vi "sub_pwrpak7-log_conversion.vi"() -> ()   [LabVIEW 2019]
panel:
  out "data T":dbl[](graph)=[382024.75, 382024.8, 382024.85, 382024.9, 382024.95, 382025.0, 382025.05, 382025.1, 382025.15, 382025.2, 382025.25, 382025.3, 382025.35, 382025.4, 382025.45, 382025.5, 382025.55, 382025.65, 382025.75, 382025.85, 382025.95, 382026.05, 382026.15, 382026.25, 382026.35, 382026.45, 382026.55, 382026.65, 382026.75, 382026.85, 382026.95, 382027.05, 382027.15, 382027.25, 382027.35, 382027.45, 382027.55, 382027.65, 382027.75, 382027.85, 382027.95, 382028.05, 382028.15, 382028.25, 382028.35, 382028.45, 382028.55, 382028.65, 382028.75, 382028.75, 382028.85, 382028.95, 382029.0, 382029.05, 382029.2, 382029.25, 382029.4, 382029.45, 382029.45, 382029.6, 382029.65, 382029.65, 382029.8, 382029.85, 382029.85, 382029.95, 382030.0, 382030.05, 382030.1, 382030.15, 382030.2, 382030.25, 382030.3, 382030.35, 382030.4, 382030.45, 382030.5, 382030.55, 382030.6, 382030.65, 382030.7, 382030.75, 382030.8, 382030.85, 382030.9, 382030.95, 382031.0, 382031.05, 382031.1, 382031.15, 382031.2, 382031.25, 382031.3, 382031.35, 382031.45, 382031.5, 382031.55, 382031.65, 382031.7, 382031.75, 382031.85, 382031.95, 382032.05, 382032.15, 382032.25, 382032.35, 382032.45, 382032.55, 382032.65, 382032.75, 382032.85, 382032.95, 382033.05, 382033.15, 382033.25, 382033.35, 382033.45, 382033.55, 382033.65, 382033.75, 382033.85, 382033.95, 382034.05, 382034.15, 382034.25, 382034.35, 382034.45, 382034.55, 382034.65, 382034.65, 382034.75, 382034.85, 382034.95, 382035.05, 382035.15, 382035.25, 382035.25, 382035.35, 382035.45, 382035.5, 382035.55, 382035.7, 382035.75, 382035.85, 382035.9, 382035.95, 382036.05, 382036.1, 382036.15, 382036.3, 382036.35, 382036.35, 382036.5, 382036.55, 382036.55, 382036.7, 382036.75, 382036.75, 382036.85, 382036.9, 382036.95, 382037.0, 382037.05, 382037.1, 382037.15, 382037.2, 382037.25, 382037.3, 382037.35, 382037.4, 382037.45, 382037.5, 382037.55, 382037.6, 382037.65, 382037.7, 382037.75, 382037.8, 382037.85, 382037.95, 382038.0, 382038.05, 382038.15, 382038.2, 382038.25, 382038.35, 382038.4, 382038.45, 382038.55, 382038.6, 382038.65, 382038.75, 382038.8, 382038.85, 382038.95, 382039.05, 382039.15, 382039.25, 382039.3, 382039.35, 382039.45, 382039.5, 382039.55, 382039.65, 382039.7, 382039.75, 382039.85, 382039.95, 382040.05, 382040.15, 382040.25, 382040.35, 382040.45, 382040.55, 382040.65, 382040.75, 382040.85, 382040.95, 382041.05, 382041.15, 382041.25, 382041.35, 382041.45, 382041.55, 382041.65, 382041.75, 382041.85, 382041.95, 382042.05, 382042.15, 382042.25, 382042.35, 382042.35, 382042.5, 382042.55, 382042.55, 382042.7, 382042.75, 382042.75, 382042.9, 382042.95, 382043.0, 382043.05, 382043.15, 382043.2, 382043.3, 382043.35, 382043.4, 382043.45, 382043.55, 382043.6, 382043.65, 382043.65, 382043.75, 382043.8, 382043.85, 382043.85, 382043.95, 382044.0, 382044.05, 382044.1, 382044.15, 382044.2, 382044.25, 382044.3, 382044.35, 382044.4, 382044.45, 382044.5, 382044.55, 382044.6, 382044.65, 382044.7, 382044.75, 382044.8, 382044.85, 382044.9, 382044.95, 382045.05, 382045.1, 382045.15, 382045.25, 382045.3, 382045.35, 382045.45, 382045.5, 382045.55, 382045.65, 382045.7, 382045.75, 382045.85, 382045.9, 382045.95, 382046.0, 382046.05, 382046.15, 382046.25, 382046.35, 382046.45, 382046.55, 382046.65, 382046.75, 382046.85, 382046.95, 382047.05, 382047.15, 382047.25, 382047.35, 382047.45, 382047.55, 382047.65, 382047.75, 382047.85, 382047.95, 382048.05, 382048.15, 382048.25, 382048.35, 382048.45, 382048.55, 382048.65, 382048.75, 382048.85, 382048.95, 382049.05, 382049.15, 382049.25, 382049.35, 382049.45, 382049.55, 382049.55, 382049.65, 382049.75, 382049.8, 382049.85, 382049.95, 382050.0, 382050.05, 382050.05, 382050.15, 382050.2, 382050.25, 382050.25, 382050.35, 382050.4, 382050.45, 382050.45, 382050.55, 382050.6, 382050.65, 382050.7, 382050.75, 382050.8, 382050.85, 382050.9, 382050.95, 382051.0, 382051.05, 382051.1, 382051.15, 382051.2, 382051.25, 382051.3, 382051.35, 382051.4, 382051.45, 382051.5, 382051.55, 382051.65, 382051.7, 382051.75, 382051.85, 382051.9, 382051.95, 382052.05, 382052.1, 382052.15, 382052.25, 382052.3, 382052.35, 382052.45, 382052.5, 382052.55, 382052.65, 382052.75, 382052.85, 382052.95, 382053.05, 382053.15, 382053.25, 382053.35, 382053.45, 382053.55, 382053.65, 382053.75, 382053.85, 382053.95, 382054.05, 382054.15, 382054.25, 382054.35, 382054.45, 382054.55, 382054.65, 382054.75, 382054.85, 382054.95, 382055.05, 382055.15, 382055.25, 382055.35, 382055.45, 382055.6, 382055.65, 382055.75, 382055.85, 382055.95, 382056.05, 382056.05, 382056.15, 382056.25, 382056.25, 382056.35, 382056.45, 382056.5, 382056.55, 382056.65, 382056.7, 382056.75, 382056.85, 382056.9, 382056.95, 382057.05, 382057.1, 382057.15, 382057.15, 382057.25, 382057.3, 382057.35, 382057.35, 382057.45, 382057.5, 382057.55, 382057.6, 382057.65, 382057.7, 382057.75, 382057.8, 382057.85, 382057.9, 382057.95, 382058.0, 382058.05, 382058.1, 382058.15, 382058.2, 382058.25, 382058.3, 382058.35, 382058.4, 382058.45, 382058.55, 382058.6, 382058.65, 382058.75, 382058.8, 382058.85, 382058.95, 382059.0, 382059.05, 382059.15, 382059.2, 382059.25, 382059.35, 382059.4, 382059.45, 382059.55, 382059.6, 382059.65, 382059.75, 382059.8, 382059.85, 382059.95, 382060.0, 382060.05, 382060.15, 382060.25, 382060.35, 382060.4, 382060.45, 382060.55, 382060.6, 382060.65, 382060.75, 382060.85, 382060.95, 382061.05, 382061.15, 382061.25, 382061.35, 382061.45, 382061.55, 382061.65, 382061.75, 382061.85, 382061.95, 382062.05, 382062.15, 382062.25, 382062.35, 382062.45, 382062.55, 382062.65, 382062.75, 382062.85, 382062.95, 382063.05, 382063.05, 382063.15, 382063.25, 382063.25, 382063.35, 382063.45, 382063.5, 382063.55, 382063.65, 382063.7, 382063.75, 382063.85, 382063.9, 382063.95, 382063.95, 382064.1, 382064.15, 382064.15, 382064.25, 382064.3, 382064.35, 382064.35, 382064.5, 382064.55, 382064.6, 382064.7, 382064.75, 382064.8, 382064.9, 382064.95, 382065.0, 382065.05, 382065.1, 382065.15, 382065.2, 382065.25, 382065.3, 382065.35, 382065.4, 382065.45, 382065.5, 382065.55, 382065.6, 382065.65, 382065.75, 382065.8, 382065.85, 382065.9, 382065.95, 382066.0, 382066.05, 382066.1, 382066.15, 382066.2, 382066.25, 382066.3, 382066.35, 382066.4, 382066.45, 382066.5, 382066.55, 382066.65, 382066.7, 382066.75, 382066.85, 382066.9, 382066.95, 382067.05, 382067.1, 382067.15, 382067.25, 382067.3, 382067.35, 382067.45, 382067.5, 382067.55, 382067.65, 382067.75, 382067.85, 382067.9, 382067.95, 382068.05, 382068.15, 382068.25, 382068.35, 382068.45, 382068.55, 382068.65, 382068.75, 382068.85, 382068.95, 382069.05, 382069.15, 382069.25, 382069.35, 382069.45, 382069.55, 382069.65, 382069.75, 382069.85, 382069.95, 382070.05, 382070.15, 382070.25, 382070.35, 382070.45, 382070.55, 382070.55, 382070.65, 382070.75, 382070.75, 382070.9, 382070.95, 382071.1, 382071.15, 382071.15, 382071.3, 382071.35, 382071.35, 382071.45, 382071.55, 382071.6, 382071.7, 382071.75, 382071.8, 382071.85, 382071.95, 382072.0, 382072.05, 382072.1, 382072.15, 382072.2, 382072.25, 382072.25, 382072.35, 382072.4, 382072.45, 382072.45, 382072.55, 382072.6, 382072.65, 382072.75, 382072.8, 382072.85, 382072.9, 382072.95, 382073.0, 382073.05, 382073.1, 382073.15, 382073.2, 382073.25, 382073.3, 382073.35, 382073.4, 382073.45, 382073.5, 382073.55, 382073.6, 382073.65, 382073.7, 382073.75, 382073.8, 382073.85, 382073.95, 382074.05, 382074.1, 382074.15, 382074.25, 382074.35, 382074.45, 382074.5, 382074.55, 382074.65, 382074.75, 382074.85, 382074.95, 382075.05, 382075.15, 382075.25, 382075.35, 382075.45, 382075.55, 382075.65, 382075.75, 382075.85, 382075.95, 382076.05, 382076.15, 382076.25, 382076.35, 382076.45, 382076.55, 382076.7, 382076.75, 382076.9, 382076.95, 382077.05, 382077.15, 382077.15, 382077.3, 382077.35, 382077.35, 382077.45, 382077.55, 382077.55, 382077.7, 382077.75, 382077.8, 382077.9, 382077.95, 382078.0, 382078.05, 382078.15, 382078.2, 382078.25, 382078.3, 382078.35, 382078.4, 382078.45, 382078.5, 382078.55, 382078.6, 382078.65, 382078.7, 382078.75, 382078.8, 382078.85, 382078.95, 382079.0, 382079.05, 382079.15, 382079.2, 382079.25, 382079.35, 382079.4, 382079.45, 382079.55, 382079.6, 382079.65, 382079.7, 382079.75, 382079.85, 382079.95, 382080.05, 382080.15, 382080.25, 382080.35, 382080.45, 382080.5, 382080.55, 382080.65, 382080.75, 382080.85, 382080.95, 382081.05, 382081.15, 382081.25, 382081.35, 382081.45, 382081.55, 382081.65, 382081.75, 382081.85, 382081.95, 382082.05, 382082.15, 382082.25, 382082.35, 382082.45, 382082.55, 382082.65, 382082.75, 382082.85, 382082.95, 382083.05, 382083.15, 382083.3, 382083.35, 382083.45, 382083.55, 382083.7, 382083.75, 382083.75, 382083.9, 382083.95, 382084.1, 382084.15, 382084.15, 382084.3, 382084.35, 382084.35, 382084.5, 382084.55, 382084.55, 382084.65, 382084.7, 382084.75, 382084.75, 382084.9, 382084.95, 382084.95, 382085.05, 382085.1, 382085.15, 382085.15, 382085.25, 382085.3, 382085.35, 382085.35, 382085.45, 382085.5, 382085.55, 382085.6, 382085.65, 382085.7, 382085.75, 382085.8, 382085.85, 382085.9, 382085.95, 382086.0, 382086.05, 382086.1, 382086.15, 382086.2, 382086.25, 382086.3, 382086.35, 382086.4, 382086.45, 382086.55, 382086.6, 382086.65, 382086.75, 382086.8, 382086.85, 382086.95, 382087.0, 382087.05, 382087.15, 382087.2, 382087.25, 382087.35, 382087.45]
  out "heading T":dbl[](graph)=[382025.6, 382025.7, 382025.8, 382025.9, 382026.0, 382026.1, 382026.2, 382026.3, 382026.4, 382026.5, 382026.6, 382026.7, 382026.8, 382026.9, 382027.0, 382027.1, 382027.2, 382027.3, 382027.4, 382027.5, 382027.6, 382027.7, 382027.8, 382027.9, 382028.0, 382028.1, 382028.2, 382028.3, 382028.4, 382028.5, 382028.6, 382028.8, 382029.0, 382029.1, 382029.2, 382029.3, 382029.5, 382029.7, 382031.4, 382031.6, 382031.8, 382031.9, 382032.0, 382032.1, 382032.2, 382032.3, 382032.4, 382032.5, 382032.6, 382032.7, 382032.8, 382032.9, 382033.0, 382033.1, 382033.2, 382033.3, 382033.4, 382033.5, 382033.6, 382033.7, 382033.8, 382033.9, 382034.0, 382034.1, 382034.2, 382034.3, 382034.4, 382034.5, 382034.7, 382034.8, 382034.9, 382035.0, 382035.1, 382035.3, 382035.5, 382035.6, 382035.7, 382035.9, 382036.1, 382036.2, 382036.4, 382036.6, 382037.9, 382038.1, 382038.3, 382038.5, 382038.7, 382038.9, 382039.0, 382039.1, 382039.2, 382039.4, 382039.6, 382039.8, 382039.9, 382040.0, 382040.1, 382040.2, 382040.3, 382040.4, 382040.5, 382040.6, 382040.7, 382040.8, 382040.9, 382041.0, 382041.1, 382041.2, 382041.3, 382041.4, 382041.5, 382041.6, 382041.7, 382041.8, 382041.9, 382042.0, 382042.1, 382042.2, 382042.4, 382042.6, 382042.8, 382043.0, 382043.2, 382043.4, 382045.0, 382045.2, 382045.4, 382045.6, 382045.8, 382046.1, 382046.2, 382046.3, 382046.4, 382046.5, 382046.6, 382046.7, 382046.8, 382046.9, 382047.0, 382047.1, 382047.2, 382047.3, 382047.4, 382047.5, 382047.6, 382047.7, 382047.8, 382047.9, 382048.0, 382048.1, 382048.2, 382048.3, 382048.4, 382048.5, 382048.6, 382048.7, 382048.8, 382048.9, 382049.0, 382049.1, 382049.2, 382049.3, 382049.4, 382049.6, 382049.8, 382051.6, 382051.8, 382052.0, 382052.2, 382052.4, 382052.6, 382052.7, 382052.8, 382052.9, 382053.0, 382053.1, 382053.2, 382053.3, 382053.4, 382053.5, 382053.6, 382053.7, 382053.8, 382053.9, 382054.0, 382054.1, 382054.2, 382054.3, 382054.4, 382054.5, 382054.6, 382054.7, 382054.8, 382054.9, 382055.0, 382055.1, 382055.2, 382055.3, 382055.4, 382055.5, 382055.6, 382055.7, 382055.8, 382055.9, 382056.1, 382056.3, 382056.5, 382056.7, 382056.9, 382058.5, 382058.7, 382058.9, 382059.1, 382059.3, 382059.5, 382059.7, 382059.9, 382060.1, 382060.2, 382060.3, 382060.5, 382060.7, 382060.8, 382060.9, 382061.0, 382061.1, 382061.2, 382061.3, 382061.4, 382061.5, 382061.6, 382061.7, 382061.8, 382061.9, 382062.0, 382062.1, 382062.2, 382062.3, 382062.4, 382062.5, 382062.6, 382062.7, 382062.8, 382062.9, 382063.1, 382063.3, 382063.5, 382063.7, 382064.0, 382064.4, 382064.6, 382064.8, 382065.7, 382066.6, 382066.8, 382067.0, 382067.2, 382067.4, 382067.6, 382067.7, 382067.8, 382068.0, 382068.1, 382068.2, 382068.3, 382068.4, 382068.5, 382068.6, 382068.7, 382068.8, 382068.9, 382069.0, 382069.1, 382069.2, 382069.3, 382069.4, 382069.5, 382069.6, 382069.7, 382069.8, 382069.9, 382070.0, 382070.1, 382070.2, 382070.3, 382070.4, 382070.6, 382070.8, 382070.9, 382071.0, 382071.2, 382071.4, 382071.6, 382071.8, 382072.7, 382073.9, 382074.0, 382074.2, 382074.3, 382074.4, 382074.6, 382074.7, 382074.8, 382074.9, 382075.0, 382075.1, 382075.2, 382075.3, 382075.4, 382075.5, 382075.6, 382075.7, 382075.8, 382075.9, 382076.0, 382076.1, 382076.2, 382076.3, 382076.4, 382076.5, 382076.6, 382076.7, 382076.8, 382076.9, 382077.0, 382077.2, 382077.4, 382077.6, 382077.8, 382078.0, 382078.9, 382079.1, 382079.3, 382079.5, 382079.8, 382079.9, 382080.0, 382080.1, 382080.2, 382080.3, 382080.4, 382080.6, 382080.7, 382080.8, 382080.9, 382081.0, 382081.1, 382081.2, 382081.3, 382081.4, 382081.5, 382081.6, 382081.7, 382081.8, 382081.9, 382082.0, 382082.1, 382082.2, 382082.3, 382082.4, 382082.5, 382082.6, 382082.7, 382082.8, 382082.9, 382083.0, 382083.1, 382083.2, 382083.3, 382083.4, 382083.5, 382083.6, 382083.8, 382083.9, 382084.0, 382084.2, 382084.4, 382084.8, 382086.5, 382086.7, 382086.9, 382087.1, 382087.3, 382087.4]
  out "I":i32=3229
  out "heading arr":string[][](array[string])
  out "data arr":string[][](array[string])
  out "부분배열":string[](array[string])=["", "", "", "", "", "", "", "", "", "", "", "", "", "", "", "", "", "", "", "", "", "", "", "", "", "", "", "", "", "", "", "", "", "", "", "", "", "", "", "", "", "", "", "", "", "", "", "", "", "", "", "", "", "", "", "", "", "", "", "", "", "", "", "", "", "", "", "", "", "", "", "", "", "", "", "", "", "", "", "", "", "", "", "", "", "", "", "", "", "", "", "", "", "", "", "", "", "", "", "", "", "", "", "", "", "", "", "", "", "", "", "", "", "", "", "", "", "", "", "", "", "", "", "", "", "", "", "", "", "", "", "", "", "", "", "", "", "", "", "", "", "", "", "", "", "", "", "", "", "", "", "", "", "", "", "", "", "", "", "", "", "", "", "", "", "", "", "", "", "", "", "", "", "", "", "", "", "", "", "", "", "", "", "", "", "", "", "", "", "", "", "", "", "", "", "", "", "", "", "", "", "", "", "", "", "", "", "", "", "", "", "", "", "", "", "", "", "", "", "", "", "", "", "", "", "", "", "", "", "", "", "", "", "", "", "", "<OK", "robot status", "<OK", "robot status", "<OK", "robot status", "<OK", "robot status", "<OK", "robot status", "<OK", "robot status", "<OK", "robot status", "<OK", "robot status", "<OK", "robot status", "<OK", "robot status", "<OK", "robot status", "<OK", "robot status", "<OK", "robot status", "<OK", "robot status", "<OK", "robot status", "<OK", "robot status", "<OK", "robot status", "<OK", "robot status", "<OK", "robot status", "<OK", "robot status", "<OK", "robot status", "<OK", "robot status", "<OK", "robot status", "<OK", "robot status", "<OK", "robot status", "<OK", "robot status", "<OK", "robot status", "<OK", "robot status", "<OK", "robot status", "<OK", "robot status", "<OK", "robot status", "<OK", "robot status", "<OK", "robot status", "<OK", "robot status", "<OK", "robot status", "<OK", "robot status", "<OK", "robot status", "<OK", "robot status", "<OK", "robot status", "<OK", "robot status", "<OK", "robot status", "<OK", "robot status", "<OK", "robot status", "<OK", "robot status", "<OK", "robot status", "<OK", "robot status", "<OK", "robot status", "<OK", "robot status", "<OK", "robot status", "<OK", "robot status", "<OK", "robot status", "<OK", "robot status", "<OK", "robot status", "<OK", "robot status", "<OK", "robot status", "<OK", "robot status", "<OK", "robot status", "<OK", "robot status", "<OK", "robot status", "<OK", "robot status", "<OK", "robot status", "<OK", "robot status", "<OK", "robot status", "<OK", "robot status", "<OK", "robot status", "<OK", "robot status", "<OK", "robot status", "<OK", "robot status", "<OK", "robot status", "<OK", "robot status", "<OK", "robot status", "<OK", "robot status", "<OK", "robot status", "<OK", "robot status", "<OK", "robot status", "<OK", "robot status", "<OK", "robot status", "<OK", "robot status", "<OK", "robot status", "<OK", "robot status", "<OK", "robot status", "<OK", "robot status", "<OK", "robot status", "<OK", "robot status", "<OK", "robot status", "<OK", "robot status", "<OK", "robot status", "<OK", "robot status", "<OK", "robot status", "<OK", "robot status", "<OK", "robot status", "<OK", "robot status", "<OK", "robot status", "<OK", "robot status", "<OK", "robot status", "<OK", "robot status", "<OK", "robot status", "<OK", "robot status", "<OK", "robot status", "<OK", "robot status", "<OK", "robot status", "<OK", "robot status", "<OK", "robot status", "<OK", "robot status", "<OK", "robot status", "<OK", "robot status", "<OK", "robot status", "<OK", "robot status", "<OK", "robot status", "<OK", "robot status", "<OK", "robot status", "<OK", "robot status", "<OK", "robot status", "<OK", "robot status", "<OK", "robot status", "<OK", "robot status", "<OK", "robot status", "<OK", "robot status", "<OK", "robot status", "<OK", "robot status", "<OK", "robot status", "<OK", "robot status", "<OK", "robot status", "<OK", "robot status", "<OK", "robot status", "<OK", "robot status", "<OK", "robot status", "<OK", "robot status", "<OK", "robot status", "<OK", "robot status", "<OK", "robot status", "<OK", "robot status", "<OK", "robot status", "<OK", "robot status", "<OK", "robot status", "<OK", "robot status", "<OK", "robot status", "<OK", "robot status", "<OK", "robot status", "<OK", "robot status", "<OK", "robot status", "<OK", "robot status", "<OK", "robot status", "<OK", "robot status", "<OK", "robot status", "<OK", "robot status", "<OK", "robot status", "<OK", "robot status", "<OK", "robot status", "<OK", "robot status", "<OK", "robot status", "<OK", "robot status", "<OK", "robot status", "<OK", "robot status", "<OK", "robot status", "<OK", "robot status", "<OK", "robot status", "<OK", "robot status", "<OK", "robot status", "<OK", "robot status", "<OK", "robot status", "<OK", "robot status", "<OK", "robot status", "<OK", "robot status", "<OK", "robot status", "<OK", "robot status", "<OK", "robot status", "<OK", "robot status", "<OK", "robot status", "<OK", "robot status", "<OK", "robot status", "<OK", "robot status", "<OK", "robot status", "<OK", "robot status", "<OK", "robot status", "<OK", "robot status", "<OK", "robot status", "<OK", "robot status", "<OK", "robot status", "<OK", "robot status", "<OK", "robot status", "<OK", "robot status", "<OK", "robot status", "<OK", "robot status", "<OK", "robot status", "<OK", "robot status", "<OK", "robot status", "<OK", "robot status", "<OK", "robot status", "<OK", "robot status", "<OK", "robot status", "<OK", "robot status", "<OK", "robot status", "<OK", "robot status", "<OK", "robot status", "<OK", "robot status", "<OK", "robot status", "<OK", "robot status", "<OK", "robot status", "<OK", "robot status", "<OK", "robot status", "<OK", "robot status", "<OK", "robot status", "<OK", "robot status", "<OK", "robot status", "<OK", "robot status", "<OK", "robot status", "<OK", "robot status", "<OK", "robot status", "<OK", "robot status", "<OK", "robot status", "<OK", "robot status", "<OK", "robot status", "<OK", "robot status", "<OK", "robot status", "<OK", "robot status", "<OK", "robot status", "<OK", "robot status", "<OK", "robot status", "<OK", "robot status", "<OK", "robot status", "<OK", "robot status", "<OK", "robot status", "<OK", "robot status", "<OK", "robot status", "<OK", "robot status", "<OK", "robot status", "<OK", "robot status", "<OK", "robot status", "<OK", "robot status", "<OK", "robot status", "<OK", "robot status", "<OK", "robot status", "<OK", "robot status", "<OK", "robot status", "<OK", "robot status", "<OK", "robot status", "<OK", "robot status", "<OK", "robot status", "<OK", "robot status", "<OK", "robot status", "<OK", "robot status", "<OK", "robot status", "<OK", "robot status", "<OK", "robot status", "<OK", "robot status", "<OK", "robot status", "<OK", "robot status", "<OK", "robot status", "<OK", "robot status", "<OK", "robot status", "#INSPVAXA,USB3,0,41.0,FINESTEERING,2113,382024.750,02000000,471d,15824;INS_SOLUTION_GOOD,INS_RTKFIXED,37.37018369976,126.72086597157,9.9381,22.3000,0.0198,0.0069,0.0055,-0.729721292,-0.467737212,152.592783383,0.0830,0.0922,0.0819,0.0253,0.0263,0.0205,0.0289,0.0288,0.0775,0f000041,0*b216c52d", "robot status", "#INSPVAXA,USB3,0,41.0,FINESTEERING,2113,382024.800,02000000,471d,15824;INS_SOLUTION_GOOD,INS_RTKFIXED,37.37018370626,126.72086597191,9.9383,22.3000,0.0206,0.0063,0.0054,-0.730371572,-0.467330960,152.593899261,0.0830,0.0922,0.0819,0.0253,0.0263,0.0205,0.0289,0.0288,0.0775,0f000041,0*340d1d1e", "robot status", "#INSPVAXA,USB3,0,41.0,FINESTEERING,2113,382024.850,02000000,471d,15824;INS_SOLUTION_GOOD,INS_RTKFIXED,37.37018371265,126.72086597165,9.9385,22.3000,0.0208,0.0067,0.0057,-0.730042287,-0.466924674,152.593459848,0.0830,0.0922,0.0819,0.0253,0.0263,0.0205,0.0289,0.0288,0.0775,0f000041,0*a3e0566d", "robot status", "#INSPVAXA,USB3,0,41.0,FINESTEERING,2113,382024.900,02000000,471d,15824;INS_SOLUTION_GOOD,INS_RTKFIXED,37.37018371942,126.72086597216,9.9387,22.3000,0.0203,0.0070,0.0059,-0.730302817,-0.466656468,152.594518112,0.0830,0.0922,0.0819,0.0253,0.0263,0.0205,0.0289,0.0288,0.0775,0f000041,0*b966c6e0", "robot status", "#INSPVAXA,USB3,0,41.0,FINESTEERING,2113,382024.950,02000000,471d,15824;INS_SOLUTION_GOOD,INS_RTKFIXED,37.37018372616,126.72086597280,9.9389,22.3000,0.0205,0.0071,0.0058,-0.729837391,-0.467014747,152.594484484,0.0830,0.0922,0.0819,0.0253,0.0263,0.0205,0.0289,0.0288,0.0775,0f000041,0*c9b08c61", "robot status", "#INSPVAXA,USB3,0,41.0,FINESTEERING,2113,382025.000,02000000,471d,15824;INS_SOLUTION_GOOD,INS_RTKFIXED,37.37018373314,126.72086597346,9.9392,22.3000,0.0211,0.0068,0.0059,-0.729725959,-0.466969403,152.594152669,0.0830,0.0922,0.0819,0.0253,0.0263,0.0205,0.0289,0.0288,0.0775,0f000041,0*c8abde32", "robot status", "#INSPVAXA,USB3,0,41.0,FINESTEERING,2113,382025.050,02000000,471d,15824;INS_SOLUTION_GOOD,INS_RTKFIXED,37.37018373760,126.72086597197,9.9393,22.3000,0.0218,0.0067,0.0058,-0.729631791,-0.467061420,152.593830540,0.0961,0.1071,0.0938,0.0275,0.0290,0.0215,0.0301,0.0299,0.0782,0f000041,0*f74ecec6", "robot status", "#INSPVAXA,USB3,0,45.5,FINESTEERING,2113,382025.100,02000000,471d,15824;INS_SOLUTION_GOOD,INS_RTKFIXED,37.37018374163,126.72086597046,9.9393,22.3000,0.0217,0.0067,0.0060,-0.730180033,-0.466610622,152.593108629,0.0961,0.1071,0.0938,0.0275,0.0290,0.0215,0.0301,0.0299,0.0782,0f000041,0*ede3f3a7", "robot status", "#INSPVAXA,USB3,0,45.5,FINESTEERING,2113,382025.150,02000000,471d,15824;INS_SOLUTION_GOOD,INS_RTKFIXED,37.37018374560,126.72086596911,9.9394,22.3000,0.0214,0.0071,0.0058,-0.729850693,-0.466261357,152.594252106,0.0961,0.1071,0.0938,0.0275,0.0290,0.0215,0.0301,0.0299,0.0782,0f000041,0*dbccd46e", "robot status", "#INSPVAXA,USB3,0,45.5,FINESTEERING,2113,382025.200,02000000,471d,15824;INS_SOLUTION_GOOD,INS_RTKFIXED,37.37018374958,126.72086596786,9.9395,22.3000,0.0215,0.0068,0.0059,-0.730016188,-0.466427204,152.593304599,0.0961,0.1071,0.0938,0.0275,0.0290,0.0215,0.0301,0.0299,0.0782,0f000041,0*6894b41e", "robot status", "#INSPVAXA,USB3,0,45.5,FINESTEERING,2113,382025.250,02000000,471d,15824;INS_SOLUTION_GOOD,INS_RTKFIXED,37.37018375384,126.72086596657,9.9396,22.3000,0.0223,0.0069,0.0058,-0.730137890,-0.466685773,152.593266150,0.0961,0.1071,0.0938,0.0275,0.0290,0.0215,0.0301,0.0299,0.0782,0f000041,0*47582ee5", "robot status", "#INSPVAXA,USB3,0,45.5,FINESTEERING,2113,382025.300,02000000,471d,15824;INS_SOLUTION_GOOD,INS_RTKFIXED,37.37018375759,126.72086596450,9.9396,22.3000,0.0226,0.0066,0.0057,-0.729934603,-0.466322917,152.593247189,0.0961,0.1071,0.0938,0.0275,0.0290,0.0215,0.0301,0.0299,0.0782,0f000041,0*28a54055", "robot status", "#INSPVAXA,USB3,0,45.5,FINESTEERING,2113,382025.350,02000000,471d,15824;INS_SOLUTION_GOOD,INS_RTKFIXED,37.37018376219,126.72086596322,9.9397,22.3000,0.0224,0.0067,0.0057,-0.729983991,-0.466103112,152.593315489,0.0961,0.1071,0.0938,0.0275,0.0290,0.0215,0.0301,0.0299,0.0782,0f000041,0*5693f211", "robot status", "#INSPVAXA,USB3,0,45.5,FINESTEERING,2113,382025.400,02000000,471d,15824;INS_SOLUTION_GOOD,INS_RTKFIXED,37.37018376676,126.72086596200,9.9398,22.3000,0.0225,0.0065,0.0057,-0.729588122,-0.466736324,152.593809863,0.0961,0.1071,0.0938,0.0275,0.0290,0.0215,0.0301,0.0299,0.0782,0f000041,0*8175a42e", "robot status", "#INSPVAXA,USB3,0,45.5,FINESTEERING,2113,382025.450,02000000,471d,15824;INS_SOLUTION_GOOD,INS_RTKFIXED,37.37018377077,126.72086595999,9.9398,22.3000,0.0231,0.0063,0.0056,-0.729925270,-0.467152594,152.593776517,0.0961,0.1071,0.0938,0.0275,0.0290,0.0215,0.0301,0.0299,0.0782,0f000041,0*10a645a0", "robot status", "#INSPVAXA,USB3,0,45.5,FINESTEERING,2113,382025.500,02000000,471d,15824;INS_SOLUTION_GOOD,INS_RTKFIXED,37.37018377589,126.72086595868,9.9399,22.3000,0.0237,0.0061,0.0057,-0.729817898,-0.467054387,152.593893018,0.0961,0.1071,0.0938,0.0275,0.0290,0.0215,0.0301,0.0299,0.0782,0f000041,0*9fba37f2", "robot status", "#INSPVAXA,USB3,0,45.5,FINESTEERING,2113,382025.550,02000000,471d,15824;INS_SOLUTION_GOOD,INS_RTKFIXED,37.37018378124,126.72086595741,9.9400,22.3000,0.0238,0.0062,0.0056,-0.729449696,-0.467439102,152.593895045,0.0961,0.1071,0.0938,0.0275,0.0290,0.0215,0.0301,0.0299,0.0782,0f000041,0*02ddb99e", "robot status", "#DUALANTENNAHEADINGA,USB3,0,45.5,FINESTEERING,2113,382025.600,02000000,d426,15824;SOL_COMPUTED,NARROW_INT,-1.000000000,157.761886597,-14.048614502,0.0,0.340079188,0.906907201,\"681H\",37,27,27,20,04,00,30,33*30139603", "robot status", "#INSPVAXA,USB3,0,45.5,FINESTEERING,2113,382025.650,02000000,471d,15824;INS_SOLUTION_GOOD,INS_RTKFIXED,37.37018379199,126.72086595512,9.9402,22.3000,0.0238,0.0064,0.0057,-0.729977006,-0.466502482,152.593562345,0.0961,0.1071,0.0938,0.0275,0.0290,0.0215,0.0301,0.0299,0.0782,0f000041,0*e9293c2f", "robot status", "#DUALANTENNAHEADINGA,USB3,0,45.5,FINESTEERING,2113,382025.700,02000000,d426,15824;SOL_COMPUTED,NARROW_INT,-1.000000000,157.699172974,-14.030242920,0.0,0.340588301,0.908101737,\"681H\",37,27,27,20,04,00,30,33*1b355fa5", "robot status", "#INSPVAXA,USB3,0,45.5,FINESTEERING,2113,382025.750,02000000,471d,15824;INS_SOLUTION_GOOD,INS_RTKFIXED,37.37018380260,126.72086595218,9.9404,22.3000,0.0244,0.0062,0.0058,-0.728657563,-0.465931440,152.593624205,0.0961,0.1071,0.0938,0.0275,0.0290,0.0215,0.0301,0.0299,0.0782,0f000041,0*74c13f5b", "robot status", "#DUALANTENNAHEADINGA,USB3,0,45.5,FINESTEERING,2113,382025.800,02000000,d426,15824;SOL_COMPUTED,NARROW_INT,-1.000000000,157.821578979,-14.375122070,0.0,0.342067271,0.910245121,\"681H\",37,27,27,20,04,00,30,33*2529407e", "robot status", "#INSPVAXA,USB3,0,45.5,FINESTEERING,2113,382025.850,02000000,471d,15824;INS_SOLUTION_GOOD,INS_RTKFIXED,37.37018381375,126.72086594948,9.9405,22.3000,0.0243,0.0064,0.0059,-0.728879825,-0.466013684,152.593850424,0.0961,0.1071,0.0938,0.0275,0.0290,0.0215,0.0301,0.0299,0.0782,0f000041,0*d9358f05", "robot status", "#DUALANTENNAHEADINGA,USB3,0,45.5,FINESTEERING,2113,382025.900,02000000,d426,15824;SOL_COMPUTED,NARROW_INT,-1.000000000,157.786605835,-14.218627930,0.0,0.341675878,0.910721183,\"681H\",37,27,27,20,04,00,30,33*64d0d047", "robot status", "#INSPVAXA,USB3,0,45.5,FINESTEERING,2113,382025.950,02000000,471d,15824;INS_SOLUTION_GOOD,INS_RTKFIXED,37.37018382627,126.72086594769,9.9407,22.3000,0.0251,0.0064,0.0057,-0.728736707,-0.465697206,152.593264431,0.0961,0.1071,0.0938,0.0275,0.0290,0.0215,0.0301,0.0299,0.0782,0f000041,0*70b4c2e8", "robot status", "#DUALANTENNAHEADINGA,USB3,0,45.5,FINESTEERING,2113,382026.000,02000000,d426,15824;SOL_COMPUTED,NARROW_INT,-1.000000000,157.656082153,-13.939971924,0.0,0.342579305,0.914604962,\"681H\",37,27,27,20,04,00,30,33*0038ead5", "robot status", "#INSPVAXA,USB3,0,45.5,FINESTEERING,2113,382026.050,02000000,471d,15824;INS_SOLUTION_GOOD,INS_RTKFIXED,37.37018383590,126.72086594359,9.9408,22.3000,0.0254,0.0063,0.0058,-0.728220972,-0.466045039,152.593491664,0.1074,0.1213,0.1046,0.0293,0.0313,0.0223,0.0311,0.0309,0.0789,0f000041,0*ddca915d", "robot status", "#DUALANTENNAHEADINGA,USB3,0,45.5,FINESTEERING,2113,382026.100,02000000,d426,15824;SOL_COMPUTED,NARROW_INT,-1.000000000,157.813766479,-14.580902100,0.0,0.344610006,0.918504715,\"681H\",37,27,27,20,04,00,30,33*b665cead", "robot status", "#INSPVAXA,USB3,0,45.5,FINESTEERING,2113,382026.150,02000000,471d,15824;INS_SOLUTION_GOOD,INS_RTKFIXED,37.37018384191,126.72086593759,9.9409,22.3000,0.0256,0.0061,0.0059,-0.728788620,-0.466458201,152.592754737,0.1074,0.1213,0.1046,0.0293,0.0313,0.0223,0.0311,0.0309,0.0789,0f000041,0*1db6a280", "robot status", "#DUALANTENNAHEADINGA,USB3,0,45.5,FINESTEERING,2113,382026.200,02000000,d426,15824;SOL_COMPUTED,NARROW_INT,-1.000000000,157.657928467,-13.661041260,0.0,0.250532568,0.451991320,\"681H\",37,28,28,21,04,00,30,33*b4e2ce87", "robot status", "#INSPVAXA,USB3,0,45.5,FINESTEERING,2113,382026.250,02000000,471d,15824;INS_SOLUTION_GOOD,INS_RTKFIXED,37.37018384854,126.72086593159,9.9409,22.3000,0.0258,0.0059,0.0061,-0.729011578,-0.466641645,152.592433509,0.1074,0.1213,0.1046,0.0293,0.0313,0.0223,0.0311,0.0309,0.0789,0f000041,0*f2421b2e", "robot status", "#DUALANTENNAHEADINGA,USB3,0,45.5,FINESTEERING,2113,382026.300,02000000,d426,15824;SOL_COMPUTED,NARROW_INT,-1.000000000,157.811996460,-13.674285889,0.0,0.250180334,0.450847596,\"681H\",37,28,28,21,04,00,30,33*6e576a72", "robot status", "#INSPVAXA,USB3,0,45.5,FINESTEERING,2113,382026.350,02000000,471d,15824;INS_SOLUTION_GOOD,INS_RTKFIXED,37.37018385449,126.72086592473,9.9409,22.3000,0.0260,0.0057,0.0060,-0.729419124,-0.468118596,152.593211469,0.1074,0.1213,0.1046,0.0293,0.0313,0.0223,0.0311,0.0309,0.0789,0f000041,0*939db643", "robot status", "#DUALANTENNAHEADINGA,USB3,0,45.5,FINESTEERING,2113,382026.400,02000000,d426,15824;SOL_COMPUTED,NARROW_INT,-1.000000000,157.790802002,-13.518280029,0.0,0.249182746,0.449917048,\"681H\",37,28,28,21,04,00,30,33*9ca43c5c", "robot status", "#INSPVAXA,USB3,0,45.5,FINESTEERING,2113,382026.450,02000000,471d,15824;INS_SOLUTION_GOOD,INS_RTKFIXED,37.37018386083,126.72086591801,9.9409,22.3000,0.0262,0.0056,0.0058,-0.728866584,-0.468667556,152.592837179,0.1074,0.1213,0.1046,0.0293,0.0313,0.0223,0.0311,0.0309,0.0789,0f000041,0*4f8b9385", "robot status", "#DUALANTENNAHEADINGA,USB3,0,45.5,FINESTEERING,2113,382026.500,02000000,d426,15824;SOL_COMPUTED,NARROW_INT,-1.000000000,157.809783936,-13.655975342,0.0,0.249282792,0.449163228,\"681H\",37,28,28,21,04,00,30,33*0a3d9fb3", "robot status", "#INSPVAXA,USB3,0,45.5,FINESTEERING,2113,382026.550,02000000,471d,15824;INS_SOLUTION_GOOD,INS_RTKFIXED,37.37018386863,126.72086591228,9.9410,22.3000,0.0262,0.0056,0.0059,-0.728296903,-0.468521646,152.592669171,0.1074,0.1213,0.1046,0.0293,0.0313,0.0223,0.0311,0.0309,0.0789,0f000041,0*1809c9bb", "robot status", "#DUALANTENNAHEADINGA,USB3,0,45.5,FINESTEERING,2113,382026.600,02000000,d426,15824;SOL_COMPUTED,NARROW_INT,-1.000000000,157.826156616,-13.286224365,0.0,0.249381214,0.450397789,\"681H\",37,28,28,21,04,00,30,33*a1eef553", "robot status", "#INSPVAXA,USB3,0,45.5,FINESTEERING,2113,382026.650,02000000,471d,15824;INS_SOLUTION_GOOD,INS_RTKFIXED,37.37018387390,126.72086590707,9.9411,22.3000,0.0206,0.0090,0.0055,-0.728052930,-0.459535077,152.515196847,0.1074,0.1213,0.1046,0.0293,0.0313,0.0223,0.0311,0.0309,0.0789,0f000041,0*a50522dd", "robot status", "#DUALANTENNAHEADINGA,USB3,0,45.5,FINESTEERING,2113,382026.700,02000000,d426,15824;SOL_COMPUTED,NARROW_INT,-1.000000000,157.605941772,-13.480682373,0.0,0.249976858,0.451360375,\"681H\",37,28,28,21,04,00,30,33*e0b55b15", "robot status", "#INSPVAXA,USB3,0,45.5,FINESTEERING,2113,382026.750,02000000,471d,15824;INS_SOLUTION_GOOD,INS_RTKFIXED,37.37018386692,126.72086591194,9.9411,22.3000,-0.0038,0.0214,0.0051,-0.741471713,-0.426381972,152.256583462,0.1074,0.1213,0.1046,0.0293,0.0313,0.0223,0.0311,0.0309,0.0789,0f000041,0*d49ecacb", "robot status", "#DUALANTENNAHEADINGA,USB3,0,45.5,FINESTEERING,2113,382026.800,02000000,d426,15824;SOL_COMPUTED,NARROW_INT,-1.000000000,157.260543823,-13.341644287,0.0,0.248979479,0.450180978,\"681H\",37,28,28,21,04,00,30,33*89246cae", "robot status", "#INSPVAXA,USB3,0,45.5,FINESTEERING,2113,382026.850,02000000,471d,15824;INS_SOLUTION_GOOD,INS_RTKFIXED,37.37018383812,126.72086592861,9.9412,22.3000,-0.0252,0.0289,0.0067,-0.764949009,-0.395213206,151.943519287,0.1074,0.1213,0.1046,0.0293,0.0313,0.0223,0.0311,0.0309,0.0789,0f000041,0*9ae6352c", "robot status", "#DUALANTENNAHEADINGA,USB3,0,45.5,FINESTEERING,2113,382026.900,02000000,d426,15824;SOL_COMPUTED,NARROW_INT,-1.000000000,156.915863037,-13.211517334,0.0,0.249344677,0.451337904,\"681H\",37,28,28,21,04,00,30,33*a0b0eddf", "robot status", "#INSPVAXA,USB3,0,45.5,FINESTEERING,2113,382026.950,02000000,471d,15824;INS_SOLUTION_GOOD,INS_RTKFIXED,37.37018377309,126.72086595230,9.9415,22.3000,-0.0879,0.0314,0.0029,-0.828695783,-0.285356825,151.441232536,0.1074,0.1213,0.1046,0.0293,0.0313,0.0223,0.0311,0.0309,0.0789,0f000041,0*bf083295", "robot status", "#DUALANTENNAHEADINGA,USB3,0,45.5,FINESTEERING,2113,382027.000,02000000,d426,15824;SOL_COMPUTED,NARROW_INT,-1.000000000,156.241455078,-13.160186768,0.0,0.247624099,0.449924767,\"681H\",37,28,28,21,04,00,30,33*46f838e6", "robot status", "#INSPVAXA,USB3,0,45.5,FINESTEERING,2113,382027.050,02000000,471d,15824;INS_SOLUTION_GOOD,INS_RTKFIXED,37.37018366001,126.72086597018,9.9419,22.3000,-0.1214,0.0319,0.0109,-0.833606937,-0.286887161,150.527554805,0.1173,0.1332,0.1140,0.0308,0.0331,0.0228,0.0320,0.0318,0.0796,0f000041,0*55b03074", "robot status", "#DUALANTENNAHEADINGA,USB3,0,45.0,FINESTEERING,2113,382027.100,02000000,d426,15824;SOL_COMPUTED,NARROW_INT,-1.000000000,155.351913452,-12.896453857,0.0,0.247077301,0.450401723,\"681H\",37,28,28,21,04,00,30,33*84044d4e", "robot status", "#INSPVAXA,USB3,0,45.0,FINESTEERING,2113,382027.150,02000000,471d,15824;INS_SOLUTION_GOOD,INS_RTKFIXED,37.37018352263,126.72086601161,9.9421,22.3000,-0.1357,0.0653,0.0076,-0.832653540,-0.312850321,149.713105011,0.1173,0.1332,0.1140,0.0308,0.0331,0.0228,0.0320,0.0318,0.0796,0f000041,0*6f3a4945", "robot status", "#DUALANTENNAHEADINGA,USB3,0,45.0,FINESTEERING,2113,382027.200,02000000,d426,15824;SOL_COMPUTED,NARROW_INT,-1.000000000,154.459472656,-12.925933838,0.0,0.338010401,0.912385702,\"681H\",37,28,28,23,04,00,30,33*d80ba54f", "robot status", "#INSPVAXA,USB3,0,45.0,FINESTEERING,2113,382027.250,02000000,471d,15824;INS_SOLUTION_GOOD,INS_RTKFIXED,37.37018338020,126.72086607307,9.9424,22.3000,-0.1383,0.0719,0.0046,-0.751633358,-0.331230126,149.109098673,0.1173,0.1332,0.1140,0.0308,0.0331,0.0228,0.0320,0.0318,0.0796,0f000041,0*4ad22fb3", "robot status", "#DUALANTENNAHEADINGA,USB3,0,45.0,FINESTEERING,2113,382027.300,02000000,d426,15824;SOL_COMPUTED,NARROW_INT,-1.000000000,154.180465698,-13.140441895,0.0,0.336679190,0.909444690,\"681H\",37,28,28,23,04,00,30,33*26e9658a", "robot status", "#INSPVAXA,USB3,0,45.0,FINESTEERING,2113,382027.350,02000000,471d,15824;INS_SOLUTION_GOOD,INS_RTKFIXED,37.37018324256,126.72086615320,9.9429,22.3000,-0.1275,0.1002,0.0074,-0.820753827,-0.331514928,148.703206870,0.1173,0.1332,0.1140,0.0308,0.0331,0.0228,0.0320,0.0318,0.0796,0f000041,0*79badbc9", "robot status", "#DUALANTENNAHEADINGA,USB3,0,45.0,FINESTEERING,2113,382027.400,02000000,d426,15824;SOL_COMPUTED,NARROW_INT,-1.000000000,153.986251831,-12.734893799,0.0,0.339710087,0.919114232,\"681H\",37,28,28,23,04,00,30,33*69bcc4de", "robot status", "#INSPVAXA,USB3,0,45.0,FINESTEERING,2113,382027.450,02000000,471d,15824;INS_SOLUTION_GOOD,INS_RTKFIXED,37.37018310294,126.72086624949,9.9427,22.3000,-0.1380,0.0972,0.0053,-0.872166164,-0.381909150,148.411356187,0.1173,0.1332,0.1140,0.0308,0.0331,0.0228,0.0320,0.0318,0.0796,0f000041,0*66da6b52", "robot status", "#DUALANTENNAHEADINGA,USB3,0,45.0,FINESTEERING,2113,382027.500,02000000,d426,15824;SOL_COMPUTED,NARROW_INT,-1.000000000,153.684631348,-12.823913574,0.0,0.338548183,0.917375743,\"681H\",37,28,28,23,04,00,30,33*d83ca21d", "robot status", "#INSPVAXA,USB3,0,45.0,FINESTEERING,2113,382027.550,02000000,471d,15824;INS_SOLUTION_GOOD,INS_RTKFIXED,37.37018296034,126.72086634103,9.9424,22.3000,-0.1391,0.0956,0.0048,-0.818820811,-0.403526520,148.063328951,0.1173,0.1332,0.1140,0.0308,0.0331,0.0228,0.0320,0.0318,0.0796,0f000041,0*baf86aa9", "robot status", "#DUALANTENNAHEADINGA,USB3,0,45.0,FINESTEERING,2113,382027.600,02000000,d426,15824;SOL_COMPUTED,NARROW_INT,-1.000000000,153.287597656,-12.288726807,0.0,0.342138797,0.927053928,\"681H\",37,28,28,23,04,00,30,33*b4d4855d", "robot status", "#INSPVAXA,USB3,0,45.0,FINESTEERING,2113,382027.650,02000000,471d,15824;INS_SOLUTION_GOOD,INS_RTKFIXED,37.37018282250,126.72086643807,9.9425,22.3000,-0.1190,0.0903,0.0088,-0.840171068,-0.453068369,147.683405031,0.1173,0.1332,0.1140,0.0308,0.0331,0.0228,0.0320,0.0318,0.0796,0f000041,0*e3dd1b0e", "robot status", "#DUALANTENNAHEADINGA,USB3,0,45.0,FINESTEERING,2113,382027.700,02000000,d426,15824;SOL_COMPUTED,NARROW_INT,-1.000000000,153.066085815,-12.042663574,0.0,0.343047619,0.930896401,\"681H\",37,28,28,23,04,00,30,33*f2abea1a", "robot status", "#INSPVAXA,USB3,0,45.0,FINESTEERING,2113,382027.750,02000000,471d,15824;INS_SOLUTION_GOOD,INS_RTKFIXED,37.37018269002,126.72086652106,9.9428,22.3000,-0.1372,0.0959,0.0079,-0.778295062,-0.444595992,147.394086139,0.1173,0.1332,0.1140,0.0308,0.0331,0.0228,0.0320,0.0318,0.0796,0f000041,0*3b14e06f", "robot status", "#DUALANTENNAHEADINGA,USB3,0,45.0,FINESTEERING,2113,382027.800,02000000,d426,15824;SOL_COMPUTED,NARROW_INT,-1.000000000,152.814361572,-12.192199707,0.0,0.343393594,0.931128740,\"681H\",37,28,28,23,04,00,30,33*2938f518", "robot status", "#INSPVAXA,USB3,0,45.0,FINESTEERING,2113,382027.850,02000000,471d,15824;INS_SOLUTION_GOOD,INS_RTKFIXED,37.37018254991,126.72086663700,9.9428,22.3000,-0.1414,0.1084,0.0045,-0.824604775,-0.541130568,147.189765666,0.1173,0.1332,0.1140,0.0308,0.0331,0.0228,0.0320,0.0318,0.0796,0f000041,0*b170f649", "robot status", "#DUALANTENNAHEADINGA,USB3,0,45.0,FINESTEERING,2113,382027.900,02000000,d426,15824;SOL_COMPUTED,NARROW_INT,-1.000000000,152.573516846,-13.259033203,0.0,0.344713658,0.933732092,\"681H\",37,28,28,23,04,00,30,33*0652e530", "robot status", "#INSPVAXA,USB3,0,45.0,FINESTEERING,2113,382027.950,02000000,471d,15824;INS_SOLUTION_GOOD,INS_RTKFIXED,37.37018240464,126.72086673027,9.9429,22.3000,-0.1372,0.0996,0.0038,-0.787171702,-0.468906181,146.762263490,0.1173,0.1332,0.1140,0.0308,0.0331,0.0228,0.0320,0.0318,0.0796,0f000041,0*b0a91176", "robot status", "#DUALANTENNAHEADINGA,USB3,0,45.0,FINESTEERING,2113,382028.000,02000000,d426,15824;SOL_COMPUTED,NARROW_INT,-1.000000000,151.886795044,-12.737731934,0.0,0.340786248,0.925476909,\"681H\",37,28,28,23,04,00,30,33*40e8b561", "robot status", "#INSPVAXA,USB3,0,45.0,FINESTEERING,2113,382028.050,02000000,471d,15824;INS_SOLUTION_GOOD,INS_RTKFIXED,37.37018226892,126.72086683422,9.9429,22.3000,-0.1346,0.1080,0.0034,-0.816615190,-0.549208473,146.451006332,0.1266,0.1409,0.1219,0.0324,0.0342,0.0233,0.0326,0.0325,0.0803,0f000041,0*6c3557a7", "robot status", "#DUALANTENNAHEADINGA,USB3,0,45.0,FINESTEERING,2113,382028.100,02000000,d426,15824;SOL_COMPUTED,NARROW_INT,-1.000000000,151.732757568,-13.181213379,0.0,0.342809558,0.927002490,\"681H\",37,28,28,23,04,00,30,33*3a292bc0", "robot status", "#INSPVAXA,USB3,0,45.0,FINESTEERING,2113,382028.150,02000000,471d,15824;INS_SOLUTION_GOOD,INS_RTKFIXED,37.37018211897,126.72086693094,9.9426,22.3000,-0.1461,0.1130,0.0091,-0.730104671,-0.576236530,146.306482822,0.1266,0.1409,0.1219,0.0324,0.0342,0.0233,0.0326,0.0325,0.0803,0f000041,0*e87428ea", "robot status", "#DUALANTENNAHEADINGA,USB3,0,45.0,FINESTEERING,2113,382028.200,02000000,d426,15824;SOL_COMPUTED,NARROW_INT,-1.000000000,151.663055420,-12.860565186,0.0,0.343021452,0.929463506,\"681H\",37,28,28,23,04,00,30,33*bcc4118d", "robot status", "#INSPVAXA,USB3,0,45.0,FINESTEERING,2113,382028.250,02000000,471d,15824;INS_SOLUTION_GOOD,INS_RTKFIXED,37.37018196774,126.72086704330,9.9427,22.3000,-0.1376,0.1224,-0.0049,-0.801020112,-0.544590154,146.071828508,0.1266,0.1409,0.1219,0.0324,0.0342,0.0233,0.0326,0.0325,0.0803,0f000041,0*749635fc", "robot status", "#DUALANTENNAHEADINGA,USB3,0,45.0,FINESTEERING,2113,382028.300,02000000,d426,15824;SOL_COMPUTED,NARROW_INT,-1.000000000,151.432601929,-13.367828369,0.0,0.346029371,0.937085807,\"681H\",37,28,28,23,04,00,30,33*de301cba", "robot status", "#INSPVAXA,USB3,0,45.0,FINESTEERING,2113,382028.350,02000000,471d,15824;INS_SOLUTION_GOOD,INS_RTKFIXED,37.37018182665,126.72086712758,9.9423,22.3000,-0.1264,0.0795,0.0069,-0.743304792,-0.626001329,145.696957983,0.1266,0.1409,0.1219,0.0324,0.0342,0.0233,0.0326,0.0325,0.0803,0f000041,0*437207fc", "robot status", "#DUALANTENNAHEADINGA,USB3,0,45.0,FINESTEERING,2113,382028.400,02000000,d426,15824;SOL_COMPUTED,NARROW_INT,-1.000000000,150.962142944,-13.235198975,0.0,0.348135680,0.943217695,\"681H\",37,28,28,23,04,00,30,33*7acd45ef", "robot status", "#INSPVAXA,USB3,0,45.0,FINESTEERING,2113,382028.450,02000000,471d,15824;INS_SOLUTION_GOOD,INS_RTKFIXED,37.37018169674,126.72086721145,9.9422,22.3000,-0.1150,0.1072,0.0011,-0.695050374,-0.718921850,145.472127602,0.1266,0.1409,0.1219,0.0324,0.0342,0.0233,0.0326,0.0325,0.0803,0f000041,0*eb1df100", "robot status", "#DUALANTENNAHEADINGA,USB3,0,45.0,FINESTEERING,2113,382028.500,02000000,d426,15824;SOL_COMPUTED,NARROW_INT,-1.000000000,150.584945679,-13.356414795,0.0,0.346031010,0.937932432,\"681H\",37,28,28,22,04,00,30,33*9f6e71fb", "robot status", "#INSPVAXA,USB3,0,45.0,FINESTEERING,2113,382028.550,02000000,471d,15824;INS_SOLUTION_GOOD,INS_RTKFIXED,37.37018157142,126.72086729553,9.9422,22.3000,-0.1203,0.0816,0.0095,-0.715162026,-0.699309353,145.126556394,0.1266,0.1409,0.1219,0.0324,0.0342,0.0233,0.0326,0.0325,0.0803,0f000041,0*368ecc1a", "robot status", "#DUALANTENNAHEADINGA,USB3,0,45.0,FINESTEERING,2113,382028.600,02000000,d426,15824;SOL_COMPUTED,NARROW_INT,-1.000000000,150.185440063,-13.701995850,0.0,0.345769703,0.937384784,\"681H\",37,28,28,22,04,00,30,33*f06ae36e", "robot status", "#INSPVAXA,USB3,0,45.0,FINESTEERING,2113,382028.650,02000000,471d,15824;INS_SOLUTION_GOOD,INS_RTKFIXED,37.37018144382,126.72086737306,9.9419,22.3000,-0.1168,0.0950,0.0018,-0.728745914,-0.637370114,144.743835103,0.1266,0.1409,0.1219,0.0324,0.0342,0.0233,0.0326,0.0325,0.0803,0f000041,0*78fc01ae", "robot status", "#INSPVAXA,USB3,0,45.0,FINESTEERING,2113,382028.750,02000000,471d,15824;INS_SOLUTION_GOOD,INS_RTKFIXED,37.37018131816,126.72086746313,9.9417,22.3000,-0.1192,0.1016,-0.0000,-0.723266696,-0.684400467,144.489232544,0.1266,0.1409,0.1219,0.0324,0.0342,0.0233,0.0326,0.0325,0.0803,0f000041,0*9493f89d", "robot status", "#INSPVAXA,USB3,0,45.0,FINESTEERING,2113,382028.750,02000000,471d,15824;INS_SOLUTION_GOOD,INS_RTKFIXED,37.37018131816,126.72086746313,9.9417,22.3000,-0.1192,0.1016,-0.0000,-0.723266696,-0.684400467,144.489232544,0.1266,0.1409,0.1219,0.0324,0.0342,0.0233,0.0326,0.0325,0.0803,0f000041,0*9493f89d", "robot status", "#DUALANTENNAHEADINGA,USB3,0,45.0,FINESTEERING,2113,382028.800,02000000,d426,15824;SOL_COMPUTED,NARROW_INT,-1.000000000,149.314788818,-14.509643555,0.0,0.344122738,0.932756066,\"681H\",37,28,28,23,04,00,30,33*3e386749", "robot status", "#INSPVAXA,USB3,0,45.0,FINESTEERING,2113,382028.850,02000000,471d,15824;INS_SOLUTION_GOOD,INS_RTKFIXED,37.37018119274,126.72086755820,9.9414,22.3000,-0.1203,0.1005,0.0025,-0.731696993,-0.634675365,144.226558190,0.1266,0.1409,0.1219,0.0324,0.0342,0.0233,0.0326,0.0325,0.0803,0f000041,0*01ba01ab", "robot status", "#INSPVAXA,USB3,0,45.0,FINESTEERING,2113,382028.950,02000000,471d,15824;INS_SOLUTION_GOOD,INS_RTKFIXED,37.37018106915,126.72086763924,9.9415,22.3000,-0.1178,0.0835,-0.0063,-0.766877785,-0.487025716,143.856266135,0.1266,0.1409,0.1219,0.0324,0.0342,0.0233,0.0326,0.0325,0.0803,0f000041,0*cc141e23", "robot status", "#INSPVAXA,USB3,0,45.0,FINESTEERING,2113,382029.000,02000000,471d,15824;INS_SOLUTION_GOOD,INS_RTKFIXED,37.37018100836,126.72086767737,9.9413,22.3000,-0.1169,0.0863,-0.0001,-0.740797224,-0.493394451,143.678090005,0.1266,0.1409,0.1219,0.0324,0.0342,0.0233,0.0326,0.0325,0.0803,0f000041,0*2796755e", "robot status", "#DUALANTENNAHEADINGA,USB3,0,45.0,FINESTEERING,2113,382029.000,02000000,d426,15824;SOL_COMPUTED,NARROW_INT,-1.000000000,148.747497559,-14.477294922,0.0,0.343506366,0.931676030,\"681H\",38,28,28,23,04,00,30,33*66bd932d", "robot status", "#INSPVAXA,USB3,0,45.0,FINESTEERING,2113,382029.050,02000000,471d,15824;INS_SOLUTION_GOOD,INS_RTKFIXED,37.37018094029,126.72086771672,9.9409,22.3000,-0.1186,0.0969,-0.0012,-0.731617504,-0.440006284,143.558313047,0.1347,0.1449,0.1282,0.0339,0.0349,0.0235,0.0331,0.0330,0.0810,0f000041,0*02c55e6f", "robot status", "#DUALANTENNAHEADINGA,USB3,0,45.0,FINESTEERING,2113,382029.100,02000000,d426,15824;SOL_COMPUTED,NARROW_INT,-1.000000000,148.538803101,-13.550445557,0.0,0.343090981,0.938554645,\"681H\",38,28,28,23,04,00,30,33*e490c6c8", "robot status", "#INSPVAXA,USB3,0,45.0,FINESTEERING,2113,382029.200,02000000,471d,15824;INS_SOLUTION_GOOD,INS_RTKFIXED,37.37018073980,126.72086787179,9.9404,22.3000,-0.1228,0.1025,-0.0008,-0.773586830,-0.471863439,143.303506074,0.1347,0.1449,0.1282,0.0339,0.0349,0.0235,0.0331,0.0330,0.0810,0f000041,0*31d3088a", "robot status", "#DUALANTENNAHEADINGA,USB3,0,45.0,FINESTEERING,2113,382029.200,02000000,d426,15824;SOL_COMPUTED,NARROW_INT,-1.000000000,148.654098511,-13.142150879,0.0,0.344523758,0.940166295,\"681H\",38,28,28,23,04,00,30,33*2a6385a7", "robot status", "#INSPVAXA,USB3,0,45.0,FINESTEERING,2113,382029.250,02000000,471d,15824;INS_SOLUTION_GOOD,INS_RTKFIXED,37.37018066989,126.72086791715,9.9401,22.3000,-0.1193,0.1000,0.0007,-0.798793107,-0.412955262,143.126156023,0.1347,0.1449,0.1282,0.0339,0.0349,0.0235,0.0331,0.0330,0.0810,0f000041,0*9a915e04", "robot status", "#DUALANTENNAHEADINGA,USB3,0,45.0,FINESTEERING,2113,382029.300,02000000,d426,15824;SOL_COMPUTED,NARROW_INT,-1.000000000,148.217773438,-13.508789063,0.0,0.343095958,0.934650242,\"681H\",38,28,28,23,04,00,30,33*1245e49c", "robot status", "#INSPVAXA,USB3,0,45.0,FINESTEERING,2113,382029.400,02000000,471d,15824;INS_SOLUTION_GOOD,INS_RTKFIXED,37.37018046759,126.72086805050,9.9397,22.3000,-0.1249,0.1031,0.0034,-0.720505559,-0.381138323,142.750222934,0.1347,0.1449,0.1282,0.0339,0.0349,0.0235,0.0331,0.0330,0.0810,0f000041,0*a99795a9", "robot status", "#INSPVAXA,USB3,0,45.0,FINESTEERING,2113,382029.450,02000000,471d,15824;INS_SOLUTION_GOOD,INS_RTKFIXED,37.37018039578,126.72086810323,9.9395,22.3000,-0.1292,0.1217,-0.0014,-0.686897121,-0.384447132,142.697922850,0.1347,0.1449,0.1282,0.0339,0.0349,0.0235,0.0331,0.0330,0.0810,0f000041,0*5af9d940", "robot status", "#INSPVAXA,USB3,0,45.0,FINESTEERING,2113,382029.450,02000000,471d,15824;INS_SOLUTION_GOOD,INS_RTKFIXED,37.37018039578,126.72086810323,9.9395,22.3000,-0.1292,0.1217,-0.0014,-0.686897121,-0.384447132,142.697922850,0.1347,0.1449,0.1282,0.0339,0.0349,0.0235,0.0331,0.0330,0.0810,0f000041,0*5af9d940", "robot status", "#DUALANTENNAHEADINGA,USB3,0,45.0,FINESTEERING,2113,382029.500,02000000,d426,15824;SOL_COMPUTED,NARROW_INT,-1.000000000,147.984436035,-14.029235840,0.0,0.342575997,0.935300469,\"681H\",38,28,28,23,04,00,30,33*f0bdccbb", "robot status", "#INSPVAXA,USB3,0,45.0,FINESTEERING,2113,382029.600,02000000,471d,15824;INS_SOLUTION_GOOD,INS_RTKFIXED,37.37018018620,126.72086826747,9.9390,22.3000,-0.1145,0.0898,0.0016,-0.690148999,-0.336993817,142.313742872,0.1347,0.1449,0.1282,0.0339,0.0349,0.0235,0.0331,0.0330,0.0810,0f000041,0*cd02684e", "robot status", "#INSPVAXA,USB3,0,45.0,FINESTEERING,2113,382029.650,02000000,471d,15824;INS_SOLUTION_GOOD,INS_RTKFIXED,37.37018012125,126.72086830483,9.9388,22.3000,-0.1100,0.0824,-0.0009,-0.656032651,-0.303559739,142.149329661,0.1347,0.1449,0.1282,0.0339,0.0349,0.0235,0.0331,0.0330,0.0810,0f000041,0*ce4c8193", "robot status", "#INSPVAXA,USB3,0,45.0,FINESTEERING,2113,382029.650,02000000,471d,15824;INS_SOLUTION_GOOD,INS_RTKFIXED,37.37018012125,126.72086830483,9.9388,22.3000,-0.1100,0.0824,-0.0009,-0.656032651,-0.303559739,142.149329661,0.1347,0.1449,0.1282,0.0339,0.0349,0.0235,0.0331,0.0330,0.0810,0f000041,0*ce4c8193", "robot status", "#DUALANTENNAHEADINGA,USB3,0,45.0,FINESTEERING,2113,382029.700,02000000,d426,15824;SOL_COMPUTED,NARROW_INT,-1.000000000,147.084045410,-14.474975586,0.0,0.342461318,0.936222255,\"681H\",36,28,28,23,04,00,30,33*aa5376e9", "robot status", "#INSPVAXA,USB3,0,45.0,FINESTEERING,2113,382029.800,02000000,471d,15824;INS_SOLUTION_GOOD,INS_RTKFIXED,37.37017995800,126.72086841502,9.9384,22.3000,-0.0778,0.0753,0.0008,-0.510693599,-0.359491334,141.973133237,0.1347,0.1449,0.1282,0.0339,0.0349,0.0235,0.0331,0.0330,0.0810,0f000041,0*6b4e41f9", "robot status", "#INSPVAXA,USB3,0,45.0,FINESTEERING,2113,382029.850,02000000,471d,15824;INS_SOLUTION_GOOD,INS_RTKFIXED,37.37017991408,126.72086844304,9.9382,22.3000,-0.0531,0.0578,-0.0008,-0.473777902,-0.383229256,142.080235315,0.1347,0.1449,0.1282,0.0339,0.0349,0.0235,0.0331,0.0330,0.0810,0f000041,0*9081a0aa", "robot status", "#INSPVAXA,USB3,0,45.0,FINESTEERING,2113,382029.850,02000000,471d,15824;INS_SOLUTION_GOOD,INS_RTKFIXED,37.37017991408,126.72086844304,9.9382,22.3000,-0.0531,0.0578,-0.0008,-0.473777902,-0.383229256,142.080235315,0.1347,0.1449,0.1282,0.0339,0.0349,0.0235,0.0331,0.0330,0.0810,0f000041,0*9081a0aa", "robot status", "#INSPVAXA,USB3,0,45.0,FINESTEERING,2113,382029.950,02000000,471d,15824;INS_SOLUTION_GOOD,INS_RTKFIXED,37.37017987220,126.72086846481,9.9373,22.3000,0.0136,0.0075,-0.0056,-0.549419245,-0.438856369,142.595872632,0.1347,0.1449,0.1282,0.0339,0.0349,0.0235,0.0331,0.0330,0.0810,0f000041,0*1dff9198", "robot status", "#INSPVAXA,USB3,0,45.0,FINESTEERING,2113,382030.000,02000000,471d,15824;INS_SOLUTION_GOOD,INS_RTKFIXED,37.37017987507,126.72086845270,9.9372,22.3000,0.0501,-0.0145,0.0014,-0.500101526,-0.422133138,142.387042693,0.1347,0.1449,0.1282,0.0339,0.0349,0.0235,0.0331,0.0330,0.0810,0f000041,0*da7a6e44", "robot status", "#INSPVAXA,USB3,0,45.0,FINESTEERING,2113,382030.050,02000000,471d,15824;INS_SOLUTION_GOOD,INS_RTKFIXED,37.37017988457,126.72086843209,9.9369,22.3000,0.0683,-0.0239,-0.0025,-0.537551561,-0.414672106,142.352258707,0.1413,0.1474,0.1331,0.0351,0.0356,0.0237,0.0336,0.0337,0.0817,0f000041,0*332fa38f", "robot status", "#INSPVAXA,USB3,0,42.5,FINESTEERING,2113,382030.100,02000000,471d,15824;INS_SOLUTION_GOOD,INS_RTKFIXED,37.37017989677,126.72086840600,9.9369,22.3000,0.0610,-0.0356,-0.0015,-0.551601155,-0.382946615,142.472938123,0.1413,0.1474,0.1331,0.0351,0.0356,0.0237,0.0336,0.0337,0.0817,0f000041,0*72715536", "robot status", "#INSPVAXA,USB3,0,42.5,FINESTEERING,2113,382030.150,02000000,471d,15824;INS_SOLUTION_GOOD,INS_RTKFIXED,37.37017990426,126.72086837979,9.9367,22.3000,0.0494,-0.0246,-0.0029,-0.532668927,-0.380992522,142.394428538,0.1413,0.1474,0.1331,0.0351,0.0356,0.0237,0.0336,0.0337,0.0817,0f000041,0*0e336d96", "robot status", "#INSPVAXA,USB3,0,42.5,FINESTEERING,2113,382030.200,02000000,471d,15824;INS_SOLUTION_GOOD,INS_RTKFIXED,37.37017990667,126.72086836348,9.9366,22.3000,0.0363,-0.0035,-0.0020,-0.546082139,-0.370728369,142.360741443,0.1413,0.1474,0.1331,0.0351,0.0356,0.0237,0.0336,0.0337,0.0817,0f000041,0*827712c1", "robot status", "#INSPVAXA,USB3,0,42.5,FINESTEERING,2113,382030.250,02000000,471d,15824;INS_SOLUTION_GOOD,INS_RTKFIXED,37.37017989927,126.72086835389,9.9365,22.3000,0.0165,0.0026,-0.0010,-0.563934485,-0.374700017,142.425555375,0.1413,0.1474,0.1331,0.0351,0.0356,0.0237,0.0336,0.0337,0.0817,0f000041,0*f494a8c8", "robot status", "#INSPVAXA,USB3,0,42.5,FINESTEERING,2113,382030.300,02000000,471d,15824;INS_SOLUTION_GOOD,INS_RTKFIXED,37.37017988868,126.72086834599,9.9365,22.3000,0.0123,-0.0006,-0.0027,-0.548180889,-0.387208420,142.402336099,0.1413,0.1474,0.1331,0.0351,0.0356,0.0237,0.0336,0.0337,0.0817,0f000041,0*0d7cbe96", "robot status", "#INSPVAXA,USB3,0,42.5,FINESTEERING,2113,382030.350,02000000,471d,15824;INS_SOLUTION_GOOD,INS_RTKFIXED,37.37017988049,126.72086833702,9.9364,22.3000,0.0243,-0.0015,-0.0010,-0.538574228,-0.392377468,142.413056231,0.1413,0.1474,0.1331,0.0351,0.0356,0.0237,0.0336,0.0337,0.0817,0f000041,0*a750c7ba", "robot status", "#INSPVAXA,USB3,0,42.5,FINESTEERING,2113,382030.400,02000000,471d,15824;INS_SOLUTION_GOOD,INS_RTKFIXED,37.37017987738,126.72086832643,9.9363,22.3000,0.0334,-0.0073,-0.0023,-0.547534085,-0.390686577,142.431405168,0.1413,0.1474,0.1331,0.0351,0.0356,0.0237,0.0336,0.0337,0.0817,0f000041,0*99389371", "robot status", "#INSPVAXA,USB3,0,42.5,FINESTEERING,2113,382030.450,02000000,471d,15824;INS_SOLUTION_GOOD,INS_RTKFIXED,37.37017987639,126.72086831177,9.9362,22.3000,0.0337,-0.0146,-0.0015,-0.545800579,-0.385454638,142.405840222,0.1413,0.1474,0.1331,0.0351,0.0356,0.0237,0.0336,0.0337,0.0817,0f000041,0*309c8354", "robot status", "#INSPVAXA,USB3,0,42.5,FINESTEERING,2113,382030.500,02000000,471d,15824;INS_SOLUTION_GOOD,INS_RTKFIXED,37.37017987255,126.72086829529,9.9361,22.3000,0.0310,-0.0103,-0.0013,-0.541731022,-0.379840887,142.416856827,0.1413,0.1474,0.1331,0.0351,0.0356,0.0237,0.0336,0.0337,0.0817,0f000041,0*28cfb681", "robot status", "#INSPVAXA,USB3,0,42.5,FINESTEERING,2113,382030.550,02000000,471d,15824;INS_SOLUTION_GOOD,INS_RTKFIXED,37.37017986983,126.72086828341,9.9360,22.3000,0.0271,-0.0039,-0.0021,-0.546418678,-0.380531626,142.414757469,0.1413,0.1474,0.1331,0.0351,0.0356,0.0237,0.0336,0.0337,0.0817,0f000041,0*9dd20320", "robot status", "#INSPVAXA,USB3,0,42.5,FINESTEERING,2113,382030.600,02000000,471d,15824;INS_SOLUTION_GOOD,INS_RTKFIXED,37.37017986548,126.72086827271,9.9359,22.3000,0.0239,-0.0058,-0.0017,-0.547988045,-0.386001302,142.410059408,0.1413,0.1474,0.1331,0.0351,0.0356,0.0237,0.0336,0.0337,0.0817,0f000041,0*b31e4140", "robot status", "#INSPVAXA,USB3,0,42.5,FINESTEERING,2113,382030.650,02000000,471d,15824;INS_SOLUTION_GOOD,INS_RTKFIXED,37.37017985896,126.72086825909,9.9359,22.3000,0.0272,-0.0092,-0.0018,-0.543750597,-0.386107961,142.422594945,0.1413,0.1474,0.1331,0.0351,0.0356,0.0237,0.0336,0.0337,0.0817,0f000041,0*9c47158f", "robot status", "#INSPVAXA,USB3,0,42.5,FINESTEERING,2113,382030.700,02000000,471d,15824;INS_SOLUTION_GOOD,INS_RTKFIXED,37.37017985692,126.72086824601,9.9358,22.3000,0.0315,-0.0094,-0.0020,-0.542536221,-0.385294075,142.414689640,0.1413,0.1474,0.1331,0.0351,0.0356,0.0237,0.0336,0.0337,0.0817,0f000041,0*86e73438", "robot status", "#INSPVAXA,USB3,0,42.5,FINESTEERING,2113,382030.750,02000000,471d,15824;INS_SOLUTION_GOOD,INS_RTKFIXED,37.37017985566,126.72086823282,9.9357,22.3000,0.0301,-0.0098,-0.0019,-0.547292860,-0.381578568,142.415561153,0.1413,0.1474,0.1331,0.0351,0.0356,0.0237,0.0336,0.0337,0.0817,0f000041,0*1cdf1f9d", "robot status", "#INSPVAXA,USB3,0,42.5,FINESTEERING,2113,382030.800,02000000,471d,15824;INS_SOLUTION_GOOD,INS_RTKFIXED,37.37017985294,126.72086821975,9.9356,22.3000,0.0256,-0.0089,-0.0021,-0.546222115,-0.380559388,142.417813308,0.1413,0.1474,0.1331,0.0351,0.0356,0.0237,0.0336,0.0337,0.0817,0f000041,0*16aa2e26", "robot status", "#INSPVAXA,USB3,0,42.5,FINESTEERING,2113,382030.850,02000000,471d,15824;INS_SOLUTION_GOOD,INS_RTKFIXED,37.37017984948,126.72086820783,9.9355,22.3000,0.0258,-0.0066,-0.0021,-0.544040370,-0.383622061,142.414564641,0.1413,0.1474,0.1331,0.0351,0.0356,0.0237,0.0336,0.0337,0.0817,0f000041,0*28959844", "robot status", "#INSPVAXA,USB3,0,42.5,FINESTEERING,2113,382030.900,02000000,471d,15824;INS_SOLUTION_GOOD,INS_RTKFIXED,37.37017984439,126.72086819477,9.9354,22.3000,0.0279,-0.0088,-0.0019,-0.546777227,-0.385245828,142.420637928,0.1413,0.1474,0.1331,0.0351,0.0356,0.0237,0.0336,0.0337,0.0817,0f000041,0*6f79455c", "robot status", "#INSPVAXA,USB3,0,42.5,FINESTEERING,2113,382030.950,02000000,471d,15824;INS_SOLUTION_GOOD,INS_RTKFIXED,37.37017984259,126.72086818141,9.9353,22.3000,0.0291,-0.0119,-0.0019,-0.546344698,-0.384266415,142.416913485,0.1413,0.1474,0.1331,0.0351,0.0356,0.0237,0.0336,0.0337,0.0817,0f000041,0*b907505a", "robot status", "#INSPVAXA,USB3,0,42.5,FINESTEERING,2113,382031.000,02000000,471d,15824;INS_SOLUTION_GOOD,INS_RTKFIXED,37.37017984109,126.72086816755,9.9353,22.3000,0.0287,-0.0109,-0.0017,-0.545584609,-0.382148088,142.415514521,0.1413,0.1474,0.1331,0.0351,0.0356,0.0237,0.0336,0.0337,0.0817,0f000041,0*7a1b9ac2", "robot status", "#INSPVAXA,USB3,0,42.5,FINESTEERING,2113,382031.050,02000000,471d,15824;INS_SOLUTION_GOOD,INS_RTKFIXED,37.37017983424,126.72086815425,9.9351,22.3000,0.0267,-0.0089,-0.0018,-0.547505658,-0.381237454,142.417505280,0.1462,0.1496,0.1369,0.0360,0.0363,0.0239,0.0342,0.0343,0.0825,0f000041,0*6dd38661", "robot status", "#INSPVAXA,USB3,0,44.0,FINESTEERING,2113,382031.100,02000000,471d,15824;INS_SOLUTION_GOOD,INS_RTKFIXED,37.37017982843,126.72086814301,9.9350,22.3000,0.0256,-0.0097,-0.0017,-0.546965838,-0.381770900,142.416361696,0.1462,0.1496,0.1369,0.0360,0.0363,0.0239,0.0342,0.0343,0.0825,0f000041,0*c332444d", "robot status", "#INSPVAXA,USB3,0,44.0,FINESTEERING,2113,382031.150,02000000,471d,15824;INS_SOLUTION_GOOD,INS_RTKFIXED,37.37017982297,126.72086813118,9.9349,22.3000,0.0273,-0.0108,-0.0015,-0.545126210,-0.382317151,142.419621658,0.1462,0.1496,0.1369,0.0360,0.0363,0.0239,0.0342,0.0343,0.0825,0f000041,0*c375f341", "robot status", "#INSPVAXA,USB3,0,44.0,FINESTEERING,2113,382031.200,02000000,471d,15824;INS_SOLUTION_GOOD,INS_RTKFIXED,37.37017981847,126.72086811894,9.9347,22.3000,0.0289,-0.0113,-0.0017,-0.546685897,-0.380513956,142.416970449,0.1462,0.1496,0.1369,0.0360,0.0363,0.0239,0.0342,0.0343,0.0825,0f000041,0*eeb4dfa7", "robot status", "#INSPVAXA,USB3,0,44.0,FINESTEERING,2113,382031.250,02000000,471d,15824;INS_SOLUTION_GOOD,INS_RTKFIXED,37.37017981172,126.72086810567,9.9346,22.3000,0.0276,-0.0115,-0.0018,-0.547971580,-0.379632756,142.416363509,0.1462,0.1496,0.1369,0.0360,0.0363,0.0239,0.0342,0.0343,0.0825,0f000041,0*ff4e777b", "robot status", "#INSPVAXA,USB3,0,44.0,FINESTEERING,2113,382031.300,02000000,471d,15824;INS_SOLUTION_GOOD,INS_RTKFIXED,37.37017980678,126.72086809354,9.9344,22.3000,0.0256,-0.0106,-0.0018,-0.546737394,-0.379360102,142.417700456,0.1462,0.1496,0.1369,0.0360,0.0363,0.0239,0.0342,0.0343,0.0825,0f000041,0*ed2b430a", "robot status", "#INSPVAXA,USB3,0,44.0,FINESTEERING,2113,382031.350,02000000,471d,15824;INS_SOLUTION_GOOD,INS_RTKFIXED,37.37017980173,126.72086808187,9.9343,22.3000,0.0261,-0.0103,-0.0019,-0.547079467,-0.381109001,142.416768344,0.1462,0.1496,0.1369,0.0360,0.0363,0.0239,0.0342,0.0343,0.0825,0f000041,0*a1ec21f2", "robot status", "#DUALANTENNAHEADINGA,USB3,0,44.0,FINESTEERING,2113,382031.400,02000000,d426,15824;SOL_COMPUTED,NARROW_INT,-1.000000000,147.424392700,-13.453247070,0.0,0.338110238,0.920547247,\"681H\",37,28,28,24,04,00,30,33*ddc00683", "robot status", "#INSPVAXA,USB3,0,44.0,FINESTEERING,2113,382031.450,02000000,471d,15824;INS_SOLUTION_GOOD,INS_RTKFIXED,37.37017979066,126.72086805628,9.9340,22.3000,0.0275,-0.0125,-0.0020,-0.547539180,-0.380361963,142.417580645,0.1462,0.1496,0.1369,0.0360,0.0363,0.0239,0.0342,0.0343,0.0825,0f000041,0*94092a02", "robot status", "#INSPVAXA,USB3,0,44.0,FINESTEERING,2113,382031.500,02000000,471d,15824;INS_SOLUTION_GOOD,INS_RTKFIXED,37.37017978659,126.72086804382,9.9339,22.3000,0.0268,-0.0116,-0.0021,-0.546948573,-0.378855506,142.417510041,0.1462,0.1496,0.1369,0.0360,0.0363,0.0239,0.0342,0.0343,0.0825,0f000041,0*0e229a32", "robot status", "#INSPVAXA,USB3,0,44.0,FINESTEERING,2113,382031.550,02000000,471d,15824;INS_SOLUTION_GOOD,INS_RTKFIXED,37.37017978224,126.72086803181,9.9337,22.3000,0.0256,-0.0111,-0.0023,-0.547686208,-0.380389728,142.418399270,0.1462,0.1496,0.1369,0.0360,0.0363,0.0239,0.0342,0.0343,0.0825,0f000041,0*4345ee88", "robot status", "#DUALANTENNAHEADINGA,USB3,0,44.0,FINESTEERING,2113,382031.600,02000000,d426,15824;SOL_COMPUTED,NARROW_INT,-1.000000000,147.570556641,-14.387939453,0.0,0.338513523,0.918324351,\"681H\",37,28,28,24,04,00,30,33*53154418", "robot status", "#INSPVAXA,USB3,0,44.0,FINESTEERING,2113,382031.650,02000000,471d,15824;INS_SOLUTION_GOOD,INS_RTKFIXED,37.37017977119,126.72086800644,9.9334,22.3000,0.0265,-0.0124,-0.0022,-0.546796964,-0.380689614,142.418751964,0.1462,0.1496,0.1369,0.0360,0.0363,0.0239,0.0342,0.0343,0.0825,0f000041,0*1ed2b6c6", "robot status", "#INSPVAXA,USB3,0,44.0,FINESTEERING,2113,382031.700,02000000,471d,15824;INS_SOLUTION_GOOD,INS_RTKFIXED,37.37017976745,126.72086799376,9.9332,22.3000,0.0264,-0.0129,-0.0021,-0.547228105,-0.379461001,142.417510213,0.1462,0.1496,0.1369,0.0360,0.0363,0.0239,0.0342,0.0343,0.0825,0f000041,0*389e13a0", "robot status", "#INSPVAXA,USB3,0,44.0,FINESTEERING,2113,382031.750,02000000,471d,15824;INS_SOLUTION_GOOD,INS_RTKFIXED,37.37017976363,126.72086798106,9.9331,22.3000,0.0255,-0.0126,-0.0023,-0.546414505,-0.379195147,142.417465304,0.1462,0.1496,0.1369,0.0360,0.0363,0.0239,0.0342,0.0343,0.0825,0f000041,0*77c33b70", "robot status", "#DUALANTENNAHEADINGA,USB3,0,44.0,FINESTEERING,2113,382031.800,02000000,d426,15824;SOL_COMPUTED,NARROW_INT,-1.000000000,147.497467041,-13.451293945,0.0,0.335862130,0.915910482,\"681H\",37,28,28,24,04,00,30,33*822b83fb", "robot status", "#INSPVAXA,USB3,0,44.0,FINESTEERING,2113,382031.850,02000000,471d,15824;INS_SOLUTION_GOOD,INS_RTKFIXED,37.37017975564,126.72086795593,9.9327,22.3000,0.0255,-0.0131,-0.0025,-0.546170185,-0.379325924,142.417840920,0.1462,0.1496,0.1369,0.0360,0.0363,0.0239,0.0342,0.0343,0.0825,0f000041,0*a8273bf7", "robot status", "#DUALANTENNAHEADINGA,USB3,0,44.0,FINESTEERING,2113,382031.900,02000000,d426,15824;SOL_COMPUTED,NARROW_INT,-1.000000000,147.633483887,-13.628692627,0.0,0.336416453,0.918723643,\"681H\",37,28,28,24,04,00,30,33*aee097b1", "robot status", "#INSPVAXA,USB3,0,44.0,FINESTEERING,2113,382031.950,02000000,471d,15824;INS_SOLUTION_GOOD,INS_RTKFIXED,37.37017974622,126.72086792884,9.9324,22.3000,0.0255,-0.0140,-0.0023,-0.546314526,-0.377783765,142.419101431,0.1462,0.1496,0.1369,0.0360,0.0363,0.0239,0.0342,0.0343,0.0825,0f000041,0*6b4fe082", "robot status", "#DUALANTENNAHEADINGA,USB3,0,44.0,FINESTEERING,2113,382032.000,02000000,d426,15824;SOL_COMPUTED,NARROW_INT,-1.000000000,147.470779419,-13.850677490,0.0,0.335202277,0.914509058,\"681H\",37,27,27,22,04,00,30,33*bc4e5f73", "robot status", "#INSPVAXA,USB3,0,44.0,FINESTEERING,2113,382032.050,02000000,471d,15824;INS_SOLUTION_GOOD,INS_RTKFIXED,37.37017973358,126.72086790495,9.9321,22.3000,0.0242,-0.0138,-0.0026,-0.546322742,-0.378433365,142.418321183,0.1497,0.1514,0.1395,0.0368,0.0370,0.0241,0.0347,0.0348,0.0832,0f000041,0*1b0862e2", "robot status", "#DUALANTENNAHEADINGA,USB3,0,44.0,FINESTEERING,2113,382032.100,02000000,d426,15824;SOL_COMPUTED,NARROW_INT,-1.000000000,147.471832275,-13.630493164,0.0,0.334774137,0.911805034,\"681H\",37,28,28,23,04,00,30,33*a85516f5", "robot status", "#INSPVAXA,USB3,0,46.0,FINESTEERING,2113,382032.150,02000000,471d,15824;INS_SOLUTION_GOOD,INS_RTKFIXED,37.37017971904,126.72086788710,9.9319,22.3000,0.0247,-0.0146,-0.0027,-0.547023789,-0.378098606,142.417033366,0.1497,0.1514,0.1395,0.0368,0.0370,0.0241,0.0347,0.0348,0.0832,0f000041,0*d24c5010", "robot status", "#DUALANTENNAHEADINGA,USB3,0,46.0,FINESTEERING,2113,382032.200,02000000,d426,15824;SOL_COMPUTED,NARROW_INT,-1.000000000,147.567276001,-13.428741455,0.0,0.334659070,0.913134634,\"681H\",37,28,28,23,04,00,30,33*61ef7426", "robot status", "#INSPVAXA,USB3,0,46.0,FINESTEERING,2113,382032.250,02000000,471d,15824;INS_SOLUTION_GOOD,INS_RTKFIXED,37.37017970240,126.72086786881,9.9317,22.3000,0.0240,-0.0145,-0.0031,-0.547665259,-0.378798614,142.416391203,0.1497,0.1514,0.1395,0.0368,0.0370,0.0241,0.0347,0.0348,0.0832,0f000041,0*452dd163", "robot status", "#DUALANTENNAHEADINGA,USB3,0,46.0,FINESTEERING,2113,382032.300,02000000,d426,15824;SOL_COMPUTED,NARROW_INT,-1.000000000,147.542755127,-13.863616943,0.0,0.335281938,0.914014935,\"681H\",37,28,28,23,04,00,30,33*d153f4e1", "robot status", "#INSPVAXA,USB3,0,46.0,FINESTEERING,2113,382032.350,02000000,471d,15824;INS_SOLUTION_GOOD,INS_RTKFIXED,37.37017968868,126.72086785066,9.9314,22.3000,0.0242,-0.0149,-0.0035,-0.547446160,-0.378237080,142.416983778,0.1497,0.1514,0.1395,0.0368,0.0370,0.0241,0.0347,0.0348,0.0832,0f000041,0*ccacac98", "robot status", "#DUALANTENNAHEADINGA,USB3,0,46.0,FINESTEERING,2113,382032.400,02000000,d426,15824;SOL_COMPUTED,NARROW_INT,-1.000000000,147.633514404,-14.064239502,0.0,0.333826274,0.907531559,\"681H\",37,28,28,23,04,00,30,33*b10c0148", "robot status", "#INSPVAXA,USB3,0,46.0,FINESTEERING,2113,382032.450,02000000,471d,15824;INS_SOLUTION_GOOD,INS_RTKFIXED,37.37017967567,126.72086783218,9.9311,22.3000,0.0239,-0.0147,-0.0034,-0.547421366,-0.376637268,142.416122870,0.1497,0.1514,0.1395,0.0368,0.0370,0.0241,0.0347,0.0348,0.0832,0f000041,0*c68f6a9e", "robot status", "#DUALANTENNAHEADINGA,USB3,0,46.0,FINESTEERING,2113,382032.500,02000000,d426,15824;SOL_COMPUTED,NARROW_INT,-1.000000000,147.605773926,-13.720153809,0.0,0.334427088,0.910322726,\"681H\",37,28,28,23,04,00,30,33*8e08e436", "robot status", "#INSPVAXA,USB3,0,46.0,FINESTEERING,2113,382032.550,02000000,471d,15824;INS_SOLUTION_GOOD,INS_RTKFIXED,37.37017966024,126.72086781356,9.9308,22.3000,0.0234,-0.0151,-0.0034,-0.548213170,-0.375706833,142.416349114,0.1497,0.1514,0.1395,0.0368,0.0370,0.0241,0.0347,0.0348,0.0832,0f000041,0*8d184a72", "robot status", "#DUALANTENNAHEADINGA,USB3,0,46.0,FINESTEERING,2113,382032.600,02000000,d426,15824;SOL_COMPUTED,NARROW_INT,-1.000000000,147.680450439,-14.212280273,0.0,0.337830007,0.918079555,\"681H\",37,28,28,24,04,00,30,33*ec6cbef1", "robot status", "#INSPVAXA,USB3,0,46.0,FINESTEERING,2113,382032.650,02000000,471d,15824;INS_SOLUTION_GOOD,INS_RTKFIXED,37.37017964547,126.72086779453,9.9306,22.3000,0.0236,-0.0153,-0.0036,-0.547465626,-0.374246908,142.416504998,0.1497,0.1514,0.1395,0.0368,0.0370,0.0241,0.0347,0.0348,0.0832,0f000041,0*18f20d28", "robot status", "#DUALANTENNAHEADINGA,USB3,0,46.0,FINESTEERING,2113,382032.700,02000000,d426,15824;SOL_COMPUTED,NARROW_INT,-1.000000000,147.557327271,-13.653442383,0.0,0.336965472,0.918174922,\"681H\",37,28,28,24,04,00,30,33*76931c3f", "robot status", "#INSPVAXA,USB3,0,46.0,FINESTEERING,2113,382032.750,02000000,471d,15824;INS_SOLUTION_GOOD,INS_RTKFIXED,37.37017963382,126.72086777558,9.9302,22.3000,0.0235,-0.0156,-0.0038,-0.547787938,-0.375922635,142.416770454,0.1497,0.1514,0.1395,0.0368,0.0370,0.0241,0.0347,0.0348,0.0832,0f000041,0*89b2a1f1", "robot status", "#DUALANTENNAHEADINGA,USB3,0,46.0,FINESTEERING,2113,382032.800,02000000,d426,15824;SOL_COMPUTED,NARROW_INT,-1.000000000,147.587890625,-13.205261230,0.0,0.335237086,0.914233923,\"681H\",37,28,28,24,04,00,30,33*a40483ec", "robot status", "#INSPVAXA,USB3,0,46.0,FINESTEERING,2113,382032.850,02000000,471d,15824;INS_SOLUTION_GOOD,INS_RTKFIXED,37.37017962290,126.72086775622,9.9299,22.3000,0.0237,-0.0159,-0.0041,-0.546930434,-0.376234284,142.415444705,0.1497,0.1514,0.1395,0.0368,0.0370,0.0241,0.0347,0.0348,0.0832,0f000041,0*240c5b47", "robot status", "#DUALANTENNAHEADINGA,USB3,0,46.0,FINESTEERING,2113,382032.900,02000000,d426,15824;SOL_COMPUTED,NARROW_INT,-1.000000000,147.621200562,-13.761627197,0.0,0.337081671,0.918612719,\"681H\",37,28,28,23,04,00,30,33*24926c59", "robot status", "#INSPVAXA,USB3,0,46.0,FINESTEERING,2113,382032.950,02000000,471d,15824;INS_SOLUTION_GOOD,INS_RTKFIXED,37.37017961001,126.72086773644,9.9296,22.3000,0.0235,-0.0158,-0.0041,-0.547138206,-0.375895619,142.415215242,0.1497,0.1514,0.1395,0.0368,0.0370,0.0241,0.0347,0.0348,0.0832,0f000041,0*5c19a7e7", "robot status", "#DUALANTENNAHEADINGA,USB3,0,46.0,FINESTEERING,2113,382033.000,02000000,d426,15824;SOL_COMPUTED,NARROW_INT,-1.000000000,147.660507202,-13.878356934,0.0,0.338865966,0.922558546,\"681H\",37,28,28,23,04,00,30,33*c713fa30", "robot status", "#INSPVAXA,USB3,0,46.0,FINESTEERING,2113,382033.050,02000000,471d,15824;INS_SOLUTION_GOOD,INS_RTKFIXED,37.37017959900,126.72086771810,9.9293,22.3000,0.0236,-0.0163,-0.0041,-0.547176543,-0.375392866,142.415846508,0.1520,0.1529,0.1414,0.0375,0.0376,0.0242,0.0351,0.0352,0.0840,0f000041,0*479fcffc", "robot status", "#DUALANTENNAHEADINGA,USB3,0,46.0,FINESTEERING,2113,382033.100,02000000,d426,15824;SOL_COMPUTED,NARROW_INT,-1.000000000,147.663513184,-14.312103271,0.0,0.341427773,0.929877698,\"681H\",37,28,28,23,04,00,30,33*7c949c2f", "robot status", "#INSPVAXA,USB3,0,46.0,FINESTEERING,2113,382033.150,02000000,471d,15824;INS_SOLUTION_GOOD,INS_RTKFIXED,37.37017958595,126.72086770344,9.9293,22.3000,0.0233,-0.0165,-0.0041,-0.547100497,-0.375669663,142.415603725,0.1520,0.1529,0.1414,0.0375,0.0376,0.0242,0.0351,0.0352,0.0840,0f000041,0*64787cd5", "robot status", "#DUALANTENNAHEADINGA,USB3,0,46.0,FINESTEERING,2113,382033.200,02000000,d426,15824;SOL_COMPUTED,NARROW_INT,-1.000000000,147.501770020,-12.949005127,0.0,0.338094473,0.924235582,\"681H\",37,29,29,24,04,00,30,33*1e691d39", "robot status", "#INSPVAXA,USB3,0,46.0,FINESTEERING,2113,382033.250,02000000,471d,15824;INS_SOLUTION_GOOD,INS_RTKFIXED,37.37017957334,126.72086768869,9.9293,22.3000,0.0234,-0.0165,-0.0043,-0.547810074,-0.375834004,142.415588762,0.1520,0.1529,0.1414,0.0375,0.0376,0.0242,0.0351,0.0352,0.0840,0f000041,0*5721023b", "robot status", "#DUALANTENNAHEADINGA,USB3,0,46.0,FINESTEERING,2113,382033.300,02000000,d426,15824;SOL_COMPUTED,NARROW_INT,-1.000000000,147.555221558,-13.413085938,0.0,0.338916332,0.923790455,\"681H\",37,29,29,24,04,00,30,33*f67f1fa1", "robot status", "#INSPVAXA,USB3,0,46.0,FINESTEERING,2113,382033.350,02000000,471d,15824;INS_SOLUTION_GOOD,INS_RTKFIXED,37.37017956342,126.72086767341,9.9292,22.3000,0.0229,-0.0166,-0.0043,-0.547694562,-0.375635405,142.415026909,0.1520,0.1529,0.1414,0.0375,0.0376,0.0242,0.0351,0.0352,0.0840,0f000041,0*8dcfcd57", "robot status", "#DUALANTENNAHEADINGA,USB3,0,46.0,FINESTEERING,2113,382033.400,02000000,d426,15824;SOL_COMPUTED,NARROW_INT,-1.000000000,147.773559570,-13.823394775,0.0,0.340764105,0.928639412,\"681H\",37,29,29,24,04,00,30,33*1ef169a5", "robot status", "#INSPVAXA,USB3,0,46.0,FINESTEERING,2113,382033.450,02000000,471d,15824;INS_SOLUTION_GOOD,INS_RTKFIXED,37.37017955259,126.72086765939,9.9291,22.3000,0.0186,-0.0125,-0.0047,-0.547916877,-0.371886801,142.368633785,0.1520,0.1529,0.1414,0.0375,0.0376,0.0242,0.0351,0.0352,0.0840,0f000041,0*ba253e89", "robot status", "#DUALANTENNAHEADINGA,USB3,0,46.0,FINESTEERING,2113,382033.500,02000000,d426,15824;SOL_COMPUTED,NARROW_INT,-1.000000000,147.532882690,-13.543701172,0.0,0.340999722,0.929950953,\"681H\",37,28,28,23,04,00,30,33*7a9ae75d", "robot status", "#INSPVAXA,USB3,0,46.0,FINESTEERING,2113,382033.550,02000000,471d,15824;INS_SOLUTION_GOOD,INS_RTKFIXED,37.37017952891,126.72086765613,9.9290,22.3000,-0.0002,0.0010,-0.0068,-0.554931524,-0.348428210,142.133743385,0.1520,0.1529,0.1414,0.0375,0.0376,0.0242,0.0351,0.0352,0.0840,0f000041,0*a4fb30e7", "robot status", "#DUALANTENNAHEADINGA,USB3,0,46.0,FINESTEERING,2113,382033.600,02000000,d426,15824;SOL_COMPUTED,NARROW_INT,-1.000000000,147.207748413,-13.984344482,0.0,0.341872275,0.930336773,\"681H\",37,29,29,24,04,00,30,33*8fbd8216", "robot status", "#INSPVAXA,USB3,0,46.0,FINESTEERING,2113,382033.650,02000000,471d,15824;INS_SOLUTION_GOOD,INS_RTKFIXED,37.37017948382,126.72086767106,9.9289,22.3000,-0.0394,0.0232,-0.0040,-0.563302760,-0.298058493,141.870858485,0.1520,0.1529,0.1414,0.0375,0.0376,0.0242,0.0351,0.0352,0.0840,0f000041,0*a37e698c", "robot status", "#DUALANTENNAHEADINGA,USB3,0,46.0,FINESTEERING,2113,382033.700,02000000,d426,15824;SOL_COMPUTED,NARROW_INT,-1.000000000,146.917007446,-13.644836426,0.0,0.342521280,0.932795286,\"681H\",37,29,29,24,04,00,30,33*6f572c3f", "robot status", "#INSPVAXA,USB3,0,46.0,FINESTEERING,2113,382033.750,02000000,471d,15824;INS_SOLUTION_GOOD,INS_RTKFIXED,37.37017938693,126.72086772727,9.9287,22.3000,-0.1084,0.0724,-0.0044,-0.538845302,-0.233690415,141.518364970,0.1520,0.1529,0.1414,0.0375,0.0376,0.0242,0.0351,0.0352,0.0840,0f000041,0*530c9730", "robot status", "#DUALANTENNAHEADINGA,USB3,0,46.0,FINESTEERING,2113,382033.800,02000000,d426,15824;SOL_COMPUTED,NARROW_INT,-1.000000000,146.546005249,-13.247344971,0.0,0.340983421,0.928570807,\"681H\",37,29,29,24,04,00,30,33*a9f60b5f", "robot status", "#INSPVAXA,USB3,0,46.0,FINESTEERING,2113,382033.850,02000000,471d,15824;INS_SOLUTION_GOOD,INS_RTKFIXED,37.37017924042,126.72086784072,9.9286,22.3000,-0.1500,0.1224,-0.0030,-0.561937166,-0.215991900,141.155580204,0.1520,0.1529,0.1414,0.0375,0.0376,0.0242,0.0351,0.0352,0.0840,0f000041,0*607dc084", "robot status", "#DUALANTENNAHEADINGA,USB3,0,46.0,FINESTEERING,2113,382033.900,02000000,d426,15824;SOL_COMPUTED,NARROW_INT,-1.000000000,146.414611816,-13.241760254,0.0,0.341605425,0.931110740,\"681H\",37,29,29,24,04,00,30,33*055d4c93", "robot status", "#INSPVAXA,USB3,0,46.0,FINESTEERING,2113,382033.950,02000000,471d,15824;INS_SOLUTION_GOOD,INS_RTKFIXED,37.37017906432,126.72086799717,9.9286,22.3000,-0.1693,0.1452,-0.0044,-0.543602734,-0.306257258,141.045154353,0.1520,0.1529,0.1414,0.0375,0.0376,0.0242,0.0351,0.0352,0.0840,0f000041,0*d3c5d385", "robot status", "#DUALANTENNAHEADINGA,USB3,0,46.0,FINESTEERING,2113,382034.000,02000000,d426,15824;SOL_COMPUTED,NARROW_INT,-1.000000000,146.478866577,-12.810150146,0.0,0.342516333,0.935827315,\"681H\",37,29,29,24,04,00,30,33*2ccadfdc", "robot status", "#INSPVAXA,USB3,0,45.5,FINESTEERING,2113,382034.050,02000000,471d,15824;INS_SOLUTION_GOOD,INS_RTKFIXED,37.37017888510,126.72086815559,9.9288,22.3000,-0.1648,0.1232,-0.0010,-0.585630516,-0.263647642,140.847537490,0.1543,0.1531,0.1427,0.0381,0.0381,0.0243,0.0352,0.0354,0.0847,0f000041,0*fe604449", "robot status", "#DUALANTENNAHEADINGA,USB3,0,45.5,FINESTEERING,2113,382034.100,02000000,d426,15824;SOL_COMPUTED,NARROW_INT,-1.000000000,146.156738281,-13.703491211,0.0,0.343589127,0.936918616,\"681H\",37,29,29,24,04,00,30,33*da03cdc1", "robot status", "#INSPVAXA,USB3,0,45.5,FINESTEERING,2113,382034.150,02000000,471d,15824;INS_SOLUTION_GOOD,INS_RTKFIXED,37.37017871550,126.72086829489,9.9279,22.3000,-0.1402,0.1187,-0.0056,-0.579919682,-0.246344639,140.606635849,0.1543,0.1531,0.1427,0.0381,0.0381,0.0243,0.0352,0.0354,0.0847,0f000041,0*67df8422", "robot status", "#DUALANTENNAHEADINGA,USB3,0,45.5,FINESTEERING,2113,382034.200,02000000,d426,15824;SOL_COMPUTED,NARROW_INT,-1.000000000,145.943847656,-13.405151367,0.0,0.342577010,0.935270369,\"681H\",37,29,29,24,04,00,30,33*b1543e0c", "robot status", "#INSPVAXA,USB3,0,45.5,FINESTEERING,2113,382034.250,02000000,471d,15824;INS_SOLUTION_GOOD,INS_RTKFIXED,37.37017856450,126.72086842716,9.9277,22.3000,-0.1308,0.1005,-0.0046,-0.533419520,-0.317264427,140.477287337,0.1543,0.1531,0.1427,0.0381,0.0381,0.0243,0.0352,0.0354,0.0847,0f000041,0*d17420c4", "robot status", "#DUALANTENNAHEADINGA,USB3,0,45.5,FINESTEERING,2113,382034.300,02000000,d426,15824;SOL_COMPUTED,NARROW_INT,-1.000000000,145.654525757,-13.427581787,0.0,0.342915505,0.938795328,\"681H\",37,29,29,24,04,00,30,33*9aa2385d", "robot status", "#INSPVAXA,USB3,0,45.5,FINESTEERING,2113,382034.350,02000000,471d,15824;INS_SOLUTION_GOOD,INS_RTKFIXED,37.37017843036,126.72086854331,9.9273,22.3000,-0.1042,0.0829,-0.0009,-0.521519207,-0.282443525,140.275408670,0.1543,0.1531,0.1427,0.0381,0.0381,0.0243,0.0352,0.0354,0.0847,0f000041,0*cec2228c", "robot status", "#DUALANTENNAHEADINGA,USB3,0,45.5,FINESTEERING,2113,382034.400,02000000,d426,15824;SOL_COMPUTED,NARROW_INT,-1.000000000,145.423385620,-13.754333496,0.0,0.345984697,0.948092937,\"681H\",37,29,29,24,04,00,30,33*c0282408", "robot status", "#INSPVAXA,USB3,0,45.5,FINESTEERING,2113,382034.450,02000000,471d,15824;INS_SOLUTION_GOOD,INS_RTKFIXED,37.37017830267,126.72086862272,9.9268,22.3000,-0.1128,0.0650,-0.0084,-0.398656374,-0.259682939,139.931798645,0.1543,0.1531,0.1427,0.0381,0.0381,0.0243,0.0352,0.0354,0.0847,0f000041,0*55e94dbb", "robot status", "#DUALANTENNAHEADINGA,USB3,0,45.5,FINESTEERING,2113,382034.500,02000000,d426,15824;SOL_COMPUTED,NARROW_INT,-1.000000000,144.879302979,-12.860168457,0.0,0.345901459,0.952228725,\"681H\",37,29,29,24,04,00,30,33*df6340d3", "robot status", "#INSPVAXA,USB3,0,45.5,FINESTEERING,2113,382034.550,02000000,471d,15824;INS_SOLUTION_GOOD,INS_RTKFIXED,37.37017817450,126.72086873161,9.9263,22.3000,-0.1117,0.1083,-0.0032,-0.398883944,-0.306674809,139.664814502,0.1543,0.1531,0.1427,0.0381,0.0381,0.0243,0.0352,0.0354,0.0847,0f000041,0*8e2a6893", "robot status", "#INSPVAXA,USB3,0,45.5,FINESTEERING,2113,382034.650,02000000,471d,15824;INS_SOLUTION_GOOD,INS_RTKFIXED,37.37017803343,126.72086885744,9.9258,22.3000,-0.1324,0.1088,-0.0052,-0.343949486,-0.326992443,139.549936239,0.1543,0.1531,0.1427,0.0381,0.0381,0.0243,0.0352,0.0354,0.0847,0f000041,0*eff8c5d9", "robot status", "#INSPVAXA,USB3,0,45.5,FINESTEERING,2113,382034.650,02000000,471d,15824;INS_SOLUTION_GOOD,INS_RTKFIXED,37.37017803343,126.72086885744,9.9258,22.3000,-0.1324,0.1088,-0.0052,-0.343949486,-0.326992443,139.549936239,0.1543,0.1531,0.1427,0.0381,0.0381,0.0243,0.0352,0.0354,0.0847,0f000041,0*eff8c5d9", "robot status", "#DUALANTENNAHEADINGA,USB3,0,45.5,FINESTEERING,2113,382034.700,02000000,d426,15824;SOL_COMPUTED,NARROW_INT,-1.000000000,144.732101440,-12.617797852,0.0,0.349006176,0.958688200,\"681H\",36,29,29,24,04,00,30,33*2f2aaad2", "robot status", "#INSPVAXA,USB3,0,45.5,FINESTEERING,2113,382034.750,02000000,471d,15824;INS_SOLUTION_GOOD,INS_RTKFIXED,37.37017788822,126.72086897686,9.9250,22.3000,-0.1324,0.0880,-0.0131,-0.314087302,-0.310188373,139.159395779,0.1543,0.1531,0.1427,0.0381,0.0381,0.0243,0.0352,0.0354,0.0847,0f000041,0*b3950d91", "robot status", "#DUALANTENNAHEADINGA,USB3,0,45.5,FINESTEERING,2113,382034.800,02000000,d426,15824;SOL_COMPUTED,NARROW_INT,-1.000000000,144.261596680,-12.579010010,0.0,0.352737516,0.968103468,\"681H\",37,29,29,24,04,00,30,33*b72dc266", "robot status", "#INSPVAXA,USB3,0,45.5,FINESTEERING,2113,382034.850,02000000,471d,15824;INS_SOLUTION_GOOD,INS_RTKFIXED,37.37017774971,126.72086908581,9.9244,22.3000,-0.1101,0.1034,-0.0045,-0.260270682,-0.286911105,138.938494595,0.1543,0.1531,0.1427,0.0381,0.0381,0.0243,0.0352,0.0354,0.0847,0f000041,0*abe6ae4d", "robot status", "#DUALANTENNAHEADINGA,USB3,0,45.5,FINESTEERING,2113,382034.900,02000000,d426,15824;SOL_COMPUTED,NARROW_INT,-1.000000000,144.158706665,-12.778289795,0.0,0.352949679,0.966478884,\"681H\",37,29,29,24,04,00,30,33*9f1f1cec", "robot status", "#INSPVAXA,USB3,0,45.5,FINESTEERING,2113,382034.950,02000000,471d,15824;INS_SOLUTION_GOOD,INS_RTKFIXED,37.37017761764,126.72086921709,9.9238,22.3000,-0.1225,0.1099,-0.0126,-0.363570148,-0.293083747,138.780967944,0.1543,0.1531,0.1427,0.0381,0.0381,0.0243,0.0352,0.0354,0.0847,0f000041,0*00dbf10c", "robot status", "#DUALANTENNAHEADINGA,USB3,0,45.5,FINESTEERING,2113,382035.000,02000000,d426,15824;SOL_COMPUTED,NARROW_INT,-1.000000000,143.904144287,-12.943817139,0.0,0.351785988,0.961377859,\"681H\",36,28,28,23,04,00,30,33*10795ecd", "robot status", "#INSPVAXA,USB3,0,45.5,FINESTEERING,2113,382035.050,02000000,471d,15824;INS_SOLUTION_GOOD,INS_RTKFIXED,37.37017748072,126.72086934651,9.9231,22.3000,-0.1199,0.0996,-0.0082,-0.451427101,-0.215956162,138.526690049,0.1567,0.1517,0.1436,0.0388,0.0381,0.0245,0.0352,0.0356,0.0853,0f000041,0*6e62362d", "robot status", "#DUALANTENNAHEADINGA,USB3,0,45.5,FINESTEERING,2113,382035.100,02000000,d426,15824;SOL_COMPUTED,NARROW_INT,-1.000000000,143.487380981,-13.028076172,0.0,0.351447284,0.960495532,\"681H\",36,27,27,22,04,00,30,33*07437053", "robot status", "#INSPVAXA,USB3,0,46.0,FINESTEERING,2113,382035.150,02000000,471d,15824;INS_SOLUTION_GOOD,INS_RTKFIXED,37.37017733641,126.72086945761,9.9227,22.3000,-0.1262,0.0863,-0.0142,-0.427571759,-0.205490811,138.176706965,0.1567,0.1517,0.1436,0.0388,0.0381,0.0245,0.0352,0.0356,0.0853,0f000041,0*4bbe4f53", "robot status", "#INSPVAXA,USB3,0,46.0,FINESTEERING,2113,382035.250,02000000,471d,15824;INS_SOLUTION_GOOD,INS_RTKFIXED,37.37017720050,126.72086957388,9.9227,22.3000,-0.1109,0.0983,-0.0087,-0.444634053,-0.283405777,137.883234714,0.1567,0.1517,0.1436,0.0388,0.0381,0.0245,0.0352,0.0356,0.0853,0f000041,0*c04cf8ae", "robot status", "#INSPVAXA,USB3,0,46.0,FINESTEERING,2113,382035.250,02000000,471d,15824;INS_SOLUTION_GOOD,INS_RTKFIXED,37.37017720050,126.72086957388,9.9227,22.3000,-0.1109,0.0983,-0.0087,-0.444634053,-0.283405777,137.883234714,0.1567,0.1517,0.1436,0.0388,0.0381,0.0245,0.0352,0.0356,0.0853,0f000041,0*c04cf8ae", "robot status", "#DUALANTENNAHEADINGA,USB3,0,46.0,FINESTEERING,2113,382035.300,02000000,d426,15824;SOL_COMPUTED,NARROW_INT,-1.000000000,142.740325928,-13.488647461,0.0,0.350875437,0.954844952,\"681H\",36,28,28,22,04,00,30,33*53f7949d", "robot status", "#INSPVAXA,USB3,0,46.0,FINESTEERING,2113,382035.350,02000000,471d,15824;INS_SOLUTION_GOOD,INS_RTKFIXED,37.37017707535,126.72086969032,9.9228,22.3000,-0.1051,0.0893,-0.0100,-0.516217387,-0.226496732,137.702360311,0.1567,0.1517,0.1436,0.0388,0.0381,0.0245,0.0352,0.0356,0.0853,0f000041,0*fcb41b07", "robot status", "#INSPVAXA,USB3,0,46.0,FINESTEERING,2113,382035.450,02000000,471d,15824;INS_SOLUTION_GOOD,INS_RTKFIXED,37.37017695300,126.72086978371,9.9228,22.3000,-0.1054,0.0661,-0.0077,-0.512684815,-0.185503590,137.217109794,0.1567,0.1517,0.1436,0.0388,0.0381,0.0245,0.0352,0.0356,0.0853,0f000041,0*cfec679e", "robot status", "#INSPVAXA,USB3,0,46.0,FINESTEERING,2113,382035.500,02000000,471d,15824;INS_SOLUTION_GOOD,INS_RTKFIXED,37.37017688977,126.72086982893,9.9228,22.3000,-0.1058,0.0803,-0.0108,-0.507749021,-0.185252142,136.999229251,0.1567,0.1517,0.1436,0.0388,0.0381,0.0245,0.0352,0.0356,0.0853,0f000041,0*515e313e", "robot status", "#DUALANTENNAHEADINGA,USB3,0,46.0,FINESTEERING,2113,382035.500,02000000,d426,15824;SOL_COMPUTED,NARROW_INT,-1.000000000,142.351409912,-13.256134033,0.0,0.347597092,0.947488010,\"681H\",36,28,28,22,04,00,30,33*353c45ef", "robot status", "#INSPVAXA,USB3,0,46.0,FINESTEERING,2113,382035.550,02000000,471d,15824;INS_SOLUTION_GOOD,INS_RTKFIXED,37.37017682778,126.72086988324,9.9228,22.3000,-0.1093,0.0985,-0.0082,-0.503569323,-0.226773130,136.854020668,0.1567,0.1517,0.1436,0.0388,0.0381,0.0245,0.0352,0.0356,0.0853,0f000041,0*8bf81598", "robot status", "#DUALANTENNAHEADINGA,USB3,0,46.0,FINESTEERING,2113,382035.600,02000000,d426,15824;SOL_COMPUTED,NARROW_INT,-1.000000000,142.134765625,-13.774871826,0.0,0.348382890,0.947803617,\"681H\",35,28,28,22,04,00,30,33*899876aa", "robot status", "#INSPVAXA,USB3,0,46.0,FINESTEERING,2113,382035.700,02000000,471d,15824;INS_SOLUTION_GOOD,INS_RTKFIXED,37.37017662012,126.72087008196,9.9227,22.3000,-0.1326,0.1111,-0.0054,-0.505647508,-0.267464720,136.492237328,0.1567,0.1517,0.1436,0.0388,0.0381,0.0245,0.0352,0.0356,0.0853,0f000041,0*1d09d545", "robot status", "#DUALANTENNAHEADINGA,USB3,0,46.0,FINESTEERING,2113,382035.700,02000000,d426,15824;SOL_COMPUTED,NARROW_INT,-1.000000000,142.166244507,-12.547790527,0.0,0.347424209,0.947535038,\"681H\",35,28,28,22,04,00,30,33*424e8164", "robot status", "#INSPVAXA,USB3,0,46.0,FINESTEERING,2113,382035.750,02000000,471d,15824;INS_SOLUTION_GOOD,INS_RTKFIXED,37.37017654621,126.72087014548,9.9229,22.3000,-0.1356,0.1021,-0.0051,-0.507130959,-0.242924673,136.308397009,0.1567,0.1517,0.1436,0.0388,0.0381,0.0245,0.0352,0.0356,0.0853,0f000041,0*6eefa77b", "robot status", "#INSPVAXA,USB3,0,46.0,FINESTEERING,2113,382035.850,02000000,471d,15824;INS_SOLUTION_GOOD,INS_RTKFIXED,37.37017640209,126.72087027126,9.9227,22.3000,-0.1216,0.1139,-0.0060,-0.513341100,-0.258435964,135.923267121,0.1567,0.1517,0.1436,0.0388,0.0381,0.0245,0.0352,0.0356,0.0853,0f000041,0*251a5cf7", "robot status", "#INSPVAXA,USB3,0,46.0,FINESTEERING,2113,382035.900,02000000,471d,15824;INS_SOLUTION_GOOD,INS_RTKFIXED,37.37017633461,126.72087034120,9.9228,22.3000,-0.1245,0.1214,-0.0054,-0.496872782,-0.348410223,135.820160504,0.1567,0.1517,0.1436,0.0388,0.0381,0.0245,0.0352,0.0356,0.0853,0f000041,0*5331177e", "robot status", "#DUALANTENNAHEADINGA,USB3,0,46.0,FINESTEERING,2113,382035.900,02000000,d426,15824;SOL_COMPUTED,NARROW_INT,-1.000000000,141.341598511,-12.057983398,0.0,0.348134905,0.950228930,\"681H\",35,28,28,22,04,00,30,33*385dd9f5", "robot status", "#INSPVAXA,USB3,0,46.0,FINESTEERING,2113,382035.950,02000000,471d,15824;INS_SOLUTION_GOOD,INS_RTKFIXED,37.37017626407,126.72087041360,9.9225,22.3000,-0.1322,0.1244,-0.0152,-0.481843137,-0.349918836,135.771901116,0.1567,0.1517,0.1436,0.0388,0.0381,0.0245,0.0352,0.0356,0.0853,0f000041,0*9b4964c3", "robot status", "#INSPVAXA,USB3,0,46.0,FINESTEERING,2113,382036.050,02000000,471d,15824;INS_SOLUTION_GOOD,INS_RTKFIXED,37.37017611225,126.72087056975,9.9221,22.3000,-0.1504,0.1320,-0.0160,-0.431775707,-0.399331657,135.605996277,0.1594,0.1485,0.1442,0.0395,0.0379,0.0246,0.0351,0.0357,0.0860,0f000041,0*ba791927", "robot status", "#INSPVAXA,USB3,0,43.0,FINESTEERING,2113,382036.100,02000000,471d,15824;INS_SOLUTION_GOOD,INS_RTKFIXED,37.37017602832,126.72087064507,9.9221,22.3000,-0.1541,0.1252,-0.0010,-0.418006820,-0.383555922,135.414734649,0.1594,0.1485,0.1442,0.0395,0.0379,0.0246,0.0351,0.0357,0.0860,0f000041,0*fc53c8f2", "robot status", "#DUALANTENNAHEADINGA,USB3,0,43.0,FINESTEERING,2113,382036.100,02000000,d426,15824;SOL_COMPUTED,NARROW_INT,-1.000000000,140.735229492,-12.557037354,0.0,0.351257235,0.952364743,\"681H\",36,28,28,22,04,00,30,33*85bb44bd", "robot status", "#INSPVAXA,USB3,0,43.0,FINESTEERING,2113,382036.150,02000000,471d,15824;INS_SOLUTION_GOOD,INS_RTKFIXED,37.37017594700,126.72087072053,9.9219,22.3000,-0.1477,0.1332,-0.0185,-0.396978318,-0.336780700,135.308765379,0.1594,0.1485,0.1442,0.0395,0.0379,0.0246,0.0351,0.0357,0.0860,0f000041,0*adc00bc6", "robot status", "#DUALANTENNAHEADINGA,USB3,0,43.0,FINESTEERING,2113,382036.200,02000000,d426,15824;SOL_COMPUTED,NARROW_INT,-1.000000000,140.484741211,-12.597045898,0.0,0.355971217,0.962328553,\"681H\",36,27,27,22,04,00,30,33*22095ba9", "robot status", "#INSPVAXA,USB3,0,43.0,FINESTEERING,2113,382036.300,02000000,471d,15824;INS_SOLUTION_GOOD,INS_RTKFIXED,37.37017573070,126.72087095509,9.9220,22.3000,-0.1237,0.1136,-0.0071,-0.384020682,-0.385100724,135.100336300,0.1594,0.1485,0.1442,0.0395,0.0379,0.0246,0.0351,0.0357,0.0860,0f000041,0*219b2090", "robot status", "#INSPVAXA,USB3,0,43.0,FINESTEERING,2113,382036.350,02000000,471d,15824;INS_SOLUTION_GOOD,INS_RTKFIXED,37.37017566444,126.72087101910,9.9217,22.3000,-0.1154,0.1037,-0.0130,-0.374805893,-0.378924336,135.009446233,0.1594,0.1485,0.1442,0.0395,0.0379,0.0246,0.0351,0.0357,0.0860,0f000041,0*3b0f3cc7", "robot status", "#INSPVAXA,USB3,0,43.0,FINESTEERING,2113,382036.350,02000000,471d,15824;INS_SOLUTION_GOOD,INS_RTKFIXED,37.37017566444,126.72087101910,9.9217,22.3000,-0.1154,0.1037,-0.0130,-0.374805893,-0.378924336,135.009446233,0.1594,0.1485,0.1442,0.0395,0.0379,0.0246,0.0351,0.0357,0.0860,0f000041,0*3b0f3cc7", "robot status", "#DUALANTENNAHEADINGA,USB3,0,43.0,FINESTEERING,2113,382036.400,02000000,d426,15824;SOL_COMPUTED,NARROW_INT,-1.000000000,140.298324585,-12.188201904,0.0,0.357363671,0.965269744,\"681H\",36,27,27,22,04,00,30,33*55f53c89", "robot status", "#INSPVAXA,USB3,0,43.0,FINESTEERING,2113,382036.500,02000000,471d,15824;INS_SOLUTION_GOOD,INS_RTKFIXED,37.37017546895,126.72087119787,9.9215,22.3000,-0.1198,0.1117,-0.0059,-0.305855333,-0.341639681,134.583793155,0.1594,0.1485,0.1442,0.0395,0.0379,0.0246,0.0351,0.0357,0.0860,0f000041,0*300d0d12", "robot status", "#INSPVAXA,USB3,0,43.0,FINESTEERING,2113,382036.550,02000000,471d,15824;INS_SOLUTION_GOOD,INS_RTKFIXED,37.37017540244,126.72087126841,9.9214,22.3000,-0.1228,0.1276,-0.0098,-0.291202196,-0.382468099,134.516010395,0.1594,0.1485,0.1442,0.0395,0.0379,0.0246,0.0351,0.0357,0.0860,0f000041,0*414c82b6", "robot status", "#INSPVAXA,USB3,0,43.0,FINESTEERING,2113,382036.550,02000000,471d,15824;INS_SOLUTION_GOOD,INS_RTKFIXED,37.37017540244,126.72087126841,9.9214,22.3000,-0.1228,0.1276,-0.0098,-0.291202196,-0.382468099,134.516010395,0.1594,0.1485,0.1442,0.0395,0.0379,0.0246,0.0351,0.0357,0.0860,0f000041,0*414c82b6", "robot status", "#DUALANTENNAHEADINGA,USB3,0,43.0,FINESTEERING,2113,382036.600,02000000,d426,15824;SOL_COMPUTED,NARROW_INT,-1.000000000,140.120742798,-12.776428223,0.0,0.364644855,0.976225138,\"681H\",36,27,27,21,04,00,30,33*18b75c25", "robot status", "#INSPVAXA,USB3,0,43.0,FINESTEERING,2113,382036.700,02000000,471d,15824;INS_SOLUTION_GOOD,INS_RTKFIXED,37.37017519599,126.72087149967,9.9210,22.3000,-0.1211,0.1218,-0.0071,-0.341525472,-0.423184652,134.209569095,0.1594,0.1485,0.1442,0.0395,0.0379,0.0246,0.0351,0.0357,0.0860,0f000041,0*95a53141", "robot status", "#INSPVAXA,USB3,0,43.0,FINESTEERING,2113,382036.750,02000000,471d,15824;INS_SOLUTION_GOOD,INS_RTKFIXED,37.37017512870,126.72087156444,9.9209,22.3000,-0.1256,0.0996,-0.0139,-0.307522001,-0.418777977,134.029836966,0.1594,0.1485,0.1442,0.0395,0.0379,0.0246,0.0351,0.0357,0.0860,0f000041,0*2ea19536", "robot status", "#INSPVAXA,USB3,0,43.0,FINESTEERING,2113,382036.750,02000000,471d,15824;INS_SOLUTION_GOOD,INS_RTKFIXED,37.37017512870,126.72087156444,9.9209,22.3000,-0.1256,0.0996,-0.0139,-0.307522001,-0.418777977,134.029836966,0.1594,0.1485,0.1442,0.0395,0.0379,0.0246,0.0351,0.0357,0.0860,0f000041,0*2ea19536", "robot status", "#INSPVAXA,USB3,0,43.0,FINESTEERING,2113,382036.850,02000000,471d,15824;INS_SOLUTION_GOOD,INS_RTKFIXED,37.37017499448,126.72087168018,9.9206,22.3000,-0.1143,0.1060,0.0015,-0.175648547,-0.457552379,133.717191746,0.1594,0.1485,0.1442,0.0395,0.0379,0.0246,0.0351,0.0357,0.0860,0f000041,0*76572a5a", "robot status", "#INSPVAXA,USB3,0,43.0,FINESTEERING,2113,382036.900,02000000,471d,15824;INS_SOLUTION_GOOD,INS_RTKFIXED,37.37017493280,126.72087174571,9.9207,22.3000,-0.1112,0.1180,-0.0086,-0.119865949,-0.529113606,133.656233636,0.1594,0.1485,0.1442,0.0395,0.0379,0.0246,0.0351,0.0357,0.0860,0f000041,0*59f1f104", "robot status", "#INSPVAXA,USB3,0,43.0,FINESTEERING,2113,382036.950,02000000,471d,15824;INS_SOLUTION_GOOD,INS_RTKFIXED,37.37017487150,126.72087181550,9.9207,22.3000,-0.1099,0.1208,-0.0046,-0.122254097,-0.540921596,133.619626258,0.1594,0.1485,0.1442,0.0395,0.0379,0.0246,0.0351,0.0357,0.0860,0f000041,0*ba11facd", "robot status", "#INSPVAXA,USB3,0,43.0,FINESTEERING,2113,382037.000,02000000,471d,15824;INS_SOLUTION_GOOD,INS_RTKFIXED,37.37017481173,126.72087188339,9.9208,22.3000,-0.1061,0.1122,-0.0074,-0.149066915,-0.553505756,133.474230666,0.1594,0.1485,0.1442,0.0395,0.0379,0.0246,0.0351,0.0357,0.0860,0f000041,0*569baee2", "robot status", "#INSPVAXA,USB3,0,43.0,FINESTEERING,2113,382037.050,02000000,471d,15824;INS_SOLUTION_GOOD,INS_RTKFIXED,37.37017475032,126.72087194377,9.9207,22.3000,-0.1063,0.0931,-0.0081,-0.183412825,-0.545303380,133.241776623,0.1622,0.1450,0.1448,0.0402,0.0376,0.0248,0.0349,0.0357,0.0867,0f000041,0*08d98314", "robot status", "#INSPVAXA,USB3,0,45.5,FINESTEERING,2113,382037.100,02000000,471d,15824;INS_SOLUTION_GOOD,INS_RTKFIXED,37.37017468694,126.72087199527,9.9205,22.3000,-0.1059,0.0819,-0.0115,-0.186336891,-0.527372034,132.951029256,0.1622,0.1450,0.1448,0.0402,0.0376,0.0248,0.0349,0.0357,0.0867,0f000041,0*37a253e8", "robot status", "#INSPVAXA,USB3,0,45.5,FINESTEERING,2113,382037.150,02000000,471d,15824;INS_SOLUTION_GOOD,INS_RTKFIXED,37.37017462526,126.72087204414,9.9201,22.3000,-0.1006,0.0812,-0.0073,-0.176565743,-0.482234995,132.695681690,0.1622,0.1450,0.1448,0.0402,0.0376,0.0248,0.0349,0.0357,0.0867,0f000041,0*86f79269", "robot status", "#INSPVAXA,USB3,0,45.5,FINESTEERING,2113,382037.200,02000000,471d,15824;INS_SOLUTION_GOOD,INS_RTKFIXED,37.37017456813,126.72087209313,9.9202,22.3000,-0.0937,0.0818,-0.0007,-0.155528665,-0.553727183,132.470354491,0.1622,0.1450,0.1448,0.0402,0.0376,0.0248,0.0349,0.0357,0.0867,0f000041,0*73c46839", "robot status", "#INSPVAXA,USB3,0,45.5,FINESTEERING,2113,382037.250,02000000,471d,15824;INS_SOLUTION_GOOD,INS_RTKFIXED,37.37017451159,126.72087213871,9.9202,22.3000,-0.0915,0.0743,-0.0055,-0.136766507,-0.566468560,132.242584427,0.1622,0.1450,0.1448,0.0402,0.0376,0.0248,0.0349,0.0357,0.0867,0f000041,0*a43f99e4", "robot status", "#INSPVAXA,USB3,0,45.5,FINESTEERING,2113,382037.300,02000000,471d,15824;INS_SOLUTION_GOOD,INS_RTKFIXED,37.37017445556,126.72087218406,9.9203,22.3000,-0.0960,0.0811,0.0002,-0.090493119,-0.568676122,132.014930352,0.1622,0.1450,0.1448,0.0402,0.0376,0.0248,0.0349,0.0357,0.0867,0f000041,0*5f745cee", "robot status", "#INSPVAXA,USB3,0,45.5,FINESTEERING,2113,382037.350,02000000,471d,15824;INS_SOLUTION_GOOD,INS_RTKFIXED,37.37017440004,126.72087223491,9.9204,22.3000,-0.0910,0.0900,-0.0054,-0.089033758,-0.533890492,131.824235174,0.1622,0.1450,0.1448,0.0402,0.0376,0.0248,0.0349,0.0357,0.0867,0f000041,0*ade87302", "robot status", "#INSPVAXA,USB3,0,45.5,FINESTEERING,2113,382037.400,02000000,471d,15824;INS_SOLUTION_GOOD,INS_RTKFIXED,37.37017434592,126.72087228439,9.9203,22.3000,-0.0932,0.0746,-0.0142,-0.141491167,-0.485624758,131.565470396,0.1622,0.1450,0.1448,0.0402,0.0376,0.0248,0.0349,0.0357,0.0867,0f000041,0*e5a8b6e9", "robot status", "#INSPVAXA,USB3,0,45.5,FINESTEERING,2113,382037.450,02000000,471d,15824;INS_SOLUTION_GOOD,INS_RTKFIXED,37.37017428589,126.72087232621,9.9201,22.3000,-0.1121,0.0652,-0.0147,-0.185891346,-0.366709082,131.220853502,0.1622,0.1450,0.1448,0.0402,0.0376,0.0248,0.0349,0.0357,0.0867,0f000041,0*ebee27fa", "robot status", "#INSPVAXA,USB3,0,45.5,FINESTEERING,2113,382037.500,02000000,471d,15824;INS_SOLUTION_GOOD,INS_RTKFIXED,37.37017422140,126.72087236909,9.9203,22.3000,-0.1141,0.0798,-0.0010,-0.101055560,-0.366673628,130.865435791,0.1622,0.1450,0.1448,0.0402,0.0376,0.0248,0.0349,0.0357,0.0867,0f000041,0*945da2a9", "robot status", "#INSPVAXA,USB3,0,45.5,FINESTEERING,2113,382037.550,02000000,471d,15824;INS_SOLUTION_GOOD,INS_RTKFIXED,37.37017415612,126.72087242490,9.9202,22.3000,-0.1186,0.1091,-0.0136,-0.138663111,-0.385854826,130.613680441,0.1622,0.1450,0.1448,0.0402,0.0376,0.0248,0.0349,0.0357,0.0867,0f000041,0*3790431d", "robot status", "#INSPVAXA,USB3,0,45.5,FINESTEERING,2113,382037.600,02000000,471d,15824;INS_SOLUTION_GOOD,INS_RTKFIXED,37.37017409086,126.72087249341,9.9201,22.3000,-0.1188,0.1262,-0.0040,-0.093162398,-0.435999911,130.327771161,0.1622,0.1450,0.1448,0.0402,0.0376,0.0248,0.0349,0.0357,0.0867,0f000041,0*9293c3cc", "robot status", "#INSPVAXA,USB3,0,45.5,FINESTEERING,2113,382037.650,02000000,471d,15824;INS_SOLUTION_GOOD,INS_RTKFIXED,37.37017402070,126.72087256588,9.9200,22.3000,-0.1285,0.1205,-0.0140,-0.122134356,-0.469834445,130.159602799,0.1622,0.1450,0.1448,0.0402,0.0376,0.0248,0.0349,0.0357,0.0867,0f000041,0*0880db8d", "robot status", "#INSPVAXA,USB3,0,45.5,FINESTEERING,2113,382037.700,02000000,471d,15824;INS_SOLUTION_GOOD,INS_RTKFIXED,37.37017395121,126.72087263441,9.9196,22.3000,-0.1227,0.1189,-0.0082,-0.054100785,-0.450527608,129.981031322,0.1622,0.1450,0.1448,0.0402,0.0376,0.0248,0.0349,0.0357,0.0867,0f000041,0*d599605b", "robot status", "#INSPVAXA,USB3,0,45.5,FINESTEERING,2113,382037.750,02000000,471d,15824;INS_SOLUTION_GOOD,INS_RTKFIXED,37.37017388961,126.72087270548,9.9197,22.3000,-0.0982,0.1240,-0.0037,-0.105032056,-0.407338792,129.808393019,0.1622,0.1450,0.1448,0.0402,0.0376,0.0248,0.0349,0.0357,0.0867,0f000041,0*35334fae", "robot status", "#INSPVAXA,USB3,0,45.5,FINESTEERING,2113,382037.800,02000000,471d,15824;INS_SOLUTION_GOOD,INS_RTKFIXED,37.37017383404,126.72087277135,9.9193,22.3000,-0.0945,0.0997,-0.0132,-0.158440926,-0.418813709,129.537462978,0.1622,0.1450,0.1448,0.0402,0.0376,0.0248,0.0349,0.0357,0.0867,0f000041,0*a594d64d", "robot status", "#INSPVAXA,USB3,0,45.5,FINESTEERING,2113,382037.850,02000000,471d,15824;INS_SOLUTION_GOOD,INS_RTKFIXED,37.37017377604,126.72087282497,9.9194,22.3000,-0.1017,0.0836,-0.0066,-0.145595047,-0.397399259,129.308058409,0.1622,0.1450,0.1448,0.0402,0.0376,0.0248,0.0349,0.0357,0.0867,0f000041,0*9ba3960d", "robot status", "#DUALANTENNAHEADINGA,USB3,0,45.5,FINESTEERING,2113,382037.900,02000000,d426,15824;SOL_COMPUTED,NARROW_INT,-1.000000000,133.748184204,-14.352416992,0.0,0.369591892,0.942851245,\"681H\",37,29,29,21,04,00,30,33*2be12134", "robot status", "#INSPVAXA,USB3,0,45.5,FINESTEERING,2113,382037.950,02000000,471d,15824;INS_SOLUTION_GOOD,INS_RTKFIXED,37.37017366182,126.72087293423,9.9190,22.3000,-0.1015,0.1069,-0.0118,-0.085374161,-0.412975524,128.964153610,0.1622,0.1450,0.1448,0.0402,0.0376,0.0248,0.0349,0.0357,0.0867,0f000041,0*d7d9e099", "robot status", "#INSPVAXA,USB3,0,45.5,FINESTEERING,2113,382038.000,02000000,471d,15824;INS_SOLUTION_GOOD,INS_RTKFIXED,37.37017360350,126.72087299570,9.9187,22.3000,-0.1084,0.1056,-0.0094,-0.044012011,-0.422366305,128.743881766,0.1622,0.1450,0.1448,0.0402,0.0376,0.0248,0.0349,0.0357,0.0867,0f000041,0*a17e0a0e", "robot status", "#INSPVAXA,USB3,0,44.5,FINESTEERING,2113,382038.050,02000000,471d,15824;INS_SOLUTION_GOOD,INS_RTKFIXED,37.37017354069,126.72087305769,9.9183,22.3000,-0.1073,0.1045,-0.0079,0.018350397,-0.406160875,128.548769137,0.1652,0.1385,0.1451,0.0408,0.0366,0.0249,0.0347,0.0360,0.0874,0f000041,0*48a78d6b", "robot status", "#DUALANTENNAHEADINGA,USB3,0,44.5,FINESTEERING,2113,382038.100,02000000,d426,15824;SOL_COMPUTED,NARROW_INT,-1.000000000,132.982055664,-14.845703125,0.0,0.374608010,0.943178952,\"681H\",37,29,29,21,04,00,30,33*db169fd3", "robot status", "#INSPVAXA,USB3,0,44.5,FINESTEERING,2113,382038.150,02000000,471d,15824;INS_SOLUTION_GOOD,INS_RTKFIXED,37.37017342162,126.72087318312,9.9186,22.3000,-0.0954,0.0950,-0.0146,-0.000818494,-0.369424525,128.075434167,0.1652,0.1385,0.1451,0.0408,0.0366,0.0249,0.0347,0.0360,0.0874,0f000041,0*658a76dc", "robot status", "#INSPVAXA,USB3,0,44.5,FINESTEERING,2113,382038.200,02000000,471d,15824;INS_SOLUTION_GOOD,INS_RTKFIXED,37.37017336427,126.72087323705,9.9186,22.3000,-0.0975,0.0851,0.0015,0.021030805,-0.372529253,127.796387907,0.1652,0.1385,0.1451,0.0408,0.0366,0.0249,0.0347,0.0360,0.0874,0f000041,0*9c11a226", "robot status", "#INSPVAXA,USB3,0,44.5,FINESTEERING,2113,382038.250,02000000,471d,15824;INS_SOLUTION_GOOD,INS_RTKFIXED,37.37017330203,126.72087328993,9.9186,22.3000,-0.1062,0.0880,-0.0106,0.070740995,-0.401140926,127.546780444,0.1652,0.1385,0.1451,0.0408,0.0366,0.0249,0.0347,0.0360,0.0874,0f000041,0*288102bb", "robot status", "#DUALANTENNAHEADINGA,USB3,0,44.5,FINESTEERING,2113,382038.300,02000000,d426,15824;SOL_COMPUTED,NARROW_INT,-1.000000000,131.856643677,-14.958892822,0.0,0.375133634,0.935270488,\"681H\",37,28,28,22,04,00,30,33*372a2756", "robot status", "#INSPVAXA,USB3,0,44.5,FINESTEERING,2113,382038.350,02000000,471d,15824;INS_SOLUTION_GOOD,INS_RTKFIXED,37.37017317724,126.72087340884,9.9187,22.3000,-0.1045,0.1126,-0.0126,0.205985057,-0.433585857,127.099263383,0.1652,0.1385,0.1451,0.0408,0.0366,0.0249,0.0347,0.0360,0.0874,0f000041,0*989d35df", "robot status", "#INSPVAXA,USB3,0,44.5,FINESTEERING,2113,382038.400,02000000,471d,15824;INS_SOLUTION_GOOD,INS_RTKFIXED,37.37017311852,126.72087347763,9.9186,22.3000,-0.0931,0.1173,-0.0039,0.235960639,-0.440283042,126.992343180,0.1652,0.1385,0.1451,0.0408,0.0366,0.0249,0.0347,0.0360,0.0874,0f000041,0*a8303163", "robot status", "#INSPVAXA,USB3,0,44.5,FINESTEERING,2113,382038.450,02000000,471d,15824;INS_SOLUTION_GOOD,INS_RTKFIXED,37.37017306723,126.72087354439,9.9188,22.3000,-0.0754,0.1075,-0.0046,0.220974745,-0.440106435,126.958200547,0.1652,0.1385,0.1451,0.0408,0.0366,0.0249,0.0347,0.0360,0.0874,0f000041,0*f332e25c", "robot status", "#DUALANTENNAHEADINGA,USB3,0,44.5,FINESTEERING,2113,382038.500,02000000,d426,15824;SOL_COMPUTED,NARROW_INT,-1.000000000,131.791564941,-13.635559082,0.0,0.375162244,0.940676570,\"681H\",37,28,28,22,04,00,30,33*f3e89b6f", "robot status", "#INSPVAXA,USB3,0,44.5,FINESTEERING,2113,382038.550,02000000,471d,15824;INS_SOLUTION_GOOD,INS_RTKFIXED,37.37017299767,126.72087362423,9.9187,22.3000,-0.0114,0.0229,-0.0046,0.226922561,-0.493761898,127.488517855,0.1652,0.1385,0.1451,0.0408,0.0366,0.0249,0.0347,0.0360,0.0874,0f000041,0*5d5dac61", "robot status", "#INSPVAXA,USB3,0,44.5,FINESTEERING,2113,382038.600,02000000,471d,15824;INS_SOLUTION_GOOD,INS_RTKFIXED,37.37017298716,126.72087362893,9.9185,22.3000,0.0229,-0.0187,-0.0137,0.210471735,-0.489646969,127.479239030,0.1652,0.1385,0.1451,0.0408,0.0366,0.0249,0.0347,0.0360,0.0874,0f000041,0*a79fb506", "robot status", "#INSPVAXA,USB3,0,44.5,FINESTEERING,2113,382038.650,02000000,471d,15824;INS_SOLUTION_GOOD,INS_RTKFIXED,37.37017298602,126.72087361235,9.9184,22.3000,0.0400,-0.0521,-0.0085,0.218299649,-0.459276579,127.263496377,0.1652,0.1385,0.1451,0.0408,0.0366,0.0249,0.0347,0.0360,0.0874,0f000041,0*578d5b72", "robot status", "#DUALANTENNAHEADINGA,USB3,0,44.5,FINESTEERING,2113,382038.700,02000000,d426,15824;SOL_COMPUTED,NARROW_INT,-1.000000000,132.110488892,-13.338256836,0.0,0.380160600,0.952131987,\"681H\",37,28,28,21,04,00,30,33*dec645dd", "robot status", "#INSPVAXA,USB3,0,44.5,FINESTEERING,2113,382038.750,02000000,471d,15824;INS_SOLUTION_GOOD,INS_RTKFIXED,37.37017301524,126.72087352273,9.9181,22.3000,0.0869,-0.1187,-0.0100,0.250060195,-0.512328301,127.462726059,0.1652,0.1385,0.1451,0.0408,0.0366,0.0249,0.0347,0.0360,0.0874,0f000041,0*4523ef4d", "robot status", "#INSPVAXA,USB3,0,44.5,FINESTEERING,2113,382038.800,02000000,471d,15824;INS_SOLUTION_GOOD,INS_RTKFIXED,37.37017304934,126.72087345003,9.9179,22.3000,0.1217,-0.1492,-0.0062,0.287670797,-0.539861381,127.317267323,0.1652,0.1385,0.1451,0.0408,0.0366,0.0249,0.0347,0.0360,0.0874,0f000041,0*0fcdda23", "robot status", "#INSPVAXA,USB3,0,44.5,FINESTEERING,2113,382038.850,02000000,471d,15824;INS_SOLUTION_GOOD,INS_RTKFIXED,37.37017309614,126.72087335661,9.9179,22.3000,0.1532,-0.1940,-0.0096,0.252126489,-0.559872136,127.280462060,0.1652,0.1385,0.1451,0.0408,0.0366,0.0249,0.0347,0.0360,0.0874,0f000041,0*f373c1d6", "robot status", "#DUALANTENNAHEADINGA,USB3,0,44.5,FINESTEERING,2113,382038.900,02000000,d426,15824;SOL_COMPUTED,NARROW_INT,-1.000000000,131.914276123,-15.260711670,0.0,0.379344344,0.944019556,\"681H\",37,28,28,21,04,00,30,33*abf7e7ac", "robot status", "#INSPVAXA,USB3,0,44.5,FINESTEERING,2113,382038.950,02000000,471d,15824;INS_SOLUTION_GOOD,INS_RTKFIXED,37.37017324351,126.72087309140,9.9172,22.3000,0.2291,-0.2865,-0.0108,0.132420933,-0.616735917,127.142439043,0.1652,0.1385,0.1451,0.0408,0.0366,0.0249,0.0347,0.0360,0.0874,0f000041,0*c7b4d67c", "robot status", "#DUALANTENNAHEADINGA,USB3,0,44.5,FINESTEERING,2113,382039.000,02000000,d426,15824;SOL_COMPUTED,NARROW_INT,-1.000000000,131.589553833,-15.212341309,0.0,0.379837811,0.945539713,\"681H\",37,28,28,21,04,00,30,33*5be776f0", "robot status", "#INSPVAXA,USB3,0,44.5,FINESTEERING,2113,382039.050,02000000,471d,15824;INS_SOLUTION_GOOD,INS_RTKFIXED,37.37017346694,126.72087268611,9.9166,22.3000,0.3222,-0.4372,-0.0049,0.092112708,-0.709135065,127.018965567,0.1682,0.1342,0.1455,0.0413,0.0361,0.0251,0.0347,0.0361,0.0882,0f000041,0*10805667", "robot status", "#DUALANTENNAHEADINGA,USB3,0,44.5,FINESTEERING,2113,382039.100,02000000,d426,15824;SOL_COMPUTED,NARROW_INT,-1.000000000,131.513717651,-14.392364502,0.0,0.380167335,0.950130761,\"681H\",37,28,28,21,04,00,30,33*f87b02b6", "robot status", "#INSPVAXA,USB3,0,45.0,FINESTEERING,2113,382039.150,02000000,471d,15824;INS_SOLUTION_GOOD,INS_RTKFIXED,37.37017378630,126.72087213679,9.9169,22.3000,0.4190,-0.5672,-0.0394,-0.007640761,-0.718204375,126.777494187,0.1682,0.1342,0.1455,0.0413,0.0361,0.0251,0.0347,0.0361,0.0882,0f000041,0*65be2f9d", "robot status", "#DUALANTENNAHEADINGA,USB3,0,45.0,FINESTEERING,2113,382039.200,02000000,d426,15824;SOL_COMPUTED,NARROW_INT,-1.000000000,131.121780396,-14.650421143,0.0,0.380796850,0.906092942,\"681H\",37,28,28,21,04,00,30,33*9bda838a", "robot status", "#INSPVAXA,USB3,0,45.0,FINESTEERING,2113,382039.250,02000000,471d,15824;INS_SOLUTION_GOOD,INS_RTKFIXED,37.37017418920,126.72087143733,9.9174,22.3000,0.5193,-0.6816,-0.0264,-0.134549913,-0.573595170,126.604647909,0.1682,0.1342,0.1455,0.0413,0.0361,0.0251,0.0347,0.0361,0.0882,0f000041,0*9380e58d", "robot status", "#INSPVAXA,USB3,0,45.0,FINESTEERING,2113,382039.300,02000000,471d,15824;INS_SOLUTION_GOOD,INS_RTKFIXED,37.37017442059,126.72087104053,9.9164,22.3000,0.5575,-0.7376,-0.0163,-0.358166188,-0.676721230,126.502598718,0.1682,0.1342,0.1455,0.0413,0.0361,0.0251,0.0347,0.0361,0.0882,0f000041,0*c5a04323", "robot status", "#INSPVAXA,USB3,0,45.0,FINESTEERING,2113,382039.350,02000000,471d,15824;INS_SOLUTION_GOOD,INS_RTKFIXED,37.37017466807,126.72087060869,9.9155,22.3000,0.5894,-0.8045,-0.0454,-0.228393430,-0.529299494,126.474074744,0.1682,0.1342,0.1455,0.0413,0.0361,0.0251,0.0347,0.0361,0.0882,0f000041,0*e24fc955", "robot status", "#DUALANTENNAHEADINGA,USB3,0,45.0,FINESTEERING,2113,382039.400,02000000,d426,15824;SOL_COMPUTED,NARROW_INT,-1.000000000,131.504135132,-13.201354980,0.0,0.381710082,0.915473580,\"681H\",37,28,28,21,04,00,30,33*a55ebdaf", "robot status", "#INSPVAXA,USB3,0,45.0,FINESTEERING,2113,382039.450,02000000,471d,15824;INS_SOLUTION_GOOD,INS_RTKFIXED,37.37017520934,126.72086966540,9.9161,22.3000,0.6550,-0.8885,0.0097,-0.396464277,-0.648383569,126.274232981,0.1682,0.1342,0.1455,0.0413,0.0361,0.0251,0.0347,0.0361,0.0882,0f000041,0*3ea90089", "robot status", "#INSPVAXA,USB3,0,45.0,FINESTEERING,2113,382039.500,02000000,471d,15824;INS_SOLUTION_GOOD,INS_RTKFIXED,37.37017550105,126.72086915131,9.9163,22.3000,0.6854,-0.9349,-0.0007,-0.354689430,-0.475031426,126.266254413,0.1682,0.1342,0.1455,0.0413,0.0361,0.0251,0.0347,0.0361,0.0882,0f000041,0*10d2ab12", "robot status", "#INSPVAXA,USB3,0,45.0,FINESTEERING,2113,382039.550,02000000,471d,15824;INS_SOLUTION_GOOD,INS_RTKFIXED,37.37017580890,126.72086861779,9.9167,22.3000,0.7224,-0.9663,-0.0003,-0.488193360,-0.406006969,126.160945445,0.1682,0.1342,0.1455,0.0413,0.0361,0.0251,0.0347,0.0361,0.0882,0f000041,0*ce2f4901", "robot status", "#DUALANTENNAHEADINGA,USB3,0,45.0,FINESTEERING,2113,382039.600,02000000,d426,15824;SOL_COMPUTED,NARROW_INT,-1.000000000,130.749755859,-15.418060303,0.0,0.392649740,0.926576793,\"681H\",37,28,28,21,04,00,30,33*5324307f", "robot status", "#INSPVAXA,USB3,0,45.0,FINESTEERING,2113,382039.650,02000000,471d,15824;INS_SOLUTION_GOOD,INS_RTKFIXED,37.37017645344,126.72086746708,9.9170,22.3000,0.7697,-1.0767,-0.0294,-0.485532075,-0.386630388,125.975723550,0.1682,0.1342,0.1455,0.0413,0.0361,0.0251,0.0347,0.0361,0.0882,0f000041,0*30030612", "robot status", "#INSPVAXA,USB3,0,45.0,FINESTEERING,2113,382039.700,02000000,471d,15824;INS_SOLUTION_GOOD,INS_RTKFIXED,37.37017680164,126.72086685532,9.9174,22.3000,0.8098,-1.1056,0.0218,-0.513147126,-0.403534188,125.866876908,0.1682,0.1342,0.1455,0.0413,0.0361,0.0251,0.0347,0.0361,0.0882,0f000041,0*33193311", "robot status", "#INSPVAXA,USB3,0,45.0,FINESTEERING,2113,382039.750,02000000,471d,15824;INS_SOLUTION_GOOD,INS_RTKFIXED,37.37017716338,126.72086622398,9.9180,22.3000,0.8364,-1.1406,-0.0018,-0.610723888,-0.458838053,125.752655178,0.1682,0.1342,0.1455,0.0413,0.0361,0.0251,0.0347,0.0361,0.0882,0f000041,0*fc77852f", "robot status", "#DUALANTENNAHEADINGA,USB3,0,45.0,FINESTEERING,2113,382039.800,02000000,d426,15824;SOL_COMPUTED,NARROW_INT,-1.000000000,130.576797485,-13.400848389,0.0,0.405704230,0.959964871,\"681H\",37,28,28,21,04,00,30,33*daa10485", "robot status", "#INSPVAXA,USB3,0,45.0,FINESTEERING,2113,382039.850,02000000,471d,15824;INS_SOLUTION_GOOD,INS_RTKFIXED,37.37017791407,126.72086490546,9.9174,22.3000,0.8613,-1.1911,0.0088,-0.805642160,-0.662709261,125.481368019,0.1682,0.1342,0.1455,0.0413,0.0361,0.0251,0.0347,0.0361,0.0882,0f000041,0*d6e9af4e", "robot status", "#DUALANTENNAHEADINGA,USB3,0,45.0,FINESTEERING,2113,382039.900,02000000,d426,15824;SOL_COMPUTED,NARROW_INT,-1.000000000,130.281204224,-14.222045898,0.0,0.407653749,0.959813118,\"681H\",37,28,28,21,04,00,30,33*653ec9f5", "robot status", "#INSPVAXA,USB3,0,45.0,FINESTEERING,2113,382039.950,02000000,471d,15824;INS_SOLUTION_GOOD,INS_RTKFIXED,37.37017865878,126.72086355931,9.9173,22.3000,0.8365,-1.1903,-0.0026,-0.690319926,-0.717177185,125.275608922,0.1682,0.1342,0.1455,0.0413,0.0361,0.0251,0.0347,0.0361,0.0882,0f000041,0*f182f7a8", "robot status", "#DUALANTENNAHEADINGA,USB3,0,45.0,FINESTEERING,2113,382040.000,02000000,d426,15824;SOL_COMPUTED,NARROW_INT,-1.000000000,130.328094482,-14.070892334,0.0,0.406570047,0.957207561,\"681H\",36,27,27,20,04,00,30,33*0b6d1c2d", "robot status", "#INSPVAXA,USB3,0,45.0,FINESTEERING,2113,382040.050,02000000,471d,15824;INS_SOLUTION_GOOD,INS_RTKFIXED,37.37017938611,126.72086224371,9.9170,22.3000,0.8057,-1.1751,-0.0233,-0.579108683,-0.523577997,125.006024550,0.1706,0.1306,0.1461,0.0417,0.0356,0.0252,0.0346,0.0363,0.0889,0f000041,0*cdd5fc88", "robot status", "#DUALANTENNAHEADINGA,USB3,0,44.0,FINESTEERING,2113,382040.100,02000000,d426,15824;SOL_COMPUTED,NARROW_INT,-1.000000000,130.335845947,-13.151580811,0.0,0.417014152,0.981959403,\"681H\",36,27,27,20,04,00,30,33*f26c0f61", "robot status", "#INSPVAXA,USB3,0,44.0,FINESTEERING,2113,382040.150,02000000,471d,15824;INS_SOLUTION_GOOD,INS_RTKFIXED,37.37018010503,126.72086101023,9.9163,22.3000,0.7736,-1.1087,-0.0053,-0.631835187,-0.452826202,124.757480547,0.1706,0.1306,0.1461,0.0417,0.0356,0.0252,0.0346,0.0363,0.0889,0f000041,0*44d4169e", "robot status", "#DUALANTENNAHEADINGA,USB3,0,44.0,FINESTEERING,2113,382040.200,02000000,d426,15824;SOL_COMPUTED,NARROW_INT,-1.000000000,129.794647217,-12.979339600,0.0,0.416089982,0.978759348,\"681H\",35,28,28,20,04,00,30,33*5271a122", "robot status", "#INSPVAXA,USB3,0,44.0,FINESTEERING,2113,382040.250,02000000,471d,15824;INS_SOLUTION_GOOD,INS_RTKFIXED,37.37018077591,126.72085983080,9.9171,22.3000,0.7258,-1.0347,0.0144,-0.638063256,-0.109269939,124.622891978,0.1706,0.1306,0.1461,0.0417,0.0356,0.0252,0.0346,0.0363,0.0889,0f000041,0*7d553eb5", "robot status", "#DUALANTENNAHEADINGA,USB3,0,44.0,FINESTEERING,2113,382040.300,02000000,d426,15824;SOL_COMPUTED,NARROW_INT,-1.000000000,129.701660156,-13.405090332,0.0,0.424458444,1.000435591,\"681H\",36,28,28,19,04,00,30,33*ffd7ae58", "robot status", "#INSPVAXA,USB3,0,44.0,FINESTEERING,2113,382040.350,02000000,471d,15824;INS_SOLUTION_GOOD,INS_RTKFIXED,37.37018140352,126.72085878190,9.9189,22.3000,0.6461,-0.9073,-0.0022,-0.872774653,-0.052154221,124.401871260,0.1706,0.1306,0.1461,0.0417,0.0356,0.0252,0.0346,0.0363,0.0889,0f000041,0*c4ef61b3", "robot status", "#DUALANTENNAHEADINGA,USB3,0,44.0,FINESTEERING,2113,382040.400,02000000,d426,15824;SOL_COMPUTED,NARROW_INT,-1.000000000,129.465454102,-13.373413086,0.0,0.421807587,0.998780966,\"681H\",36,28,28,19,04,00,30,33*d009ed86", "robot status", "#INSPVAXA,USB3,0,44.0,FINESTEERING,2113,382040.450,02000000,471d,15824;INS_SOLUTION_GOOD,INS_RTKFIXED,37.37018193164,126.72085786176,9.9205,22.3000,0.5280,-0.7924,0.0341,-0.916260371,-0.180167364,124.252750461,0.1706,0.1306,0.1461,0.0417,0.0356,0.0252,0.0346,0.0363,0.0889,0f000041,0*c9086a24", "robot status", "#DUALANTENNAHEADINGA,USB3,0,44.0,FINESTEERING,2113,382040.500,02000000,d426,15824;SOL_COMPUTED,NARROW_INT,-1.000000000,129.559051514,-11.819091797,0.0,0.417860329,0.993308306,\"681H\",36,28,28,20,04,00,30,33*a6287bb7", "robot status", "#INSPVAXA,USB3,0,44.0,FINESTEERING,2113,382040.550,02000000,471d,15824;INS_SOLUTION_GOOD,INS_RTKFIXED,37.37018236752,126.72085709311,9.9206,22.3000,0.4354,-0.6143,-0.0034,-0.820690096,-0.070667195,123.676235211,0.1706,0.1306,0.1461,0.0417,0.0356,0.0252,0.0346,0.0363,0.0889,0f000041,0*850bb0b4", "robot status", "#DUALANTENNAHEADINGA,USB3,0,44.0,FINESTEERING,2113,382040.600,02000000,d426,15824;SOL_COMPUTED,NARROW_INT,-1.000000000,128.443878174,-11.809295654,0.0,0.428597450,1.006724000,\"681H\",36,28,28,20,04,00,30,33*4b71f5f9", "robot status", "#INSPVAXA,USB3,0,44.0,FINESTEERING,2113,382040.650,02000000,471d,15824;INS_SOLUTION_GOOD,INS_RTKFIXED,37.37018269617,126.72085657263,9.9199,22.3000,0.2906,-0.4045,-0.0359,-0.774173731,-0.339101181,123.154795404,0.1706,0.1306,0.1461,0.0417,0.0356,0.0252,0.0346,0.0363,0.0889,0f000041,0*1bb2cdc0", "robot status", "#DUALANTENNAHEADINGA,USB3,0,44.0,FINESTEERING,2113,382040.700,02000000,d426,15824;SOL_COMPUTED,NARROW_INT,-1.000000000,128.251495361,-13.475311279,0.0,0.436341643,1.020166755,\"681H\",36,28,28,20,04,00,30,33*c729bd15", "robot status", "#INSPVAXA,USB3,0,44.0,FINESTEERING,2113,382040.750,02000000,471d,15824;INS_SOLUTION_GOOD,INS_RTKFIXED,37.37018287091,126.72085628357,9.9203,22.3000,0.1212,-0.1698,-0.0047,-0.634967207,-0.257097098,122.881002520,0.1706,0.1306,0.1461,0.0417,0.0356,0.0252,0.0346,0.0363,0.0889,0f000041,0*203b5b4a", "robot status", "#DUALANTENNAHEADINGA,USB3,0,44.0,FINESTEERING,2113,382040.800,02000000,d426,15824;SOL_COMPUTED,NARROW_INT,-1.000000000,127.882827759,-14.149047852,0.0,0.435033113,1.012094378,\"681H\",36,28,28,20,04,00,30,33*1c659d40", "robot status", "#INSPVAXA,USB3,0,44.0,FINESTEERING,2113,382040.850,02000000,471d,15824;INS_SOLUTION_GOOD,INS_RTKFIXED,37.37018294926,126.72085620787,9.9199,22.3000,0.0672,-0.0742,-0.0121,-0.706315718,-0.421420554,122.854161170,0.1706,0.1306,0.1461,0.0417,0.0356,0.0252,0.0346,0.0363,0.0889,0f000041,0*59eb6afa", "robot status", "#DUALANTENNAHEADINGA,USB3,0,44.0,FINESTEERING,2113,382040.900,02000000,d426,15824;SOL_COMPUTED,NARROW_INT,-1.000000000,127.949264526,-13.875885010,0.0,0.433813214,1.009172082,\"681H\",36,28,28,20,04,00,30,33*84155cd9", "robot status", "#INSPVAXA,USB3,0,44.0,FINESTEERING,2113,382040.950,02000000,471d,15824;INS_SOLUTION_GOOD,INS_RTKFIXED,37.37018301783,126.72085611332,9.9196,22.3000,0.0816,-0.1513,0.0005,-0.687891989,-0.659339914,122.492535409,0.1706,0.1306,0.1461,0.0417,0.0356,0.0252,0.0346,0.0363,0.0889,0f000041,0*662e47b0", "robot status", "#DUALANTENNAHEADINGA,USB3,0,44.0,FINESTEERING,2113,382041.000,02000000,d426,15824;SOL_COMPUTED,NARROW_INT,-1.000000000,127.347503662,-14.073913574,0.0,0.432040602,1.001151681,\"681H\",36,28,28,20,04,00,30,33*8fa1cd44", "robot status", "#INSPVAXA,USB3,0,44.0,FINESTEERING,2113,382041.050,02000000,471d,15824;INS_SOLUTION_GOOD,INS_RTKFIXED,37.37018310405,126.72085599307,9.9191,22.3000,0.0977,-0.1199,-0.0093,-0.612937733,-0.622906252,122.061292730,0.1729,0.1267,0.1466,0.0419,0.0346,0.0254,0.0344,0.0364,0.0897,0f000041,0*2e336a51", "robot status", "#DUALANTENNAHEADINGA,USB3,0,44.0,FINESTEERING,2113,382041.100,02000000,d426,15824;SOL_COMPUTED,NARROW_INT,-1.000000000,126.880668640,-13.804931641,0.0,0.430480123,0.998872519,\"681H\",36,28,28,20,04,00,30,33*c150a0a5", "robot status", "#INSPVAXA,USB3,0,45.5,FINESTEERING,2113,382041.150,02000000,471d,15824;INS_SOLUTION_GOOD,INS_RTKFIXED,37.37018317199,126.72085595570,9.9189,22.3000,0.0230,-0.0336,-0.0090,-0.597265728,-0.554547247,121.741932736,0.1729,0.1267,0.1466,0.0419,0.0346,0.0254,0.0344,0.0364,0.0897,0f000041,0*fffed022", "robot status", "#DUALANTENNAHEADINGA,USB3,0,45.5,FINESTEERING,2113,382041.200,02000000,d426,15824;SOL_COMPUTED,NARROW_INT,-1.000000000,126.550605774,-12.867858887,0.0,0.421657920,1.033517003,\"681H\",36,28,28,21,04,00,30,33*8b6a9263", "robot status", "#INSPVAXA,USB3,0,45.5,FINESTEERING,2113,382041.250,02000000,471d,15824;INS_SOLUTION_GOOD,INS_RTKFIXED,37.37018317716,126.72085604942,9.9188,22.3000,-0.0271,0.1079,-0.0028,-0.644900705,-0.521703597,121.633917003,0.1729,0.1267,0.1466,0.0419,0.0346,0.0254,0.0344,0.0364,0.0897,0f000041,0*c8fcfe2f", "robot status", "#DUALANTENNAHEADINGA,USB3,0,45.5,FINESTEERING,2113,382041.300,02000000,d426,15824;SOL_COMPUTED,NARROW_INT,-1.000000000,126.780883789,-13.160034180,0.0,0.417828888,1.025860429,\"681H\",36,28,28,21,04,00,30,33*a7c41a4c", "robot status", "#INSPVAXA,USB3,0,45.5,FINESTEERING,2113,382041.350,02000000,471d,15824;INS_SOLUTION_GOOD,INS_RTKFIXED,37.37018313295,126.72085626891,9.9192,22.3000,-0.0932,0.1803,-0.0021,-0.791987506,-0.589586799,121.458841080,0.1729,0.1267,0.1466,0.0419,0.0346,0.0254,0.0344,0.0364,0.0897,0f000041,0*bf6e772d", "robot status", "#DUALANTENNAHEADINGA,USB3,0,45.5,FINESTEERING,2113,382041.400,02000000,d426,15824;SOL_COMPUTED,NARROW_INT,-1.000000000,126.330741882,-14.128784180,0.0,0.417461425,1.015315294,\"681H\",36,28,28,21,04,00,30,33*cabdff96", "robot status", "#INSPVAXA,USB3,0,45.5,FINESTEERING,2113,382041.450,02000000,471d,15824;INS_SOLUTION_GOOD,INS_RTKFIXED,37.37018304119,126.72085653991,9.9195,22.3000,-0.1190,0.2038,-0.0004,-0.675601789,-0.668217598,121.170638709,0.1729,0.1267,0.1466,0.0419,0.0346,0.0254,0.0344,0.0364,0.0897,0f000041,0*6eac59ce", "robot status", "#DUALANTENNAHEADINGA,USB3,0,45.5,FINESTEERING,2113,382041.500,02000000,d426,15824;SOL_COMPUTED,NARROW_INT,-1.000000000,126.128067017,-13.198364258,0.0,0.413153559,1.010225892,\"681H\",37,28,28,21,04,00,30,33*588c2281", "robot status", "#INSPVAXA,USB3,0,45.5,FINESTEERING,2113,382041.550,02000000,471d,15824;INS_SOLUTION_GOOD,INS_RTKFIXED,37.37018295507,126.72085680167,9.9196,22.3000,-0.0851,0.1800,0.0029,-0.608502215,-0.690852555,120.854392991,0.1729,0.1267,0.1466,0.0419,0.0346,0.0254,0.0344,0.0364,0.0897,0f000041,0*88d97a82", "robot status", "#DUALANTENNAHEADINGA,USB3,0,45.5,FINESTEERING,2113,382041.600,02000000,d426,15824;SOL_COMPUTED,NARROW_INT,-1.000000000,125.864669800,-13.245239258,0.0,0.408464223,1.000799894,\"681H\",37,28,28,21,04,00,30,33*653ccc29", "robot status", "#INSPVAXA,USB3,0,45.5,FINESTEERING,2113,382041.650,02000000,471d,15824;INS_SOLUTION_GOOD,INS_RTKFIXED,37.37018290771,126.72085703245,9.9200,22.3000,-0.0513,0.1415,-0.0096,-0.738251358,-0.700928213,120.688048973,0.1729,0.1267,0.1466,0.0419,0.0346,0.0254,0.0344,0.0364,0.0897,0f000041,0*280cbd85", "robot status", "#DUALANTENNAHEADINGA,USB3,0,45.5,FINESTEERING,2113,382041.700,02000000,d426,15824;SOL_COMPUTED,NARROW_INT,-1.000000000,125.815193176,-13.145996094,0.0,0.408402503,1.001439214,\"681H\",37,28,28,21,04,00,30,33*c6f32cf9", "robot status", "#INSPVAXA,USB3,0,45.5,FINESTEERING,2113,382041.750,02000000,471d,15824;INS_SOLUTION_GOOD,INS_RTKFIXED,37.37018286409,126.72085720949,9.9199,22.3000,-0.0677,0.1045,-0.0084,-0.685619982,-0.669310142,120.313555328,0.1729,0.1267,0.1466,0.0419,0.0346,0.0254,0.0344,0.0364,0.0897,0f000041,0*5133ee27", "robot status", "#DUALANTENNAHEADINGA,USB3,0,45.5,FINESTEERING,2113,382041.800,02000000,d426,15824;SOL_COMPUTED,NARROW_INT,-1.000000000,125.454772949,-12.735107422,0.0,0.407116205,0.996651351,\"681H\",37,28,28,21,04,00,30,33*6c18e486", "robot status", "#INSPVAXA,USB3,0,45.5,FINESTEERING,2113,382041.850,02000000,471d,15824;INS_SOLUTION_GOOD,INS_RTKFIXED,37.37018282098,126.72085738973,9.9195,22.3000,-0.0545,0.1317,-0.0124,-0.664856353,-0.645418340,119.928134420,0.1729,0.1267,0.1466,0.0419,0.0346,0.0254,0.0344,0.0364,0.0897,0f000041,0*e362a80e", "robot status", "#DUALANTENNAHEADINGA,USB3,0,45.5,FINESTEERING,2113,382041.900,02000000,d426,15824;SOL_COMPUTED,NARROW_INT,-1.000000000,124.977478027,-12.484527588,0.0,0.404974282,0.986610413,\"681H\",37,28,28,21,04,00,30,33*61023521", "robot status", "#INSPVAXA,USB3,0,45.5,FINESTEERING,2113,382041.950,02000000,471d,15824;INS_SOLUTION_GOOD,INS_RTKFIXED,37.37018278268,126.72085759212,9.9195,22.3000,-0.0580,0.1536,-0.0009,-0.715837836,-0.589213950,119.680768588,0.1729,0.1267,0.1466,0.0419,0.0346,0.0254,0.0344,0.0364,0.0897,0f000041,0*ce251c89", "robot status", "#DUALANTENNAHEADINGA,USB3,0,45.5,FINESTEERING,2113,382042.000,02000000,d426,15824;SOL_COMPUTED,NARROW_INT,-1.000000000,124.872573853,-12.600860596,0.0,0.404576421,0.984803259,\"681H\",37,28,28,21,04,00,30,33*e6df10c4", "robot status", "#INSPVAXA,USB3,0,45.5,FINESTEERING,2113,382042.050,02000000,471d,15824;INS_SOLUTION_GOOD,INS_RTKFIXED,37.37018273023,126.72085780898,9.9196,22.3000,-0.0753,0.1593,-0.0048,-0.778324792,-0.511227199,119.408087923,0.1750,0.1231,0.1470,0.0421,0.0337,0.0255,0.0341,0.0365,0.0905,0f000041,0*e5deea1d", "robot status", "#DUALANTENNAHEADINGA,USB3,0,42.0,FINESTEERING,2113,382042.100,02000000,d426,15824;SOL_COMPUTED,NARROW_INT,-1.000000000,124.569641113,-12.740020752,0.0,0.399478376,0.970420361,\"681H\",37,28,28,21,04,00,30,33*991b1b3e", "robot status", "#INSPVAXA,USB3,0,42.0,FINESTEERING,2113,382042.150,02000000,471d,15824;INS_SOLUTION_GOOD,INS_RTKFIXED,37.37018265862,126.72085801536,9.9195,22.3000,-0.0726,0.1586,-0.0090,-0.764160347,-0.454116886,118.973352725,0.1750,0.1231,0.1470,0.0421,0.0337,0.0255,0.0341,0.0365,0.0905,0f000041,0*cc4da7ee", "robot status", "#DUALANTENNAHEADINGA,USB3,0,42.0,FINESTEERING,2113,382042.200,02000000,d426,15824;SOL_COMPUTED,NARROW_INT,-1.000000000,123.845954895,-13.371032715,0.0,0.400096387,0.962732196,\"681H\",37,28,28,22,04,00,30,33*e4228c9e", "robot status", "#INSPVAXA,USB3,0,42.0,FINESTEERING,2113,382042.250,02000000,471d,15824;INS_SOLUTION_GOOD,INS_RTKFIXED,37.37018260131,126.72085821856,9.9200,22.3000,-0.0566,0.1560,-0.0017,-0.759139266,-0.468139219,118.683807868,0.1750,0.1231,0.1470,0.0421,0.0337,0.0255,0.0341,0.0365,0.0905,0f000041,0*fdc94f88", "robot status", "#INSPVAXA,USB3,0,42.0,FINESTEERING,2113,382042.350,02000000,471d,15824;INS_SOLUTION_GOOD,INS_RTKFIXED,37.37018255721,126.72085842274,9.9203,22.3000,-0.0469,0.1519,-0.0036,-0.848481326,-0.411291027,118.455593913,0.1750,0.1231,0.1470,0.0421,0.0337,0.0255,0.0341,0.0365,0.0905,0f000041,0*e7ce3ab6", "robot status", "#INSPVAXA,USB3,0,42.0,FINESTEERING,2113,382042.350,02000000,471d,15824;INS_SOLUTION_GOOD,INS_RTKFIXED,37.37018255721,126.72085842274,9.9203,22.3000,-0.0469,0.1519,-0.0036,-0.848481326,-0.411291027,118.455593913,0.1750,0.1231,0.1470,0.0421,0.0337,0.0255,0.0341,0.0365,0.0905,0f000041,0*e7ce3ab6", "robot status", "#DUALANTENNAHEADINGA,USB3,0,42.0,FINESTEERING,2113,382042.400,02000000,d426,15824;SOL_COMPUTED,NARROW_INT,-1.000000000,123.320114136,-13.632385254,0.0,0.397878706,0.950293362,\"681H\",37,28,28,22,04,00,30,33*b252c18e", "robot status", "#INSPVAXA,USB3,0,42.0,FINESTEERING,2113,382042.500,02000000,471d,15824;INS_SOLUTION_GOOD,INS_RTKFIXED,37.37018246278,126.72085868015,9.9207,22.3000,-0.0731,0.1346,-0.0103,-0.728761343,-0.282319381,117.654727820,0.1750,0.1231,0.1470,0.0421,0.0337,0.0255,0.0341,0.0365,0.0905,0f000041,0*f5aa0955", "robot status", "#INSPVAXA,USB3,0,42.0,FINESTEERING,2113,382042.550,02000000,471d,15824;INS_SOLUTION_GOOD,INS_RTKFIXED,37.37018243530,126.72085877125,9.9207,22.3000,-0.0513,0.1449,-0.0051,-0.700499096,-0.301125060,117.381291460,0.1750,0.1231,0.1470,0.0421,0.0337,0.0255,0.0341,0.0365,0.0905,0f000041,0*679bd386", "robot status", "#INSPVAXA,USB3,0,42.0,FINESTEERING,2113,382042.550,02000000,471d,15824;INS_SOLUTION_GOOD,INS_RTKFIXED,37.37018243530,126.72085877125,9.9207,22.3000,-0.0513,0.1449,-0.0051,-0.700499096,-0.301125060,117.381291460,0.1750,0.1231,0.1470,0.0421,0.0337,0.0255,0.0341,0.0365,0.0905,0f000041,0*679bd386", "robot status", "#DUALANTENNAHEADINGA,USB3,0,42.0,FINESTEERING,2113,382042.600,02000000,d426,15824;SOL_COMPUTED,NARROW_INT,-1.000000000,122.133644104,-13.482116699,0.0,0.400358945,0.948118985,\"681H\",36,28,28,22,04,00,30,33*8f2b2377", "robot status", "#INSPVAXA,USB3,0,42.0,FINESTEERING,2113,382042.700,02000000,471d,15824;INS_SOLUTION_GOOD,INS_RTKFIXED,37.37018235948,126.72085904228,9.9210,22.3000,-0.0525,0.1383,-0.0029,-0.688303195,-0.303404905,116.724046512,0.1750,0.1231,0.1470,0.0421,0.0337,0.0255,0.0341,0.0365,0.0905,0f000041,0*e760ad34", "robot status", "#INSPVAXA,USB3,0,42.0,FINESTEERING,2113,382042.750,02000000,471d,15824;INS_SOLUTION_GOOD,INS_RTKFIXED,37.37018233796,126.72085913340,9.9212,22.3000,-0.0483,0.1434,-0.0052,-0.684254535,-0.304866849,116.506184902,0.1750,0.1231,0.1470,0.0421,0.0337,0.0255,0.0341,0.0365,0.0905,0f000041,0*1fcf7a94", "robot status", "#INSPVAXA,USB3,0,42.0,FINESTEERING,2113,382042.750,02000000,471d,15824;INS_SOLUTION_GOOD,INS_RTKFIXED,37.37018233796,126.72085913340,9.9212,22.3000,-0.0483,0.1434,-0.0052,-0.684254535,-0.304866849,116.506184902,0.1750,0.1231,0.1470,0.0421,0.0337,0.0255,0.0341,0.0365,0.0905,0f000041,0*1fcf7a94", "robot status", "#DUALANTENNAHEADINGA,USB3,0,42.0,FINESTEERING,2113,382042.800,02000000,d426,15824;SOL_COMPUTED,NARROW_INT,-1.000000000,121.384597778,-12.706634521,0.0,0.402153343,0.948337138,\"681H\",36,28,28,22,04,00,30,33*16b0933c", "robot status", "#INSPVAXA,USB3,0,42.0,FINESTEERING,2113,382042.900,02000000,471d,15824;INS_SOLUTION_GOOD,INS_RTKFIXED,37.37018225748,126.72085940042,9.9213,22.3000,-0.0593,0.1464,-0.0057,-0.614364063,-0.293247191,115.649490894,0.1750,0.1231,0.1470,0.0421,0.0337,0.0255,0.0341,0.0365,0.0905,0f000041,0*dc53ceba", "robot status", "#INSPVAXA,USB3,0,42.0,FINESTEERING,2113,382042.950,02000000,471d,15824;INS_SOLUTION_GOOD,INS_RTKFIXED,37.37018222994,126.72085949579,9.9213,22.3000,-0.0643,0.1521,-0.0116,-0.639279962,-0.319745948,115.400719299,0.1750,0.1231,0.1470,0.0421,0.0337,0.0255,0.0341,0.0365,0.0905,0f000041,0*ca73d494", "robot status", "#INSPVAXA,USB3,0,42.0,FINESTEERING,2113,382043.000,02000000,471d,15824;INS_SOLUTION_GOOD,INS_RTKFIXED,37.37018219939,126.72085959420,9.9210,22.3000,-0.0707,0.1615,-0.0128,-0.580172028,-0.293733213,115.123214081,0.1750,0.1231,0.1470,0.0421,0.0337,0.0255,0.0341,0.0365,0.0905,0f000041,0*c9ae7347", "robot status", "#DUALANTENNAHEADINGA,USB3,0,42.0,FINESTEERING,2113,382043.000,02000000,d426,15824;SOL_COMPUTED,NARROW_INT,-1.000000000,120.096504211,-13.048706055,0.0,0.404469609,0.941555977,\"681H\",36,28,28,22,04,00,30,33*8ce35e69", "robot status", "#INSPVAXA,USB3,0,42.0,FINESTEERING,2113,382043.050,02000000,471d,15824;INS_SOLUTION_GOOD,INS_RTKFIXED,37.37018217133,126.72085969568,9.9208,22.3000,-0.0514,0.1748,-0.0029,-0.539329529,-0.322608006,114.934303882,0.1771,0.1195,0.1474,0.0423,0.0328,0.0256,0.0339,0.0366,0.0912,0f000041,0*d87b3c4d", "robot status", "#INSPVAXA,USB3,0,44.5,FINESTEERING,2113,382043.150,02000000,471d,15824;INS_SOLUTION_GOOD,INS_RTKFIXED,37.37018212345,126.72085988069,9.9206,22.3000,-0.0509,0.1461,-0.0106,-0.651882987,-0.322495907,114.428430048,0.1771,0.1195,0.1474,0.0423,0.0328,0.0256,0.0339,0.0366,0.0912,0f000041,0*0e90e5a9", "robot status", "#INSPVAXA,USB3,0,44.5,FINESTEERING,2113,382043.200,02000000,471d,15824;INS_SOLUTION_GOOD,INS_RTKFIXED,37.37018209537,126.72085995747,9.9204,22.3000,-0.0568,0.1320,-0.0078,-0.671759286,-0.298418516,114.130824552,0.1771,0.1195,0.1474,0.0423,0.0328,0.0256,0.0339,0.0366,0.0912,0f000041,0*eb9b973d", "robot status", "#DUALANTENNAHEADINGA,USB3,0,44.5,FINESTEERING,2113,382043.200,02000000,d426,15824;SOL_COMPUTED,NARROW_INT,-1.000000000,119.233612061,-13.515014648,0.0,0.404297411,0.930233717,\"681H\",36,28,28,23,04,00,30,33*50fa3145", "robot status", "#INSPVAXA,USB3,0,44.5,FINESTEERING,2113,382043.300,02000000,471d,15824;INS_SOLUTION_GOOD,INS_RTKFIXED,37.37018204186,126.72086011273,9.9202,22.3000,-0.0535,0.1450,-0.0116,-0.623638454,-0.380842955,113.596312059,0.1771,0.1195,0.1474,0.0423,0.0328,0.0256,0.0339,0.0366,0.0912,0f000041,0*829218ac", "robot status", "#INSPVAXA,USB3,0,44.5,FINESTEERING,2113,382043.350,02000000,471d,15824;INS_SOLUTION_GOOD,INS_RTKFIXED,37.37018201377,126.72086019385,9.9199,22.3000,-0.0569,0.1474,-0.0087,-0.569123391,-0.410611637,113.288066281,0.1771,0.1195,0.1474,0.0423,0.0328,0.0256,0.0339,0.0366,0.0912,0f000041,0*fb415d35", "robot status", "#INSPVAXA,USB3,0,44.5,FINESTEERING,2113,382043.400,02000000,471d,15824;INS_SOLUTION_GOOD,INS_RTKFIXED,37.37018198664,126.72086027857,9.9196,22.3000,-0.0502,0.1580,-0.0112,-0.527926735,-0.427861530,113.045564094,0.1771,0.1195,0.1474,0.0423,0.0328,0.0256,0.0339,0.0366,0.0912,0f000041,0*a8d11b66", "robot status", "#DUALANTENNAHEADINGA,USB3,0,44.5,FINESTEERING,2113,382043.400,02000000,d426,15824;SOL_COMPUTED,NARROW_INT,-1.000000000,118.083244324,-13.913055420,0.0,0.405499697,0.923583090,\"681H\",36,28,28,23,04,00,30,33*b587c552", "robot status", "#INSPVAXA,USB3,0,44.5,FINESTEERING,2113,382043.450,02000000,471d,15824;INS_SOLUTION_GOOD,INS_RTKFIXED,37.37018196462,126.72086036513,9.9194,22.3000,-0.0324,0.1535,-0.0054,-0.544396528,-0.392479170,112.858057396,0.1771,0.1195,0.1474,0.0423,0.0328,0.0256,0.0339,0.0366,0.0912,0f000041,0*5ace5e87", "robot status", "#INSPVAXA,USB3,0,44.5,FINESTEERING,2113,382043.550,02000000,471d,15824;INS_SOLUTION_GOOD,INS_RTKFIXED,37.37018194447,126.72086050535,9.9192,22.3000,0.0046,0.0927,-0.0079,-0.592611486,-0.442736317,112.878015631,0.1771,0.1195,0.1474,0.0423,0.0328,0.0256,0.0339,0.0366,0.0912,0f000041,0*30410c8e", "robot status", "#INSPVAXA,USB3,0,44.5,FINESTEERING,2113,382043.600,02000000,471d,15824;INS_SOLUTION_GOOD,INS_RTKFIXED,37.37018194988,126.72086054205,9.9192,22.3000,0.0331,0.0407,-0.0011,-0.600024074,-0.500060840,113.186159853,0.1771,0.1195,0.1474,0.0423,0.0328,0.0256,0.0339,0.0366,0.0912,0f000041,0*08d40667", "robot status", "#INSPVAXA,USB3,0,44.5,FINESTEERING,2113,382043.650,02000000,471d,15824;INS_SOLUTION_GOOD,INS_RTKFIXED,37.37018196403,126.72086054798,9.9191,22.3000,0.0457,-0.0133,-0.0120,-0.616446841,-0.489842416,113.076235379,0.1771,0.1195,0.1474,0.0423,0.0328,0.0256,0.0339,0.0366,0.0912,0f000041,0*fc165023", "robot status", "#INSPVAXA,USB3,0,44.5,FINESTEERING,2113,382043.650,02000000,471d,15824;INS_SOLUTION_GOOD,INS_RTKFIXED,37.37018196403,126.72086054798,9.9191,22.3000,0.0457,-0.0133,-0.0120,-0.616446841,-0.489842416,113.076235379,0.1771,0.1195,0.1474,0.0423,0.0328,0.0256,0.0339,0.0366,0.0912,0f000041,0*fc165023", "robot status", "#INSPVAXA,USB3,0,44.5,FINESTEERING,2113,382043.750,02000000,471d,15824;INS_SOLUTION_GOOD,INS_RTKFIXED,37.37018200479,126.72086050099,9.9189,22.3000,0.0634,-0.0484,-0.0097,-0.572527014,-0.443924648,113.404612747,0.1771,0.1195,0.1474,0.0423,0.0328,0.0256,0.0339,0.0366,0.0912,0f000041,0*0b8ce0fb", "robot status", "#INSPVAXA,USB3,0,44.5,FINESTEERING,2113,382043.800,02000000,471d,15824;INS_SOLUTION_GOOD,INS_RTKFIXED,37.37018202867,126.72086047502,9.9186,22.3000,0.0559,-0.0399,-0.0150,-0.656309069,-0.384020317,113.624775736,0.1771,0.1195,0.1474,0.0423,0.0328,0.0256,0.0339,0.0366,0.0912,0f000041,0*1ed5e243", "robot status", "#INSPVAXA,USB3,0,44.5,FINESTEERING,2113,382043.850,02000000,471d,15824;INS_SOLUTION_GOOD,INS_RTKFIXED,37.37018204771,126.72086045367,9.9186,22.3000,0.0465,-0.0296,-0.0029,-0.640293829,-0.381349282,113.650349507,0.1771,0.1195,0.1474,0.0423,0.0328,0.0256,0.0339,0.0366,0.0912,0f000041,0*bf548666", "robot status", "#INSPVAXA,USB3,0,44.5,FINESTEERING,2113,382043.850,02000000,471d,15824;INS_SOLUTION_GOOD,INS_RTKFIXED,37.37018204771,126.72086045367,9.9186,22.3000,0.0465,-0.0296,-0.0029,-0.640293829,-0.381349282,113.650349507,0.1771,0.1195,0.1474,0.0423,0.0328,0.0256,0.0339,0.0366,0.0912,0f000041,0*bf548666", "robot status", "#INSPVAXA,USB3,0,44.5,FINESTEERING,2113,382043.950,02000000,471d,15824;INS_SOLUTION_GOOD,INS_RTKFIXED,37.37018208741,126.72086042533,9.9184,22.3000,0.0482,-0.0091,-0.0053,-0.632769829,-0.363094801,113.765640648,0.1771,0.1195,0.1474,0.0423,0.0328,0.0256,0.0339,0.0366,0.0912,0f000041,0*54fc1bdd", "robot status", "#INSPVAXA,USB3,0,44.5,FINESTEERING,2113,382044.000,02000000,471d,15824;INS_SOLUTION_GOOD,INS_RTKFIXED,37.37018210526,126.72086042034,9.9182,22.3000,0.0440,-0.0043,-0.0101,-0.643990490,-0.380204849,114.052677998,0.1771,0.1195,0.1474,0.0423,0.0328,0.0256,0.0339,0.0366,0.0912,0f000041,0*8e2fb256", "robot status", "#INSPVAXA,USB3,0,44.0,FINESTEERING,2113,382044.050,02000000,471d,15824;INS_SOLUTION_GOOD,INS_RTKFIXED,37.37018212062,126.72086041430,9.9182,22.3000,0.0512,-0.0116,-0.0036,-0.633398688,-0.375165666,114.208056039,0.1789,0.1177,0.1478,0.0426,0.0324,0.0257,0.0339,0.0369,0.0920,0f000041,0*cf9d4b24", "robot status", "#INSPVAXA,USB3,0,44.0,FINESTEERING,2113,382044.100,02000000,471d,15824;INS_SOLUTION_GOOD,INS_RTKFIXED,37.37018213908,126.72086039923,9.9184,22.3000,0.0840,-0.0380,-0.0078,-0.597883749,-0.413980337,114.449110353,0.1789,0.1177,0.1478,0.0426,0.0324,0.0257,0.0339,0.0369,0.0920,0f000041,0*32e76cd8", "robot status", "#INSPVAXA,USB3,0,44.0,FINESTEERING,2113,382044.150,02000000,471d,15824;INS_SOLUTION_GOOD,INS_RTKFIXED,37.37018218466,126.72086036553,9.9186,22.3000,0.1593,-0.0749,-0.0041,-0.538473127,-0.456700757,115.001034625,0.1789,0.1177,0.1478,0.0426,0.0324,0.0257,0.0339,0.0369,0.0920,0f000041,0*3c61a5e5", "robot status", "#INSPVAXA,USB3,0,44.0,FINESTEERING,2113,382044.200,02000000,471d,15824;INS_SOLUTION_GOOD,INS_RTKFIXED,37.37018225639,126.72086031208,9.9190,22.3000,0.1909,-0.1069,0.0029,-0.714606306,-0.380473357,115.707639774,0.1789,0.1177,0.1478,0.0426,0.0324,0.0257,0.0339,0.0369,0.0920,0f000041,0*968eb905", "robot status", "#INSPVAXA,USB3,0,44.0,FINESTEERING,2113,382044.250,02000000,471d,15824;INS_SOLUTION_GOOD,INS_RTKFIXED,37.37018233048,126.72086024084,9.9194,22.3000,0.1921,-0.1423,-0.0100,-0.683722161,-0.381580693,116.417824477,0.1789,0.1177,0.1478,0.0426,0.0324,0.0257,0.0339,0.0369,0.0920,0f000041,0*311486b1", "robot status", "#INSPVAXA,USB3,0,44.0,FINESTEERING,2113,382044.300,02000000,471d,15824;INS_SOLUTION_GOOD,INS_RTKFIXED,37.37018240996,126.72086014853,9.9196,22.3000,0.2044,-0.1778,-0.0021,-0.737866067,-0.406460181,117.135528003,0.1789,0.1177,0.1478,0.0426,0.0324,0.0257,0.0339,0.0369,0.0920,0f000041,0*35824f16", "robot status", "#INSPVAXA,USB3,0,44.0,FINESTEERING,2113,382044.350,02000000,471d,15824;INS_SOLUTION_GOOD,INS_RTKFIXED,37.37018249635,126.72086003550,9.9195,22.3000,0.2124,-0.2163,-0.0116,-0.688973545,-0.399385228,117.716803341,0.1789,0.1177,0.1478,0.0426,0.0324,0.0257,0.0339,0.0369,0.0920,0f000041,0*874a051d", "robot status", "#INSPVAXA,USB3,0,44.0,FINESTEERING,2113,382044.400,02000000,471d,15824;INS_SOLUTION_GOOD,INS_RTKFIXED,37.37018258226,126.72085990615,9.9199,22.3000,0.2097,-0.2383,0.0029,-0.801988126,-0.384587612,118.190737712,0.1789,0.1177,0.1478,0.0426,0.0324,0.0257,0.0339,0.0369,0.0920,0f000041,0*758e727b", "robot status", "#INSPVAXA,USB3,0,44.0,FINESTEERING,2113,382044.450,02000000,471d,15824;INS_SOLUTION_GOOD,INS_RTKFIXED,37.37018267261,126.72085976407,9.9203,22.3000,0.2185,-0.2573,0.0045,-0.867415686,-0.329624648,118.460395859,0.1789,0.1177,0.1478,0.0426,0.0324,0.0257,0.0339,0.0369,0.0920,0f000041,0*78eed538", "robot status", "#INSPVAXA,USB3,0,44.0,FINESTEERING,2113,382044.500,02000000,471d,15824;INS_SOLUTION_GOOD,INS_RTKFIXED,37.37018275271,126.72085961829,9.9210,22.3000,0.1822,-0.2552,-0.0007,-0.867166551,-0.265336659,118.723840884,0.1789,0.1177,0.1478,0.0426,0.0324,0.0257,0.0339,0.0369,0.0920,0f000041,0*8e081eb9", "robot status", "#INSPVAXA,USB3,0,44.0,FINESTEERING,2113,382044.550,02000000,471d,15824;INS_SOLUTION_GOOD,INS_RTKFIXED,37.37018282547,126.72085946886,9.9209,22.3000,0.1823,-0.2693,-0.0124,-0.706254619,-0.392370502,118.947238928,0.1789,0.1177,0.1478,0.0426,0.0324,0.0257,0.0339,0.0369,0.0920,0f000041,0*8ff19df0", "robot status", "#INSPVAXA,USB3,0,44.0,FINESTEERING,2113,382044.600,02000000,471d,15824;INS_SOLUTION_GOOD,INS_RTKFIXED,37.37018290598,126.72085931252,9.9214,22.3000,0.2084,-0.2796,0.0144,-0.720943222,-0.454320641,118.965140950,0.1789,0.1177,0.1478,0.0426,0.0324,0.0257,0.0339,0.0369,0.0920,0f000041,0*c86eec22", "robot status", "#INSPVAXA,USB3,0,44.0,FINESTEERING,2113,382044.650,02000000,471d,15824;INS_SOLUTION_GOOD,INS_RTKFIXED,37.37018299681,126.72085914882,9.9219,22.3000,0.2252,-0.2917,-0.0068,-0.804348021,-0.400015813,118.985170722,0.1789,0.1177,0.1478,0.0426,0.0324,0.0257,0.0339,0.0369,0.0920,0f000041,0*7255a9e5", "robot status", "#INSPVAXA,USB3,0,44.0,FINESTEERING,2113,382044.700,02000000,471d,15824;INS_SOLUTION_GOOD,INS_RTKFIXED,37.37018308536,126.72085898732,9.9223,22.3000,0.2083,-0.2765,0.0050,-0.806747859,-0.428071591,119.204492465,0.1789,0.1177,0.1478,0.0426,0.0324,0.0257,0.0339,0.0369,0.0920,0f000041,0*96e7d984", "robot status", "#INSPVAXA,USB3,0,44.0,FINESTEERING,2113,382044.750,02000000,471d,15824;INS_SOLUTION_GOOD,INS_RTKFIXED,37.37018316536,126.72085883491,9.9223,22.3000,0.1825,-0.2560,-0.0156,-0.753881296,-0.474609175,119.423997421,0.1789,0.1177,0.1478,0.0426,0.0324,0.0257,0.0339,0.0369,0.0920,0f000041,0*79fd0a37", "robot status", "#INSPVAXA,USB3,0,44.0,FINESTEERING,2113,382044.800,02000000,471d,15824;INS_SOLUTION_GOOD,INS_RTKFIXED,37.37018323548,126.72085870279,9.9226,22.3000,0.1614,-0.2053,0.0063,-0.739986548,-0.407825269,119.431156514,0.1789,0.1177,0.1478,0.0426,0.0324,0.0257,0.0339,0.0369,0.0920,0f000041,0*f0a1c265", "robot status", "#INSPVAXA,USB3,0,44.0,FINESTEERING,2113,382044.850,02000000,471d,15824;INS_SOLUTION_GOOD,INS_RTKFIXED,37.37018329279,126.72085860340,9.9230,22.3000,0.1304,-0.1399,-0.0083,-0.802491521,-0.354025239,119.389802932,0.1789,0.1177,0.1478,0.0426,0.0324,0.0257,0.0339,0.0369,0.0920,0f000041,0*c2af1227", "robot status", "#INSPVAXA,USB3,0,44.0,FINESTEERING,2113,382044.900,02000000,471d,15824;INS_SOLUTION_GOOD,INS_RTKFIXED,37.37018333425,126.72085854385,9.9231,22.3000,0.0862,-0.0638,-0.0029,-0.826266057,-0.349275152,119.405657063,0.1789,0.1177,0.1478,0.0426,0.0324,0.0257,0.0339,0.0369,0.0920,0f000041,0*2cb8dc6c", "robot status", "#INSPVAXA,USB3,0,44.0,FINESTEERING,2113,382044.950,02000000,471d,15824;INS_SOLUTION_GOOD,INS_RTKFIXED,37.37018335529,126.72085852863,9.9233,22.3000,0.0404,0.0149,-0.0050,-0.829689843,-0.335273876,119.413268918,0.1789,0.1177,0.1478,0.0426,0.0324,0.0257,0.0339,0.0369,0.0920,0f000041,0*d9216fec", "robot status", "#DUALANTENNAHEADINGA,USB3,0,44.0,FINESTEERING,2113,382045.000,02000000,d426,15824;SOL_COMPUTED,NARROW_INT,-1.000000000,124.594978333,-12.904571533,0.0,0.383978039,0.931631625,\"681H\",36,27,27,21,04,00,30,33*1014dfef", "robot status", "#INSPVAXA,USB3,0,44.0,FINESTEERING,2113,382045.050,02000000,471d,15824;INS_SOLUTION_GOOD,INS_RTKFIXED,37.37018334562,126.72085860644,9.9233,22.3000,-0.0173,0.1156,-0.0088,-0.808506545,-0.356613639,119.335655135,0.1794,0.1189,0.1483,0.0426,0.0326,0.0258,0.0341,0.0370,0.0928,0f000041,0*9ceee5e3", "robot status", "#INSPVAXA,USB3,0,44.0,FINESTEERING,2113,382045.100,02000000,471d,15824;INS_SOLUTION_GOOD,INS_RTKFIXED,37.37018332729,126.72085867565,9.9232,22.3000,-0.0256,0.1358,-0.0089,-0.802300406,-0.390704596,119.268252073,0.1794,0.1189,0.1483,0.0426,0.0326,0.0258,0.0341,0.0370,0.0928,0f000041,0*b548db3d", "robot status", "#INSPVAXA,USB3,0,45.0,FINESTEERING,2113,382045.150,02000000,471d,15824;INS_SOLUTION_GOOD,INS_RTKFIXED,37.37018330754,126.72085875037,9.9231,22.3000,-0.0243,0.1345,-0.0093,-0.796317012,-0.402649837,119.117498902,0.1794,0.1189,0.1483,0.0426,0.0326,0.0258,0.0341,0.0370,0.0928,0f000041,0*35a6db17", "robot status", "#DUALANTENNAHEADINGA,USB3,0,45.0,FINESTEERING,2113,382045.200,02000000,d426,15824;SOL_COMPUTED,NARROW_INT,-1.000000000,123.928237915,-13.600097656,0.0,0.387685776,0.933416307,\"681H\",36,28,28,21,04,00,30,33*7771ad58", "robot status", "#INSPVAXA,USB3,0,45.0,FINESTEERING,2113,382045.250,02000000,471d,15824;INS_SOLUTION_GOOD,INS_RTKFIXED,37.37018326842,126.72085889097,9.9232,22.3000,-0.0273,0.1208,-0.0078,-0.754616174,-0.414293255,118.931089377,0.1794,0.1189,0.1483,0.0426,0.0326,0.0258,0.0341,0.0370,0.0928,0f000041,0*4a91f728", "robot status", "#INSPVAXA,USB3,0,45.0,FINESTEERING,2113,382045.300,02000000,471d,15824;INS_SOLUTION_GOOD,INS_RTKFIXED,37.37018325024,126.72085895434,9.9233,22.3000,-0.0152,0.1110,-0.0019,-0.758979193,-0.433624310,118.973847932,0.1794,0.1189,0.1483,0.0426,0.0326,0.0258,0.0341,0.0370,0.0928,0f000041,0*804c01e5", "robot status", "#INSPVAXA,USB3,0,45.0,FINESTEERING,2113,382045.350,02000000,471d,15824;INS_SOLUTION_GOOD,INS_RTKFIXED,37.37018324363,126.72085900249,9.9235,22.3000,0.0200,0.0672,-0.0068,-0.750044443,-0.481733340,118.746744087,0.1794,0.1189,0.1483,0.0426,0.0326,0.0258,0.0341,0.0370,0.0928,0f000041,0*74fceb12", "robot status", "#DUALANTENNAHEADINGA,USB3,0,45.0,FINESTEERING,2113,382045.400,02000000,d426,15824;SOL_COMPUTED,NARROW_INT,-1.000000000,123.179939270,-14.330291748,0.0,0.389762998,0.932966173,\"681H\",36,28,28,21,04,00,30,33*a31ecb32", "robot status", "#INSPVAXA,USB3,0,45.0,FINESTEERING,2113,382045.450,02000000,471d,15824;INS_SOLUTION_GOOD,INS_RTKFIXED,37.37018326605,126.72085901762,9.9237,22.3000,0.0545,-0.0208,-0.0038,-0.776504404,-0.416347157,118.286471645,0.1794,0.1189,0.1483,0.0426,0.0326,0.0258,0.0341,0.0370,0.0928,0f000041,0*9234cbb8", "robot status", "#INSPVAXA,USB3,0,45.0,FINESTEERING,2113,382045.500,02000000,471d,15824;INS_SOLUTION_GOOD,INS_RTKFIXED,37.37018328098,126.72085900164,9.9237,22.3000,0.0438,-0.0229,-0.0067,-0.767156036,-0.367634401,118.004377112,0.1794,0.1189,0.1483,0.0426,0.0326,0.0258,0.0341,0.0370,0.0928,0f000041,0*6ed207d8", "robot status", "#INSPVAXA,USB3,0,45.0,FINESTEERING,2113,382045.550,02000000,471d,15824;INS_SOLUTION_GOOD,INS_RTKFIXED,37.37018328789,126.72085899695,9.9239,22.3000,0.0197,0.0175,0.0026,-0.755262930,-0.250312537,117.641322086,0.1794,0.1189,0.1483,0.0426,0.0326,0.0258,0.0341,0.0370,0.0928,0f000041,0*c524a68f", "robot status", "#DUALANTENNAHEADINGA,USB3,0,45.0,FINESTEERING,2113,382045.600,02000000,d426,15824;SOL_COMPUTED,NARROW_INT,-1.000000000,122.177436829,-13.534210205,0.0,0.392673314,0.933407128,\"681H\",36,28,28,21,04,00,30,33*55bee265", "robot status", "#INSPVAXA,USB3,0,45.0,FINESTEERING,2113,382045.650,02000000,471d,15824;INS_SOLUTION_GOOD,INS_RTKFIXED,37.37018326398,126.72085908994,9.9251,22.3000,-0.0489,0.1465,-0.0180,-0.743039230,-0.038515063,116.751384495,0.1794,0.1189,0.1483,0.0426,0.0326,0.0258,0.0341,0.0370,0.0928,0f000041,0*25660571", "robot status", "#INSPVAXA,USB3,0,45.0,FINESTEERING,2113,382045.700,02000000,471d,15824;INS_SOLUTION_GOOD,INS_RTKFIXED,37.37018322037,126.72085917955,9.9248,22.3000,-0.1033,0.1813,-0.0009,-0.722450884,-0.098766890,116.132751118,0.1794,0.1189,0.1483,0.0426,0.0326,0.0258,0.0341,0.0370,0.0928,0f000041,0*56afa59a", "robot status", "#INSPVAXA,USB3,0,45.0,FINESTEERING,2113,382045.750,02000000,471d,15824;INS_SOLUTION_GOOD,INS_RTKFIXED,37.37018315612,126.72085928801,9.9250,22.3000,-0.1463,0.2107,-0.0113,-0.696558758,-0.123722440,115.686260551,0.1794,0.1189,0.1483,0.0426,0.0326,0.0258,0.0341,0.0370,0.0928,0f000041,0*58646f9c", "robot status", "#DUALANTENNAHEADINGA,USB3,0,45.0,FINESTEERING,2113,382045.800,02000000,d426,15824;SOL_COMPUTED,NARROW_INT,-1.000000000,120.007202148,-13.639373779,0.0,0.399467647,0.935086608,\"681H\",36,28,28,21,04,00,30,33*4bafb432", "robot status", "#INSPVAXA,USB3,0,45.0,FINESTEERING,2113,382045.850,02000000,471d,15824;INS_SOLUTION_GOOD,INS_RTKFIXED,37.37018303491,126.72085956877,9.9250,22.3000,-0.0948,0.2766,-0.0024,-0.671142601,-0.127895351,114.582432246,0.1794,0.1189,0.1483,0.0426,0.0326,0.0258,0.0341,0.0370,0.0928,0f000041,0*c547236c", "robot status", "#INSPVAXA,USB3,0,45.0,FINESTEERING,2113,382045.900,02000000,471d,15824;INS_SOLUTION_GOOD,INS_RTKFIXED,37.37018298036,126.72085971954,9.9246,22.3000,-0.1168,0.2643,-0.0215,-0.707291504,-0.238411576,114.060517724,0.1794,0.1189,0.1483,0.0426,0.0326,0.0258,0.0341,0.0370,0.0928,0f000041,0*7bf7fc26", "robot status", "#INSPVAXA,USB3,0,45.0,FINESTEERING,2113,382045.950,02000000,471d,15824;INS_SOLUTION_GOOD,INS_RTKFIXED,37.37018291624,126.72085986085,9.9241,22.3000,-0.1288,0.2480,-0.0089,-0.580459835,-0.269960432,113.644325856,0.1794,0.1189,0.1483,0.0426,0.0326,0.0258,0.0341,0.0370,0.0928,0f000041,0*a3ca4e44", "robot status", "#INSPVAXA,USB3,0,45.0,FINESTEERING,2113,382046.000,02000000,471d,15824;INS_SOLUTION_GOOD,INS_RTKFIXED,37.37018285947,126.72086000357,9.9241,22.3000,-0.0921,0.2655,-0.0050,-0.474581926,-0.209286328,113.324658424,0.1794,0.1189,0.1483,0.0426,0.0326,0.0258,0.0341,0.0370,0.0928,0f000041,0*e113bff5", "robot status", "#INSPVAXA,USB3,0,45.0,FINESTEERING,2113,382046.050,02000000,471d,15824;INS_SOLUTION_GOOD,INS_RTKFIXED,37.37018281412,126.72086014802,9.9239,22.3000,-0.0529,0.2622,-0.0090,-0.558415808,-0.188217768,112.935146496,0.1805,0.1174,0.1486,0.0428,0.0319,0.0259,0.0340,0.0372,0.0936,0f000041,0*215c3e39", "robot status", "#DUALANTENNAHEADINGA,USB3,0,44.0,FINESTEERING,2113,382046.100,02000000,d426,15824;SOL_COMPUTED,NARROW_INT,-1.000000000,117.478904724,-13.876281738,0.0,0.404973328,0.925294816,\"681H\",36,28,28,21,04,00,30,33*b21d5689", "robot status", "#INSPVAXA,USB3,0,44.0,FINESTEERING,2113,382046.150,02000000,471d,15824;INS_SOLUTION_GOOD,INS_RTKFIXED,37.37018271366,126.72086040443,9.9227,22.3000,-0.0951,0.2130,-0.0133,-0.556427454,-0.280435139,112.091749820,0.1805,0.1174,0.1486,0.0428,0.0319,0.0259,0.0340,0.0372,0.0936,0f000041,0*6ceedc27", "robot status", "#DUALANTENNAHEADINGA,USB3,0,44.0,FINESTEERING,2113,382046.200,02000000,d426,15824;SOL_COMPUTED,NARROW_INT,-1.000000000,116.657501221,-13.462432861,0.0,0.406259596,0.922787368,\"681H\",36,28,28,21,04,00,30,33*04ce2f58", "robot status", "#INSPVAXA,USB3,0,44.0,FINESTEERING,2113,382046.250,02000000,471d,15824;INS_SOLUTION_GOOD,INS_RTKFIXED,37.37018261515,126.72086064789,9.9219,22.3000,-0.0490,0.2382,-0.0063,-0.513116671,-0.266158735,111.311036839,0.1805,0.1174,0.1486,0.0428,0.0319,0.0259,0.0340,0.0372,0.0936,0f000041,0*ae3884b5", "robot status", "#DUALANTENNAHEADINGA,USB3,0,44.0,FINESTEERING,2113,382046.300,02000000,d426,15824;SOL_COMPUTED,NARROW_INT,-1.000000000,116.124450684,-13.352752686,0.0,0.410278559,0.927334487,\"681H\",36,28,28,21,04,00,30,33*f53ce2cd", "robot status", "#INSPVAXA,USB3,0,44.0,FINESTEERING,2113,382046.350,02000000,471d,15824;INS_SOLUTION_GOOD,INS_RTKFIXED,37.37018252576,126.72086090290,9.9215,22.3000,-0.0993,0.2214,-0.0117,-0.608050703,-0.351712909,110.360802695,0.1805,0.1174,0.1486,0.0428,0.0319,0.0259,0.0340,0.0372,0.0936,0f000041,0*8566a023", "robot status", "#DUALANTENNAHEADINGA,USB3,0,44.0,FINESTEERING,2113,382046.400,02000000,d426,15824;SOL_COMPUTED,NARROW_INT,-1.000000000,115.258308411,-12.881195068,0.0,0.415206283,0.933827043,\"681H\",36,28,28,21,04,00,30,33*6300acc5", "robot status", "#INSPVAXA,USB3,0,44.0,FINESTEERING,2113,382046.450,02000000,471d,15824;INS_SOLUTION_GOOD,INS_RTKFIXED,37.37018240836,126.72086115150,9.9205,22.3000,-0.0683,0.2492,-0.0016,-0.369754373,-0.426283382,109.431251569,0.1805,0.1174,0.1486,0.0428,0.0319,0.0259,0.0340,0.0372,0.0936,0f000041,0*8af59999", "robot status", "#DUALANTENNAHEADINGA,USB3,0,44.0,FINESTEERING,2113,382046.500,02000000,d426,15824;SOL_COMPUTED,NARROW_INT,-1.000000000,113.988082886,-13.483612061,0.0,0.419930547,0.932076275,\"681H\",36,27,27,21,04,00,30,33*e11a59c9", "robot status", "#INSPVAXA,USB3,0,44.0,FINESTEERING,2113,382046.550,02000000,471d,15824;INS_SOLUTION_GOOD,INS_RTKFIXED,37.37018232964,126.72086142961,9.9202,22.3000,-0.0825,0.2387,-0.0117,-0.513809080,-0.527696716,108.344891464,0.1805,0.1174,0.1486,0.0428,0.0319,0.0259,0.0340,0.0372,0.0936,0f000041,0*69fdf985", "robot status", "#DUALANTENNAHEADINGA,USB3,0,44.0,FINESTEERING,2113,382046.600,02000000,d426,15824;SOL_COMPUTED,NARROW_INT,-1.000000000,112.414703369,-13.860504150,0.0,0.426283747,0.931046665,\"681H\",36,27,27,21,04,00,30,33*42464bf0", "robot status", "#INSPVAXA,USB3,0,44.0,FINESTEERING,2113,382046.650,02000000,471d,15824;INS_SOLUTION_GOOD,INS_RTKFIXED,37.37018221960,126.72086167550,9.9203,22.3000,-0.0677,0.2344,0.0017,-0.297748569,-0.671206781,107.376844926,0.1805,0.1174,0.1486,0.0428,0.0319,0.0259,0.0340,0.0372,0.0936,0f000041,0*3b7dc13b", "robot status", "#DUALANTENNAHEADINGA,USB3,0,44.0,FINESTEERING,2113,382046.700,02000000,d426,15824;SOL_COMPUTED,NARROW_INT,-1.000000000,111.457298279,-13.806365967,0.0,0.430951893,0.932600021,\"681H\",36,27,27,21,04,00,30,33*cc9c9ea7", "robot status", "#INSPVAXA,USB3,0,44.0,FINESTEERING,2113,382046.750,02000000,471d,15824;INS_SOLUTION_GOOD,INS_RTKFIXED,37.37018214736,126.72086194511,9.9201,22.3000,-0.0634,0.2491,-0.0163,-0.425432975,-0.728050663,106.341980121,0.1805,0.1174,0.1486,0.0428,0.0319,0.0259,0.0340,0.0372,0.0936,0f000041,0*24dbf45c", "robot status", "#DUALANTENNAHEADINGA,USB3,0,44.0,FINESTEERING,2113,382046.800,02000000,d426,15824;SOL_COMPUTED,NARROW_INT,-1.000000000,110.397987366,-14.550201416,0.0,0.432301432,0.923781157,\"681H\",36,27,27,21,04,00,30,33*b80a9211", "robot status", "#INSPVAXA,USB3,0,44.0,FINESTEERING,2113,382046.850,02000000,471d,15824;INS_SOLUTION_GOOD,INS_RTKFIXED,37.37018205145,126.72086219756,9.9195,22.3000,-0.0568,0.2321,0.0017,-0.279923454,-0.803252761,105.338081208,0.1805,0.1174,0.1486,0.0428,0.0319,0.0259,0.0340,0.0372,0.0936,0f000041,0*d4a563e9", "robot status", "#DUALANTENNAHEADINGA,USB3,0,44.0,FINESTEERING,2113,382046.900,02000000,d426,15824;SOL_COMPUTED,NARROW_INT,-1.000000000,109.613197327,-14.308807373,0.0,0.434831947,0.925777912,\"681H\",36,27,27,21,04,00,30,33*f51c7b46", "robot status", "#INSPVAXA,USB3,0,44.0,FINESTEERING,2113,382046.950,02000000,471d,15824;INS_SOLUTION_GOOD,INS_RTKFIXED,37.37018198656,126.72086244734,9.9192,22.3000,-0.0393,0.2213,-0.0128,-0.467090658,-0.714998177,104.190201915,0.1805,0.1174,0.1486,0.0428,0.0319,0.0259,0.0340,0.0372,0.0936,0f000041,0*2573d2ea", "robot status", "#DUALANTENNAHEADINGA,USB3,0,44.0,FINESTEERING,2113,382047.000,02000000,d426,15824;SOL_COMPUTED,NARROW_INT,-1.000000000,108.607452393,-13.600738525,0.0,0.439293146,0.932854354,\"681H\",36,27,27,21,04,00,30,33*96979504", "robot status", "#INSPVAXA,USB3,0,44.0,FINESTEERING,2113,382047.050,02000000,471d,15824;INS_SOLUTION_GOOD,INS_RTKFIXED,37.37018190192,126.72086266714,9.9189,22.3000,-0.0663,0.1997,-0.0068,-0.422150093,-0.769144869,103.086248386,0.1819,0.1170,0.1480,0.0432,0.0328,0.0259,0.0345,0.0374,0.0945,0f000041,0*74968d1e", "robot status", "#DUALANTENNAHEADINGA,USB3,0,44.0,FINESTEERING,2113,382047.100,02000000,d426,15824;SOL_COMPUTED,NARROW_INT,-1.000000000,107.593391418,-13.394836426,0.0,0.443387747,0.934106708,\"681H\",36,27,27,21,04,00,30,33*8ce1c884", "robot status", "#INSPVAXA,USB3,0,45.0,FINESTEERING,2113,382047.150,02000000,471d,15824;INS_SOLUTION_GOOD,INS_RTKFIXED,37.37018182751,126.72086287013,9.9200,22.3000,-0.0206,0.2030,-0.0063,-0.549115962,-0.700042196,101.995500830,0.1819,0.1170,0.1480,0.0432,0.0328,0.0259,0.0345,0.0374,0.0945,0f000041,0*81053848", "robot status", "#DUALANTENNAHEADINGA,USB3,0,45.0,FINESTEERING,2113,382047.200,02000000,d426,15824;SOL_COMPUTED,NARROW_INT,-1.000000000,106.413528442,-12.896942139,0.0,0.444939315,0.931608737,\"681H\",36,28,28,22,04,00,30,33*322da1ec", "robot status", "#INSPVAXA,USB3,0,45.0,FINESTEERING,2113,382047.250,02000000,471d,15824;INS_SOLUTION_GOOD,INS_RTKFIXED,37.37018175451,126.72086304980,9.9201,22.3000,-0.0513,0.1626,-0.0153,-0.554432882,-0.725918527,100.957692880,0.1819,0.1170,0.1480,0.0432,0.0328,0.0259,0.0345,0.0374,0.0945,0f000041,0*e2fc0ef0", "robot status", "#DUALANTENNAHEADINGA,USB3,0,45.0,FINESTEERING,2113,382047.300,02000000,d426,15824;SOL_COMPUTED,NARROW_INT,-1.000000000,105.589530945,-12.932952881,0.0,0.447847217,0.929723382,\"681H\",36,28,28,22,04,00,30,33*e2824a2c", "robot status", "#INSPVAXA,USB3,0,45.0,FINESTEERING,2113,382047.350,02000000,471d,15824;INS_SOLUTION_GOOD,INS_RTKFIXED,37.37018170455,126.72086318106,9.9205,22.3000,0.0195,0.1157,-0.0076,-0.517345426,-0.816566560,100.354245672,0.1819,0.1170,0.1480,0.0432,0.0328,0.0259,0.0345,0.0374,0.0945,0f000041,0*2509961e", "robot status", "#DUALANTENNAHEADINGA,USB3,0,45.0,FINESTEERING,2113,382047.400,02000000,d426,15824;SOL_COMPUTED,NARROW_INT,-1.000000000,105.122306824,-13.538848877,0.0,0.448971778,0.926412821,\"681H\",36,28,28,22,04,00,30,33*33a4cb3b", "robot status", "#INSPVAXA,USB3,0,45.0,FINESTEERING,2113,382047.450,02000000,471d,15824;INS_SOLUTION_GOOD,INS_RTKFIXED,37.37018169919,126.72086324959,9.9210,22.3000,0.0490,0.0601,-0.0059,-0.555029124,-0.854723439,100.883796938,0.1819,0.1170,0.1480,0.0432,0.0328,0.0259,0.0345,0.0374,0.0945,0f000041,0*2ee7376e", "robot status", "#DUALANTENNAHEADINGA,USB3,0,45.0,FINESTEERING,2113,382047.500,02000000,d426,15824;SOL_COMPUTED,NARROW_INT,-1.000000000,106.227523804,-13.724945068,0.0,0.443731487,0.922842503,\"681H\",36,28,28,22,04,00,30,33*d398b7e8", "robot status", "#INSPVAXA,USB3,0,45.0,FINESTEERING,2113,382047.550,02000000,471d,15824;INS_SOLUTION_GOOD,INS_RTKFIXED,37.37018170445,126.72086325644,9.9212,22.3000,0.0406,0.0032,-0.0077,-0.562375264,-0.872773332,100.726887379,0.1819,0.1170,0.1480,0.0432,0.0328,0.0259,0.0345,0.0374,0.0945,0f000041,0*333adc69", "robot status", "#DUALANTENNAHEADINGA,USB3,0,45.0,FINESTEERING,2113,382047.600,02000000,d426,15824;SOL_COMPUTED,NARROW_INT,-1.000000000,105.693519592,-13.339385986,0.0,0.448140502,0.929471552,\"681H\",36,28,28,22,04,00,30,33*b78f902b", "robot status", "#INSPVAXA,USB3,0,45.0,FINESTEERING,2113,382047.650,02000000,471d,15824;INS_SOLUTION_GOOD,INS_RTKFIXED,37.37018171220,126.72086322021,9.9217,22.3000,0.0562,-0.0087,-0.0083,-0.569870798,-0.840734273,100.914601520,0.1819,0.1170,0.1480,0.0432,0.0328,0.0259,0.0345,0.0374,0.0945,0f000041,0*6503f1c3", "robot status", "#DUALANTENNAHEADINGA,USB3,0,45.0,FINESTEERING,2113,382047.700,02000000,d426,15824;SOL_COMPUTED,NARROW_INT,-1.000000000,105.813179016,-13.557037354,0.0,0.450193226,0.934405982,\"681H\",36,28,28,22,04,00,30,33*840ba539", "robot status", "#INSPVAXA,USB3,0,45.0,FINESTEERING,2113,382047.750,02000000,471d,15824;INS_SOLUTION_GOOD,INS_RTKFIXED,37.37018172180,126.72086319293,9.9220,22.3000,0.0431,0.0085,-0.0048,-0.565718123,-0.830916693,100.831199650,0.1819,0.1170,0.1480,0.0432,0.0328,0.0259,0.0345,0.0374,0.0945,0f000041,0*baa94eea", "robot status", "#DUALANTENNAHEADINGA,USB3,0,45.0,FINESTEERING,2113,382047.800,02000000,d426,15824;SOL_COMPUTED,NARROW_INT,-1.000000000,105.765167236,-13.312500000,0.0,0.450101197,0.935074985,\"681H\",36,28,28,22,04,00,30,33*184a026b", "robot status", "#INSPVAXA,USB3,0,45.0,FINESTEERING,2113,382047.850,02000000,471d,15824;INS_SOLUTION_GOOD,INS_RTKFIXED,37.37018172820,126.72086318164,9.9225,22.3000,0.0484,0.0145,-0.0050,-0.569930538,-0.846887671,100.819425519,0.1819,0.1170,0.1480,0.0432,0.0328,0.0259,0.0345,0.0374,0.0945,0f000041,0*714d04d7", "robot status", "#DUALANTENNAHEADINGA,USB3,0,45.0,FINESTEERING,2113,382047.900,02000000,d426,15824;SOL_COMPUTED,NARROW_INT,-1.000000000,105.740768433,-13.858642578,0.0,0.447376400,0.927213788,\"681H\",36,28,28,22,04,00,30,33*563420bb", "robot status", "#INSPVAXA,USB3,0,45.0,FINESTEERING,2113,382047.950,02000000,471d,15824;INS_SOLUTION_GOOD,INS_RTKFIXED,37.37018173686,126.72086316498,9.9229,22.3000,0.0466,0.0038,-0.0051,-0.565966285,-0.841132141,100.853522197,0.1819,0.1170,0.1480,0.0432,0.0328,0.0259,0.0345,0.0374,0.0945,0f000041,0*4668e94a", "robot status", "#DUALANTENNAHEADINGA,USB3,0,45.0,FINESTEERING,2113,382048.000,02000000,d426,15824;SOL_COMPUTED,NARROW_INT,-1.000000000,105.898361206,-13.665161133,0.0,0.448473990,0.931421578,\"681H\",36,28,28,22,04,00,30,33*18af81fc", "robot status", "#INSPVAXA,USB3,0,45.0,FINESTEERING,2113,382048.050,02000000,471d,15824;INS_SOLUTION_GOOD,INS_RTKFIXED,37.37018174522,126.72086314749,9.9233,22.3000,0.0461,0.0103,-0.0049,-0.571911188,-0.837334848,100.856344663,0.1832,0.1175,0.1476,0.0436,0.0336,0.0260,0.0348,0.0376,0.0952,0f000041,0*3d853827", "robot status", "#DUALANTENNAHEADINGA,USB3,0,43.5,FINESTEERING,2113,382048.100,02000000,d426,15824;SOL_COMPUTED,NARROW_INT,-1.000000000,105.881820679,-13.540191650,0.0,0.451658428,0.937966526,\"681H\",36,28,28,22,04,00,30,33*def820eb", "robot status", "#INSPVAXA,USB3,0,43.5,FINESTEERING,2113,382048.150,02000000,471d,15824;INS_SOLUTION_GOOD,INS_RTKFIXED,37.37018174524,126.72086313260,9.9236,22.3000,0.0482,0.0068,-0.0050,-0.565487628,-0.842979376,100.841811075,0.1832,0.1175,0.1476,0.0436,0.0336,0.0260,0.0348,0.0376,0.0952,0f000041,0*8b811e99", "robot status", "#DUALANTENNAHEADINGA,USB3,0,43.5,FINESTEERING,2113,382048.200,02000000,d426,15824;SOL_COMPUTED,NARROW_INT,-1.000000000,105.761756897,-12.936126709,0.0,0.450926661,0.938185155,\"681H\",36,28,28,22,04,00,30,33*64ca5e34", "robot status", "#INSPVAXA,USB3,0,43.5,FINESTEERING,2113,382048.250,02000000,471d,15824;INS_SOLUTION_GOOD,INS_RTKFIXED,37.37018174751,126.72086311446,9.9239,22.3000,0.0454,0.0064,-0.0055,-0.568128737,-0.838472145,100.837507360,0.1832,0.1175,0.1476,0.0436,0.0336,0.0260,0.0348,0.0376,0.0952,0f000041,0*3b237696", "robot status", "#DUALANTENNAHEADINGA,USB3,0,43.5,FINESTEERING,2113,382048.300,02000000,d426,15824;SOL_COMPUTED,NARROW_INT,-1.000000000,105.861244202,-13.786956787,0.0,0.450709343,0.933096230,\"681H\",36,28,28,22,04,00,30,33*5d673c61", "robot status", "#INSPVAXA,USB3,0,43.5,FINESTEERING,2113,382048.350,02000000,471d,15824;INS_SOLUTION_GOOD,INS_RTKFIXED,37.37018174675,126.72086309750,9.9242,22.3000,0.0479,0.0078,-0.0053,-0.567481244,-0.841384254,100.847934116,0.1832,0.1175,0.1476,0.0436,0.0336,0.0260,0.0348,0.0376,0.0952,0f000041,0*716dd434", "robot status", "#DUALANTENNAHEADINGA,USB3,0,43.5,FINESTEERING,2113,382048.400,02000000,d426,15824;SOL_COMPUTED,NARROW_INT,-1.000000000,105.830253601,-13.503204346,0.0,0.448643357,0.930388987,\"681H\",36,28,28,22,04,00,30,33*bd417d6c", "robot status", "#INSPVAXA,USB3,0,43.5,FINESTEERING,2113,382048.450,02000000,471d,15824;INS_SOLUTION_GOOD,INS_RTKFIXED,37.37018174665,126.72086307832,9.9246,22.3000,0.0464,0.0051,-0.0047,-0.565957923,-0.838244625,100.851921729,0.1832,0.1175,0.1476,0.0436,0.0336,0.0260,0.0348,0.0376,0.0952,0f000041,0*694aa4e3", "robot status", "#DUALANTENNAHEADINGA,USB3,0,43.5,FINESTEERING,2113,382048.500,02000000,d426,15824;SOL_COMPUTED,NARROW_INT,-1.000000000,105.917610168,-12.879028320,0.0,0.448994756,0.934205532,\"681H\",36,28,28,22,04,00,30,33*9839706a", "robot status", "#INSPVAXA,USB3,0,43.5,FINESTEERING,2113,382048.550,02000000,471d,15824;INS_SOLUTION_GOOD,INS_RTKFIXED,37.37018175041,126.72086306223,9.9249,22.3000,0.0467,0.0073,-0.0049,-0.567643390,-0.839683144,100.849091788,0.1832,0.1175,0.1476,0.0436,0.0336,0.0260,0.0348,0.0376,0.0952,0f000041,0*956c7baf", "robot status", "#DUALANTENNAHEADINGA,USB3,0,43.5,FINESTEERING,2113,382048.600,02000000,d426,15824;SOL_COMPUTED,NARROW_INT,-1.000000000,105.843879700,-13.245758057,0.0,0.447214097,0.928849638,\"681H\",36,28,28,22,04,00,30,33*7a7753ef", "robot status", "#INSPVAXA,USB3,0,43.5,FINESTEERING,2113,382048.650,02000000,471d,15824;INS_SOLUTION_GOOD,INS_RTKFIXED,37.37018175132,126.72086304402,9.9252,22.3000,0.0470,0.0047,-0.0048,-0.565695111,-0.840387671,100.845531863,0.1832,0.1175,0.1476,0.0436,0.0336,0.0260,0.0348,0.0376,0.0952,0f000041,0*57feaf2a", "robot status", "#DUALANTENNAHEADINGA,USB3,0,43.5,FINESTEERING,2113,382048.700,02000000,d426,15824;SOL_COMPUTED,NARROW_INT,-1.000000000,105.774047852,-13.596527100,0.0,0.447161019,0.923722863,\"681H\",36,28,28,22,04,00,30,33*19cb2569", "robot status", "#INSPVAXA,USB3,0,43.5,FINESTEERING,2113,382048.750,02000000,471d,15824;INS_SOLUTION_GOOD,INS_RTKFIXED,37.37018175606,126.72086302875,9.9255,22.3000,0.0455,0.0106,-0.0051,-0.567537582,-0.836856638,100.807562146,0.1832,0.1175,0.1476,0.0436,0.0336,0.0260,0.0348,0.0376,0.0952,0f000041,0*4ea62479", "robot status", "#DUALANTENNAHEADINGA,USB3,0,43.5,FINESTEERING,2113,382048.800,02000000,d426,15824;SOL_COMPUTED,NARROW_INT,-1.000000000,105.758270264,-12.780456543,0.0,0.445461690,0.923769176,\"681H\",36,28,28,21,04,00,30,33*83da7012", "robot status", "#INSPVAXA,USB3,0,43.5,FINESTEERING,2113,382048.850,02000000,471d,15824;INS_SOLUTION_GOOD,INS_RTKFIXED,37.37018175721,126.72086302655,9.9258,22.3000,0.0427,0.0335,-0.0059,-0.581006833,-0.821254954,100.577930500,0.1832,0.1175,0.1476,0.0436,0.0336,0.0260,0.0348,0.0376,0.0952,0f000041,0*12bbf60b", "robot status", "#DUALANTENNAHEADINGA,USB3,0,43.5,FINESTEERING,2113,382048.900,02000000,d426,15824;SOL_COMPUTED,NARROW_INT,-1.000000000,105.415016174,-13.279327393,0.0,0.448866785,0.923833966,\"681H\",36,28,28,21,04,00,30,33*3e830be4", "robot status", "#INSPVAXA,USB3,0,43.5,FINESTEERING,2113,382048.950,02000000,471d,15824;INS_SOLUTION_GOOD,INS_RTKFIXED,37.37018175557,126.72086305260,9.9261,22.3000,0.0343,0.0521,-0.0031,-0.588757317,-0.822527035,100.291212555,0.1832,0.1175,0.1476,0.0436,0.0336,0.0260,0.0348,0.0376,0.0952,0f000041,0*02ef5191", "robot status", "#DUALANTENNAHEADINGA,USB3,0,43.5,FINESTEERING,2113,382049.000,02000000,d426,15824;SOL_COMPUTED,NARROW_INT,-1.000000000,105.012748718,-13.373535156,0.0,0.449422091,0.921198428,\"681H\",36,28,28,21,04,00,30,33*808960d5", "robot status", "#INSPVAXA,USB3,0,43.5,FINESTEERING,2113,382049.050,02000000,471d,15824;INS_SOLUTION_GOOD,INS_RTKFIXED,37.37018173546,126.72086310546,9.9266,22.3000,0.0048,0.0828,-0.0028,-0.652405165,-0.806839997,99.865893021,0.1844,0.1184,0.1476,0.0439,0.0341,0.0260,0.0351,0.0379,0.0961,0f000041,0*d4f0806e", "robot status", "#DUALANTENNAHEADINGA,USB3,0,43.5,FINESTEERING,2113,382049.100,02000000,d426,15824;SOL_COMPUTED,NARROW_INT,-1.000000000,104.565528870,-13.454772949,0.0,0.452582359,0.921454370,\"681H\",36,28,28,21,04,00,30,33*3e9979d8", "robot status", "#INSPVAXA,USB3,0,45.5,FINESTEERING,2113,382049.150,02000000,471d,15824;INS_SOLUTION_GOOD,INS_RTKFIXED,37.37018167841,126.72086320881,9.9271,22.3000,-0.0307,0.1298,-0.0041,-0.633499394,-0.850525346,98.967439962,0.1844,0.1184,0.1476,0.0439,0.0341,0.0260,0.0351,0.0379,0.0961,0f000041,0*5110c669", "robot status", "#DUALANTENNAHEADINGA,USB3,0,45.5,FINESTEERING,2113,382049.200,02000000,d426,15824;SOL_COMPUTED,NARROW_INT,-1.000000000,103.331459045,-13.499847412,0.0,0.457163900,0.920419574,\"681H\",36,28,28,21,04,00,30,33*ebf8cba2", "robot status", "#INSPVAXA,USB3,0,45.5,FINESTEERING,2113,382049.250,02000000,471d,15824;INS_SOLUTION_GOOD,INS_RTKFIXED,37.37018161188,126.72086336681,9.9278,22.3000,-0.0189,0.1729,-0.0038,-0.599893984,-0.965135396,98.094171059,0.1844,0.1184,0.1476,0.0439,0.0341,0.0260,0.0351,0.0379,0.0961,0f000041,0*98d032e1", "robot status", "#DUALANTENNAHEADINGA,USB3,0,45.5,FINESTEERING,2113,382049.300,02000000,d426,15824;SOL_COMPUTED,NARROW_INT,-1.000000000,102.421768188,-14.127593994,0.0,0.459712535,0.917162299,\"681H\",36,28,28,21,04,00,30,33*9eb7a063", "robot status", "#INSPVAXA,USB3,0,45.5,FINESTEERING,2113,382049.350,02000000,471d,15824;INS_SOLUTION_GOOD,INS_RTKFIXED,37.37018155298,126.72086355540,9.9282,22.3000,-0.0032,0.1878,0.0005,-0.569745476,-1.011439121,97.322605170,0.1844,0.1184,0.1476,0.0439,0.0341,0.0260,0.0351,0.0379,0.0961,0f000041,0*d1391cab", "robot status", "#DUALANTENNAHEADINGA,USB3,0,45.5,FINESTEERING,2113,382049.400,02000000,d426,15824;SOL_COMPUTED,NARROW_INT,-1.000000000,102.023880005,-14.092468262,0.0,0.460822582,0.917445600,\"681H\",36,28,28,20,04,00,30,33*df94957b", "robot status", "#INSPVAXA,USB3,0,45.5,FINESTEERING,2113,382049.450,02000000,471d,15824;INS_SOLUTION_GOOD,INS_RTKFIXED,37.37018150678,126.72086374259,9.9285,22.3000,-0.0074,0.1714,-0.0025,-0.630167281,-1.042497658,96.576189483,0.1844,0.1184,0.1476,0.0439,0.0341,0.0260,0.0351,0.0379,0.0961,0f000041,0*c2c5cc33", "robot status", "#INSPVAXA,USB3,0,45.5,FINESTEERING,2113,382049.550,02000000,471d,15824;INS_SOLUTION_GOOD,INS_RTKFIXED,37.37018145518,126.72086391622,9.9286,22.3000,0.0003,0.1706,-0.0104,-0.566342979,-1.097877509,95.906901055,0.1844,0.1184,0.1476,0.0439,0.0341,0.0260,0.0351,0.0379,0.0961,0f000041,0*8d12361b", "robot status", "#INSPVAXA,USB3,0,45.5,FINESTEERING,2113,382049.550,02000000,471d,15824;INS_SOLUTION_GOOD,INS_RTKFIXED,37.37018145518,126.72086391622,9.9286,22.3000,0.0003,0.1706,-0.0104,-0.566342979,-1.097877509,95.906901055,0.1844,0.1184,0.1476,0.0439,0.0341,0.0260,0.0351,0.0379,0.0961,0f000041,0*8d12361b", "robot status", "#DUALANTENNAHEADINGA,USB3,0,45.5,FINESTEERING,2113,382049.600,02000000,d426,15824;SOL_COMPUTED,NARROW_INT,-1.000000000,100.833160400,-14.113891602,0.0,0.465645880,0.916137636,\"681H\",35,28,28,20,04,00,30,33*55e3a81f", "robot status", "#INSPVAXA,USB3,0,45.5,FINESTEERING,2113,382049.650,02000000,471d,15824;INS_SOLUTION_GOOD,INS_RTKFIXED,37.37018142891,126.72086410525,9.9287,22.3000,0.0289,0.1876,-0.0024,-0.585501815,-1.129898412,95.492061117,0.1844,0.1184,0.1476,0.0439,0.0341,0.0260,0.0351,0.0379,0.0961,0f000041,0*9598d23a", "robot status", "#INSPVAXA,USB3,0,45.5,FINESTEERING,2113,382049.750,02000000,471d,15824;INS_SOLUTION_GOOD,INS_RTKFIXED,37.37018140072,126.72086429201,9.9290,22.3000,0.0063,0.1632,-0.0064,-0.554196999,-1.074189925,95.038345956,0.1844,0.1184,0.1476,0.0439,0.0341,0.0260,0.0351,0.0379,0.0961,0f000041,0*659d7b37", "robot status", "#INSPVAXA,USB3,0,45.5,FINESTEERING,2113,382049.800,02000000,471d,15824;INS_SOLUTION_GOOD,INS_RTKFIXED,37.37018138143,126.72086437510,9.9291,22.3000,-0.0046,0.1594,0.0003,-0.537401947,-1.054245393,94.781261983,0.1844,0.1184,0.1476,0.0439,0.0341,0.0260,0.0351,0.0379,0.0961,0f000041,0*19abe31e", "robot status", "#DUALANTENNAHEADINGA,USB3,0,45.5,FINESTEERING,2113,382049.800,02000000,d426,15824;SOL_COMPUTED,NARROW_INT,-1.000000000,100.229255676,-13.089080811,0.0,0.465936780,0.920580983,\"681H\",36,28,28,20,04,00,30,33*de0af68d", "robot status", "#INSPVAXA,USB3,0,45.5,FINESTEERING,2113,382049.850,02000000,471d,15824;INS_SOLUTION_GOOD,INS_RTKFIXED,37.37018136188,126.72086445886,9.9292,22.3000,0.0063,0.1644,-0.0085,-0.481873199,-1.062030172,94.510071252,0.1844,0.1184,0.1476,0.0439,0.0341,0.0260,0.0351,0.0379,0.0961,0f000041,0*657613cf", "robot status", "#INSPVAXA,USB3,0,45.5,FINESTEERING,2113,382049.950,02000000,471d,15824;INS_SOLUTION_GOOD,INS_RTKFIXED,37.37018134102,126.72086464287,9.9295,22.3000,0.0323,0.1808,-0.0017,-0.489634964,-1.152595008,94.076171892,0.1844,0.1184,0.1476,0.0439,0.0341,0.0260,0.0351,0.0379,0.0961,0f000041,0*c13a5434", "robot status", "#INSPVAXA,USB3,0,45.5,FINESTEERING,2113,382050.000,02000000,471d,15824;INS_SOLUTION_GOOD,INS_RTKFIXED,37.37018132968,126.72086473691,9.9296,22.3000,0.0079,0.1780,-0.0077,-0.490765811,-1.141148403,93.892109760,0.1844,0.1184,0.1476,0.0439,0.0341,0.0260,0.0351,0.0379,0.0961,0f000041,0*cea9f920", "robot status", "#INSPVAXA,USB3,0,45.5,FINESTEERING,2113,382050.050,02000000,471d,15824;INS_SOLUTION_GOOD,INS_RTKFIXED,37.37018130962,126.72086482891,9.9297,22.3000,0.0059,0.1822,-0.0050,-0.435162265,-1.162384663,93.644831082,0.1849,0.1198,0.1468,0.0443,0.0350,0.0260,0.0355,0.0380,0.0970,0f000041,0*2ded2fe7", "robot status", "#INSPVAXA,USB3,0,45.5,FINESTEERING,2113,382050.050,02000000,471d,15824;INS_SOLUTION_GOOD,INS_RTKFIXED,37.37018130962,126.72086482891,9.9297,22.3000,0.0059,0.1822,-0.0050,-0.435162265,-1.162384663,93.644831082,0.1849,0.1198,0.1468,0.0443,0.0350,0.0260,0.0355,0.0380,0.0970,0f000041,0*2ded2fe7", "robot status", "#INSPVAXA,USB3,0,44.5,FINESTEERING,2113,382050.150,02000000,471d,15824;INS_SOLUTION_GOOD,INS_RTKFIXED,37.37018126818,126.72086502025,9.9301,22.3000,0.0133,0.1897,0.0076,-0.387085282,-1.194958607,93.062153086,0.1849,0.1198,0.1468,0.0443,0.0350,0.0260,0.0355,0.0380,0.0970,0f000041,0*d76b09ad", "robot status", "#INSPVAXA,USB3,0,44.5,FINESTEERING,2113,382050.200,02000000,471d,15824;INS_SOLUTION_GOOD,INS_RTKFIXED,37.37018124809,126.72086511888,9.9307,22.3000,0.0095,0.1972,-0.0001,-0.337244182,-1.229905011,92.899531373,0.1849,0.1198,0.1468,0.0443,0.0350,0.0260,0.0355,0.0380,0.0970,0f000041,0*aba23f29", "robot status", "#INSPVAXA,USB3,0,44.5,FINESTEERING,2113,382050.250,02000000,471d,15824;INS_SOLUTION_GOOD,INS_RTKFIXED,37.37018123041,126.72086522148,9.9308,22.3000,0.0228,0.2020,-0.0066,-0.266186102,-1.194717685,92.764319307,0.1849,0.1198,0.1468,0.0443,0.0350,0.0260,0.0355,0.0380,0.0970,0f000041,0*5206b714", "robot status", "#INSPVAXA,USB3,0,44.5,FINESTEERING,2113,382050.250,02000000,471d,15824;INS_SOLUTION_GOOD,INS_RTKFIXED,37.37018123041,126.72086522148,9.9308,22.3000,0.0228,0.2020,-0.0066,-0.266186102,-1.194717685,92.764319307,0.1849,0.1198,0.1468,0.0443,0.0350,0.0260,0.0355,0.0380,0.0970,0f000041,0*5206b714", "robot status", "#INSPVAXA,USB3,0,44.5,FINESTEERING,2113,382050.350,02000000,471d,15824;INS_SOLUTION_GOOD,INS_RTKFIXED,37.37018119962,126.72086541685,9.9316,22.3000,0.0196,0.1773,-0.0058,-0.256234743,-1.191471983,92.415710953,0.1849,0.1198,0.1468,0.0443,0.0350,0.0260,0.0355,0.0380,0.0970,0f000041,0*a780f33b", "robot status", "#INSPVAXA,USB3,0,44.5,FINESTEERING,2113,382050.400,02000000,471d,15824;INS_SOLUTION_GOOD,INS_RTKFIXED,37.37018118113,126.72086550221,9.9320,22.3000,0.0051,0.1623,0.0044,-0.229268957,-1.196420514,92.170492785,0.1849,0.1198,0.1468,0.0443,0.0350,0.0260,0.0355,0.0380,0.0970,0f000041,0*19cc5693", "robot status", "#INSPVAXA,USB3,0,44.5,FINESTEERING,2113,382050.450,02000000,471d,15824;INS_SOLUTION_GOOD,INS_RTKFIXED,37.37018115486,126.72086558048,9.9322,22.3000,0.0054,0.1548,-0.0022,-0.180579571,-1.128593844,91.952964787,0.1849,0.1198,0.1468,0.0443,0.0350,0.0260,0.0355,0.0380,0.0970,0f000041,0*ebdf7eab", "robot status", "#INSPVAXA,USB3,0,44.5,FINESTEERING,2113,382050.450,02000000,471d,15824;INS_SOLUTION_GOOD,INS_RTKFIXED,37.37018115486,126.72086558048,9.9322,22.3000,0.0054,0.1548,-0.0022,-0.180579571,-1.128593844,91.952964787,0.1849,0.1198,0.1468,0.0443,0.0350,0.0260,0.0355,0.0380,0.0970,0f000041,0*ebdf7eab", "robot status", "#INSPVAXA,USB3,0,44.5,FINESTEERING,2113,382050.550,02000000,471d,15824;INS_SOLUTION_GOOD,INS_RTKFIXED,37.37018113121,126.72086574007,9.9329,22.3000,0.0399,0.1642,-0.0063,-0.184853935,-1.124001014,91.582935033,0.1849,0.1198,0.1468,0.0443,0.0350,0.0260,0.0355,0.0380,0.0970,0f000041,0*277afedf", "robot status", "#INSPVAXA,USB3,0,44.5,FINESTEERING,2113,382050.600,02000000,471d,15824;INS_SOLUTION_GOOD,INS_RTKFIXED,37.37018112423,126.72086582234,9.9332,22.3000,0.0320,0.1612,0.0080,-0.201336111,-1.132555013,91.415878382,0.1849,0.1198,0.1468,0.0443,0.0350,0.0260,0.0355,0.0380,0.0970,0f000041,0*36de1878", "robot status", "#INSPVAXA,USB3,0,44.5,FINESTEERING,2113,382050.650,02000000,471d,15824;INS_SOLUTION_GOOD,INS_RTKFIXED,37.37018110676,126.72086590086,9.9339,22.3000,0.0138,0.1571,-0.0005,-0.212659413,-1.048142277,91.271099466,0.1849,0.1198,0.1468,0.0443,0.0350,0.0260,0.0355,0.0380,0.0970,0f000041,0*502affa9", "robot status", "#INSPVAXA,USB3,0,44.5,FINESTEERING,2113,382050.700,02000000,471d,15824;INS_SOLUTION_GOOD,INS_RTKFIXED,37.37018109022,126.72086597967,9.9340,22.3000,0.0180,0.1564,-0.0048,-0.202371792,-0.963931490,91.076293796,0.1849,0.1198,0.1468,0.0443,0.0350,0.0260,0.0355,0.0380,0.0970,0f000041,0*51ad9123", "robot status", "#INSPVAXA,USB3,0,44.5,FINESTEERING,2113,382050.750,02000000,471d,15824;INS_SOLUTION_GOOD,INS_RTKFIXED,37.37018107558,126.72086605847,9.9342,22.3000,0.0175,0.1561,-0.0024,-0.236316662,-0.929648674,90.830399127,0.1849,0.1198,0.1468,0.0443,0.0350,0.0260,0.0355,0.0380,0.0970,0f000041,0*d0a9e9c1", "robot status", "#INSPVAXA,USB3,0,44.5,FINESTEERING,2113,382050.800,02000000,471d,15824;INS_SOLUTION_GOOD,INS_RTKFIXED,37.37018106072,126.72086613522,9.9345,22.3000,0.0179,0.1499,0.0004,-0.272198453,-0.873462394,90.558205191,0.1849,0.1198,0.1468,0.0443,0.0350,0.0260,0.0355,0.0380,0.0970,0f000041,0*03d11443", "robot status", "#INSPVAXA,USB3,0,44.5,FINESTEERING,2113,382050.850,02000000,471d,15824;INS_SOLUTION_GOOD,INS_RTKFIXED,37.37018104795,126.72086621185,9.9348,22.3000,0.0251,0.1544,0.0000,-0.259833918,-0.916884009,90.379072251,0.1849,0.1198,0.1468,0.0443,0.0350,0.0260,0.0355,0.0380,0.0970,0f000041,0*013dd7fc", "robot status", "#INSPVAXA,USB3,0,44.5,FINESTEERING,2113,382050.900,02000000,471d,15824;INS_SOLUTION_GOOD,INS_RTKFIXED,37.37018103744,126.72086628903,9.9351,22.3000,0.0403,0.1567,-0.0014,-0.273561712,-0.867845727,90.256795895,0.1849,0.1198,0.1468,0.0443,0.0350,0.0260,0.0355,0.0380,0.0970,0f000041,0*7634b06a", "robot status", "#INSPVAXA,USB3,0,44.5,FINESTEERING,2113,382050.950,02000000,471d,15824;INS_SOLUTION_GOOD,INS_RTKFIXED,37.37018103434,126.72086636887,9.9357,22.3000,0.0408,0.1580,0.0069,-0.324644104,-0.883840391,90.114974929,0.1849,0.1198,0.1468,0.0443,0.0350,0.0260,0.0355,0.0380,0.0970,0f000041,0*fa7ba641", "robot status", "#INSPVAXA,USB3,0,44.5,FINESTEERING,2113,382051.000,02000000,471d,15824;INS_SOLUTION_GOOD,INS_RTKFIXED,37.37018102502,126.72086644623,9.9361,22.3000,0.0169,0.1468,-0.0053,-0.442705799,-0.815306344,89.900536425,0.1849,0.1198,0.1468,0.0443,0.0350,0.0260,0.0355,0.0380,0.0970,0f000041,0*7fffac76", "robot status", "#INSPVAXA,USB3,0,44.5,FINESTEERING,2113,382051.050,02000000,471d,15824;INS_SOLUTION_GOOD,INS_RTKFIXED,37.37018100203,126.72086651607,9.9365,22.3000,0.0072,0.1382,0.0038,-0.420034648,-0.789508624,89.562696335,0.1851,0.1217,0.1459,0.0445,0.0358,0.0260,0.0359,0.0382,0.0978,0f000041,0*304a6888", "robot status", "#INSPVAXA,USB3,0,45.5,FINESTEERING,2113,382051.100,02000000,471d,15824;INS_SOLUTION_GOOD,INS_RTKFIXED,37.37018097873,126.72086658429,9.9368,22.3000,-0.0019,0.1306,-0.0049,-0.464673244,-0.744055356,89.229838566,0.1851,0.1217,0.1459,0.0445,0.0358,0.0260,0.0359,0.0382,0.0978,0f000041,0*8fd9c7a4", "robot status", "#INSPVAXA,USB3,0,45.5,FINESTEERING,2113,382051.150,02000000,471d,15824;INS_SOLUTION_GOOD,INS_RTKFIXED,37.37018095311,126.72086664895,9.9371,22.3000,-0.0025,0.1272,0.0083,-0.381713978,-0.709357994,88.813680377,0.1851,0.1217,0.1459,0.0445,0.0358,0.0260,0.0359,0.0382,0.0978,0f000041,0*65136cc2", "robot status", "#INSPVAXA,USB3,0,45.5,FINESTEERING,2113,382051.200,02000000,471d,15824;INS_SOLUTION_GOOD,INS_RTKFIXED,37.37018092901,126.72086671527,9.9376,22.3000,0.0027,0.1344,-0.0006,-0.409857320,-0.716858961,88.535610087,0.1851,0.1217,0.1459,0.0445,0.0358,0.0260,0.0359,0.0382,0.0978,0f000041,0*832b7b60", "robot status", "#INSPVAXA,USB3,0,45.5,FINESTEERING,2113,382051.250,02000000,471d,15824;INS_SOLUTION_GOOD,INS_RTKFIXED,37.37018090495,126.72086678410,9.9378,22.3000,0.0141,0.1418,0.0003,-0.349653583,-0.702932311,88.195432157,0.1851,0.1217,0.1459,0.0445,0.0358,0.0260,0.0359,0.0382,0.0978,0f000041,0*713cfa67", "robot status", "#INSPVAXA,USB3,0,45.5,FINESTEERING,2113,382051.300,02000000,471d,15824;INS_SOLUTION_GOOD,INS_RTKFIXED,37.37018088806,126.72086685897,9.9382,22.3000,0.0157,0.1487,0.0018,-0.384110139,-0.710509274,87.914151991,0.1851,0.1217,0.1459,0.0445,0.0358,0.0260,0.0359,0.0382,0.0978,0f000041,0*af6142b4", "robot status", "#INSPVAXA,USB3,0,45.5,FINESTEERING,2113,382051.350,02000000,471d,15824;INS_SOLUTION_GOOD,INS_RTKFIXED,37.37018087139,126.72086693427,9.9385,22.3000,0.0158,0.1459,0.0032,-0.366710551,-0.673352368,87.625481317,0.1851,0.1217,0.1459,0.0445,0.0358,0.0260,0.0359,0.0382,0.0978,0f000041,0*e4cc7965", "robot status", "#INSPVAXA,USB3,0,45.5,FINESTEERING,2113,382051.400,02000000,471d,15824;INS_SOLUTION_GOOD,INS_RTKFIXED,37.37018085780,126.72086700977,9.9389,22.3000,0.0266,0.1490,-0.0052,-0.440000688,-0.585115962,87.376687522,0.1851,0.1217,0.1459,0.0445,0.0358,0.0260,0.0359,0.0382,0.0978,0f000041,0*8faff436", "robot status", "#INSPVAXA,USB3,0,45.5,FINESTEERING,2113,382051.450,02000000,471d,15824;INS_SOLUTION_GOOD,INS_RTKFIXED,37.37018084613,126.72086708594,9.9390,22.3000,0.0245,0.1505,0.0024,-0.427569695,-0.557040776,87.076465613,0.1851,0.1217,0.1459,0.0445,0.0358,0.0260,0.0359,0.0382,0.0978,0f000041,0*fdbed822", "robot status", "#INSPVAXA,USB3,0,45.5,FINESTEERING,2113,382051.500,02000000,471d,15824;INS_SOLUTION_GOOD,INS_RTKFIXED,37.37018082574,126.72086716151,9.9395,22.3000,0.0074,0.1481,0.0007,-0.459304805,-0.555384832,86.760746120,0.1851,0.1217,0.1459,0.0445,0.0358,0.0260,0.0359,0.0382,0.0978,0f000041,0*0d6f9cf0", "robot status", "#INSPVAXA,USB3,0,45.5,FINESTEERING,2113,382051.550,02000000,471d,15824;INS_SOLUTION_GOOD,INS_RTKFIXED,37.37018080569,126.72086723831,9.9397,22.3000,0.0075,0.1504,-0.0037,-0.430325659,-0.541577150,86.427058208,0.1851,0.1217,0.1459,0.0445,0.0358,0.0260,0.0359,0.0382,0.0978,0f000041,0*3a27e988", "robot status", "#DUALANTENNAHEADINGA,USB3,0,45.5,FINESTEERING,2113,382051.600,02000000,d426,15824;SOL_COMPUTED,NARROW_INT,-1.000000000,91.200332642,-12.874969482,0.0,0.502065778,0.941429377,\"681H\",36,27,27,20,04,00,30,33*78bc3ed3", "robot status", "#INSPVAXA,USB3,0,45.5,FINESTEERING,2113,382051.650,02000000,471d,15824;INS_SOLUTION_GOOD,INS_RTKFIXED,37.37018078104,126.72086740003,9.9401,22.3000,0.0435,0.1576,-0.0006,-0.438446356,-0.531007552,85.881078044,0.1851,0.1217,0.1459,0.0445,0.0358,0.0260,0.0359,0.0382,0.0978,0f000041,0*0d8e5d0a", "robot status", "#INSPVAXA,USB3,0,45.5,FINESTEERING,2113,382051.700,02000000,471d,15824;INS_SOLUTION_GOOD,INS_RTKFIXED,37.37018077493,126.72086748008,9.9405,22.3000,0.0279,0.1503,0.0038,-0.474447572,-0.504595474,85.635007812,0.1851,0.1217,0.1459,0.0445,0.0358,0.0260,0.0359,0.0382,0.0978,0f000041,0*36c59d27", "robot status", "#INSPVAXA,USB3,0,45.5,FINESTEERING,2113,382051.750,02000000,471d,15824;INS_SOLUTION_GOOD,INS_RTKFIXED,37.37018076363,126.72086755522,9.9410,22.3000,0.0205,0.1437,0.0031,-0.468173380,-0.413955005,85.389353825,0.1851,0.1217,0.1459,0.0445,0.0358,0.0260,0.0359,0.0382,0.0978,0f000041,0*574bce3f", "robot status", "#DUALANTENNAHEADINGA,USB3,0,45.5,FINESTEERING,2113,382051.800,02000000,d426,15824;SOL_COMPUTED,NARROW_INT,-1.000000000,90.446022034,-12.705749512,0.0,0.504162908,0.942347586,\"681H\",35,27,27,20,04,00,30,33*0a4ce294", "robot status", "#INSPVAXA,USB3,0,45.5,FINESTEERING,2113,382051.850,02000000,471d,15824;INS_SOLUTION_GOOD,INS_RTKFIXED,37.37018074287,126.72086771243,9.9416,22.3000,0.0380,0.1598,0.0111,-0.426875222,-0.381991351,84.856929899,0.1851,0.1217,0.1459,0.0445,0.0358,0.0260,0.0359,0.0382,0.0978,0f000041,0*284d57f5", "robot status", "#INSPVAXA,USB3,0,45.5,FINESTEERING,2113,382051.900,02000000,471d,15824;INS_SOLUTION_GOOD,INS_RTKFIXED,37.37018073593,126.72086780079,9.9420,22.3000,0.0425,0.1769,-0.0070,-0.502325145,-0.389753898,84.700003332,0.1851,0.1217,0.1459,0.0445,0.0358,0.0260,0.0359,0.0382,0.0978,0f000041,0*606ad4ed", "robot status", "#INSPVAXA,USB3,0,45.5,FINESTEERING,2113,382051.950,02000000,471d,15824;INS_SOLUTION_GOOD,INS_RTKFIXED,37.37018073582,126.72086789503,9.9422,22.3000,0.0503,0.1842,0.0070,-0.468060598,-0.421916297,84.515093743,0.1851,0.1217,0.1459,0.0445,0.0358,0.0260,0.0359,0.0382,0.0978,0f000041,0*65b531b7", "robot status", "#DUALANTENNAHEADINGA,USB3,0,45.5,FINESTEERING,2113,382052.000,02000000,d426,15824;SOL_COMPUTED,NARROW_INT,-1.000000000,89.847023010,-12.895446777,0.0,0.504291773,0.940064251,\"681H\",36,27,27,20,04,00,30,33*1b6b92b9", "robot status", "#INSPVAXA,USB3,0,45.5,FINESTEERING,2113,382052.050,02000000,471d,15824;INS_SOLUTION_GOOD,INS_RTKFIXED,37.37018073261,126.72086808973,9.9428,22.3000,0.0476,0.1794,0.0007,-0.538984490,-0.348212852,84.222396666,0.1844,0.1241,0.1444,0.0447,0.0367,0.0259,0.0362,0.0382,0.0987,0f000041,0*1044515d", "robot status", "#INSPVAXA,USB3,0,46.0,FINESTEERING,2113,382052.100,02000000,471d,15824;INS_SOLUTION_GOOD,INS_RTKFIXED,37.37018072753,126.72086817872,9.9429,22.3000,0.0358,0.1618,-0.0041,-0.537605028,-0.347272605,84.080967185,0.1844,0.1241,0.1444,0.0447,0.0367,0.0259,0.0362,0.0382,0.0987,0f000041,0*e8da5ef5", "robot status", "#INSPVAXA,USB3,0,46.0,FINESTEERING,2113,382052.150,02000000,471d,15824;INS_SOLUTION_GOOD,INS_RTKFIXED,37.37018071877,126.72086825415,9.9430,22.3000,0.0326,0.1288,-0.0013,-0.516640890,-0.342626933,84.006257748,0.1844,0.1241,0.1444,0.0447,0.0367,0.0259,0.0362,0.0382,0.0987,0f000041,0*bdd80b0a", "robot status", "#DUALANTENNAHEADINGA,USB3,0,46.0,FINESTEERING,2113,382052.200,02000000,d426,15824;SOL_COMPUTED,NARROW_INT,-1.000000000,89.707420349,-11.955627441,0.0,0.504837215,0.945536554,\"681H\",36,28,28,21,04,00,30,33*8b800c43", "robot status", "#INSPVAXA,USB3,0,46.0,FINESTEERING,2113,382052.250,02000000,471d,15824;INS_SOLUTION_GOOD,INS_RTKFIXED,37.37018070790,126.72086833066,9.9436,22.3000,0.0467,0.0390,-0.0077,-0.526836690,-0.439737948,84.774174189,0.1844,0.1241,0.1444,0.0447,0.0367,0.0259,0.0362,0.0382,0.0987,0f000041,0*f5b90d33", "robot status", "#INSPVAXA,USB3,0,46.0,FINESTEERING,2113,382052.300,02000000,471d,15824;INS_SOLUTION_GOOD,INS_RTKFIXED,37.37018070196,126.72086833442,9.9433,22.3000,0.0280,-0.0010,-0.0019,-0.596431136,-0.451726301,84.695125504,0.1844,0.1241,0.1444,0.0447,0.0367,0.0259,0.0362,0.0382,0.0987,0f000041,0*fd9af9e0", "robot status", "#INSPVAXA,USB3,0,46.0,FINESTEERING,2113,382052.350,02000000,471d,15824;INS_SOLUTION_GOOD,INS_RTKFIXED,37.37018069117,126.72086831966,9.9438,22.3000,0.0294,-0.0261,0.0035,-0.499897801,-0.422580103,84.472174360,0.1844,0.1241,0.1444,0.0447,0.0367,0.0259,0.0362,0.0382,0.0987,0f000041,0*36b5961f", "robot status", "#DUALANTENNAHEADINGA,USB3,0,46.0,FINESTEERING,2113,382052.400,02000000,d426,15824;SOL_COMPUTED,NARROW_INT,-1.000000000,89.961700439,-12.154754639,0.0,0.503814876,0.948016882,\"681H\",36,28,28,21,04,00,30,33*b35dea40", "robot status", "#INSPVAXA,USB3,0,46.0,FINESTEERING,2113,382052.450,02000000,471d,15824;INS_SOLUTION_GOOD,INS_RTKFIXED,37.37018066615,126.72086825732,9.9441,22.3000,0.0196,-0.0481,-0.0024,-0.562344990,-0.397818625,84.675806077,0.1844,0.1241,0.1444,0.0447,0.0367,0.0259,0.0362,0.0382,0.0987,0f000041,0*2891a571", "robot status", "#INSPVAXA,USB3,0,46.0,FINESTEERING,2113,382052.500,02000000,471d,15824;INS_SOLUTION_GOOD,INS_RTKFIXED,37.37018065330,126.72086822544,9.9441,22.3000,0.0243,-0.0394,0.0018,-0.522331775,-0.384220270,84.565201848,0.1844,0.1241,0.1444,0.0447,0.0367,0.0259,0.0362,0.0382,0.0987,0f000041,0*e0d85e99", "robot status", "#INSPVAXA,USB3,0,46.0,FINESTEERING,2113,382052.550,02000000,471d,15824;INS_SOLUTION_GOOD,INS_RTKFIXED,37.37018064425,126.72086819970,9.9443,22.3000,0.0325,-0.0259,-0.0019,-0.535554134,-0.372070987,84.541288817,0.1844,0.1241,0.1444,0.0447,0.0367,0.0259,0.0362,0.0382,0.0987,0f000041,0*eb8ba849", "robot status", "#DUALANTENNAHEADINGA,USB3,0,46.0,FINESTEERING,2113,382052.600,02000000,d426,15824;SOL_COMPUTED,NARROW_INT,-1.000000000,90.250518799,-12.286987305,0.0,0.509872377,0.963131726,\"681H\",36,28,28,21,04,00,30,33*b2de7fd5", "robot status", "#INSPVAXA,USB3,0,46.0,FINESTEERING,2113,382052.650,02000000,471d,15824;INS_SOLUTION_GOOD,INS_RTKFIXED,37.37018062125,126.72086817136,9.9447,22.3000,0.0247,-0.0023,-0.0013,-0.534550076,-0.378355923,84.580026911,0.1844,0.1241,0.1444,0.0447,0.0367,0.0259,0.0362,0.0382,0.0987,0f000041,0*7bb01d9a", "robot status", "#DUALANTENNAHEADINGA,USB3,0,46.0,FINESTEERING,2113,382052.700,02000000,d426,15824;SOL_COMPUTED,NARROW_INT,-1.000000000,90.108192444,-12.658966064,0.0,0.506707370,0.954566121,\"681H\",36,28,28,21,04,00,30,33*a21dce10", "robot status", "#INSPVAXA,USB3,0,46.0,FINESTEERING,2113,382052.750,02000000,471d,15824;INS_SOLUTION_GOOD,INS_RTKFIXED,37.37018060475,126.72086815034,9.9450,22.3000,0.0278,-0.0114,-0.0005,-0.551485032,-0.387253774,84.609360453,0.1844,0.1241,0.1444,0.0447,0.0367,0.0259,0.0362,0.0382,0.0987,0f000041,0*5a756de1", "robot status", "#DUALANTENNAHEADINGA,USB3,0,46.0,FINESTEERING,2113,382052.800,02000000,d426,15824;SOL_COMPUTED,NARROW_INT,-1.000000000,90.319557190,-12.106506348,0.0,0.505696654,0.957320929,\"681H\",36,28,28,21,04,00,30,33*59bf7502", "robot status", "#INSPVAXA,USB3,0,46.0,FINESTEERING,2113,382052.850,02000000,471d,15824;INS_SOLUTION_GOOD,INS_RTKFIXED,37.37018058477,126.72086811847,9.9453,22.3000,0.0259,-0.0195,0.0000,-0.534953434,-0.382624380,84.591784393,0.1844,0.1241,0.1444,0.0447,0.0367,0.0259,0.0362,0.0382,0.0987,0f000041,0*275d6a88", "robot status", "#DUALANTENNAHEADINGA,USB3,0,46.0,FINESTEERING,2113,382052.900,02000000,d426,15824;SOL_COMPUTED,NARROW_INT,-1.000000000,90.238014221,-12.982330322,0.0,0.507720888,0.955418169,\"681H\",36,28,28,21,04,00,30,33*d29b1b06", "robot status", "#INSPVAXA,USB3,0,46.0,FINESTEERING,2113,382052.950,02000000,471d,15824;INS_SOLUTION_GOOD,INS_RTKFIXED,37.37018056378,126.72086808606,9.9457,22.3000,0.0245,-0.0125,0.0004,-0.541796060,-0.381889944,84.582768054,0.1844,0.1241,0.1444,0.0447,0.0367,0.0259,0.0362,0.0382,0.0987,0f000041,0*3cd6b34e", "robot status", "#DUALANTENNAHEADINGA,USB3,0,46.0,FINESTEERING,2113,382053.000,02000000,d426,15824;SOL_COMPUTED,NARROW_INT,-1.000000000,90.194465637,-12.220642090,0.0,0.508546054,0.963238716,\"681H\",35,27,27,20,04,00,30,33*732b77ad", "robot status", "#INSPVAXA,USB3,0,46.0,FINESTEERING,2113,382053.050,02000000,471d,15824;INS_SOLUTION_GOOD,INS_RTKFIXED,37.37018054061,126.72086806082,9.9460,22.3000,0.0251,-0.0156,0.0000,-0.540367925,-0.383885063,84.598379103,0.1847,0.1275,0.1440,0.0449,0.0374,0.0260,0.0364,0.0383,0.0994,0f000041,0*f29a6df3", "robot status", "#DUALANTENNAHEADINGA,USB3,0,46.0,FINESTEERING,2113,382053.100,02000000,d426,15824;SOL_COMPUTED,NARROW_INT,-1.000000000,90.188461304,-12.512664795,0.0,0.513727963,0.973524988,\"681H\",36,27,27,20,04,00,30,33*538bceab", "robot status", "#INSPVAXA,USB3,0,46.0,FINESTEERING,2113,382053.150,02000000,471d,15824;INS_SOLUTION_GOOD,INS_RTKFIXED,37.37018051973,126.72086804093,9.9463,22.3000,0.0225,-0.0166,-0.0001,-0.539967903,-0.380388346,84.598287837,0.1847,0.1275,0.1440,0.0449,0.0374,0.0260,0.0364,0.0383,0.0994,0f000041,0*1f4aaea2", "robot status", "#DUALANTENNAHEADINGA,USB3,0,46.0,FINESTEERING,2113,382053.200,02000000,d426,15824;SOL_COMPUTED,NARROW_INT,-1.000000000,90.062850952,-12.819946289,0.0,0.516938269,0.976916850,\"681H\",35,24,24,20,04,00,30,33*150a9e2f", "robot status", "#INSPVAXA,USB3,0,46.0,FINESTEERING,2113,382053.250,02000000,471d,15824;INS_SOLUTION_GOOD,INS_RTKFIXED,37.37018049617,126.72086802276,9.9466,22.3000,0.0241,-0.0145,0.0001,-0.538948993,-0.381673142,84.592459360,0.1847,0.1275,0.1440,0.0449,0.0374,0.0260,0.0364,0.0383,0.0994,0f000041,0*352d146b", "robot status", "#DUALANTENNAHEADINGA,USB3,0,46.0,FINESTEERING,2113,382053.300,02000000,d426,15824;SOL_COMPUTED,NARROW_INT,-1.000000000,90.156661987,-13.009857178,0.0,0.515168965,0.973820329,\"681H\",35,24,24,20,04,00,30,33*c845c594", "robot status", "#INSPVAXA,USB3,0,46.0,FINESTEERING,2113,382053.350,02000000,471d,15824;INS_SOLUTION_GOOD,INS_RTKFIXED,37.37018047554,126.72086800377,9.9469,22.3000,0.0218,-0.0172,0.0003,-0.536398191,-0.380594093,84.593113983,0.1847,0.1275,0.1440,0.0449,0.0374,0.0260,0.0364,0.0383,0.0994,0f000041,0*8522b6a2", "robot status", "#DUALANTENNAHEADINGA,USB3,0,46.0,FINESTEERING,2113,382053.400,02000000,d426,15824;SOL_COMPUTED,NARROW_INT,-1.000000000,90.003448486,-12.996765137,0.0,0.509641051,0.964000881,\"681H\",35,24,24,20,04,00,30,33*9487bed1", "robot status", "#INSPVAXA,USB3,0,46.0,FINESTEERING,2113,382053.450,02000000,471d,15824;INS_SOLUTION_GOOD,INS_RTKFIXED,37.37018045249,126.72086798352,9.9472,22.3000,0.0220,-0.0159,0.0005,-0.537349033,-0.379636502,84.595391126,0.1847,0.1275,0.1440,0.0449,0.0374,0.0260,0.0364,0.0383,0.0994,0f000041,0*58a681c3", "robot status", "#DUALANTENNAHEADINGA,USB3,0,46.0,FINESTEERING,2113,382053.500,02000000,d426,15824;SOL_COMPUTED,NARROW_INT,-1.000000000,90.136512756,-12.748596191,0.0,0.510926664,0.968839943,\"681H\",35,24,24,20,04,00,30,33*844b6c7c", "robot status", "#INSPVAXA,USB3,0,46.0,FINESTEERING,2113,382053.550,02000000,471d,15824;INS_SOLUTION_GOOD,INS_RTKFIXED,37.37018043218,126.72086796480,9.9474,22.3000,0.0213,-0.0167,0.0003,-0.536431745,-0.380837636,84.598477176,0.1847,0.1275,0.1440,0.0449,0.0374,0.0260,0.0364,0.0383,0.0994,0f000041,0*4fd36ed4", "robot status", "#DUALANTENNAHEADINGA,USB3,0,46.0,FINESTEERING,2113,382053.600,02000000,d426,15824;SOL_COMPUTED,NARROW_INT,-1.000000000,90.071426392,-12.335327148,0.0,0.514146507,0.976225972,\"681H\",35,24,24,20,04,00,30,33*6a6e223c", "robot status", "#INSPVAXA,USB3,0,46.0,FINESTEERING,2113,382053.650,02000000,471d,15824;INS_SOLUTION_GOOD,INS_RTKFIXED,37.37018040898,126.72086794441,9.9477,22.3000,0.0197,-0.0171,0.0001,-0.536182692,-0.380283801,84.595463591,0.1847,0.1275,0.1440,0.0449,0.0374,0.0260,0.0364,0.0383,0.0994,0f000041,0*b99c192b", "robot status", "#DUALANTENNAHEADINGA,USB3,0,46.0,FINESTEERING,2113,382053.700,02000000,d426,15824;SOL_COMPUTED,NARROW_INT,-1.000000000,90.132423401,-12.745422363,0.0,0.511970282,0.971639693,\"681H\",35,24,24,20,04,00,30,33*e638bd3d", "robot status", "#INSPVAXA,USB3,0,46.0,FINESTEERING,2113,382053.750,02000000,471d,15824;INS_SOLUTION_GOOD,INS_RTKFIXED,37.37018038880,126.72086792486,9.9480,22.3000,0.0200,-0.0160,0.0002,-0.536003121,-0.380556679,84.595595957,0.1847,0.1275,0.1440,0.0449,0.0374,0.0260,0.0364,0.0383,0.0994,0f000041,0*069c343b", "robot status", "#DUALANTENNAHEADINGA,USB3,0,46.0,FINESTEERING,2113,382053.800,02000000,d426,15824;SOL_COMPUTED,NARROW_INT,-1.000000000,90.168548584,-12.345092773,0.0,0.509989262,0.971799135,\"681H\",35,24,24,20,04,00,30,33*51bc5b61", "robot status", "#INSPVAXA,USB3,0,46.0,FINESTEERING,2113,382053.850,02000000,471d,15824;INS_SOLUTION_GOOD,INS_RTKFIXED,37.37018036844,126.72086790490,9.9483,22.3000,0.0180,-0.0170,0.0008,-0.535597521,-0.379163305,84.598217615,0.1847,0.1275,0.1440,0.0449,0.0374,0.0260,0.0364,0.0383,0.0994,0f000041,0*c4b09d16", "robot status", "#DUALANTENNAHEADINGA,USB3,0,46.0,FINESTEERING,2113,382053.900,02000000,d426,15824;SOL_COMPUTED,NARROW_INT,-1.000000000,90.044799805,-12.915191650,0.0,0.510914207,0.966265976,\"681H\",35,24,24,20,04,00,30,33*641dbe82", "robot status", "#INSPVAXA,USB3,0,46.0,FINESTEERING,2113,382053.950,02000000,471d,15824;INS_SOLUTION_GOOD,INS_RTKFIXED,37.37018034512,126.72086788442,9.9485,22.3000,0.0178,-0.0164,0.0005,-0.534980038,-0.378397505,84.598844386,0.1847,0.1275,0.1440,0.0449,0.0374,0.0260,0.0364,0.0383,0.0994,0f000041,0*4bfff5fd", "robot status", "#DUALANTENNAHEADINGA,USB3,0,46.0,FINESTEERING,2113,382054.000,02000000,d426,15824;SOL_COMPUTED,NARROW_INT,-1.000000000,90.102714539,-12.857177734,0.0,0.510702372,0.967817128,\"681H\",35,24,24,20,04,00,30,33*ab7d5ad0", "robot status", "#INSPVAXA,USB3,0,44.5,FINESTEERING,2113,382054.050,02000000,471d,15824;INS_SOLUTION_GOOD,INS_RTKFIXED,37.37018032182,126.72086786852,9.9488,22.3000,0.0168,-0.0168,0.0005,-0.535000639,-0.378640424,84.598782946,0.1852,0.1302,0.1441,0.0451,0.0377,0.0260,0.0365,0.0384,0.1002,0f000041,0*d30a7a50", "robot status", "#DUALANTENNAHEADINGA,USB3,0,44.5,FINESTEERING,2113,382054.100,02000000,d426,15824;SOL_COMPUTED,NARROW_INT,-1.000000000,89.978111267,-12.950775146,0.0,0.505953074,0.958189487,\"681H\",35,24,24,20,04,00,30,33*654bb38b", "robot status", "#INSPVAXA,USB3,0,44.5,FINESTEERING,2113,382054.150,02000000,471d,15824;INS_SOLUTION_GOOD,INS_RTKFIXED,37.37018030255,126.72086785971,9.9490,22.3000,0.0158,-0.0168,0.0003,-0.535151526,-0.378848426,84.598511770,0.1852,0.1302,0.1441,0.0451,0.0377,0.0260,0.0365,0.0384,0.1002,0f000041,0*00c0e729", "robot status", "#DUALANTENNAHEADINGA,USB3,0,44.5,FINESTEERING,2113,382054.200,02000000,d426,15824;SOL_COMPUTED,NARROW_INT,-1.000000000,90.194099426,-13.238220215,0.0,0.501824796,0.950803638,\"681H\",35,24,24,20,04,00,30,33*b5de2f7b", "robot status", "#INSPVAXA,USB3,0,44.5,FINESTEERING,2113,382054.250,02000000,471d,15824;INS_SOLUTION_GOOD,INS_RTKFIXED,37.37018028094,126.72086785188,9.9492,22.3000,0.0156,-0.0166,0.0003,-0.534463582,-0.380269743,84.600396201,0.1852,0.1302,0.1441,0.0451,0.0377,0.0260,0.0365,0.0384,0.1002,0f000041,0*9dfd8c8e", "robot status", "#DUALANTENNAHEADINGA,USB3,0,44.5,FINESTEERING,2113,382054.300,02000000,d426,15824;SOL_COMPUTED,NARROW_INT,-1.000000000,90.125175476,-12.886657715,0.0,0.507946312,0.962053776,\"681H\",35,24,24,20,04,00,30,33*c799a0cd", "robot status", "#INSPVAXA,USB3,0,44.5,FINESTEERING,2113,382054.350,02000000,471d,15824;INS_SOLUTION_GOOD,INS_RTKFIXED,37.37018026179,126.72086784267,9.9494,22.3000,0.0149,-0.0168,0.0005,-0.534172277,-0.379363148,84.599908153,0.1852,0.1302,0.1441,0.0451,0.0377,0.0260,0.0365,0.0384,0.1002,0f000041,0*5fc3acf1", "robot status", "#DUALANTENNAHEADINGA,USB3,0,44.5,FINESTEERING,2113,382054.400,02000000,d426,15824;SOL_COMPUTED,NARROW_INT,-1.000000000,90.191741943,-13.057891846,0.0,0.507700145,0.961570561,\"681H\",35,24,24,20,04,00,30,33*c52ebca7", "robot status", "#INSPVAXA,USB3,0,44.5,FINESTEERING,2113,382054.450,02000000,471d,15824;INS_SOLUTION_GOOD,INS_RTKFIXED,37.37018024283,126.72086783349,9.9495,22.3000,0.0146,-0.0164,0.0010,-0.534708812,-0.378776474,84.599704993,0.1852,0.1302,0.1441,0.0451,0.0377,0.0260,0.0365,0.0384,0.1002,0f000041,0*361a14eb", "robot status", "#DUALANTENNAHEADINGA,USB3,0,44.5,FINESTEERING,2113,382054.500,02000000,d426,15824;SOL_COMPUTED,NARROW_INT,-1.000000000,90.097595215,-12.789062500,0.0,0.509407640,0.964732945,\"681H\",35,24,24,20,04,00,30,33*edc325d1", "robot status", "#INSPVAXA,USB3,0,44.5,FINESTEERING,2113,382054.550,02000000,471d,15824;INS_SOLUTION_GOOD,INS_RTKFIXED,37.37018022161,126.72086782479,9.9497,22.3000,0.0141,-0.0170,0.0007,-0.534039460,-0.379688671,84.600550831,0.1852,0.1302,0.1441,0.0451,0.0377,0.0260,0.0365,0.0384,0.1002,0f000041,0*eb9572e3", "robot status", "#DUALANTENNAHEADINGA,USB3,0,44.5,FINESTEERING,2113,382054.600,02000000,d426,15824;SOL_COMPUTED,NARROW_INT,-1.000000000,90.240829468,-12.711303711,0.0,0.506130517,0.957408428,\"681H\",35,24,24,20,04,00,30,33*6cc8485b", "robot status", "#INSPVAXA,USB3,0,44.5,FINESTEERING,2113,382054.650,02000000,471d,15824;INS_SOLUTION_GOOD,INS_RTKFIXED,37.37018020043,126.72086781569,9.9499,22.3000,0.0132,-0.0167,0.0001,-0.534053848,-0.380011226,84.601180012,0.1852,0.1302,0.1441,0.0451,0.0377,0.0260,0.0365,0.0384,0.1002,0f000041,0*a1a8c078", "robot status", "#DUALANTENNAHEADINGA,USB3,0,44.5,FINESTEERING,2113,382054.700,02000000,d426,15824;SOL_COMPUTED,NARROW_INT,-1.000000000,90.039192200,-13.399963379,0.0,0.510455549,0.960306168,\"681H\",35,24,24,20,04,00,30,33*dd58e06a", "robot status", "#INSPVAXA,USB3,0,44.5,FINESTEERING,2113,382054.750,02000000,471d,15824;INS_SOLUTION_GOOD,INS_RTKFIXED,37.37018018167,126.72086780563,9.9500,22.3000,0.0128,-0.0168,0.0004,-0.533634995,-0.381111775,84.601340346,0.1852,0.1302,0.1441,0.0451,0.0377,0.0260,0.0365,0.0384,0.1002,0f000041,0*961452b1", "robot status", "#DUALANTENNAHEADINGA,USB3,0,44.5,FINESTEERING,2113,382054.800,02000000,d426,15824;SOL_COMPUTED,NARROW_INT,-1.000000000,90.193023682,-12.263671875,0.0,0.506186247,0.960428715,\"681H\",35,24,24,20,04,00,30,33*7e271b6c", "robot status", "#INSPVAXA,USB3,0,44.5,FINESTEERING,2113,382054.850,02000000,471d,15824;INS_SOLUTION_GOOD,INS_RTKFIXED,37.37018016269,126.72086779499,9.9502,22.3000,0.0119,-0.0173,0.0008,-0.533216730,-0.381393894,84.601588295,0.1852,0.1302,0.1441,0.0451,0.0377,0.0260,0.0365,0.0384,0.1002,0f000041,0*5eddc917", "robot status", "#DUALANTENNAHEADINGA,USB3,0,44.5,FINESTEERING,2113,382054.900,02000000,d426,15824;SOL_COMPUTED,NARROW_INT,-1.000000000,90.136703491,-13.241729736,0.0,0.504959822,0.949449122,\"681H\",35,24,24,20,04,00,30,33*c6f2e723", "robot status", "#INSPVAXA,USB3,0,44.5,FINESTEERING,2113,382054.950,02000000,471d,15824;INS_SOLUTION_GOOD,INS_RTKFIXED,37.37018014130,126.72086778491,9.9504,22.3000,0.0109,-0.0171,0.0003,-0.532789293,-0.381114669,84.601547678,0.1852,0.1302,0.1441,0.0451,0.0377,0.0260,0.0365,0.0384,0.1002,0f000041,0*12653d6a", "robot status", "#DUALANTENNAHEADINGA,USB3,0,44.5,FINESTEERING,2113,382055.000,02000000,d426,15824;SOL_COMPUTED,NARROW_INT,-1.000000000,89.879066467,-13.172302246,0.0,0.507007837,0.951018929,\"681H\",35,24,24,20,04,00,30,33*ab683dc2", "robot status", "#INSPVAXA,USB3,0,44.5,FINESTEERING,2113,382055.050,02000000,471d,15824;INS_SOLUTION_GOOD,INS_RTKFIXED,37.37018012063,126.72086777605,9.9505,22.3000,0.0105,-0.0173,0.0002,-0.532108608,-0.382082731,84.601207407,0.1856,0.1320,0.1442,0.0453,0.0379,0.0261,0.0364,0.0383,0.1010,0f000041,0*c347ce0f", "robot status", "#DUALANTENNAHEADINGA,USB3,0,44.5,FINESTEERING,2113,382055.100,02000000,d426,15824;SOL_COMPUTED,NARROW_INT,-1.000000000,90.309738159,-12.298400879,0.0,0.503382444,0.952363133,\"681H\",35,24,24,20,04,00,30,33*6811ede3", "robot status", "#INSPVAXA,USB3,0,47.5,FINESTEERING,2113,382055.150,02000000,471d,15824;INS_SOLUTION_GOOD,INS_RTKFIXED,37.37018010491,126.72086776912,9.9504,22.3000,0.0099,-0.0172,0.0005,-0.531075337,-0.383307132,84.600984795,0.1856,0.1320,0.1442,0.0453,0.0379,0.0261,0.0364,0.0383,0.1010,0f000041,0*603a748c", "robot status", "#DUALANTENNAHEADINGA,USB3,0,47.5,FINESTEERING,2113,382055.200,02000000,d426,15824;SOL_COMPUTED,NARROW_INT,-1.000000000,90.014404297,-13.102752686,0.0,0.339669675,0.485382706,\"681H\",35,25,25,21,04,00,30,33*354d98f6", "robot status", "#INSPVAXA,USB3,0,47.5,FINESTEERING,2113,382055.250,02000000,471d,15824;INS_SOLUTION_GOOD,INS_RTKFIXED,37.37018008739,126.72086776297,9.9503,22.3000,0.0094,-0.0174,0.0001,-0.531671647,-0.383555458,84.600072298,0.1856,0.1320,0.1442,0.0453,0.0379,0.0261,0.0364,0.0383,0.1010,0f000041,0*d3b44ffb", "robot status", "#DUALANTENNAHEADINGA,USB3,0,47.5,FINESTEERING,2113,382055.300,02000000,d426,15824;SOL_COMPUTED,NARROW_INT,-1.000000000,90.128822327,-13.147613525,0.0,0.338195920,0.484377682,\"681H\",35,25,25,21,04,00,30,33*498d4c02", "robot status", "#INSPVAXA,USB3,0,47.5,FINESTEERING,2113,382055.350,02000000,471d,15824;INS_SOLUTION_GOOD,INS_RTKFIXED,37.37018007167,126.72086775518,9.9503,22.3000,0.0092,-0.0177,-0.0000,-0.531540673,-0.383926147,84.599772704,0.1856,0.1320,0.1442,0.0453,0.0379,0.0261,0.0364,0.0383,0.1010,0f000041,0*a7723cd6", "robot status", "#DUALANTENNAHEADINGA,USB3,0,47.5,FINESTEERING,2113,382055.400,02000000,d426,15824;SOL_COMPUTED,NARROW_INT,-1.000000000,90.006912231,-13.236480713,0.0,0.339952201,0.486818135,\"681H\",35,25,25,21,04,00,30,33*a5f1a16f", "robot status", "#INSPVAXA,USB3,0,47.5,FINESTEERING,2113,382055.450,02000000,471d,15824;INS_SOLUTION_GOOD,INS_RTKFIXED,37.37018005616,126.72086774717,9.9502,22.3000,0.0088,-0.0177,0.0004,-0.532929555,-0.383765593,84.598867072,0.1856,0.1320,0.1442,0.0453,0.0379,0.0261,0.0364,0.0383,0.1010,0f000041,0*3c3ed412", "robot status", "#DUALANTENNAHEADINGA,USB3,0,47.5,FINESTEERING,2113,382055.500,02000000,d426,15824;SOL_COMPUTED,NARROW_INT,-1.000000000,90.128868103,-12.943328857,0.0,0.339890927,0.488435715,\"681H\",35,25,25,21,04,00,30,33*6ea13429", "robot status", "#INSPVAXA,USB3,0,47.5,FINESTEERING,2113,382055.600,02000000,471d,15824;INS_SOLUTION_GOOD,INS_RTKFIXED,37.37018003124,126.72086773554,9.9500,22.3000,0.0082,-0.0177,-0.0002,-0.532568028,-0.384301986,84.598503020,0.1856,0.1320,0.1442,0.0453,0.0379,0.0261,0.0364,0.0383,0.1010,0f000041,0*4f3e5fba", "robot status", "#DUALANTENNAHEADINGA,USB3,0,47.5,FINESTEERING,2113,382055.600,02000000,d426,15824;SOL_COMPUTED,NARROW_INT,-1.000000000,90.174949646,-13.130096436,0.0,0.347130358,0.499097437,\"681H\",35,25,25,19,04,00,30,33*78bec263", "robot status", "#INSPVAXA,USB3,0,47.5,FINESTEERING,2113,382055.650,02000000,471d,15824;INS_SOLUTION_GOOD,INS_RTKFIXED,37.37018002177,126.72086773197,9.9500,22.3000,0.0080,-0.0177,-0.0001,-0.532269420,-0.384834376,84.599468475,0.1856,0.1320,0.1442,0.0453,0.0379,0.0261,0.0364,0.0383,0.1010,0f000041,0*36d2293a", "robot status", "#DUALANTENNAHEADINGA,USB3,0,47.5,FINESTEERING,2113,382055.700,02000000,d426,15824;SOL_COMPUTED,NARROW_INT,-1.000000000,89.968322754,-13.003784180,0.0,0.345188677,0.496089429,\"681H\",35,25,25,19,04,00,30,33*f827c827", "robot status", "#INSPVAXA,USB3,0,47.5,FINESTEERING,2113,382055.750,02000000,471d,15824;INS_SOLUTION_GOOD,INS_RTKFIXED,37.37018000640,126.72086772310,9.9499,22.3000,0.0076,-0.0179,-0.0002,-0.532414148,-0.384422854,84.599668841,0.1856,0.1320,0.1442,0.0453,0.0379,0.0261,0.0364,0.0383,0.1010,0f000041,0*968f49d1", "robot status", "#DUALANTENNAHEADINGA,USB3,0,47.5,FINESTEERING,2113,382055.800,02000000,d426,15824;SOL_COMPUTED,NARROW_INT,-1.000000000,90.125228882,-13.103637695,0.0,0.354482472,0.505903780,\"681H\",35,24,24,18,04,00,30,33*2f5a6637", "robot status", "#INSPVAXA,USB3,0,47.5,FINESTEERING,2113,382055.850,02000000,471d,15824;INS_SOLUTION_GOOD,INS_RTKFIXED,37.37017999109,126.72086771387,9.9497,22.3000,0.0074,-0.0180,-0.0002,-0.533226978,-0.384292143,84.600327477,0.1856,0.1320,0.1442,0.0453,0.0379,0.0261,0.0364,0.0383,0.1010,0f000041,0*595c6d15", "robot status", "#DUALANTENNAHEADINGA,USB3,0,47.5,FINESTEERING,2113,382055.900,02000000,d426,15824;SOL_COMPUTED,NARROW_INT,-1.000000000,90.013175964,-13.203186035,0.0,0.356469244,0.515609920,\"681H\",35,24,24,18,04,00,30,33*31bc633f", "robot status", "#INSPVAXA,USB3,0,47.5,FINESTEERING,2113,382055.950,02000000,471d,15824;INS_SOLUTION_GOOD,INS_RTKFIXED,37.37017997404,126.72086770484,9.9496,22.3000,0.0068,-0.0184,0.0000,-0.532957220,-0.384357630,84.599504842,0.1856,0.1320,0.1442,0.0453,0.0379,0.0261,0.0364,0.0383,0.1010,0f000041,0*49398e4e", "robot status", "#INSPVAXA,USB3,0,47.0,FINESTEERING,2113,382056.050,02000000,471d,15824;INS_SOLUTION_GOOD,INS_RTKFIXED,37.37017995712,126.72086769776,9.9494,22.3000,0.0064,-0.0183,-0.0005,-0.532256785,-0.384152151,84.600106877,0.1859,0.1330,0.1444,0.0453,0.0379,0.0261,0.0362,0.0381,0.1017,0f000041,0*350aa7d6", "robot status", "#INSPVAXA,USB3,0,47.0,FINESTEERING,2113,382056.050,02000000,471d,15824;INS_SOLUTION_GOOD,INS_RTKFIXED,37.37017995712,126.72086769776,9.9494,22.3000,0.0064,-0.0183,-0.0005,-0.532256785,-0.384152151,84.600106877,0.1859,0.1330,0.1444,0.0453,0.0379,0.0261,0.0362,0.0381,0.1017,0f000041,0*350aa7d6", "robot status", "#DUALANTENNAHEADINGA,USB3,0,47.0,FINESTEERING,2113,382056.100,02000000,d426,15824;SOL_COMPUTED,NARROW_INT,-1.000000000,90.073341370,-12.887145996,0.0,0.356559604,0.531340778,\"681H\",35,23,23,18,04,00,30,33*0c0f24fd", "robot status", "#INSPVAXA,USB3,0,47.0,FINESTEERING,2113,382056.150,02000000,471d,15824;INS_SOLUTION_GOOD,INS_RTKFIXED,37.37017994259,126.72086769340,9.9492,22.3000,0.0059,-0.0184,-0.0004,-0.531768557,-0.383443655,84.600479585,0.1859,0.1330,0.1444,0.0453,0.0379,0.0261,0.0362,0.0381,0.1017,0f000041,0*65792197", "robot status", "#INSPVAXA,USB3,0,47.0,FINESTEERING,2113,382056.250,02000000,471d,15824;INS_SOLUTION_GOOD,INS_RTKFIXED,37.37017992658,126.72086768991,9.9490,22.3000,0.0055,-0.0181,-0.0008,-0.531494121,-0.383750833,84.600759288,0.1859,0.1330,0.1444,0.0453,0.0379,0.0261,0.0362,0.0381,0.1017,0f000041,0*73794056", "robot status", "#INSPVAXA,USB3,0,47.0,FINESTEERING,2113,382056.250,02000000,471d,15824;INS_SOLUTION_GOOD,INS_RTKFIXED,37.37017992658,126.72086768991,9.9490,22.3000,0.0055,-0.0181,-0.0008,-0.531494121,-0.383750833,84.600759288,0.1859,0.1330,0.1444,0.0453,0.0379,0.0261,0.0362,0.0381,0.1017,0f000041,0*73794056", "robot status", "#DUALANTENNAHEADINGA,USB3,0,47.0,FINESTEERING,2113,382056.300,02000000,d426,15824;SOL_COMPUTED,NARROW_INT,-1.000000000,89.984375000,-13.106140137,0.0,0.509437323,0.941881537,\"681H\",35,24,24,19,04,00,30,33*e1e9919c", "robot status", "#INSPVAXA,USB3,0,47.0,FINESTEERING,2113,382056.350,02000000,471d,15824;INS_SOLUTION_GOOD,INS_RTKFIXED,37.37017991198,126.72086768514,9.9488,22.3000,0.0051,-0.0181,-0.0008,-0.531917093,-0.383250002,84.601399322,0.1859,0.1330,0.1444,0.0453,0.0379,0.0261,0.0362,0.0381,0.1017,0f000041,0*5e9a4552", "robot status", "#INSPVAXA,USB3,0,47.0,FINESTEERING,2113,382056.450,02000000,471d,15824;INS_SOLUTION_GOOD,INS_RTKFIXED,37.37017989759,126.72086767991,9.9486,22.3000,0.0052,-0.0185,-0.0013,-0.532061744,-0.383541694,84.600988066,0.1859,0.1330,0.1444,0.0453,0.0379,0.0261,0.0362,0.0381,0.1017,0f000041,0*17bbed00", "robot status", "#INSPVAXA,USB3,0,47.0,FINESTEERING,2113,382056.500,02000000,471d,15824;INS_SOLUTION_GOOD,INS_RTKFIXED,37.37017988900,126.72086767830,9.9484,22.3000,0.0048,-0.0182,-0.0013,-0.531333151,-0.384068393,84.600408408,0.1859,0.1330,0.1444,0.0453,0.0379,0.0261,0.0362,0.0381,0.1017,0f000041,0*d0e55e83", "robot status", "#DUALANTENNAHEADINGA,USB3,0,47.0,FINESTEERING,2113,382056.500,02000000,d426,15824;SOL_COMPUTED,NARROW_INT,-1.000000000,90.150497437,-12.454925537,0.0,0.508783937,0.943969131,\"681H\",35,24,24,19,04,00,30,33*9e052d32", "robot status", "#INSPVAXA,USB3,0,47.0,FINESTEERING,2113,382056.550,02000000,471d,15824;INS_SOLUTION_GOOD,INS_RTKFIXED,37.37017988179,126.72086767554,9.9483,22.3000,0.0047,-0.0180,-0.0013,-0.531813681,-0.384181427,84.601084320,0.1859,0.1330,0.1444,0.0453,0.0379,0.0261,0.0362,0.0381,0.1017,0f000041,0*8768d569", "robot status", "#INSPVAXA,USB3,0,47.0,FINESTEERING,2113,382056.650,02000000,471d,15824;INS_SOLUTION_GOOD,INS_RTKFIXED,37.37017986604,126.72086767110,9.9481,22.3000,0.0042,-0.0180,-0.0010,-0.531748565,-0.384225193,84.601300431,0.1859,0.1330,0.1444,0.0453,0.0379,0.0261,0.0362,0.0381,0.1017,0f000041,0*149cf30c", "robot status", "#INSPVAXA,USB3,0,47.0,FINESTEERING,2113,382056.700,02000000,471d,15824;INS_SOLUTION_GOOD,INS_RTKFIXED,37.37017985885,126.72086766829,9.9479,22.3000,0.0040,-0.0179,-0.0014,-0.531385562,-0.383993428,84.601276168,0.1859,0.1330,0.1444,0.0453,0.0379,0.0261,0.0362,0.0381,0.1017,0f000041,0*e3a1f92b", "robot status", "#DUALANTENNAHEADINGA,USB3,0,47.0,FINESTEERING,2113,382056.700,02000000,d426,15824;SOL_COMPUTED,NARROW_INT,-1.000000000,90.171379089,-12.551879883,0.0,0.507556379,0.946657419,\"681H\",34,24,24,19,04,00,30,33*cb7eb9b4", "robot status", "#INSPVAXA,USB3,0,47.0,FINESTEERING,2113,382056.750,02000000,471d,15824;INS_SOLUTION_GOOD,INS_RTKFIXED,37.37017985170,126.72086766533,9.9478,22.3000,0.0039,-0.0178,-0.0016,-0.532524459,-0.384342429,84.601752358,0.1859,0.1330,0.1444,0.0453,0.0379,0.0261,0.0362,0.0381,0.1017,0f000041,0*130d45c9", "robot status", "#INSPVAXA,USB3,0,47.0,FINESTEERING,2113,382056.850,02000000,471d,15824;INS_SOLUTION_GOOD,INS_RTKFIXED,37.37017983768,126.72086765908,9.9475,22.3000,0.0041,-0.0182,-0.0014,-0.532191408,-0.384646765,84.602217629,0.1859,0.1330,0.1444,0.0453,0.0379,0.0261,0.0362,0.0381,0.1017,0f000041,0*80c911ae", "robot status", "#INSPVAXA,USB3,0,47.0,FINESTEERING,2113,382056.900,02000000,471d,15824;INS_SOLUTION_GOOD,INS_RTKFIXED,37.37017982930,126.72086765716,9.9474,22.3000,0.0038,-0.0177,-0.0017,-0.532418568,-0.384879754,84.602624668,0.1859,0.1330,0.1444,0.0453,0.0379,0.0261,0.0362,0.0381,0.1017,0f000041,0*ea783ce8", "robot status", "#DUALANTENNAHEADINGA,USB3,0,47.0,FINESTEERING,2113,382056.900,02000000,d426,15824;SOL_COMPUTED,NARROW_INT,-1.000000000,89.934776306,-13.292236328,0.0,0.512272537,0.949300468,\"681H\",34,24,24,19,04,00,30,33*126511d8", "robot status", "#INSPVAXA,USB3,0,47.0,FINESTEERING,2113,382056.950,02000000,471d,15824;INS_SOLUTION_GOOD,INS_RTKFIXED,37.37017982238,126.72086765404,9.9472,22.3000,0.0038,-0.0176,-0.0020,-0.531429370,-0.384778189,84.602546045,0.1859,0.1330,0.1444,0.0453,0.0379,0.0261,0.0362,0.0381,0.1017,0f000041,0*7eb925ca", "robot status", "#INSPVAXA,USB3,0,47.0,FINESTEERING,2113,382057.050,02000000,471d,15824;INS_SOLUTION_GOOD,INS_RTKFIXED,37.37017980838,126.72086764960,9.9469,22.3000,0.0035,-0.0177,-0.0015,-0.531216215,-0.385679922,84.602968401,0.1862,0.1335,0.1446,0.0453,0.0379,0.0262,0.0359,0.0378,0.1023,0f000041,0*3ea2aba6", "robot status", "#INSPVAXA,USB3,0,47.0,FINESTEERING,2113,382057.100,02000000,471d,15824;INS_SOLUTION_GOOD,INS_RTKFIXED,37.37017980063,126.72086765055,9.9467,22.3000,0.0033,-0.0176,-0.0017,-0.531157919,-0.385004141,84.602874249,0.1862,0.1335,0.1446,0.0453,0.0379,0.0262,0.0359,0.0378,0.1023,0f000041,0*daa27616", "robot status", "#INSPVAXA,USB3,0,47.0,FINESTEERING,2113,382057.150,02000000,471d,15824;INS_SOLUTION_GOOD,INS_RTKFIXED,37.37017979407,126.72086765007,9.9466,22.3000,0.0033,-0.0175,-0.0022,-0.531418133,-0.384919719,84.603135663,0.1862,0.1335,0.1446,0.0453,0.0379,0.0262,0.0359,0.0378,0.1023,0f000041,0*5cf4af0b", "robot status", "#INSPVAXA,USB3,0,47.0,FINESTEERING,2113,382057.150,02000000,471d,15824;INS_SOLUTION_GOOD,INS_RTKFIXED,37.37017979407,126.72086765007,9.9466,22.3000,0.0033,-0.0175,-0.0022,-0.531418133,-0.384919719,84.603135663,0.1862,0.1335,0.1446,0.0453,0.0379,0.0262,0.0359,0.0378,0.1023,0f000041,0*5cf4af0b", "robot status", "#INSPVAXA,USB3,0,47.0,FINESTEERING,2113,382057.250,02000000,471d,15824;INS_SOLUTION_GOOD,INS_RTKFIXED,37.37017977982,126.72086765019,9.9462,22.3000,0.0030,-0.0175,-0.0023,-0.532391586,-0.385230578,84.602879683,0.1862,0.1335,0.1446,0.0453,0.0379,0.0262,0.0359,0.0378,0.1023,0f000041,0*a5850e12", "robot status", "#INSPVAXA,USB3,0,47.0,FINESTEERING,2113,382057.300,02000000,471d,15824;INS_SOLUTION_GOOD,INS_RTKFIXED,37.37017977326,126.72086764949,9.9460,22.3000,0.0027,-0.0176,-0.0023,-0.532076884,-0.385445383,84.602532145,0.1862,0.1335,0.1446,0.0453,0.0379,0.0262,0.0359,0.0378,0.1023,0f000041,0*04d9604a", "robot status", "#INSPVAXA,USB3,0,47.0,FINESTEERING,2113,382057.350,02000000,471d,15824;INS_SOLUTION_GOOD,INS_RTKFIXED,37.37017976672,126.72086764873,9.9458,22.3000,0.0029,-0.0175,-0.0025,-0.531606435,-0.385715498,84.602858310,0.1862,0.1335,0.1446,0.0453,0.0379,0.0262,0.0359,0.0378,0.1023,0f000041,0*b3bab68a", "robot status", "#INSPVAXA,USB3,0,47.0,FINESTEERING,2113,382057.350,02000000,471d,15824;INS_SOLUTION_GOOD,INS_RTKFIXED,37.37017976672,126.72086764873,9.9458,22.3000,0.0029,-0.0175,-0.0025,-0.531606435,-0.385715498,84.602858310,0.1862,0.1335,0.1446,0.0453,0.0379,0.0262,0.0359,0.0378,0.1023,0f000041,0*b3bab68a", "robot status", "#INSPVAXA,USB3,0,47.0,FINESTEERING,2113,382057.450,02000000,471d,15824;INS_SOLUTION_GOOD,INS_RTKFIXED,37.37017975387,126.72086764706,9.9454,22.3000,0.0029,-0.0175,-0.0020,-0.532339583,-0.385419935,84.602090548,0.1862,0.1335,0.1446,0.0453,0.0379,0.0262,0.0359,0.0378,0.1023,0f000041,0*14f622b3", "robot status", "#INSPVAXA,USB3,0,47.0,FINESTEERING,2113,382057.500,02000000,471d,15824;INS_SOLUTION_GOOD,INS_RTKFIXED,37.37017974638,126.72086764738,9.9452,22.3000,0.0028,-0.0177,-0.0023,-0.531607577,-0.385611557,84.601647293,0.1862,0.1335,0.1446,0.0453,0.0379,0.0262,0.0359,0.0378,0.1023,0f000041,0*31a01ca7", "robot status", "#INSPVAXA,USB3,0,47.0,FINESTEERING,2113,382057.550,02000000,471d,15824;INS_SOLUTION_GOOD,INS_RTKFIXED,37.37017974016,126.72086764616,9.9450,22.3000,0.0029,-0.0177,-0.0026,-0.531485418,-0.385329731,84.602063853,0.1862,0.1335,0.1446,0.0453,0.0379,0.0262,0.0359,0.0378,0.1023,0f000041,0*ef8aff35", "robot status", "#INSPVAXA,USB3,0,47.0,FINESTEERING,2113,382057.600,02000000,471d,15824;INS_SOLUTION_GOOD,INS_RTKFIXED,37.37017973400,126.72086764481,9.9447,22.3000,0.0028,-0.0176,-0.0028,-0.532011683,-0.385021431,84.601859074,0.1862,0.1335,0.1446,0.0453,0.0379,0.0262,0.0359,0.0378,0.1023,0f000041,0*cf28feed", "robot status", "#INSPVAXA,USB3,0,47.0,FINESTEERING,2113,382057.650,02000000,471d,15824;INS_SOLUTION_GOOD,INS_RTKFIXED,37.37017972675,126.72086764463,9.9445,22.3000,0.0029,-0.0178,-0.0028,-0.532002210,-0.386014521,84.601796435,0.1862,0.1335,0.1446,0.0453,0.0379,0.0262,0.0359,0.0378,0.1023,0f000041,0*e07f4ac9", "robot status", "#INSPVAXA,USB3,0,47.0,FINESTEERING,2113,382057.700,02000000,471d,15824;INS_SOLUTION_GOOD,INS_RTKFIXED,37.37017972069,126.72086764313,9.9443,22.3000,0.0028,-0.0178,-0.0029,-0.531560026,-0.385836027,84.602112778,0.1862,0.1335,0.1446,0.0453,0.0379,0.0262,0.0359,0.0378,0.1023,0f000041,0*507b3ba6", "robot status", "#INSPVAXA,USB3,0,47.0,FINESTEERING,2113,382057.750,02000000,471d,15824;INS_SOLUTION_GOOD,INS_RTKFIXED,37.37017971466,126.72086764163,9.9440,22.3000,0.0026,-0.0175,-0.0032,-0.532186397,-0.386195584,84.602463017,0.1862,0.1335,0.1446,0.0453,0.0379,0.0262,0.0359,0.0378,0.1023,0f000041,0*ba708e58", "robot status", "#INSPVAXA,USB3,0,47.0,FINESTEERING,2113,382057.800,02000000,471d,15824;INS_SOLUTION_GOOD,INS_RTKFIXED,37.37017970870,126.72086764010,9.9438,22.3000,0.0027,-0.0173,-0.0035,-0.531922855,-0.386605714,84.602340274,0.1862,0.1335,0.1446,0.0453,0.0379,0.0262,0.0359,0.0378,0.1023,0f000041,0*64a23a87", "robot status", "#INSPVAXA,USB3,0,47.0,FINESTEERING,2113,382057.850,02000000,471d,15824;INS_SOLUTION_GOOD,INS_RTKFIXED,37.37017970160,126.72086763983,9.9436,22.3000,0.0026,-0.0173,-0.0033,-0.532361676,-0.386784365,84.602249101,0.1862,0.1335,0.1446,0.0453,0.0379,0.0262,0.0359,0.0378,0.1023,0f000041,0*913eeb60", "robot status", "#INSPVAXA,USB3,0,47.0,FINESTEERING,2113,382057.900,02000000,471d,15824;INS_SOLUTION_GOOD,INS_RTKFIXED,37.37017969576,126.72086763819,9.9433,22.3000,0.0026,-0.0174,-0.0032,-0.532540250,-0.386300252,84.602234973,0.1862,0.1335,0.1446,0.0453,0.0379,0.0262,0.0359,0.0378,0.1023,0f000041,0*f3ec8587", "robot status", "#INSPVAXA,USB3,0,47.0,FINESTEERING,2113,382057.950,02000000,471d,15824;INS_SOLUTION_GOOD,INS_RTKFIXED,37.37017968996,126.72086763654,9.9431,22.3000,0.0025,-0.0170,-0.0036,-0.532855468,-0.386372431,84.602663331,0.1862,0.1335,0.1446,0.0453,0.0379,0.0262,0.0359,0.0378,0.1023,0f000041,0*09bb26e3", "robot status", "#INSPVAXA,USB3,0,47.0,FINESTEERING,2113,382058.000,02000000,471d,15824;INS_SOLUTION_GOOD,INS_RTKFIXED,37.37017968418,126.72086763491,9.9428,22.3000,0.0025,-0.0169,-0.0036,-0.533037093,-0.385623918,84.601847948,0.1862,0.1335,0.1446,0.0453,0.0379,0.0262,0.0359,0.0378,0.1023,0f000041,0*c18c0f67", "robot status", "#INSPVAXA,USB3,0,47.0,FINESTEERING,2113,382058.050,02000000,471d,15824;INS_SOLUTION_GOOD,INS_RTKFIXED,37.37017968030,126.72086765265,9.9431,22.3000,0.0024,-0.0167,-0.0032,-0.533406096,-0.386170793,84.602055088,0.1127,0.0809,0.0983,0.0014,0.0014,0.0012,0.0192,0.0193,0.1007,0f000045,0*e3dcd422", "robot status", "#INSPVAXA,USB3,0,47.5,FINESTEERING,2113,382058.100,02000000,471d,15824;INS_SOLUTION_GOOD,INS_RTKFIXED,37.37017967867,126.72086768926,9.9438,22.3000,0.0022,-0.0159,-0.0030,-0.532174167,-0.385678493,84.602410439,0.1127,0.0809,0.0983,0.0014,0.0014,0.0012,0.0192,0.0193,0.1007,0f000045,0*a8918789", "robot status", "#INSPVAXA,USB3,0,47.5,FINESTEERING,2113,382058.150,02000000,471d,15824;INS_SOLUTION_GOOD,INS_RTKFIXED,37.37017967732,126.72086772054,9.9445,22.3000,0.0022,-0.0153,-0.0029,-0.531700990,-0.385739178,84.603182566,0.1127,0.0809,0.0983,0.0014,0.0014,0.0012,0.0192,0.0193,0.1007,0f000045,0*130ead46", "robot status", "#INSPVAXA,USB3,0,47.5,FINESTEERING,2113,382058.200,02000000,471d,15824;INS_SOLUTION_GOOD,INS_RTKFIXED,37.37017967599,126.72086775165,9.9451,22.3000,0.0021,-0.0145,-0.0029,-0.531284914,-0.385913705,84.604026992,0.1127,0.0809,0.0983,0.0014,0.0014,0.0012,0.0192,0.0193,0.1007,0f000045,0*3772a9de", "robot status", "#INSPVAXA,USB3,0,47.5,FINESTEERING,2113,382058.250,02000000,471d,15824;INS_SOLUTION_GOOD,INS_RTKFIXED,37.37017967443,126.72086778801,9.9459,22.3000,0.0023,-0.0135,-0.0025,-0.531595022,-0.386924284,84.604211463,0.1127,0.0809,0.0983,0.0014,0.0014,0.0012,0.0192,0.0193,0.1007,0f000045,0*23a50fac", "robot status", "#INSPVAXA,USB3,0,47.5,FINESTEERING,2113,382058.300,02000000,471d,15824;INS_SOLUTION_GOOD,INS_RTKFIXED,37.37017967319,126.72086781916,9.9465,22.3000,0.0021,-0.0128,-0.0021,-0.531481099,-0.387203774,84.604221051,0.1127,0.0809,0.0983,0.0014,0.0014,0.0012,0.0192,0.0193,0.1007,0f000045,0*4dc52b13", "robot status", "#INSPVAXA,USB3,0,47.5,FINESTEERING,2113,382058.350,02000000,471d,15824;INS_SOLUTION_GOOD,INS_RTKFIXED,37.37017967193,126.72086785033,9.9471,22.3000,0.0023,-0.0120,-0.0020,-0.532387050,-0.387412023,84.604562476,0.1127,0.0809,0.0983,0.0014,0.0014,0.0012,0.0192,0.0193,0.1007,0f000045,0*8aa1e341", "robot status", "#INSPVAXA,USB3,0,47.5,FINESTEERING,2113,382058.400,02000000,471d,15824;INS_SOLUTION_GOOD,INS_RTKFIXED,37.37017967081,126.72086788145,9.9478,22.3000,0.0023,-0.0111,-0.0020,-0.532349705,-0.387500642,84.605133988,0.1127,0.0809,0.0983,0.0014,0.0014,0.0012,0.0192,0.0193,0.1007,0f000045,0*e1977c37", "robot status", "#INSPVAXA,USB3,0,47.5,FINESTEERING,2113,382058.450,02000000,471d,15824;INS_SOLUTION_GOOD,INS_RTKFIXED,37.37017966972,126.72086791250,9.9484,22.3000,0.0024,-0.0105,-0.0016,-0.531980936,-0.388378966,84.604936280,0.1127,0.0809,0.0983,0.0014,0.0014,0.0012,0.0192,0.0193,0.1007,0f000045,0*b1902217", "robot status", "#DUALANTENNAHEADINGA,USB3,0,47.5,FINESTEERING,2113,382058.500,02000000,d426,15824;SOL_COMPUTED,NARROW_INT,-1.000000000,90.222557068,-13.984893799,0.0,0.365761399,0.518876314,\"681H\",35,25,25,19,04,00,30,33*80e12eec", "robot status", "#INSPVAXA,USB3,0,47.5,FINESTEERING,2113,382058.550,02000000,471d,15824;INS_SOLUTION_GOOD,INS_RTKFIXED,37.37017966725,126.72086797977,9.9498,22.3000,0.0020,-0.0088,-0.0014,-0.530756621,-0.388840171,84.605118290,0.1127,0.0809,0.0983,0.0014,0.0014,0.0012,0.0192,0.0193,0.1007,0f000045,0*ab341f62", "robot status", "#INSPVAXA,USB3,0,47.5,FINESTEERING,2113,382058.600,02000000,471d,15824;INS_SOLUTION_GOOD,INS_RTKFIXED,37.37017966616,126.72086801079,9.9504,22.3000,0.0019,-0.0079,-0.0017,-0.530722648,-0.389681209,84.604664234,0.1127,0.0809,0.0983,0.0014,0.0014,0.0012,0.0192,0.0193,0.1007,0f000045,0*2fd7c5f4", "robot status", "#INSPVAXA,USB3,0,47.5,FINESTEERING,2113,382058.650,02000000,471d,15824;INS_SOLUTION_GOOD,INS_RTKFIXED,37.37017966485,126.72086804697,9.9512,22.3000,0.0020,-0.0071,-0.0015,-0.530347227,-0.390062019,84.604448354,0.1127,0.0809,0.0983,0.0014,0.0014,0.0012,0.0192,0.0193,0.1007,0f000045,0*8c412a96", "robot status", "#DUALANTENNAHEADINGA,USB3,0,47.5,FINESTEERING,2113,382058.700,02000000,d426,15824;SOL_COMPUTED,NARROW_INT,-1.000000000,90.031181335,-13.704864502,0.0,0.382271111,0.540790319,\"681H\",36,23,23,18,04,00,30,33*d8147764", "robot status", "#INSPVAXA,USB3,0,47.5,FINESTEERING,2113,382058.750,02000000,471d,15824;INS_SOLUTION_GOOD,INS_RTKFIXED,37.37017966285,126.72086810881,9.9524,22.3000,0.0016,-0.0057,-0.0012,-0.530289977,-0.390920917,84.604154048,0.1127,0.0809,0.0983,0.0014,0.0014,0.0012,0.0192,0.0193,0.1007,0f000045,0*db754c13", "robot status", "#INSPVAXA,USB3,0,47.5,FINESTEERING,2113,382058.800,02000000,471d,15824;INS_SOLUTION_GOOD,INS_RTKFIXED,37.37017966187,126.72086813969,9.9530,22.3000,0.0017,-0.0048,-0.0015,-0.528814770,-0.391446410,84.604653388,0.1127,0.0809,0.0983,0.0014,0.0014,0.0012,0.0192,0.0193,0.1007,0f000045,0*6d9019dd", "robot status", "#INSPVAXA,USB3,0,47.5,FINESTEERING,2113,382058.850,02000000,471d,15824;INS_SOLUTION_GOOD,INS_RTKFIXED,37.37017966065,126.72086817571,9.9537,22.3000,0.0016,-0.0039,-0.0012,-0.528339629,-0.392030577,84.605158256,0.1127,0.0809,0.0983,0.0014,0.0014,0.0012,0.0192,0.0193,0.1007,0f000045,0*7eed0430", "robot status", "#DUALANTENNAHEADINGA,USB3,0,47.5,FINESTEERING,2113,382058.900,02000000,d426,15824;SOL_COMPUTED,NARROW_INT,-1.000000000,89.919311523,-13.056823730,0.0,0.386787683,0.544841170,\"681H\",36,23,23,18,04,00,30,33*d6fb5dc6", "robot status", "#INSPVAXA,USB3,0,47.5,FINESTEERING,2113,382058.950,02000000,471d,15824;INS_SOLUTION_GOOD,INS_RTKFIXED,37.37017965858,126.72086823744,9.9550,22.3000,0.0013,-0.0024,-0.0011,-0.527765184,-0.392736465,84.605220178,0.1127,0.0809,0.0983,0.0014,0.0014,0.0012,0.0192,0.0193,0.1007,0f000045,0*2f8ca643", "robot status", "#INSPVAXA,USB3,0,47.5,FINESTEERING,2113,382059.000,02000000,471d,15824;INS_SOLUTION_GOOD,INS_RTKFIXED,37.37017965754,126.72086826826,9.9556,22.3000,0.0011,-0.0015,-0.0011,-0.527874190,-0.392257209,84.605207539,0.1127,0.0809,0.0983,0.0014,0.0014,0.0012,0.0192,0.0193,0.1007,0f000045,0*38d56ef4", "robot status", "#INSPVAXA,USB3,0,46.5,FINESTEERING,2113,382059.050,02000000,471d,15824;INS_SOLUTION_GOOD,INS_RTKFIXED,37.37017965651,126.72086828319,9.9558,22.3000,0.0014,-0.0013,-0.0010,-0.528085841,-0.393420470,84.605535666,0.1067,0.0761,0.0935,0.0013,0.0013,0.0012,0.0182,0.0183,0.0993,0f000045,0*dca370d5", "robot status", "#DUALANTENNAHEADINGA,USB3,0,46.5,FINESTEERING,2113,382059.100,02000000,d426,15824;SOL_COMPUTED,NARROW_INT,-1.000000000,89.760314941,-13.278625488,0.0,0.398367465,0.570054471,\"681H\",36,23,23,17,04,00,30,33*30c943a9", "robot status", "#INSPVAXA,USB3,0,46.5,FINESTEERING,2113,382059.150,02000000,471d,15824;INS_SOLUTION_GOOD,INS_RTKFIXED,37.37017965505,126.72086828040,9.9557,22.3000,0.0012,-0.0015,-0.0012,-0.528204910,-0.393097279,84.605269842,0.1067,0.0761,0.0935,0.0013,0.0013,0.0012,0.0182,0.0183,0.0993,0f000045,0*e7c45ad9", "robot status", "#INSPVAXA,USB3,0,46.5,FINESTEERING,2113,382059.200,02000000,471d,15824;INS_SOLUTION_GOOD,INS_RTKFIXED,37.37017965435,126.72086827903,9.9556,22.3000,0.0009,-0.0012,-0.0013,-0.529187573,-0.392509641,84.604863577,0.1067,0.0761,0.0935,0.0013,0.0013,0.0012,0.0182,0.0183,0.0993,0f000045,0*b765674f", "robot status", "#INSPVAXA,USB3,0,46.5,FINESTEERING,2113,382059.250,02000000,471d,15824;INS_SOLUTION_GOOD,INS_RTKFIXED,37.37017965353,126.72086827739,9.9555,22.3000,0.0009,-0.0013,-0.0012,-0.529263004,-0.392450049,84.604605116,0.1067,0.0761,0.0935,0.0013,0.0013,0.0012,0.0182,0.0183,0.0993,0f000045,0*0bee21c7", "robot status", "#DUALANTENNAHEADINGA,USB3,0,46.5,FINESTEERING,2113,382059.300,02000000,d426,15824;SOL_COMPUTED,NARROW_INT,-1.000000000,89.957183838,-13.966003418,0.0,0.395380825,0.529536486,\"681H\",36,23,23,18,04,00,30,33*bc33605b", "robot status", "#INSPVAXA,USB3,0,46.5,FINESTEERING,2113,382059.350,02000000,471d,15824;INS_SOLUTION_GOOD,INS_RTKFIXED,37.37017965198,126.72086827442,9.9553,22.3000,0.0006,-0.0014,-0.0009,-0.529476074,-0.393067897,84.604933313,0.1067,0.0761,0.0935,0.0013,0.0013,0.0012,0.0182,0.0183,0.0993,0f000045,0*29d9df96", "robot status", "#INSPVAXA,USB3,0,46.5,FINESTEERING,2113,382059.400,02000000,471d,15824;INS_SOLUTION_GOOD,INS_RTKFIXED,37.37017965111,126.72086827300,9.9552,22.3000,0.0002,-0.0010,-0.0009,-0.529204351,-0.392512319,84.603721217,0.1067,0.0761,0.0935,0.0013,0.0013,0.0012,0.0182,0.0183,0.0993,0f000045,0*374a2353", "robot status", "#INSPVAXA,USB3,0,46.5,FINESTEERING,2113,382059.450,02000000,471d,15824;INS_SOLUTION_GOOD,INS_RTKFIXED,37.37017965017,126.72086827131,9.9551,22.3000,0.0006,-0.0013,-0.0007,-0.529356196,-0.392677850,84.603995341,0.1067,0.0761,0.0935,0.0013,0.0013,0.0012,0.0182,0.0183,0.0993,0f000045,0*0e6624d5", "robot status", "#DUALANTENNAHEADINGA,USB3,0,46.5,FINESTEERING,2113,382059.500,02000000,d426,15824;SOL_COMPUTED,NARROW_INT,-1.000000000,89.990684509,-12.901794434,0.0,0.399564207,0.541544497,\"681H\",36,23,23,18,04,00,30,33*2acc1d2d", "robot status", "#INSPVAXA,USB3,0,46.5,FINESTEERING,2113,382059.550,02000000,471d,15824;INS_SOLUTION_GOOD,INS_RTKFIXED,37.37017964864,126.72086826830,9.9549,22.3000,0.0006,-0.0012,-0.0008,-0.529861310,-0.392945918,84.605043971,0.1067,0.0761,0.0935,0.0013,0.0013,0.0012,0.0182,0.0183,0.0993,0f000045,0*470862fb", "robot status", "#INSPVAXA,USB3,0,46.5,FINESTEERING,2113,382059.600,02000000,471d,15824;INS_SOLUTION_GOOD,INS_RTKFIXED,37.37017964788,126.72086826674,9.9548,22.3000,0.0004,-0.0012,-0.0008,-0.529375788,-0.392092914,84.604213410,0.1067,0.0761,0.0935,0.0013,0.0013,0.0012,0.0182,0.0183,0.0993,0f000045,0*fc5633da", "robot status", "#INSPVAXA,USB3,0,46.5,FINESTEERING,2113,382059.650,02000000,471d,15824;INS_SOLUTION_GOOD,INS_RTKFIXED,37.37017964708,126.72086826487,9.9547,22.3000,0.0007,-0.0013,-0.0009,-0.528883469,-0.392365045,84.603706491,0.1067,0.0761,0.0935,0.0013,0.0013,0.0012,0.0182,0.0183,0.0993,0f000045,0*960c0b1b", "robot status", "#DUALANTENNAHEADINGA,USB3,0,46.5,FINESTEERING,2113,382059.700,02000000,d426,15824;SOL_COMPUTED,NARROW_INT,-1.000000000,89.814247131,-13.024017334,0.0,0.398760736,0.558425486,\"681H\",37,23,23,18,04,00,30,33*ab742ed6", "robot status", "#INSPVAXA,USB3,0,46.5,FINESTEERING,2113,382059.750,02000000,471d,15824;INS_SOLUTION_GOOD,INS_RTKFIXED,37.37017964582,126.72086826153,9.9545,22.3000,0.0006,-0.0014,-0.0010,-0.528766889,-0.392334318,84.603704045,0.1067,0.0761,0.0935,0.0013,0.0013,0.0012,0.0182,0.0183,0.0993,0f000045,0*f704f1d3", "robot status", "#INSPVAXA,USB3,0,46.5,FINESTEERING,2113,382059.800,02000000,471d,15824;INS_SOLUTION_GOOD,INS_RTKFIXED,37.37017964526,126.72086825983,9.9544,22.3000,0.0006,-0.0012,-0.0012,-0.529088986,-0.392552476,84.604569959,0.1067,0.0761,0.0935,0.0013,0.0013,0.0012,0.0182,0.0183,0.0993,0f000045,0*5f72bfe7", "robot status", "#INSPVAXA,USB3,0,46.5,FINESTEERING,2113,382059.850,02000000,471d,15824;INS_SOLUTION_GOOD,INS_RTKFIXED,37.37017964465,126.72086825788,9.9543,22.3000,0.0007,-0.0013,-0.0009,-0.528930115,-0.392562988,84.604117494,0.1067,0.0761,0.0935,0.0013,0.0013,0.0012,0.0182,0.0183,0.0993,0f000045,0*6b5aafbe", "robot status", "#DUALANTENNAHEADINGA,USB3,0,46.5,FINESTEERING,2113,382059.900,02000000,d426,15824;SOL_COMPUTED,NARROW_INT,-1.000000000,90.169891357,-13.783294678,0.0,0.393729985,0.540345550,\"681H\",36,23,23,17,04,00,30,33*4036edeb", "robot status", "#INSPVAXA,USB3,0,46.5,FINESTEERING,2113,382059.950,02000000,471d,15824;INS_SOLUTION_GOOD,INS_RTKFIXED,37.37017964359,126.72086825424,9.9541,22.3000,0.0003,-0.0013,-0.0011,-0.529222194,-0.392747354,84.604442883,0.1067,0.0761,0.0935,0.0013,0.0013,0.0012,0.0182,0.0183,0.0993,0f000045,0*86f07407", "robot status", "#INSPVAXA,USB3,0,46.5,FINESTEERING,2113,382060.000,02000000,471d,15824;INS_SOLUTION_GOOD,INS_RTKFIXED,37.37017964307,126.72086825232,9.9540,22.3000,0.0003,-0.0014,-0.0012,-0.529240385,-0.393627693,84.603346955,0.1067,0.0761,0.0935,0.0013,0.0013,0.0012,0.0182,0.0183,0.0993,0f000045,0*f15542a2", "robot status", "#INSPVAXA,USB3,0,46.5,FINESTEERING,2113,382060.050,02000000,471d,15824;INS_SOLUTION_GOOD,INS_RTKFIXED,37.37017964242,126.72086825114,9.9539,22.3000,0.0005,-0.0015,-0.0010,-0.528691513,-0.393999398,84.603462699,0.1019,0.0723,0.0894,0.0013,0.0013,0.0012,0.0180,0.0181,0.0978,0f000045,0*b77d2572", "robot status", "#DUALANTENNAHEADINGA,USB3,0,44.0,FINESTEERING,2113,382060.100,02000000,d426,15824;SOL_COMPUTED,NARROW_INT,-1.000000000,90.510375977,-13.690917969,0.0,0.387503088,0.533289671,\"681H\",37,23,23,17,04,00,30,33*bceec578", "robot status", "#INSPVAXA,USB3,0,44.0,FINESTEERING,2113,382060.150,02000000,471d,15824;INS_SOLUTION_GOOD,INS_RTKFIXED,37.37017964087,126.72086824990,9.9537,22.3000,0.0004,-0.0015,-0.0010,-0.529436537,-0.393299814,84.603594254,0.1019,0.0723,0.0894,0.0013,0.0013,0.0012,0.0180,0.0181,0.0978,0f000045,0*c7e0f5b8", "robot status", "#DUALANTENNAHEADINGA,USB3,0,44.0,FINESTEERING,2113,382060.200,02000000,d426,15824;SOL_COMPUTED,NARROW_INT,-1.000000000,90.627426147,-14.626190186,0.0,0.393142730,0.548973858,\"681H\",36,23,23,16,04,00,30,33*1e9ea427", "robot status", "#INSPVAXA,USB3,0,44.0,FINESTEERING,2113,382060.250,02000000,471d,15824;INS_SOLUTION_GOOD,INS_RTKFIXED,37.37017963935,126.72086824833,9.9534,22.3000,0.0006,-0.0016,-0.0008,-0.529437380,-0.393602053,84.603614590,0.1019,0.0723,0.0894,0.0013,0.0013,0.0012,0.0180,0.0181,0.0978,0f000045,0*cb37e91c", "robot status", "#DUALANTENNAHEADINGA,USB3,0,44.0,FINESTEERING,2113,382060.300,02000000,d426,15824;SOL_COMPUTED,NARROW_INT,-1.000000000,90.819747925,-13.982696533,0.0,0.388585508,0.566581726,\"681H\",36,22,22,15,04,00,30,33*8b6b3d4b", "robot status", "#INSPVAXA,USB3,0,44.0,FINESTEERING,2113,382060.350,02000000,471d,15824;INS_SOLUTION_GOOD,INS_RTKFIXED,37.37017963801,126.72086824696,9.9532,22.3000,0.0005,-0.0013,-0.0007,-0.529688494,-0.394132513,84.604059479,0.1019,0.0723,0.0894,0.0013,0.0013,0.0012,0.0180,0.0181,0.0978,0f000045,0*5baa7e39", "robot status", "#INSPVAXA,USB3,0,44.0,FINESTEERING,2113,382060.400,02000000,471d,15824;INS_SOLUTION_GOOD,INS_RTKFIXED,37.37017963739,126.72086824627,9.9531,22.3000,0.0007,-0.0012,-0.0008,-0.528807497,-0.394222613,84.604220348,0.1019,0.0723,0.0894,0.0013,0.0013,0.0012,0.0180,0.0181,0.0978,0f000045,0*014aa501", "robot status", "#INSPVAXA,USB3,0,44.0,FINESTEERING,2113,382060.450,02000000,471d,15824;INS_SOLUTION_GOOD,INS_RTKFIXED,37.37017963682,126.72086824561,9.9530,22.3000,0.0008,-0.0012,-0.0003,-0.529756352,-0.394568246,84.603860624,0.1019,0.0723,0.0894,0.0013,0.0013,0.0012,0.0180,0.0181,0.0978,0f000045,0*54192430", "robot status", "#DUALANTENNAHEADINGA,USB3,0,44.0,FINESTEERING,2113,382060.500,02000000,d426,15824;SOL_COMPUTED,NARROW_INT,-1.000000000,89.788841248,-13.230407715,0.0,0.389966130,0.564237118,\"681H\",36,22,22,15,04,00,30,33*d8cd7924", "robot status", "#INSPVAXA,USB3,0,44.0,FINESTEERING,2113,382060.550,02000000,471d,15824;INS_SOLUTION_GOOD,INS_RTKFIXED,37.37017963565,126.72086824428,9.9527,22.3000,0.0008,-0.0008,-0.0005,-0.529243146,-0.394124317,84.603877237,0.1019,0.0723,0.0894,0.0013,0.0013,0.0012,0.0180,0.0181,0.0978,0f000045,0*89c40cff", "robot status", "#INSPVAXA,USB3,0,44.0,FINESTEERING,2113,382060.600,02000000,471d,15824;INS_SOLUTION_GOOD,INS_RTKFIXED,37.37017963517,126.72086824362,9.9526,22.3000,0.0008,-0.0009,-0.0003,-0.528452459,-0.394390389,84.603323675,0.1019,0.0723,0.0894,0.0013,0.0013,0.0012,0.0180,0.0181,0.0978,0f000045,0*ab6ce6f2", "robot status", "#INSPVAXA,USB3,0,44.0,FINESTEERING,2113,382060.650,02000000,471d,15824;INS_SOLUTION_GOOD,INS_RTKFIXED,37.37017963458,126.72086824290,9.9525,22.3000,0.0011,-0.0010,-0.0003,-0.528082773,-0.394470896,84.603104730,0.1019,0.0723,0.0894,0.0013,0.0013,0.0012,0.0180,0.0181,0.0978,0f000045,0*7997d3ca", "robot status", "#DUALANTENNAHEADINGA,USB3,0,44.0,FINESTEERING,2113,382060.700,02000000,d426,15824;SOL_COMPUTED,NARROW_INT,-1.000000000,89.950988770,-12.975158691,0.0,0.389810354,0.544802368,\"681H\",36,23,23,16,04,00,30,33*e94df24d", "robot status", "#INSPVAXA,USB3,0,44.0,FINESTEERING,2113,382060.750,02000000,471d,15824;INS_SOLUTION_GOOD,INS_RTKFIXED,37.37017963374,126.72086824157,9.9523,22.3000,0.0009,-0.0009,-0.0005,-0.528342307,-0.395356762,84.602817143,0.1019,0.0723,0.0894,0.0013,0.0013,0.0012,0.0180,0.0181,0.0978,0f000045,0*f76c7d47", "robot status", "#DUALANTENNAHEADINGA,USB3,0,44.0,FINESTEERING,2113,382060.800,02000000,d426,15824;SOL_COMPUTED,NARROW_INT,-1.000000000,90.106506348,-12.575378418,0.0,0.388782382,0.543644547,\"681H\",36,23,23,16,04,00,30,33*0f6117c7", "robot status", "#INSPVAXA,USB3,0,44.0,FINESTEERING,2113,382060.850,02000000,471d,15824;INS_SOLUTION_GOOD,INS_RTKFIXED,37.37017963272,126.72086824004,9.9521,22.3000,0.0008,-0.0008,-0.0003,-0.528219827,-0.395630605,84.603155082,0.1019,0.0723,0.0894,0.0013,0.0013,0.0012,0.0180,0.0181,0.0978,0f000045,0*06d279c2", "robot status", "#DUALANTENNAHEADINGA,USB3,0,44.0,FINESTEERING,2113,382060.900,02000000,d426,15824;SOL_COMPUTED,NARROW_INT,-1.000000000,89.911697388,-13.454437256,0.0,0.398041755,0.546290457,\"681H\",36,23,23,15,04,00,30,33*e729d694", "robot status", "#INSPVAXA,USB3,0,44.0,FINESTEERING,2113,382060.950,02000000,471d,15824;INS_SOLUTION_GOOD,INS_RTKFIXED,37.37017963176,126.72086823870,9.9518,22.3000,0.0008,-0.0005,-0.0005,-0.529073607,-0.395968620,84.602588974,0.1019,0.0723,0.0894,0.0013,0.0013,0.0012,0.0180,0.0181,0.0978,0f000045,0*20b98184", "robot status", "#DUALANTENNAHEADINGA,USB3,0,44.0,FINESTEERING,2113,382061.000,02000000,d426,15824;SOL_COMPUTED,NARROW_INT,-1.000000000,89.977088928,-13.186584473,0.0,0.396083057,0.544201434,\"681H\",36,23,23,15,04,00,30,33*a188269c", "robot status", "#INSPVAXA,USB3,0,44.0,FINESTEERING,2113,382061.050,02000000,471d,15824;INS_SOLUTION_GOOD,INS_RTKFIXED,37.37017963057,126.72086823738,9.9516,22.3000,0.0009,-0.0005,-0.0002,-0.528612615,-0.396709415,84.601881251,0.0978,0.0690,0.0858,0.0013,0.0013,0.0011,0.0180,0.0180,0.0965,0f000045,0*db8fc301", "robot status", "#DUALANTENNAHEADINGA,USB3,0,44.0,FINESTEERING,2113,382061.100,02000000,d426,15824;SOL_COMPUTED,NARROW_INT,-1.000000000,90.027145386,-12.631042480,0.0,0.395767301,0.545643449,\"681H\",36,23,23,15,04,00,30,33*0b906523", "robot status", "#INSPVAXA,USB3,0,45.0,FINESTEERING,2113,382061.150,02000000,471d,15824;INS_SOLUTION_GOOD,INS_RTKFIXED,37.37017962876,126.72086823606,9.9514,22.3000,0.0007,-0.0003,-0.0005,-0.527312340,-0.396342999,84.603301492,0.0978,0.0690,0.0858,0.0013,0.0013,0.0011,0.0180,0.0180,0.0965,0f000045,0*2484f441", "robot status", "#DUALANTENNAHEADINGA,USB3,0,45.0,FINESTEERING,2113,382061.200,02000000,d426,15824;SOL_COMPUTED,NARROW_INT,-1.000000000,90.225608826,-12.317108154,0.0,0.499552429,0.896078169,\"681H\",36,24,24,16,04,00,30,33*7e2fb80e", "robot status", "#INSPVAXA,USB3,0,45.0,FINESTEERING,2113,382061.250,02000000,471d,15824;INS_SOLUTION_GOOD,INS_RTKFIXED,37.37017962696,126.72086823465,9.9513,22.3000,0.0007,-0.0005,-0.0002,-0.527699242,-0.396097072,84.604140375,0.0978,0.0690,0.0858,0.0013,0.0013,0.0011,0.0180,0.0180,0.0965,0f000045,0*3f48f1ef", "robot status", "#DUALANTENNAHEADINGA,USB3,0,45.0,FINESTEERING,2113,382061.300,02000000,d426,15824;SOL_COMPUTED,NARROW_INT,-1.000000000,90.075325012,-12.666290283,0.0,0.496975124,0.886718452,\"681H\",36,24,24,16,04,00,30,33*1f294aa0", "robot status", "#INSPVAXA,USB3,0,45.0,FINESTEERING,2113,382061.350,02000000,471d,15824;INS_SOLUTION_GOOD,INS_RTKFIXED,37.37017962538,126.72086823319,9.9511,22.3000,0.0008,-0.0003,-0.0004,-0.527965614,-0.396279309,84.604373224,0.0978,0.0690,0.0858,0.0013,0.0013,0.0011,0.0180,0.0180,0.0965,0f000045,0*39efad05", "robot status", "#DUALANTENNAHEADINGA,USB3,0,45.0,FINESTEERING,2113,382061.400,02000000,d426,15824;SOL_COMPUTED,NARROW_INT,-1.000000000,90.221908569,-11.989440918,0.0,0.496297628,0.887758493,\"681H\",36,24,24,16,04,00,30,33*08d00799", "robot status", "#INSPVAXA,USB3,0,45.0,FINESTEERING,2113,382061.450,02000000,471d,15824;INS_SOLUTION_GOOD,INS_RTKFIXED,37.37017962376,126.72086823173,9.9509,22.3000,0.0005,-0.0006,-0.0004,-0.527177713,-0.396146876,84.603834186,0.0978,0.0690,0.0858,0.0013,0.0013,0.0011,0.0180,0.0180,0.0965,0f000045,0*739abbc7", "robot status", "#DUALANTENNAHEADINGA,USB3,0,45.0,FINESTEERING,2113,382061.500,02000000,d426,15824;SOL_COMPUTED,NARROW_INT,-1.000000000,90.095130920,-12.774780273,0.0,0.500870585,0.889655232,\"681H\",36,24,24,16,04,00,30,33*fac6570e", "robot status", "#INSPVAXA,USB3,0,45.0,FINESTEERING,2113,382061.550,02000000,471d,15824;INS_SOLUTION_GOOD,INS_RTKFIXED,37.37017962210,126.72086823015,9.9507,22.3000,0.0004,-0.0002,-0.0004,-0.527817952,-0.396449047,84.603940275,0.0978,0.0690,0.0858,0.0013,0.0013,0.0011,0.0180,0.0180,0.0965,0f000045,0*91f80397", "robot status", "#DUALANTENNAHEADINGA,USB3,0,45.0,FINESTEERING,2113,382061.600,02000000,d426,15824;SOL_COMPUTED,NARROW_INT,-1.000000000,90.199661255,-12.463409424,0.0,0.500405312,0.888472438,\"681H\",36,24,24,16,04,00,30,33*a8d04e6b", "robot status", "#INSPVAXA,USB3,0,45.0,FINESTEERING,2113,382061.650,02000000,471d,15824;INS_SOLUTION_GOOD,INS_RTKFIXED,37.37017962035,126.72086822869,9.9505,22.3000,0.0002,-0.0003,-0.0002,-0.527718942,-0.397030658,84.605103258,0.0978,0.0690,0.0858,0.0013,0.0013,0.0011,0.0180,0.0180,0.0965,0f000045,0*bc21b3a7", "robot status", "#DUALANTENNAHEADINGA,USB3,0,45.0,FINESTEERING,2113,382061.700,02000000,d426,15824;SOL_COMPUTED,NARROW_INT,-1.000000000,90.138404846,-12.640686035,0.0,0.500510871,0.888915479,\"681H\",36,24,24,16,04,00,30,33*a67c0fc4", "robot status", "#INSPVAXA,USB3,0,45.0,FINESTEERING,2113,382061.750,02000000,471d,15824;INS_SOLUTION_GOOD,INS_RTKFIXED,37.37017961859,126.72086822744,9.9503,22.3000,0.0002,0.0001,-0.0004,-0.528243332,-0.396281275,84.604945444,0.0978,0.0690,0.0858,0.0013,0.0013,0.0011,0.0180,0.0180,0.0965,0f000045,0*3deb2616", "robot status", "#DUALANTENNAHEADINGA,USB3,0,45.0,FINESTEERING,2113,382061.800,02000000,d426,15824;SOL_COMPUTED,NARROW_INT,-1.000000000,90.231124878,-12.300476074,0.0,0.497394621,0.882756650,\"681H\",36,24,24,16,04,00,30,33*a094ba55", "robot status", "#INSPVAXA,USB3,0,45.0,FINESTEERING,2113,382061.850,02000000,471d,15824;INS_SOLUTION_GOOD,INS_RTKFIXED,37.37017961689,126.72086822626,9.9502,22.3000,0.0004,0.0001,-0.0001,-0.527222008,-0.396975217,84.604634660,0.0978,0.0690,0.0858,0.0013,0.0013,0.0011,0.0180,0.0180,0.0965,0f000045,0*fd857c3b", "robot status", "#DUALANTENNAHEADINGA,USB3,0,45.0,FINESTEERING,2113,382061.900,02000000,d426,15824;SOL_COMPUTED,NARROW_INT,-1.000000000,90.190574646,-12.881774902,0.0,0.502805352,0.887293279,\"681H\",36,24,24,16,04,00,30,33*c2225ba2", "robot status", "#INSPVAXA,USB3,0,45.0,FINESTEERING,2113,382061.950,02000000,471d,15824;INS_SOLUTION_GOOD,INS_RTKFIXED,37.37017961542,126.72086822535,9.9500,22.3000,0.0002,0.0006,0.0000,-0.527300056,-0.398047143,84.604785872,0.0978,0.0690,0.0858,0.0013,0.0013,0.0011,0.0180,0.0180,0.0965,0f000045,0*a8209603", "robot status", "#DUALANTENNAHEADINGA,USB3,0,45.0,FINESTEERING,2113,382062.000,02000000,d426,15824;SOL_COMPUTED,NARROW_INT,-1.000000000,90.038627625,-12.980133057,0.0,0.499885857,0.881782889,\"681H\",36,24,24,16,04,00,30,33*9e25d6db", "robot status", "#INSPVAXA,USB3,0,45.0,FINESTEERING,2113,382062.050,02000000,471d,15824;INS_SOLUTION_GOOD,INS_RTKFIXED,37.37017961402,126.72086822454,9.9499,22.3000,0.0002,0.0005,0.0005,-0.527913647,-0.397591766,84.604823010,0.0942,0.0662,0.0827,0.0013,0.0013,0.0011,0.0180,0.0180,0.0953,0f000045,0*c4953420", "robot status", "#DUALANTENNAHEADINGA,USB3,0,45.0,FINESTEERING,2113,382062.100,02000000,d426,15824;SOL_COMPUTED,NARROW_INT,-1.000000000,90.036399841,-13.092987061,0.0,0.498007387,0.877561092,\"681H\",36,24,24,16,04,00,30,33*3831e41f", "robot status", "#INSPVAXA,USB3,0,45.5,FINESTEERING,2113,382062.150,02000000,471d,15824;INS_SOLUTION_GOOD,INS_RTKFIXED,37.37017961286,126.72086822374,9.9498,22.3000,-0.0001,0.0009,0.0004,-0.528550181,-0.397856781,84.604225150,0.0942,0.0662,0.0827,0.0013,0.0013,0.0011,0.0180,0.0180,0.0953,0f000045,0*febf5ff8", "robot status", "#DUALANTENNAHEADINGA,USB3,0,45.5,FINESTEERING,2113,382062.200,02000000,d426,15824;SOL_COMPUTED,NARROW_INT,-1.000000000,90.099815369,-12.673614502,0.0,0.506676316,0.906221390,\"681H\",36,25,25,18,04,00,30,33*14d5fade", "robot status", "#INSPVAXA,USB3,0,45.5,FINESTEERING,2113,382062.250,02000000,471d,15824;INS_SOLUTION_GOOD,INS_RTKFIXED,37.37017961165,126.72086822288,9.9497,22.3000,-0.0001,0.0004,0.0006,-0.527085688,-0.397532754,84.604036797,0.0942,0.0662,0.0827,0.0013,0.0013,0.0011,0.0180,0.0180,0.0953,0f000045,0*97c7a4d0", "robot status", "#DUALANTENNAHEADINGA,USB3,0,45.5,FINESTEERING,2113,382062.300,02000000,d426,15824;SOL_COMPUTED,NARROW_INT,-1.000000000,90.144775391,-13.036560059,0.0,0.511643589,0.908375978,\"681H\",36,25,25,18,04,00,30,33*80ab8d0c", "robot status", "#INSPVAXA,USB3,0,45.5,FINESTEERING,2113,382062.350,02000000,471d,15824;INS_SOLUTION_GOOD,INS_RTKFIXED,37.37017961049,126.72086822212,9.9497,22.3000,-0.0001,0.0007,0.0002,-0.527679916,-0.398387442,84.603491309,0.0942,0.0662,0.0827,0.0013,0.0013,0.0011,0.0180,0.0180,0.0953,0f000045,0*d54c662c", "robot status", "#DUALANTENNAHEADINGA,USB3,0,45.5,FINESTEERING,2113,382062.400,02000000,d426,15824;SOL_COMPUTED,NARROW_INT,-1.000000000,90.053291321,-13.209472656,0.0,0.511181235,0.904071271,\"681H\",36,25,25,18,04,00,30,33*f9691172", "robot status", "#INSPVAXA,USB3,0,45.5,FINESTEERING,2113,382062.450,02000000,471d,15824;INS_SOLUTION_GOOD,INS_RTKFIXED,37.37017960924,126.72086822137,9.9496,22.3000,-0.0001,0.0004,0.0003,-0.528171588,-0.398399135,84.602567497,0.0942,0.0662,0.0827,0.0013,0.0013,0.0011,0.0180,0.0180,0.0953,0f000045,0*6ff716d0", "robot status", "#DUALANTENNAHEADINGA,USB3,0,45.5,FINESTEERING,2113,382062.500,02000000,d426,15824;SOL_COMPUTED,NARROW_INT,-1.000000000,89.896476746,-13.233062744,0.0,0.510159194,0.900192022,\"681H\",36,25,25,18,04,00,30,33*a2d5fe07", "robot status", "#INSPVAXA,USB3,0,45.5,FINESTEERING,2113,382062.550,02000000,471d,15824;INS_SOLUTION_GOOD,INS_RTKFIXED,37.37017960823,126.72086822066,9.9495,22.3000,0.0001,0.0005,0.0002,-0.527788947,-0.398049254,84.601664165,0.0942,0.0662,0.0827,0.0013,0.0013,0.0011,0.0180,0.0180,0.0953,0f000045,0*3d76b72f", "robot status", "#DUALANTENNAHEADINGA,USB3,0,45.5,FINESTEERING,2113,382062.600,02000000,d426,15824;SOL_COMPUTED,NARROW_INT,-1.000000000,90.132804871,-12.435180664,0.0,0.510948420,0.905416727,\"681H\",36,25,25,18,04,00,30,33*6e786c9e", "robot status", "#INSPVAXA,USB3,0,45.5,FINESTEERING,2113,382062.650,02000000,471d,15824;INS_SOLUTION_GOOD,INS_RTKFIXED,37.37017960734,126.72086821982,9.9495,22.3000,0.0002,0.0001,0.0008,-0.528816728,-0.399236846,84.601474399,0.0942,0.0662,0.0827,0.0013,0.0013,0.0011,0.0180,0.0180,0.0953,0f000045,0*a41bd37d", "robot status", "#DUALANTENNAHEADINGA,USB3,0,45.5,FINESTEERING,2113,382062.700,02000000,d426,15824;SOL_COMPUTED,NARROW_INT,-1.000000000,89.984909058,-13.387969971,0.0,0.509943426,0.898799360,\"681H\",36,25,25,18,04,00,30,33*ac2f2c70", "robot status", "#INSPVAXA,USB3,0,45.5,FINESTEERING,2113,382062.750,02000000,471d,15824;INS_SOLUTION_GOOD,INS_RTKFIXED,37.37017960617,126.72086821890,9.9494,22.3000,-0.0001,0.0002,0.0005,-0.529178046,-0.398731448,84.601658927,0.0942,0.0662,0.0827,0.0013,0.0013,0.0011,0.0180,0.0180,0.0953,0f000045,0*731ee853", "robot status", "#DUALANTENNAHEADINGA,USB3,0,45.5,FINESTEERING,2113,382062.800,02000000,d426,15824;SOL_COMPUTED,NARROW_INT,-1.000000000,90.177024841,-12.710632324,0.0,0.510081828,0.900352120,\"681H\",36,25,25,18,04,00,30,33*bb33f6ff", "robot status", "#INSPVAXA,USB3,0,45.5,FINESTEERING,2113,382062.850,02000000,471d,15824;INS_SOLUTION_GOOD,INS_RTKFIXED,37.37017960478,126.72086821804,9.9494,22.3000,-0.0004,0.0002,0.0011,-0.530065401,-0.399956636,84.600950473,0.0942,0.0662,0.0827,0.0013,0.0013,0.0011,0.0180,0.0180,0.0953,0f000045,0*0c02bcaa", "robot status", "#DUALANTENNAHEADINGA,USB3,0,45.5,FINESTEERING,2113,382062.900,02000000,d426,15824;SOL_COMPUTED,NARROW_INT,-1.000000000,90.056198120,-13.431762695,0.0,0.506258070,0.887736499,\"681H\",36,25,25,18,04,00,30,33*0d70b7a2", "robot status", "#INSPVAXA,USB3,0,45.5,FINESTEERING,2113,382062.950,02000000,471d,15824;INS_SOLUTION_GOOD,INS_RTKFIXED,37.37017960329,126.72086821722,9.9494,22.3000,-0.0009,0.0004,0.0010,-0.528888564,-0.400426686,84.600611774,0.0942,0.0662,0.0827,0.0013,0.0013,0.0011,0.0180,0.0180,0.0953,0f000045,0*ff916a40", "robot status", "#INSPVAXA,USB3,0,45.5,FINESTEERING,2113,382063.050,02000000,471d,15824;INS_SOLUTION_GOOD,INS_RTKFIXED,37.37017960193,126.72086821628,9.9494,22.3000,-0.0010,0.0001,0.0012,-0.529706558,-0.400504912,84.600274469,0.0909,0.0637,0.0798,0.0013,0.0013,0.0011,0.0180,0.0180,0.0941,0f000045,0*b98d1f67", "robot status", "#INSPVAXA,USB3,0,45.5,FINESTEERING,2113,382063.050,02000000,471d,15824;INS_SOLUTION_GOOD,INS_RTKFIXED,37.37017960193,126.72086821628,9.9494,22.3000,-0.0010,0.0001,0.0012,-0.529706558,-0.400504912,84.600274469,0.0909,0.0637,0.0798,0.0013,0.0013,0.0011,0.0180,0.0180,0.0941,0f000045,0*b98d1f67", "robot status", "#DUALANTENNAHEADINGA,USB3,0,45.5,FINESTEERING,2113,382063.100,02000000,d426,15824;SOL_COMPUTED,NARROW_INT,-1.000000000,89.942916870,-13.429290771,0.0,0.500825167,0.878483832,\"681H\",36,25,25,18,04,00,30,33*ca44cc62", "robot status", "#INSPVAXA,USB3,0,46.0,FINESTEERING,2113,382063.150,02000000,471d,15824;INS_SOLUTION_GOOD,INS_RTKFIXED,37.37017960099,126.72086821507,9.9493,22.3000,-0.0010,-0.0001,0.0011,-0.530412434,-0.400008154,84.599375998,0.0909,0.0637,0.0798,0.0013,0.0013,0.0011,0.0180,0.0180,0.0941,0f000045,0*cc7bfcb2", "robot status", "#INSPVAXA,USB3,0,46.0,FINESTEERING,2113,382063.250,02000000,471d,15824;INS_SOLUTION_GOOD,INS_RTKFIXED,37.37017959994,126.72086821370,9.9492,22.3000,-0.0010,-0.0001,0.0014,-0.531203031,-0.400076626,84.599792100,0.0909,0.0637,0.0798,0.0013,0.0013,0.0011,0.0180,0.0180,0.0941,0f000045,0*05ccc527", "robot status", "#INSPVAXA,USB3,0,46.0,FINESTEERING,2113,382063.250,02000000,471d,15824;INS_SOLUTION_GOOD,INS_RTKFIXED,37.37017959994,126.72086821370,9.9492,22.3000,-0.0010,-0.0001,0.0014,-0.531203031,-0.400076626,84.599792100,0.0909,0.0637,0.0798,0.0013,0.0013,0.0011,0.0180,0.0180,0.0941,0f000045,0*05ccc527", "robot status", "#DUALANTENNAHEADINGA,USB3,0,46.0,FINESTEERING,2113,382063.300,02000000,d426,15824;SOL_COMPUTED,NARROW_INT,-1.000000000,90.152618408,-12.986297607,0.0,0.324859470,0.461135149,\"681H\",36,27,27,21,04,00,30,33*13454c38", "robot status", "#INSPVAXA,USB3,0,46.0,FINESTEERING,2113,382063.350,02000000,471d,15824;INS_SOLUTION_GOOD,INS_RTKFIXED,37.37017959894,126.72086821244,9.9491,22.3000,-0.0011,-0.0001,0.0015,-0.531500302,-0.399820073,84.599734487,0.0909,0.0637,0.0798,0.0013,0.0013,0.0011,0.0180,0.0180,0.0941,0f000045,0*04141345", "robot status", "#INSPVAXA,USB3,0,46.0,FINESTEERING,2113,382063.450,02000000,471d,15824;INS_SOLUTION_GOOD,INS_RTKFIXED,37.37017959775,126.72086821104,9.9491,22.3000,-0.0010,-0.0002,0.0019,-0.531045669,-0.400810751,84.599559456,0.0909,0.0637,0.0798,0.0013,0.0013,0.0011,0.0180,0.0180,0.0941,0f000045,0*992bf93a", "robot status", "#INSPVAXA,USB3,0,46.0,FINESTEERING,2113,382063.500,02000000,471d,15824;INS_SOLUTION_GOOD,INS_RTKFIXED,37.37017959713,126.72086821039,9.9491,22.3000,-0.0011,-0.0003,0.0021,-0.531305857,-0.400180231,84.599813338,0.0909,0.0637,0.0798,0.0013,0.0013,0.0011,0.0180,0.0180,0.0941,0f000045,0*76c9b467", "robot status", "#DUALANTENNAHEADINGA,USB3,0,46.0,FINESTEERING,2113,382063.500,02000000,d426,15824;SOL_COMPUTED,NARROW_INT,-1.000000000,89.977394104,-13.266540527,0.0,0.323650479,0.457443655,\"681H\",36,27,27,21,04,00,30,33*68204c08", "robot status", "#INSPVAXA,USB3,0,46.0,FINESTEERING,2113,382063.550,02000000,471d,15824;INS_SOLUTION_GOOD,INS_RTKFIXED,37.37017959653,126.72086820967,9.9491,22.3000,-0.0009,-0.0003,0.0019,-0.531168913,-0.399832173,84.599617070,0.0909,0.0637,0.0798,0.0013,0.0013,0.0011,0.0180,0.0180,0.0941,0f000045,0*da384413", "robot status", "#INSPVAXA,USB3,0,46.0,FINESTEERING,2113,382063.650,02000000,471d,15824;INS_SOLUTION_GOOD,INS_RTKFIXED,37.37017959543,126.72086820805,9.9491,22.3000,-0.0007,-0.0007,0.0023,-0.530715169,-0.400207708,84.600689847,0.0909,0.0637,0.0798,0.0013,0.0013,0.0011,0.0180,0.0180,0.0941,0f000045,0*e36eff45", "robot status", "#INSPVAXA,USB3,0,46.0,FINESTEERING,2113,382063.700,02000000,471d,15824;INS_SOLUTION_GOOD,INS_RTKFIXED,37.37017959484,126.72086820716,9.9492,22.3000,-0.0007,-0.0007,0.0023,-0.530510978,-0.399991638,84.600223650,0.0909,0.0637,0.0798,0.0013,0.0013,0.0011,0.0180,0.0180,0.0941,0f000045,0*58d575c7", "robot status", "#DUALANTENNAHEADINGA,USB3,0,46.0,FINESTEERING,2113,382063.700,02000000,d426,15824;SOL_COMPUTED,NARROW_INT,-1.000000000,89.968521118,-13.595123291,0.0,0.322906166,0.453821391,\"681H\",36,27,27,21,04,00,30,33*7dd8f773", "robot status", "#INSPVAXA,USB3,0,46.0,FINESTEERING,2113,382063.750,02000000,471d,15824;INS_SOLUTION_GOOD,INS_RTKFIXED,37.37017959431,126.72086820628,9.9492,22.3000,-0.0007,-0.0007,0.0021,-0.531262658,-0.400489850,84.600270206,0.0909,0.0637,0.0798,0.0013,0.0013,0.0011,0.0180,0.0180,0.0941,0f000045,0*e5c39a11", "robot status", "#INSPVAXA,USB3,0,46.0,FINESTEERING,2113,382063.850,02000000,471d,15824;INS_SOLUTION_GOOD,INS_RTKFIXED,37.37017959329,126.72086820440,9.9493,22.3000,-0.0003,-0.0008,0.0023,-0.531124054,-0.399908042,84.599972117,0.0909,0.0637,0.0798,0.0013,0.0013,0.0011,0.0180,0.0180,0.0941,0f000045,0*4624da6e", "robot status", "#INSPVAXA,USB3,0,46.0,FINESTEERING,2113,382063.900,02000000,471d,15824;INS_SOLUTION_GOOD,INS_RTKFIXED,37.37017959287,126.72086820347,9.9493,22.3000,-0.0003,-0.0009,0.0025,-0.530886270,-0.400267324,84.599893955,0.0909,0.0637,0.0798,0.0013,0.0013,0.0011,0.0180,0.0180,0.0941,0f000045,0*d65ee498", "robot status", "#INSPVAXA,USB3,0,46.0,FINESTEERING,2113,382063.950,02000000,471d,15824;INS_SOLUTION_GOOD,INS_RTKFIXED,37.37017959251,126.72086820252,9.9494,22.3000,-0.0001,-0.0008,0.0025,-0.529756923,-0.400505653,84.599797002,0.0909,0.0637,0.0798,0.0013,0.0013,0.0011,0.0180,0.0180,0.0941,0f000045,0*c9ea4b99", "robot status", "#INSPVAXA,USB3,0,46.0,FINESTEERING,2113,382063.950,02000000,471d,15824;INS_SOLUTION_GOOD,INS_RTKFIXED,37.37017959251,126.72086820252,9.9494,22.3000,-0.0001,-0.0008,0.0025,-0.529756923,-0.400505653,84.599797002,0.0909,0.0637,0.0798,0.0013,0.0013,0.0011,0.0180,0.0180,0.0941,0f000045,0*c9ea4b99", "robot status", "#DUALANTENNAHEADINGA,USB3,0,46.0,FINESTEERING,2113,382064.000,02000000,d426,15824;SOL_COMPUTED,NARROW_INT,-1.000000000,90.048553467,-13.322540283,0.0,0.321700245,0.452567607,\"681H\",36,27,27,21,04,00,30,33*267e2f29", "robot status", "#INSPVAXA,USB3,0,45.0,FINESTEERING,2113,382064.100,02000000,471d,15824;INS_SOLUTION_GOOD,INS_RTKFIXED,37.37017959152,126.72086820140,9.9494,22.3000,-0.0004,-0.0006,0.0031,-0.529921539,-0.399617090,84.599119606,0.0880,0.0615,0.0773,0.0013,0.0013,0.0011,0.0180,0.0180,0.0930,0f000045,0*f671d8f3", "robot status", "#INSPVAXA,USB3,0,45.0,FINESTEERING,2113,382064.150,02000000,471d,15824;INS_SOLUTION_GOOD,INS_RTKFIXED,37.37017959123,126.72086820144,9.9493,22.3000,-0.0002,-0.0005,0.0028,-0.530605650,-0.399512203,84.599108682,0.0880,0.0615,0.0773,0.0013,0.0013,0.0011,0.0180,0.0180,0.0930,0f000045,0*f82f7386", "robot status", "#INSPVAXA,USB3,0,45.0,FINESTEERING,2113,382064.150,02000000,471d,15824;INS_SOLUTION_GOOD,INS_RTKFIXED,37.37017959123,126.72086820144,9.9493,22.3000,-0.0002,-0.0005,0.0028,-0.530605650,-0.399512203,84.599108682,0.0880,0.0615,0.0773,0.0013,0.0013,0.0011,0.0180,0.0180,0.0930,0f000045,0*f82f7386", "robot status", "#INSPVAXA,USB3,0,45.0,FINESTEERING,2113,382064.250,02000000,471d,15824;INS_SOLUTION_GOOD,INS_RTKFIXED,37.37017959057,126.72086820147,9.9493,22.3000,-0.0002,-0.0005,0.0031,-0.531289197,-0.399421902,84.600042628,0.0880,0.0615,0.0773,0.0013,0.0013,0.0011,0.0180,0.0180,0.0930,0f000045,0*7108d411", "robot status", "#INSPVAXA,USB3,0,45.0,FINESTEERING,2113,382064.300,02000000,471d,15824;INS_SOLUTION_GOOD,INS_RTKFIXED,37.37017959024,126.72086820157,9.9493,22.3000,-0.0004,-0.0004,0.0032,-0.531261617,-0.399062152,84.600046824,0.0880,0.0615,0.0773,0.0013,0.0013,0.0011,0.0180,0.0180,0.0930,0f000045,0*fc5f63c8", "robot status", "#INSPVAXA,USB3,0,45.0,FINESTEERING,2113,382064.350,02000000,471d,15824;INS_SOLUTION_GOOD,INS_RTKFIXED,37.37017958992,126.72086820165,9.9492,22.3000,-0.0004,-0.0003,0.0028,-0.531397457,-0.398661314,84.600335282,0.0880,0.0615,0.0773,0.0013,0.0013,0.0011,0.0180,0.0180,0.0930,0f000045,0*1c59157a", "robot status", "#INSPVAXA,USB3,0,45.0,FINESTEERING,2113,382064.350,02000000,471d,15824;INS_SOLUTION_GOOD,INS_RTKFIXED,37.37017958992,126.72086820165,9.9492,22.3000,-0.0004,-0.0003,0.0028,-0.531397457,-0.398661314,84.600335282,0.0880,0.0615,0.0773,0.0013,0.0013,0.0011,0.0180,0.0180,0.0930,0f000045,0*1c59157a", "robot status", "#DUALANTENNAHEADINGA,USB3,0,45.0,FINESTEERING,2113,382064.400,02000000,d426,15824;SOL_COMPUTED,NARROW_INT,-1.000000000,90.089302063,-13.128387451,0.0,0.326746911,0.461006761,\"681H\",36,27,27,21,04,00,30,33*76eeb8cc", "robot status", "#INSPVAXA,USB3,0,45.0,FINESTEERING,2113,382064.500,02000000,471d,15824;INS_SOLUTION_GOOD,INS_RTKFIXED,37.37017958887,126.72086820180,9.9492,22.3000,-0.0003,-0.0006,0.0026,-0.531038552,-0.398236849,84.600133960,0.0880,0.0615,0.0773,0.0013,0.0013,0.0011,0.0180,0.0180,0.0930,0f000045,0*858782d5", "robot status", "#INSPVAXA,USB3,0,45.0,FINESTEERING,2113,382064.550,02000000,471d,15824;INS_SOLUTION_GOOD,INS_RTKFIXED,37.37017958861,126.72086820177,9.9492,22.3000,-0.0002,-0.0004,0.0022,-0.531179856,-0.397377345,84.599798579,0.0880,0.0615,0.0773,0.0013,0.0013,0.0011,0.0180,0.0180,0.0930,0f000045,0*c0eed24b", "robot status", "#INSPVAXA,USB3,0,45.0,FINESTEERING,2113,382064.600,02000000,471d,15824;INS_SOLUTION_GOOD,INS_RTKFIXED,37.37017958840,126.72086820172,9.9492,22.3000,-0.0000,-0.0004,0.0024,-0.530766399,-0.397634343,84.599712120,0.0880,0.0615,0.0773,0.0013,0.0013,0.0011,0.0180,0.0180,0.0930,0f000045,0*a60b23f0", "robot status", "#DUALANTENNAHEADINGA,USB3,0,45.0,FINESTEERING,2113,382064.600,02000000,d426,15824;SOL_COMPUTED,NARROW_INT,-1.000000000,90.006744385,-13.242370605,0.0,0.328189790,0.461568981,\"681H\",37,27,27,21,04,00,30,33*6551d4f3", "robot status", "#INSPVAXA,USB3,0,45.0,FINESTEERING,2113,382064.700,02000000,471d,15824;INS_SOLUTION_GOOD,INS_RTKFIXED,37.37017958800,126.72086820161,9.9492,22.3000,0.0000,-0.0004,0.0026,-0.530812248,-0.397231976,84.599520849,0.0880,0.0615,0.0773,0.0013,0.0013,0.0011,0.0180,0.0180,0.0930,0f000045,0*ddbf476c", "robot status", "#INSPVAXA,USB3,0,45.0,FINESTEERING,2113,382064.750,02000000,471d,15824;INS_SOLUTION_GOOD,INS_RTKFIXED,37.37017958779,126.72086820155,9.9492,22.3000,-0.0000,-0.0002,0.0026,-0.530947382,-0.397258541,84.599200394,0.0880,0.0615,0.0773,0.0013,0.0013,0.0011,0.0180,0.0180,0.0930,0f000045,0*102ca7e8", "robot status", "#INSPVAXA,USB3,0,45.0,FINESTEERING,2113,382064.800,02000000,471d,15824;INS_SOLUTION_GOOD,INS_RTKFIXED,37.37017958763,126.72086820144,9.9492,22.3000,0.0003,-0.0004,0.0026,-0.529895606,-0.397503878,84.599474269,0.0880,0.0615,0.0773,0.0013,0.0013,0.0011,0.0180,0.0180,0.0930,0f000045,0*b12e45a2", "robot status", "#DUALANTENNAHEADINGA,USB3,0,45.0,FINESTEERING,2113,382064.800,02000000,d426,15824;SOL_COMPUTED,NARROW_INT,-1.000000000,90.009346008,-13.034606934,0.0,0.326445609,0.459365577,\"681H\",37,27,27,21,04,00,30,33*143fb095", "robot status", "#INSPVAXA,USB3,0,45.0,FINESTEERING,2113,382064.900,02000000,471d,15824;INS_SOLUTION_GOOD,INS_RTKFIXED,37.37017958732,126.72086820112,9.9492,22.3000,0.0001,-0.0005,0.0028,-0.529944435,-0.397250672,84.599735511,0.0880,0.0615,0.0773,0.0013,0.0013,0.0011,0.0180,0.0180,0.0930,0f000045,0*a6c0e08e", "robot status", "#INSPVAXA,USB3,0,45.0,FINESTEERING,2113,382064.950,02000000,471d,15824;INS_SOLUTION_GOOD,INS_RTKFIXED,37.37017958721,126.72086820088,9.9492,22.3000,0.0004,-0.0005,0.0024,-0.529943577,-0.398039765,84.599317480,0.0880,0.0615,0.0773,0.0013,0.0013,0.0011,0.0180,0.0180,0.0930,0f000045,0*b9165797", "robot status", "#INSPVAXA,USB3,0,45.0,FINESTEERING,2113,382065.000,02000000,471d,15824;INS_SOLUTION_GOOD,INS_RTKFIXED,37.37017958708,126.72086820063,9.9493,22.3000,0.0001,-0.0004,0.0023,-0.529272560,-0.398026047,84.600639049,0.0880,0.0615,0.0773,0.0013,0.0013,0.0011,0.0180,0.0180,0.0930,0f000045,0*feb18991", "robot status", "#INSPVAXA,USB3,0,45.0,FINESTEERING,2113,382065.050,02000000,471d,15824;INS_SOLUTION_GOOD,INS_RTKFIXED,37.37017958688,126.72086820038,9.9492,22.3000,0.0003,-0.0005,0.0023,-0.528652322,-0.398858884,84.600310653,0.0853,0.0595,0.0749,0.0013,0.0013,0.0011,0.0180,0.0180,0.0919,0f000045,0*355d199f", "robot status", "#INSPVAXA,USB3,0,45.0,FINESTEERING,2113,382065.100,02000000,471d,15824;INS_SOLUTION_GOOD,INS_RTKFIXED,37.37017958656,126.72086820015,9.9491,22.3000,0.0002,-0.0003,0.0022,-0.529289150,-0.398389157,84.600901777,0.0853,0.0595,0.0749,0.0013,0.0013,0.0011,0.0180,0.0180,0.0919,0f000045,0*a7b5480f", "robot status", "#INSPVAXA,USB3,0,45.5,FINESTEERING,2113,382065.150,02000000,471d,15824;INS_SOLUTION_GOOD,INS_RTKFIXED,37.37017958632,126.72086819994,9.9490,22.3000,0.0002,-0.0002,0.0018,-0.529611899,-0.398229632,84.600391907,0.0853,0.0595,0.0749,0.0013,0.0013,0.0011,0.0180,0.0180,0.0919,0f000045,0*8f89c560", "robot status", "#INSPVAXA,USB3,0,45.5,FINESTEERING,2113,382065.200,02000000,471d,15824;INS_SOLUTION_GOOD,INS_RTKFIXED,37.37017958602,126.72086819973,9.9489,22.3000,-0.0001,-0.0001,0.0021,-0.529291564,-0.398279027,84.600887183,0.0853,0.0595,0.0749,0.0013,0.0013,0.0011,0.0180,0.0180,0.0919,0f000045,0*eeebb4e6", "robot status", "#INSPVAXA,USB3,0,45.5,FINESTEERING,2113,382065.250,02000000,471d,15824;INS_SOLUTION_GOOD,INS_RTKFIXED,37.37017958559,126.72086819953,9.9488,22.3000,0.0000,-0.0002,0.0021,-0.528461563,-0.398734937,84.600806904,0.0853,0.0595,0.0749,0.0013,0.0013,0.0011,0.0180,0.0180,0.0919,0f000045,0*bb95ab59", "robot status", "#INSPVAXA,USB3,0,45.5,FINESTEERING,2113,382065.300,02000000,471d,15824;INS_SOLUTION_GOOD,INS_RTKFIXED,37.37017958523,126.72086819940,9.9487,22.3000,0.0000,-0.0002,0.0020,-0.528439708,-0.398195576,84.600491134,0.0853,0.0595,0.0749,0.0013,0.0013,0.0011,0.0180,0.0180,0.0919,0f000045,0*9f976f4c", "robot status", "#INSPVAXA,USB3,0,45.5,FINESTEERING,2113,382065.350,02000000,471d,15824;INS_SOLUTION_GOOD,INS_RTKFIXED,37.37017958493,126.72086819923,9.9486,22.3000,0.0003,-0.0001,0.0017,-0.529229709,-0.399308678,84.600328511,0.0853,0.0595,0.0749,0.0013,0.0013,0.0011,0.0180,0.0180,0.0919,0f000045,0*d259591b", "robot status", "#INSPVAXA,USB3,0,45.5,FINESTEERING,2113,382065.400,02000000,471d,15824;INS_SOLUTION_GOOD,INS_RTKFIXED,37.37017958472,126.72086819900,9.9485,22.3000,0.0003,-0.0001,0.0017,-0.528964745,-0.399026398,84.601109922,0.0853,0.0595,0.0749,0.0013,0.0013,0.0011,0.0180,0.0180,0.0919,0f000045,0*9eb61d56", "robot status", "#INSPVAXA,USB3,0,45.5,FINESTEERING,2113,382065.450,02000000,471d,15824;INS_SOLUTION_GOOD,INS_RTKFIXED,37.37017958450,126.72086819868,9.9484,22.3000,0.0004,-0.0004,0.0016,-0.529185525,-0.399026325,84.601164149,0.0853,0.0595,0.0749,0.0013,0.0013,0.0011,0.0180,0.0180,0.0919,0f000045,0*e8c65c32", "robot status", "#INSPVAXA,USB3,0,45.5,FINESTEERING,2113,382065.500,02000000,471d,15824;INS_SOLUTION_GOOD,INS_RTKFIXED,37.37017958434,126.72086819842,9.9483,22.3000,0.0003,-0.0003,0.0014,-0.529139970,-0.398965830,84.601112868,0.0853,0.0595,0.0749,0.0013,0.0013,0.0011,0.0180,0.0180,0.0919,0f000045,0*c3e40dad", "robot status", "#INSPVAXA,USB3,0,45.5,FINESTEERING,2113,382065.550,02000000,471d,15824;INS_SOLUTION_GOOD,INS_RTKFIXED,37.37017958414,126.72086819817,9.9482,22.3000,0.0003,-0.0001,0.0010,-0.529537176,-0.398724206,84.601709852,0.0853,0.0595,0.0749,0.0013,0.0013,0.0011,0.0180,0.0180,0.0919,0f000045,0*0415b434", "robot status", "#INSPVAXA,USB3,0,45.5,FINESTEERING,2113,382065.600,02000000,471d,15824;INS_SOLUTION_GOOD,INS_RTKFIXED,37.37017958395,126.72086819789,9.9481,22.3000,0.0002,-0.0002,0.0008,-0.529934423,-0.399615318,84.601852526,0.0853,0.0595,0.0749,0.0013,0.0013,0.0011,0.0180,0.0180,0.0919,0f000045,0*5a21eda9", "robot status", "#INSPVAXA,USB3,0,45.5,FINESTEERING,2113,382065.650,02000000,471d,15824;INS_SOLUTION_GOOD,INS_RTKFIXED,37.37017958374,126.72086819756,9.9480,22.3000,0.0003,-0.0004,0.0010,-0.530233892,-0.399540981,84.602063765,0.0853,0.0595,0.0749,0.0013,0.0013,0.0011,0.0180,0.0180,0.0919,0f000045,0*e92ac972", "robot status", "#DUALANTENNAHEADINGA,USB3,0,45.5,FINESTEERING,2113,382065.700,02000000,d426,15824;SOL_COMPUTED,NARROW_INT,-1.000000000,89.923263550,-13.054534912,0.0,0.478434533,0.877667189,\"681H\",37,27,27,21,04,00,30,33*c2cbf983", "robot status", "#INSPVAXA,USB3,0,45.5,FINESTEERING,2113,382065.750,02000000,471d,15824;INS_SOLUTION_GOOD,INS_RTKFIXED,37.37017958327,126.72086819681,9.9478,22.3000,0.0003,-0.0004,0.0003,-0.529917590,-0.399577616,84.601266643,0.0853,0.0595,0.0749,0.0013,0.0013,0.0011,0.0180,0.0180,0.0919,0f000045,0*d1a5d77c", "robot status", "#INSPVAXA,USB3,0,45.5,FINESTEERING,2113,382065.800,02000000,471d,15824;INS_SOLUTION_GOOD,INS_RTKFIXED,37.37017958311,126.72086819643,9.9476,22.3000,0.0003,-0.0004,0.0003,-0.529438166,-0.399493652,84.601244322,0.0853,0.0595,0.0749,0.0013,0.0013,0.0011,0.0180,0.0180,0.0919,0f000045,0*ff341026", "robot status", "#INSPVAXA,USB3,0,45.5,FINESTEERING,2113,382065.850,02000000,471d,15824;INS_SOLUTION_GOOD,INS_RTKFIXED,37.37017958288,126.72086819601,9.9475,22.3000,0.0004,-0.0005,0.0002,-0.529783933,-0.398896479,84.601349538,0.0853,0.0595,0.0749,0.0013,0.0013,0.0011,0.0180,0.0180,0.0919,0f000045,0*15ffd0b7", "robot status", "#INSPVAXA,USB3,0,45.5,FINESTEERING,2113,382065.900,02000000,471d,15824;INS_SOLUTION_GOOD,INS_RTKFIXED,37.37017958274,126.72086819558,9.9474,22.3000,0.0004,-0.0006,0.0000,-0.530213591,-0.399269254,84.601511214,0.0853,0.0595,0.0749,0.0013,0.0013,0.0011,0.0180,0.0180,0.0919,0f000045,0*623d5226", "robot status", "#INSPVAXA,USB3,0,45.5,FINESTEERING,2113,382065.950,02000000,471d,15824;INS_SOLUTION_GOOD,INS_RTKFIXED,37.37017958259,126.72086819506,9.9473,22.3000,0.0006,-0.0006,-0.0003,-0.530148815,-0.399643881,84.601982197,0.0853,0.0595,0.0749,0.0013,0.0013,0.0011,0.0180,0.0180,0.0919,0f000045,0*7b7cf703", "robot status", "#INSPVAXA,USB3,0,45.5,FINESTEERING,2113,382066.000,02000000,471d,15824;INS_SOLUTION_GOOD,INS_RTKFIXED,37.37017958250,126.72086819449,9.9471,22.3000,0.0006,-0.0006,-0.0002,-0.529743760,-0.399539955,84.601887315,0.0853,0.0595,0.0749,0.0013,0.0013,0.0011,0.0180,0.0180,0.0919,0f000045,0*ca5c2195", "robot status", "#INSPVAXA,USB3,0,45.5,FINESTEERING,2113,382066.050,02000000,471d,15824;INS_SOLUTION_GOOD,INS_RTKFIXED,37.37017958215,126.72086819424,9.9470,22.3000,0.0006,-0.0007,-0.0001,-0.529702998,-0.399954936,84.601932134,0.0829,0.0577,0.0728,0.0013,0.0013,0.0011,0.0180,0.0180,0.0910,0f000045,0*129cb53a", "robot status", "#INSPVAXA,USB3,0,43.5,FINESTEERING,2113,382066.100,02000000,471d,15824;INS_SOLUTION_GOOD,INS_RTKFIXED,37.37017958145,126.72086819421,9.9470,22.3000,0.0003,-0.0006,-0.0002,-0.529821270,-0.399604306,84.600614450,0.0829,0.0577,0.0728,0.0013,0.0013,0.0011,0.0180,0.0180,0.0910,0f000045,0*783dc487", "robot status", "#INSPVAXA,USB3,0,43.5,FINESTEERING,2113,382066.150,02000000,471d,15824;INS_SOLUTION_GOOD,INS_RTKFIXED,37.37017958081,126.72086819412,9.9469,22.3000,0.0001,-0.0004,-0.0006,-0.530081912,-0.399573378,84.600748730,0.0829,0.0577,0.0728,0.0013,0.0013,0.0011,0.0180,0.0180,0.0910,0f000045,0*e0fac88c", "robot status", "#INSPVAXA,USB3,0,43.5,FINESTEERING,2113,382066.200,02000000,471d,15824;INS_SOLUTION_GOOD,INS_RTKFIXED,37.37017958014,126.72086819407,9.9468,22.3000,-0.0001,-0.0003,-0.0006,-0.530033470,-0.399872689,84.600101642,0.0829,0.0577,0.0728,0.0013,0.0013,0.0011,0.0180,0.0180,0.0910,0f000045,0*f695a07d", "robot status", "#INSPVAXA,USB3,0,43.5,FINESTEERING,2113,382066.250,02000000,471d,15824;INS_SOLUTION_GOOD,INS_RTKFIXED,37.37017957935,126.72086819407,9.9467,22.3000,0.0001,-0.0004,-0.0005,-0.529588002,-0.399566709,84.599917015,0.0829,0.0577,0.0728,0.0013,0.0013,0.0011,0.0180,0.0180,0.0910,0f000045,0*8798b05c", "robot status", "#INSPVAXA,USB3,0,43.5,FINESTEERING,2113,382066.300,02000000,471d,15824;INS_SOLUTION_GOOD,INS_RTKFIXED,37.37017957864,126.72086819416,9.9467,22.3000,-0.0001,-0.0002,-0.0006,-0.530167712,-0.399217541,84.599581506,0.0829,0.0577,0.0728,0.0013,0.0013,0.0011,0.0180,0.0180,0.0910,0f000045,0*2cbabc82", "robot status", "#INSPVAXA,USB3,0,43.5,FINESTEERING,2113,382066.350,02000000,471d,15824;INS_SOLUTION_GOOD,INS_RTKFIXED,37.37017957789,126.72086819419,9.9466,22.3000,-0.0000,-0.0002,-0.0008,-0.529548161,-0.398796315,84.599545007,0.0829,0.0577,0.0728,0.0013,0.0013,0.0011,0.0180,0.0180,0.0910,0f000045,0*4adacab0", "robot status", "#INSPVAXA,USB3,0,43.5,FINESTEERING,2113,382066.400,02000000,471d,15824;INS_SOLUTION_GOOD,INS_RTKFIXED,37.37017957711,126.72086819427,9.9465,22.3000,-0.0003,-0.0000,-0.0004,-0.530104534,-0.398985270,84.599743308,0.0829,0.0577,0.0728,0.0013,0.0013,0.0011,0.0180,0.0180,0.0910,0f000045,0*61538b24", "robot status", "#INSPVAXA,USB3,0,43.5,FINESTEERING,2113,382066.450,02000000,471d,15824;INS_SOLUTION_GOOD,INS_RTKFIXED,37.37017957620,126.72086819432,9.9464,22.3000,-0.0002,-0.0001,-0.0003,-0.530372146,-0.398902195,84.600095650,0.0829,0.0577,0.0728,0.0013,0.0013,0.0011,0.0180,0.0180,0.0910,0f000045,0*91118b7d", "robot status", "#INSPVAXA,USB3,0,43.5,FINESTEERING,2113,382066.500,02000000,471d,15824;INS_SOLUTION_GOOD,INS_RTKFIXED,37.37017957542,126.72086819445,9.9464,22.3000,-0.0002,-0.0000,-0.0003,-0.530789561,-0.399382428,84.599670775,0.0829,0.0577,0.0728,0.0013,0.0013,0.0011,0.0180,0.0180,0.0910,0f000045,0*b658781c", "robot status", "#INSPVAXA,USB3,0,43.5,FINESTEERING,2113,382066.550,02000000,471d,15824;INS_SOLUTION_GOOD,INS_RTKFIXED,37.37017957463,126.72086819452,9.9463,22.3000,-0.0001,0.0001,-0.0004,-0.530347449,-0.399467966,84.600151693,0.0829,0.0577,0.0728,0.0013,0.0013,0.0011,0.0180,0.0180,0.0910,0f000045,0*228deed8", "robot status", "#DUALANTENNAHEADINGA,USB3,0,43.5,FINESTEERING,2113,382066.600,02000000,d426,15824;SOL_COMPUTED,NARROW_INT,-1.000000000,90.083740234,-13.159393311,0.0,0.317334384,0.462704003,\"681H\",37,26,26,21,04,00,30,33*dfef526b", "robot status", "#INSPVAXA,USB3,0,43.5,FINESTEERING,2113,382066.650,02000000,471d,15824;INS_SOLUTION_GOOD,INS_RTKFIXED,37.37017957318,126.72086819472,9.9461,22.3000,-0.0001,-0.0000,-0.0003,-0.531496820,-0.400611426,84.599942616,0.0829,0.0577,0.0728,0.0013,0.0013,0.0011,0.0180,0.0180,0.0910,0f000045,0*64570620", "robot status", "#INSPVAXA,USB3,0,43.5,FINESTEERING,2113,382066.700,02000000,471d,15824;INS_SOLUTION_GOOD,INS_RTKFIXED,37.37017957233,126.72086819487,9.9461,22.3000,-0.0003,0.0003,-0.0004,-0.530805075,-0.400024626,84.599421831,0.0829,0.0577,0.0728,0.0013,0.0013,0.0011,0.0180,0.0180,0.0910,0f000045,0*d55abd42", "robot status", "#INSPVAXA,USB3,0,43.5,FINESTEERING,2113,382066.750,02000000,471d,15824;INS_SOLUTION_GOOD,INS_RTKFIXED,37.37017957159,126.72086819502,9.9460,22.3000,-0.0002,0.0002,-0.0007,-0.530751929,-0.399759169,84.599287878,0.0829,0.0577,0.0728,0.0013,0.0013,0.0011,0.0180,0.0180,0.0910,0f000045,0*c1b22ca5", "robot status", "#DUALANTENNAHEADINGA,USB3,0,43.5,FINESTEERING,2113,382066.800,02000000,d426,15824;SOL_COMPUTED,NARROW_INT,-1.000000000,90.035583496,-13.116455078,0.0,0.318032831,0.463907361,\"681H\",37,26,26,21,04,00,30,33*acd5bd57", "robot status", "#INSPVAXA,USB3,0,43.5,FINESTEERING,2113,382066.850,02000000,471d,15824;INS_SOLUTION_GOOD,INS_RTKFIXED,37.37017957007,126.72086819567,9.9458,22.3000,-0.0000,0.0007,-0.0002,-0.531329896,-0.400807373,84.600507690,0.0829,0.0577,0.0728,0.0013,0.0013,0.0011,0.0180,0.0180,0.0910,0f000045,0*81cddf55", "robot status", "#INSPVAXA,USB3,0,43.5,FINESTEERING,2113,382066.900,02000000,471d,15824;INS_SOLUTION_GOOD,INS_RTKFIXED,37.37017956934,126.72086819579,9.9458,22.3000,-0.0005,-0.0004,-0.0003,-0.531583844,-0.401885892,84.600565950,0.0829,0.0577,0.0728,0.0013,0.0013,0.0011,0.0180,0.0180,0.0910,0f000045,0*3c5f5aca", "robot status", "#INSPVAXA,USB3,0,43.5,FINESTEERING,2113,382066.950,02000000,471d,15824;INS_SOLUTION_GOOD,INS_RTKFIXED,37.37017956860,126.72086819572,9.9457,22.3000,-0.0001,0.0005,-0.0007,-0.532448900,-0.403893349,84.603232338,0.0829,0.0577,0.0728,0.0013,0.0013,0.0011,0.0180,0.0180,0.0910,0f000045,0*4a91cf03", "robot status", "#DUALANTENNAHEADINGA,USB3,0,43.5,FINESTEERING,2113,382067.000,02000000,d426,15824;SOL_COMPUTED,NARROW_INT,-1.000000000,90.066551208,-13.218780518,0.0,0.317091048,0.463003188,\"681H\",37,26,26,21,04,00,30,33*25538102", "robot status", "#INSPVAXA,USB3,0,43.5,FINESTEERING,2113,382067.050,02000000,471d,15824;INS_SOLUTION_GOOD,INS_RTKFIXED,37.37017956738,126.72086819524,9.9456,22.3000,-0.0003,0.0003,-0.0003,-0.530710862,-0.401810279,84.600597620,0.0807,0.0561,0.0709,0.0013,0.0013,0.0011,0.0180,0.0180,0.0900,0f000045,0*8ed2c4e0", "robot status", "#INSPVAXA,USB3,0,45.5,FINESTEERING,2113,382067.100,02000000,471d,15824;INS_SOLUTION_GOOD,INS_RTKFIXED,37.37017956754,126.72086819478,9.9455,22.3000,-0.0005,0.0009,-0.0001,-0.532108252,-0.403171533,84.601667013,0.0807,0.0561,0.0709,0.0013,0.0013,0.0011,0.0180,0.0180,0.0900,0f000045,0*9af7d1a9", "robot status", "#INSPVAXA,USB3,0,45.5,FINESTEERING,2113,382067.150,02000000,471d,15824;INS_SOLUTION_GOOD,INS_RTKFIXED,37.37017956761,126.72086819446,9.9454,22.3000,-0.0007,0.0008,0.0003,-0.532196472,-0.402073419,84.599798100,0.0807,0.0561,0.0709,0.0013,0.0013,0.0011,0.0180,0.0180,0.0900,0f000045,0*1dc3605e", "robot status", "#DUALANTENNAHEADINGA,USB3,0,45.5,FINESTEERING,2113,382067.200,02000000,d426,15824;SOL_COMPUTED,NARROW_INT,-1.000000000,89.917945862,-13.216949463,0.0,0.474367589,0.867645264,\"681H\",37,27,27,22,04,00,30,33*92e21af1", "robot status", "#INSPVAXA,USB3,0,45.5,FINESTEERING,2113,382067.250,02000000,471d,15824;INS_SOLUTION_GOOD,INS_RTKFIXED,37.37017956748,126.72086819332,9.9453,22.3000,-0.0008,0.0001,0.0003,-0.532951223,-0.402732578,84.600913663,0.0807,0.0561,0.0709,0.0013,0.0013,0.0011,0.0180,0.0180,0.0900,0f000045,0*432b43a4", "robot status", "#INSPVAXA,USB3,0,45.5,FINESTEERING,2113,382067.300,02000000,471d,15824;INS_SOLUTION_GOOD,INS_RTKFIXED,37.37017956740,126.72086819344,9.9452,22.3000,-0.0007,0.0022,-0.0004,-0.533263571,-0.402498957,84.599710266,0.0807,0.0561,0.0709,0.0013,0.0013,0.0011,0.0180,0.0180,0.0900,0f000045,0*c3133298", "robot status", "#INSPVAXA,USB3,0,45.5,FINESTEERING,2113,382067.350,02000000,471d,15824;INS_SOLUTION_GOOD,INS_RTKFIXED,37.37017956730,126.72086819341,9.9452,22.3000,-0.0009,0.0008,-0.0003,-0.533481705,-0.404966683,84.604665115,0.0807,0.0561,0.0709,0.0013,0.0013,0.0011,0.0180,0.0180,0.0900,0f000045,0*a7ee1d15", "robot status", "#DUALANTENNAHEADINGA,USB3,0,45.5,FINESTEERING,2113,382067.400,02000000,d426,15824;SOL_COMPUTED,NARROW_INT,-1.000000000,89.892951965,-13.080505371,0.0,0.473694414,0.864680827,\"681H\",37,27,27,22,04,00,30,33*0ea0cd18", "robot status", "#INSPVAXA,USB3,0,45.5,FINESTEERING,2113,382067.450,02000000,471d,15824;INS_SOLUTION_GOOD,INS_RTKFIXED,37.37017956676,126.72086819072,9.9450,22.3000,-0.0011,-0.0012,-0.0002,-0.532027829,-0.401249007,84.601247560,0.0807,0.0561,0.0709,0.0013,0.0013,0.0011,0.0180,0.0180,0.0900,0f000045,0*e2e4e5ae", "robot status", "#INSPVAXA,USB3,0,45.5,FINESTEERING,2113,382067.500,02000000,471d,15824;INS_SOLUTION_GOOD,INS_RTKFIXED,37.37017956661,126.72086818987,9.9450,22.3000,-0.0005,0.0006,-0.0003,-0.533329879,-0.401270375,84.603561731,0.0807,0.0561,0.0709,0.0013,0.0013,0.0011,0.0180,0.0180,0.0900,0f000045,0*aac3fca2", "robot status", "#INSPVAXA,USB3,0,45.5,FINESTEERING,2113,382067.550,02000000,471d,15824;INS_SOLUTION_GOOD,INS_RTKFIXED,37.37017956658,126.72086819013,9.9449,22.3000,-0.0005,0.0030,0.0001,-0.535351782,-0.402604285,84.600388031,0.0807,0.0561,0.0709,0.0013,0.0013,0.0011,0.0180,0.0180,0.0900,0f000045,0*68376a5a", "robot status", "#DUALANTENNAHEADINGA,USB3,0,45.5,FINESTEERING,2113,382067.600,02000000,d426,15824;SOL_COMPUTED,NARROW_INT,-1.000000000,89.985420227,-13.320678711,0.0,0.476984203,0.868541121,\"681H\",37,26,26,21,04,00,30,33*30e69b20", "robot status", "#INSPVAXA,USB3,0,45.5,FINESTEERING,2113,382067.650,02000000,471d,15824;INS_SOLUTION_GOOD,INS_RTKFIXED,37.37017956655,126.72086818908,9.9448,22.3000,-0.0007,-0.0023,0.0002,-0.534505717,-0.403345386,84.605635436,0.0807,0.0561,0.0709,0.0013,0.0013,0.0011,0.0180,0.0180,0.0900,0f000045,0*ce759fcf", "robot status", "#DUALANTENNAHEADINGA,USB3,0,45.5,FINESTEERING,2113,382067.700,02000000,d426,15824;SOL_COMPUTED,NARROW_INT,-1.000000000,89.854522705,-13.544799805,0.0,0.480057657,0.873438954,\"681H\",37,26,26,21,04,00,30,33*26cb4598", "robot status", "#INSPVAXA,USB3,0,45.5,FINESTEERING,2113,382067.750,02000000,471d,15824;INS_SOLUTION_GOOD,INS_RTKFIXED,37.37017956620,126.72086818551,9.9448,22.3000,-0.0000,-0.0002,0.0004,-0.533527712,-0.400152135,84.602295196,0.0807,0.0561,0.0709,0.0013,0.0013,0.0011,0.0180,0.0180,0.0900,0f000045,0*62df8fab", "robot status", "#DUALANTENNAHEADINGA,USB3,0,45.5,FINESTEERING,2113,382067.800,02000000,d426,15824;SOL_COMPUTED,NARROW_INT,-1.000000000,90.083251953,-13.109008789,0.0,0.475750387,0.870726526,\"681H\",37,26,26,21,04,00,30,33*124bdf4e", "robot status", "#INSPVAXA,USB3,0,45.5,FINESTEERING,2113,382067.850,02000000,471d,15824;INS_SOLUTION_GOOD,INS_RTKFIXED,37.37017956657,126.72086818541,9.9447,22.3000,0.0006,0.0005,0.0005,-0.534154724,-0.404121709,84.599430830,0.0807,0.0561,0.0709,0.0013,0.0013,0.0011,0.0180,0.0180,0.0900,0f000045,0*5ce0d941", "robot status", "#INSPVAXA,USB3,0,45.5,FINESTEERING,2113,382067.900,02000000,471d,15824;INS_SOLUTION_GOOD,INS_RTKFIXED,37.37017956699,126.72086818478,9.9446,22.3000,0.0008,0.0002,-0.0000,-0.534543904,-0.399814340,84.605316792,0.0807,0.0561,0.0709,0.0013,0.0013,0.0011,0.0180,0.0180,0.0900,0f000045,0*d48b1bcd", "robot status", "#INSPVAXA,USB3,0,45.5,FINESTEERING,2113,382067.950,02000000,471d,15824;INS_SOLUTION_GOOD,INS_RTKFIXED,37.37017956744,126.72086818438,9.9446,22.3000,0.0008,0.0003,-0.0003,-0.535916481,-0.401813924,84.605760395,0.0807,0.0561,0.0709,0.0013,0.0013,0.0011,0.0180,0.0180,0.0900,0f000045,0*e28e21bf", "robot status", "#DUALANTENNAHEADINGA,USB3,0,45.5,FINESTEERING,2113,382068.000,02000000,d426,15824;SOL_COMPUTED,NARROW_INT,-1.000000000,89.975334167,-13.217712402,0.0,0.475380272,0.868653357,\"681H\",37,26,26,21,04,00,30,33*75a593ca", "robot status", "#INSPVAXA,USB3,0,45.5,FINESTEERING,2113,382068.050,02000000,471d,15824;INS_SOLUTION_GOOD,INS_RTKFIXED,37.37017956750,126.72086818191,9.9445,22.3000,0.0002,-0.0042,-0.0003,-0.534552805,-0.403207748,84.604161868,0.0786,0.0546,0.0691,0.0013,0.0013,0.0011,0.0180,0.0180,0.0891,0f000045,0*2991b514", "robot status", "#DUALANTENNAHEADINGA,USB3,0,45.5,FINESTEERING,2113,382068.100,02000000,d426,15824;SOL_COMPUTED,NARROW_INT,-1.000000000,89.885818481,-13.854248047,0.0,0.474171758,0.863298416,\"681H\",37,26,26,21,04,00,30,33*8b0b1d7a", "robot status", "#INSPVAXA,USB3,0,46.0,FINESTEERING,2113,382068.150,02000000,471d,15824;INS_SOLUTION_GOOD,INS_RTKFIXED,37.37017956760,126.72086818196,9.9444,22.3000,0.0016,0.0049,-0.0033,-0.557974286,-0.378775955,84.690740567,0.0786,0.0546,0.0691,0.0013,0.0013,0.0011,0.0180,0.0180,0.0891,0f000045,0*eca0edd7", "robot status", "#DUALANTENNAHEADINGA,USB3,0,46.0,FINESTEERING,2113,382068.200,02000000,d426,15824;SOL_COMPUTED,NARROW_INT,-1.000000000,90.122421265,-13.320343018,0.0,0.475840926,0.870335281,\"681H\",37,26,26,21,04,00,30,33*47ecb98f", "robot status", "#INSPVAXA,USB3,0,46.0,FINESTEERING,2113,382068.250,02000000,471d,15824;INS_SOLUTION_GOOD,INS_RTKFIXED,37.37017956502,126.72086819809,9.9442,22.3000,-0.0007,0.0178,0.0003,-0.583992517,-0.371452909,84.779265138,0.0786,0.0546,0.0691,0.0013,0.0013,0.0011,0.0180,0.0180,0.0891,0f000045,0*1575097c", "robot status", "#DUALANTENNAHEADINGA,USB3,0,46.0,FINESTEERING,2113,382068.300,02000000,d426,15824;SOL_COMPUTED,NARROW_INT,-1.000000000,90.103507996,-13.267456055,0.0,0.475297809,0.869124651,\"681H\",37,26,26,21,04,00,30,33*922b9420", "robot status", "#INSPVAXA,USB3,0,46.0,FINESTEERING,2113,382068.350,02000000,471d,15824;INS_SOLUTION_GOOD,INS_RTKFIXED,37.37017956883,126.72086821699,9.9442,22.3000,0.0030,0.0143,-0.0006,-0.595363685,-0.375172102,84.774288518,0.0786,0.0546,0.0691,0.0013,0.0013,0.0011,0.0180,0.0180,0.0891,0f000045,0*031f4309", "robot status", "#DUALANTENNAHEADINGA,USB3,0,46.0,FINESTEERING,2113,382068.400,02000000,d426,15824;SOL_COMPUTED,NARROW_INT,-1.000000000,90.142776489,-13.373718262,0.0,0.473428279,0.865718484,\"681H\",37,26,26,21,04,00,30,33*12381735", "robot status", "#INSPVAXA,USB3,0,46.0,FINESTEERING,2113,382068.450,02000000,471d,15824;INS_SOLUTION_GOOD,INS_RTKFIXED,37.37017956818,126.72086823255,9.9441,22.3000,0.0030,0.0103,0.0000,-0.586537373,-0.377590392,84.789416389,0.0786,0.0546,0.0691,0.0013,0.0013,0.0011,0.0180,0.0180,0.0891,0f000045,0*3a358f10", "robot status", "#DUALANTENNAHEADINGA,USB3,0,46.0,FINESTEERING,2113,382068.500,02000000,d426,15824;SOL_COMPUTED,NARROW_INT,-1.000000000,90.141029358,-13.346954346,0.0,0.476865083,0.869763017,\"681H\",37,26,26,21,04,00,30,33*fb31385d", "robot status", "#INSPVAXA,USB3,0,46.0,FINESTEERING,2113,382068.550,02000000,471d,15824;INS_SOLUTION_GOOD,INS_RTKFIXED,37.37017957050,126.72086824243,9.9440,22.3000,0.0001,0.0058,-0.0001,-0.594878439,-0.379255370,84.786250372,0.0786,0.0546,0.0691,0.0013,0.0013,0.0011,0.0180,0.0180,0.0891,0f000045,0*081ed6e7", "robot status", "#DUALANTENNAHEADINGA,USB3,0,46.0,FINESTEERING,2113,382068.600,02000000,d426,15824;SOL_COMPUTED,NARROW_INT,-1.000000000,90.184509277,-13.563659668,0.0,0.474369049,0.864366472,\"681H\",36,25,25,20,04,00,30,33*ff3c605f", "robot status", "#INSPVAXA,USB3,0,46.0,FINESTEERING,2113,382068.650,02000000,471d,15824;INS_SOLUTION_GOOD,INS_RTKFIXED,37.37017957063,126.72086824715,9.9440,22.3000,0.0030,0.0014,0.0001,-0.593000480,-0.380386455,84.796034157,0.0786,0.0546,0.0691,0.0013,0.0013,0.0011,0.0180,0.0180,0.0891,0f000045,0*55ba94a4", "robot status", "#DUALANTENNAHEADINGA,USB3,0,46.0,FINESTEERING,2113,382068.700,02000000,d426,15824;SOL_COMPUTED,NARROW_INT,-1.000000000,90.232742310,-13.519989014,0.0,0.474208713,0.863431811,\"681H\",37,25,25,20,04,00,30,33*c288f3df", "robot status", "#INSPVAXA,USB3,0,46.0,FINESTEERING,2113,382068.750,02000000,471d,15824;INS_SOLUTION_GOOD,INS_RTKFIXED,37.37017957159,126.72086824811,9.9439,22.3000,0.0002,0.0001,-0.0002,-0.594365779,-0.379757770,84.792580752,0.0786,0.0546,0.0691,0.0013,0.0013,0.0011,0.0180,0.0180,0.0891,0f000045,0*3261ea44", "robot status", "#DUALANTENNAHEADINGA,USB3,0,46.0,FINESTEERING,2113,382068.800,02000000,d426,15824;SOL_COMPUTED,NARROW_INT,-1.000000000,90.126564026,-13.369903564,0.0,0.476948857,0.866505861,\"681H\",36,25,25,20,04,00,30,33*6135a8af", "robot status", "#INSPVAXA,USB3,0,46.0,FINESTEERING,2113,382068.850,02000000,471d,15824;INS_SOLUTION_GOOD,INS_RTKFIXED,37.37017957244,126.72086824880,9.9438,22.3000,0.0026,0.0007,0.0002,-0.595280004,-0.378996424,84.794223591,0.0786,0.0546,0.0691,0.0013,0.0013,0.0011,0.0180,0.0180,0.0891,0f000045,0*1c66048a", "robot status", "#DUALANTENNAHEADINGA,USB3,0,46.0,FINESTEERING,2113,382068.900,02000000,d426,15824;SOL_COMPUTED,NARROW_INT,-1.000000000,90.085632324,-13.677215576,0.0,0.478393853,0.865787566,\"681H\",36,25,25,20,04,00,30,33*a121abb4", "robot status", "#INSPVAXA,USB3,0,46.0,FINESTEERING,2113,382068.950,02000000,471d,15824;INS_SOLUTION_GOOD,INS_RTKFIXED,37.37017957319,126.72086825100,9.9438,22.3000,0.0013,0.0023,0.0002,-0.595078602,-0.379578166,84.796731665,0.0786,0.0546,0.0691,0.0013,0.0013,0.0011,0.0180,0.0180,0.0891,0f000045,0*9eb9640a", "robot status", "#DUALANTENNAHEADINGA,USB3,0,46.0,FINESTEERING,2113,382069.000,02000000,d426,15824;SOL_COMPUTED,NARROW_INT,-1.000000000,90.136154175,-13.771484375,0.0,0.476806760,0.863958716,\"681H\",37,25,25,20,04,00,30,33*d7ad3bfb", "robot status", "#INSPVAXA,USB3,0,46.0,FINESTEERING,2113,382069.050,02000000,471d,15824;INS_SOLUTION_GOOD,INS_RTKFIXED,37.37017957464,126.72086825353,9.9438,22.3000,0.0021,0.0023,0.0007,-0.597230939,-0.380554569,84.794468311,0.0772,0.0538,0.0679,0.0087,0.0087,0.0083,0.0197,0.0197,0.0897,0f000041,0*d086722f", "robot status", "#DUALANTENNAHEADINGA,USB3,0,46.0,FINESTEERING,2113,382069.100,02000000,d426,15824;SOL_COMPUTED,NARROW_INT,-1.000000000,90.074874878,-13.217712402,0.0,0.473540932,0.859094441,\"681H\",36,25,25,20,04,00,30,33*df84935e", "robot status", "#INSPVAXA,USB3,0,46.0,FINESTEERING,2113,382069.150,02000000,471d,15824;INS_SOLUTION_GOOD,INS_RTKFIXED,37.37017957573,126.72086825594,9.9437,22.3000,0.0028,0.0028,0.0002,-0.596172761,-0.380216548,84.796630287,0.0772,0.0538,0.0679,0.0087,0.0087,0.0083,0.0197,0.0197,0.0897,0f000041,0*fa7feb20", "robot status", "#DUALANTENNAHEADINGA,USB3,0,46.0,FINESTEERING,2113,382069.200,02000000,d426,15824;SOL_COMPUTED,NARROW_INT,-1.000000000,90.065986633,-13.339416504,0.0,0.319388896,0.450993955,\"681H\",36,25,25,20,04,00,30,33*9272d560", "robot status", "#INSPVAXA,USB3,0,46.0,FINESTEERING,2113,382069.250,02000000,471d,15824;INS_SOLUTION_GOOD,INS_RTKFIXED,37.37017957779,126.72086826234,9.9437,22.3000,0.0030,0.0102,0.0005,-0.599078788,-0.376267628,84.796307197,0.0772,0.0538,0.0679,0.0087,0.0087,0.0083,0.0197,0.0197,0.0897,0f000041,0*122b9589", "robot status", "#DUALANTENNAHEADINGA,USB3,0,46.0,FINESTEERING,2113,382069.300,02000000,d426,15824;SOL_COMPUTED,NARROW_INT,-1.000000000,90.207122803,-13.154327393,0.0,0.317266643,0.449597001,\"681H\",36,25,25,20,04,00,30,33*50e73a86", "robot status", "#INSPVAXA,USB3,0,46.0,FINESTEERING,2113,382069.350,02000000,471d,15824;INS_SOLUTION_GOOD,INS_RTKFIXED,37.37017958083,126.72086827970,9.9437,22.3000,0.0054,0.0213,-0.0001,-0.600531163,-0.375743206,84.810081949,0.0772,0.0538,0.0679,0.0087,0.0087,0.0083,0.0197,0.0197,0.0897,0f000041,0*33270510", "robot status", "#DUALANTENNAHEADINGA,USB3,0,46.0,FINESTEERING,2113,382069.400,02000000,d426,15824;SOL_COMPUTED,NARROW_INT,-1.000000000,90.162498474,-12.966796875,0.0,0.315708518,0.448348403,\"681H\",36,25,25,20,04,00,30,33*06c60311", "robot status", "#INSPVAXA,USB3,0,46.0,FINESTEERING,2113,382069.450,02000000,471d,15824;INS_SOLUTION_GOOD,INS_RTKFIXED,37.37017958446,126.72086830585,9.9436,22.3000,0.0045,0.0241,0.0004,-0.596916668,-0.381593958,84.804773998,0.0772,0.0538,0.0679,0.0087,0.0087,0.0083,0.0197,0.0197,0.0897,0f000041,0*2a8d11c5", "robot status", "#DUALANTENNAHEADINGA,USB3,0,46.0,FINESTEERING,2113,382069.500,02000000,d426,15824;SOL_COMPUTED,NARROW_INT,-1.000000000,90.122657776,-13.570556641,0.0,0.320855975,0.460683316,\"681H\",36,25,25,19,04,00,30,33*faf96a53", "robot status", "#INSPVAXA,USB3,0,46.0,FINESTEERING,2113,382069.550,02000000,471d,15824;INS_SOLUTION_GOOD,INS_RTKFIXED,37.37017958790,126.72086832911,9.9436,22.3000,0.0043,0.0173,-0.0001,-0.597007765,-0.382991694,84.821373877,0.0772,0.0538,0.0679,0.0087,0.0087,0.0083,0.0197,0.0197,0.0897,0f000041,0*aa48a688", "robot status", "#DUALANTENNAHEADINGA,USB3,0,46.0,FINESTEERING,2113,382069.600,02000000,d426,15824;SOL_COMPUTED,NARROW_INT,-1.000000000,90.386726379,-13.099578857,0.0,0.319248110,0.470308840,\"681H\",36,24,24,18,04,00,30,33*36ba8013", "robot status", "#INSPVAXA,USB3,0,46.0,FINESTEERING,2113,382069.650,02000000,471d,15824;INS_SOLUTION_GOOD,INS_RTKFIXED,37.37017959083,126.72086834310,9.9435,22.3000,0.0036,0.0086,0.0001,-0.594285176,-0.383287555,84.814922670,0.0772,0.0538,0.0679,0.0087,0.0087,0.0083,0.0197,0.0197,0.0897,0f000041,0*f292548e", "robot status", "#DUALANTENNAHEADINGA,USB3,0,46.0,FINESTEERING,2113,382069.700,02000000,d426,15824;SOL_COMPUTED,NARROW_INT,-1.000000000,90.219703674,-13.177124023,0.0,0.319607317,0.470176995,\"681H\",36,24,24,18,04,00,30,33*d9833a1e", "robot status", "#INSPVAXA,USB3,0,46.0,FINESTEERING,2113,382069.750,02000000,471d,15824;INS_SOLUTION_GOOD,INS_RTKFIXED,37.37017959286,126.72086834824,9.9435,22.3000,0.0029,0.0015,0.0006,-0.594559630,-0.381501928,84.818904706,0.0772,0.0538,0.0679,0.0087,0.0087,0.0083,0.0197,0.0197,0.0897,0f000041,0*2df41f26", "robot status", "#DUALANTENNAHEADINGA,USB3,0,46.0,FINESTEERING,2113,382069.800,02000000,d426,15824;SOL_COMPUTED,NARROW_INT,-1.000000000,90.299545288,-13.396514893,0.0,0.319590241,0.468799740,\"681H\",36,24,24,18,04,00,30,33*e1aa8ed2", "robot status", "#INSPVAXA,USB3,0,46.0,FINESTEERING,2113,382069.850,02000000,471d,15824;INS_SOLUTION_GOOD,INS_RTKFIXED,37.37017959483,126.72086834852,9.9435,22.3000,0.0028,0.0008,0.0003,-0.595658209,-0.379112271,84.825189948,0.0772,0.0538,0.0679,0.0087,0.0087,0.0083,0.0197,0.0197,0.0897,0f000041,0*d0183e8f", "robot status", "#DUALANTENNAHEADINGA,USB3,0,46.0,FINESTEERING,2113,382069.900,02000000,d426,15824;SOL_COMPUTED,NARROW_INT,-1.000000000,90.336624146,-13.340576172,0.0,0.319771528,0.469872594,\"681H\",36,24,24,18,04,00,30,33*5d1460be", "robot status", "#INSPVAXA,USB3,0,46.0,FINESTEERING,2113,382069.950,02000000,471d,15824;INS_SOLUTION_GOOD,INS_RTKFIXED,37.37017959702,126.72086835074,9.9434,22.3000,0.0036,0.0037,0.0005,-0.594621390,-0.376739995,84.825449096,0.0772,0.0538,0.0679,0.0087,0.0087,0.0083,0.0197,0.0197,0.0897,0f000041,0*27949776", "robot status", "#DUALANTENNAHEADINGA,USB3,0,46.0,FINESTEERING,2113,382070.000,02000000,d426,15824;SOL_COMPUTED,NARROW_INT,-1.000000000,89.993789673,-13.240814209,0.0,0.320609182,0.471159637,\"681H\",36,24,24,18,04,00,30,33*9564a670", "robot status", "#INSPVAXA,USB3,0,46.0,FINESTEERING,2113,382070.050,02000000,471d,15824;INS_SOLUTION_GOOD,INS_RTKFIXED,37.37017959987,126.72086835508,9.9434,22.3000,0.0037,0.0042,0.0001,-0.594962500,-0.378543884,84.822095176,0.0770,0.0547,0.0681,0.0125,0.0125,0.0118,0.0212,0.0213,0.0903,0f000041,0*f9c5bdd8", "robot status", "#DUALANTENNAHEADINGA,USB3,0,46.0,FINESTEERING,2113,382070.100,02000000,d426,15824;SOL_COMPUTED,NARROW_INT,-1.000000000,90.128929138,-12.934967041,0.0,0.318057060,0.468930453,\"681H\",36,24,24,18,04,00,30,33*00ac6dea", "robot status", "#INSPVAXA,USB3,0,46.0,FINESTEERING,2113,382070.150,02000000,471d,15824;INS_SOLUTION_GOOD,INS_RTKFIXED,37.37017960258,126.72086835730,9.9434,22.3000,0.0038,0.0020,0.0006,-0.594837635,-0.379279499,84.823886082,0.0770,0.0547,0.0681,0.0125,0.0125,0.0118,0.0212,0.0213,0.0903,0f000041,0*739c2424", "robot status", "#DUALANTENNAHEADINGA,USB3,0,46.0,FINESTEERING,2113,382070.200,02000000,d426,15824;SOL_COMPUTED,NARROW_INT,-1.000000000,89.901245117,-13.371643066,0.0,0.470909536,0.864247501,\"681H\",36,25,25,19,04,00,30,33*7ab83f5d", "robot status", "#INSPVAXA,USB3,0,46.0,FINESTEERING,2113,382070.250,02000000,471d,15824;INS_SOLUTION_GOOD,INS_RTKFIXED,37.37017960554,126.72086835840,9.9433,22.3000,0.0044,0.0022,0.0002,-0.596110577,-0.377774161,84.824190865,0.0770,0.0547,0.0681,0.0125,0.0125,0.0118,0.0212,0.0213,0.0903,0f000041,0*3914d794", "robot status", "#DUALANTENNAHEADINGA,USB3,0,46.0,FINESTEERING,2113,382070.300,02000000,d426,15824;SOL_COMPUTED,NARROW_INT,-1.000000000,90.105155945,-12.295074463,0.0,0.476871729,0.976301491,\"681H\",36,24,24,18,04,00,30,33*2179d57c", "robot status", "#INSPVAXA,USB3,0,46.0,FINESTEERING,2113,382070.350,02000000,471d,15824;INS_SOLUTION_GOOD,INS_RTKFIXED,37.37017960885,126.72086836018,9.9433,22.3000,0.0047,0.0028,0.0004,-0.596272578,-0.378474798,84.823018076,0.0770,0.0547,0.0681,0.0125,0.0125,0.0118,0.0212,0.0213,0.0903,0f000041,0*073c2ca7", "robot status", "#DUALANTENNAHEADINGA,USB3,0,46.0,FINESTEERING,2113,382070.400,02000000,d426,15824;SOL_COMPUTED,NARROW_INT,-1.000000000,89.915763855,-12.917205811,0.0,0.487238795,0.993889093,\"681H\",36,24,24,18,04,00,30,33*b39a7c88", "robot status", "#INSPVAXA,USB3,0,46.0,FINESTEERING,2113,382070.450,02000000,471d,15824;INS_SOLUTION_GOOD,INS_RTKFIXED,37.37017961250,126.72086836205,9.9432,22.3000,0.0049,0.0022,0.0003,-0.596786883,-0.377860830,84.822701660,0.0770,0.0547,0.0681,0.0125,0.0125,0.0118,0.0212,0.0213,0.0903,0f000041,0*237af43c", "robot status", "#INSPVAXA,USB3,0,46.0,FINESTEERING,2113,382070.550,02000000,471d,15824;INS_SOLUTION_GOOD,INS_RTKFIXED,37.37017961625,126.72086836331,9.9432,22.3000,0.0049,0.0018,0.0000,-0.597856165,-0.377915716,84.822609255,0.0770,0.0547,0.0681,0.0125,0.0125,0.0118,0.0212,0.0213,0.0903,0f000041,0*02f0c77c", "robot status", "#INSPVAXA,USB3,0,46.0,FINESTEERING,2113,382070.550,02000000,471d,15824;INS_SOLUTION_GOOD,INS_RTKFIXED,37.37017961625,126.72086836331,9.9432,22.3000,0.0049,0.0018,0.0000,-0.597856165,-0.377915716,84.822609255,0.0770,0.0547,0.0681,0.0125,0.0125,0.0118,0.0212,0.0213,0.0903,0f000041,0*02f0c77c", "robot status", "#DUALANTENNAHEADINGA,USB3,0,46.0,FINESTEERING,2113,382070.600,02000000,d426,15824;SOL_COMPUTED,NARROW_INT,-1.000000000,90.015579224,-13.711334229,0.0,0.471969426,0.863615513,\"681H\",36,25,25,19,04,00,30,33*130f5095", "robot status", "#INSPVAXA,USB3,0,46.0,FINESTEERING,2113,382070.650,02000000,471d,15824;INS_SOLUTION_GOOD,INS_RTKFIXED,37.37017962013,126.72086836437,9.9431,22.3000,0.0052,0.0018,0.0003,-0.598830455,-0.377953454,84.822305427,0.0770,0.0547,0.0681,0.0125,0.0125,0.0118,0.0212,0.0213,0.0903,0f000041,0*fb5be60b", "robot status", "#INSPVAXA,USB3,0,46.0,FINESTEERING,2113,382070.750,02000000,471d,15824;INS_SOLUTION_GOOD,INS_RTKFIXED,37.37017962432,126.72086836567,9.9431,22.3000,0.0055,0.0021,-0.0000,-0.599325942,-0.377958582,84.821755205,0.0770,0.0547,0.0681,0.0125,0.0125,0.0118,0.0212,0.0213,0.0903,0f000041,0*390999e1", "robot status", "#INSPVAXA,USB3,0,46.0,FINESTEERING,2113,382070.750,02000000,471d,15824;INS_SOLUTION_GOOD,INS_RTKFIXED,37.37017962432,126.72086836567,9.9431,22.3000,0.0055,0.0021,-0.0000,-0.599325942,-0.377958582,84.821755205,0.0770,0.0547,0.0681,0.0125,0.0125,0.0118,0.0212,0.0213,0.0903,0f000041,0*390999e1", "robot status", "#DUALANTENNAHEADINGA,USB3,0,46.0,FINESTEERING,2113,382070.800,02000000,d426,15824;SOL_COMPUTED,NARROW_INT,-1.000000000,90.050712585,-13.640777588,0.0,0.474688500,0.867491066,\"681H\",36,25,25,19,04,00,30,33*04a42cd6", "robot status", "#INSPVAXA,USB3,0,46.0,FINESTEERING,2113,382070.900,02000000,471d,15824;INS_SOLUTION_GOOD,INS_RTKFIXED,37.37017963108,126.72086836751,9.9430,22.3000,0.0061,0.0020,0.0005,-0.599704789,-0.377248389,84.822155928,0.0770,0.0547,0.0681,0.0125,0.0125,0.0118,0.0212,0.0213,0.0903,0f000041,0*6ed7df37", "robot status", "#DUALANTENNAHEADINGA,USB3,0,46.0,FINESTEERING,2113,382070.900,02000000,d426,15824;SOL_COMPUTED,NARROW_INT,-1.000000000,90.056266785,-13.334869385,0.0,0.471115530,0.863354743,\"681H\",36,25,25,19,04,00,30,33*f45556a6", "robot status", "#INSPVAXA,USB3,0,46.0,FINESTEERING,2113,382070.950,02000000,471d,15824;INS_SOLUTION_GOOD,INS_RTKFIXED,37.37017963360,126.72086836810,9.9430,22.3000,0.0065,0.0020,0.0003,-0.599902178,-0.377475875,84.822300369,0.0770,0.0547,0.0681,0.0125,0.0125,0.0118,0.0212,0.0213,0.0903,0f000041,0*12bf219e", "robot status", "#DUALANTENNAHEADINGA,USB3,0,46.0,FINESTEERING,2113,382071.000,02000000,d426,15824;SOL_COMPUTED,NARROW_INT,-1.000000000,90.112846375,-13.672393799,0.0,0.472624898,0.864310026,\"681H\",37,25,25,19,04,00,30,33*87417732", "robot status", "#INSPVAXA,USB3,0,45.5,FINESTEERING,2113,382071.100,02000000,471d,15824;INS_SOLUTION_GOOD,INS_RTKFIXED,37.37017964152,126.72086836945,9.9429,22.3000,0.0070,0.0018,0.0007,-0.599937831,-0.377908607,84.821742335,0.0788,0.0582,0.0704,0.0159,0.0158,0.0144,0.0226,0.0227,0.0910,0f000041,0*950fa0ba", "robot status", "#INSPVAXA,USB3,0,45.5,FINESTEERING,2113,382071.150,02000000,471d,15824;INS_SOLUTION_GOOD,INS_RTKFIXED,37.37017964435,126.72086836974,9.9429,22.3000,0.0073,0.0019,0.0004,-0.599327233,-0.378184019,84.822303988,0.0788,0.0582,0.0704,0.0159,0.0158,0.0144,0.0226,0.0227,0.0910,0f000041,0*1238f9ef", "robot status", "#INSPVAXA,USB3,0,45.5,FINESTEERING,2113,382071.150,02000000,471d,15824;INS_SOLUTION_GOOD,INS_RTKFIXED,37.37017964435,126.72086836974,9.9429,22.3000,0.0073,0.0019,0.0004,-0.599327233,-0.378184019,84.822303988,0.0788,0.0582,0.0704,0.0159,0.0158,0.0144,0.0226,0.0227,0.0910,0f000041,0*1238f9ef", "robot status", "#DUALANTENNAHEADINGA,USB3,0,45.5,FINESTEERING,2113,382071.200,02000000,d426,15824;SOL_COMPUTED,NARROW_INT,-1.000000000,90.009086609,-13.449066162,0.0,0.326450258,0.485140413,\"681H\",36,24,24,19,04,00,30,33*a7ddfd04", "robot status", "#INSPVAXA,USB3,0,45.5,FINESTEERING,2113,382071.300,02000000,471d,15824;INS_SOLUTION_GOOD,INS_RTKFIXED,37.37017965344,126.72086837047,9.9427,22.3000,0.0081,0.0018,0.0007,-0.599821045,-0.377811686,84.823044353,0.0788,0.0582,0.0704,0.0159,0.0158,0.0144,0.0226,0.0227,0.0910,0f000041,0*1f2b1343", "robot status", "#INSPVAXA,USB3,0,45.5,FINESTEERING,2113,382071.350,02000000,471d,15824;INS_SOLUTION_GOOD,INS_RTKFIXED,37.37017965674,126.72086837088,9.9427,22.3000,0.0084,0.0021,0.0005,-0.600205314,-0.377729642,84.822485568,0.0788,0.0582,0.0704,0.0159,0.0158,0.0144,0.0226,0.0227,0.0910,0f000041,0*6cf92b78", "robot status", "#INSPVAXA,USB3,0,45.5,FINESTEERING,2113,382071.350,02000000,471d,15824;INS_SOLUTION_GOOD,INS_RTKFIXED,37.37017965674,126.72086837088,9.9427,22.3000,0.0084,0.0021,0.0005,-0.600205314,-0.377729642,84.822485568,0.0788,0.0582,0.0704,0.0159,0.0158,0.0144,0.0226,0.0227,0.0910,0f000041,0*6cf92b78", "robot status", "#DUALANTENNAHEADINGA,USB3,0,45.5,FINESTEERING,2113,382071.400,02000000,d426,15824;SOL_COMPUTED,NARROW_INT,-1.000000000,90.213706970,-13.439331055,0.0,0.324988246,0.483468056,\"681H\",36,23,23,18,04,00,30,33*ba917c21", "robot status", "#INSPVAXA,USB3,0,45.5,FINESTEERING,2113,382071.450,02000000,471d,15824;INS_SOLUTION_GOOD,INS_RTKFIXED,37.37017966379,126.72086837139,9.9426,22.3000,0.0091,0.0017,0.0008,-0.599813341,-0.377644874,84.822946217,0.0788,0.0582,0.0704,0.0159,0.0158,0.0144,0.0226,0.0227,0.0910,0f000041,0*999c8356", "robot status", "#INSPVAXA,USB3,0,45.5,FINESTEERING,2113,382071.550,02000000,471d,15824;INS_SOLUTION_GOOD,INS_RTKFIXED,37.37017967124,126.72086837224,9.9425,22.3000,0.0096,0.0020,0.0006,-0.599758372,-0.377234586,84.822730426,0.0788,0.0582,0.0704,0.0159,0.0158,0.0144,0.0226,0.0227,0.0910,0f000041,0*31b6b5f1", "robot status", "#INSPVAXA,USB3,0,45.5,FINESTEERING,2113,382071.600,02000000,471d,15824;INS_SOLUTION_GOOD,INS_RTKFIXED,37.37017967518,126.72086837263,9.9425,22.3000,0.0099,0.0019,0.0004,-0.599376063,-0.377464662,84.823420222,0.0788,0.0582,0.0704,0.0159,0.0158,0.0144,0.0226,0.0227,0.0910,0f000041,0*e9f0904f", "robot status", "#DUALANTENNAHEADINGA,USB3,0,45.5,FINESTEERING,2113,382071.600,02000000,d426,15824;SOL_COMPUTED,NARROW_INT,-1.000000000,90.154693604,-13.122772217,0.0,0.324348718,0.481329948,\"681H\",36,23,23,18,04,00,30,33*4c293c99", "robot status", "#INSPVAXA,USB3,0,45.5,FINESTEERING,2113,382071.700,02000000,471d,15824;INS_SOLUTION_GOOD,INS_RTKFIXED,37.37017968343,126.72086837314,9.9424,22.3000,0.0104,0.0013,0.0009,-0.600692783,-0.377816994,84.823270415,0.0788,0.0582,0.0704,0.0159,0.0158,0.0144,0.0226,0.0227,0.0910,0f000041,0*87dd07c2", "robot status", "#INSPVAXA,USB3,0,45.5,FINESTEERING,2113,382071.750,02000000,471d,15824;INS_SOLUTION_GOOD,INS_RTKFIXED,37.37017968772,126.72086837330,9.9423,22.3000,0.0105,0.0013,0.0007,-0.600961361,-0.377939738,84.824472402,0.0788,0.0582,0.0704,0.0159,0.0158,0.0144,0.0226,0.0227,0.0910,0f000041,0*a66a3db7", "robot status", "#INSPVAXA,USB3,0,45.5,FINESTEERING,2113,382071.800,02000000,471d,15824;INS_SOLUTION_GOOD,INS_RTKFIXED,37.37017969208,126.72086837329,9.9423,22.3000,0.0106,0.0010,0.0005,-0.600063581,-0.376584546,84.823713021,0.0788,0.0582,0.0704,0.0159,0.0158,0.0144,0.0226,0.0227,0.0910,0f000041,0*6a6d3237", "robot status", "#DUALANTENNAHEADINGA,USB3,0,45.5,FINESTEERING,2113,382071.800,02000000,d426,15824;SOL_COMPUTED,NARROW_INT,-1.000000000,90.093391418,-13.204284668,0.0,0.323663503,0.478906125,\"681H\",36,23,23,18,04,00,30,33*14b19814", "robot status", "#INSPVAXA,USB3,0,45.5,FINESTEERING,2113,382071.850,02000000,471d,15824;INS_SOLUTION_GOOD,INS_RTKFIXED,37.37017969656,126.72086837295,9.9423,22.3000,0.0109,0.0004,0.0009,-0.600806543,-0.377605027,84.824328870,0.0788,0.0582,0.0704,0.0159,0.0158,0.0144,0.0226,0.0227,0.0910,0f000041,0*8696b800", "robot status", "#INSPVAXA,USB3,0,45.5,FINESTEERING,2113,382071.950,02000000,471d,15824;INS_SOLUTION_GOOD,INS_RTKFIXED,37.37017970590,126.72086837163,9.9422,22.3000,0.0116,-0.0004,0.0008,-0.601652865,-0.377021614,84.824653791,0.0788,0.0582,0.0704,0.0159,0.0158,0.0144,0.0226,0.0227,0.0910,0f000041,0*0282df7b", "robot status", "#INSPVAXA,USB3,0,45.5,FINESTEERING,2113,382072.000,02000000,471d,15824;INS_SOLUTION_GOOD,INS_RTKFIXED,37.37017971074,126.72086837081,9.9422,22.3000,0.0117,-0.0003,0.0005,-0.600940865,-0.376307391,84.824785178,0.0788,0.0582,0.0704,0.0159,0.0158,0.0144,0.0226,0.0227,0.0910,0f000041,0*01701666", "robot status", "#INSPVAXA,USB3,0,44.5,FINESTEERING,2113,382072.050,02000000,471d,15824;INS_SOLUTION_GOOD,INS_RTKFIXED,37.37017971543,126.72086836993,9.9422,22.3000,0.0119,-0.0006,0.0010,-0.601019417,-0.376478643,84.824873391,0.0833,0.0647,0.0749,0.0190,0.0188,0.0166,0.0240,0.0240,0.0916,0f000041,0*03c0a478", "robot status", "#INSPVAXA,USB3,0,44.5,FINESTEERING,2113,382072.100,02000000,471d,15824;INS_SOLUTION_GOOD,INS_RTKFIXED,37.37017971986,126.72086836917,9.9422,22.3000,0.0119,-0.0009,0.0012,-0.601332172,-0.376678627,84.825973035,0.0833,0.0647,0.0749,0.0190,0.0188,0.0166,0.0240,0.0240,0.0916,0f000041,0*c60bcc98", "robot status", "#INSPVAXA,USB3,0,44.5,FINESTEERING,2113,382072.150,02000000,471d,15824;INS_SOLUTION_GOOD,INS_RTKFIXED,37.37017972451,126.72086836840,9.9422,22.3000,0.0123,-0.0010,0.0011,-0.601465369,-0.376853822,84.826376255,0.0833,0.0647,0.0749,0.0190,0.0188,0.0166,0.0240,0.0240,0.0916,0f000041,0*f1d5f017", "robot status", "#INSPVAXA,USB3,0,44.5,FINESTEERING,2113,382072.200,02000000,471d,15824;INS_SOLUTION_GOOD,INS_RTKFIXED,37.37017972927,126.72086836764,9.9423,22.3000,0.0124,-0.0007,0.0008,-0.601519072,-0.377778658,84.826657447,0.0833,0.0647,0.0749,0.0190,0.0188,0.0166,0.0240,0.0240,0.0916,0f000041,0*08f526c0", "robot status", "#INSPVAXA,USB3,0,44.5,FINESTEERING,2113,382072.250,02000000,471d,15824;INS_SOLUTION_GOOD,INS_RTKFIXED,37.37017973415,126.72086836681,9.9423,22.3000,0.0128,-0.0009,0.0009,-0.601475670,-0.377854853,84.826037868,0.0833,0.0647,0.0749,0.0190,0.0188,0.0166,0.0240,0.0240,0.0916,0f000041,0*9ff6539e", "robot status", "#INSPVAXA,USB3,0,44.5,FINESTEERING,2113,382072.250,02000000,471d,15824;INS_SOLUTION_GOOD,INS_RTKFIXED,37.37017973415,126.72086836681,9.9423,22.3000,0.0128,-0.0009,0.0009,-0.601475670,-0.377854853,84.826037868,0.0833,0.0647,0.0749,0.0190,0.0188,0.0166,0.0240,0.0240,0.0916,0f000041,0*9ff6539e", "robot status", "#INSPVAXA,USB3,0,44.5,FINESTEERING,2113,382072.350,02000000,471d,15824;INS_SOLUTION_GOOD,INS_RTKFIXED,37.37017974429,126.72086836467,9.9424,22.3000,0.0134,-0.0017,0.0010,-0.600482803,-0.378032131,84.825693521,0.0833,0.0647,0.0749,0.0190,0.0188,0.0166,0.0240,0.0240,0.0916,0f000041,0*eb5aeede", "robot status", "#INSPVAXA,USB3,0,44.5,FINESTEERING,2113,382072.400,02000000,471d,15824;INS_SOLUTION_GOOD,INS_RTKFIXED,37.37017974953,126.72086836352,9.9424,22.3000,0.0132,-0.0015,0.0007,-0.599581536,-0.377811464,84.825890020,0.0833,0.0647,0.0749,0.0190,0.0188,0.0166,0.0240,0.0240,0.0916,0f000041,0*786f4532", "robot status", "#INSPVAXA,USB3,0,44.5,FINESTEERING,2113,382072.450,02000000,471d,15824;INS_SOLUTION_GOOD,INS_RTKFIXED,37.37017975477,126.72086836222,9.9424,22.3000,0.0137,-0.0016,0.0008,-0.600103539,-0.377967488,84.825429010,0.0833,0.0647,0.0749,0.0190,0.0188,0.0166,0.0240,0.0240,0.0916,0f000041,0*7a8f802b", "robot status", "#INSPVAXA,USB3,0,44.5,FINESTEERING,2113,382072.450,02000000,471d,15824;INS_SOLUTION_GOOD,INS_RTKFIXED,37.37017975477,126.72086836222,9.9424,22.3000,0.0137,-0.0016,0.0008,-0.600103539,-0.377967488,84.825429010,0.0833,0.0647,0.0749,0.0190,0.0188,0.0166,0.0240,0.0240,0.0916,0f000041,0*7a8f802b", "robot status", "#INSPVAXA,USB3,0,44.5,FINESTEERING,2113,382072.550,02000000,471d,15824;INS_SOLUTION_GOOD,INS_RTKFIXED,37.37017976569,126.72086835966,9.9425,22.3000,0.0140,-0.0020,0.0012,-0.600893384,-0.378412181,84.826402664,0.0833,0.0647,0.0749,0.0190,0.0188,0.0166,0.0240,0.0240,0.0916,0f000041,0*9bd92c16", "robot status", "#INSPVAXA,USB3,0,44.5,FINESTEERING,2113,382072.600,02000000,471d,15824;INS_SOLUTION_GOOD,INS_RTKFIXED,37.37017977124,126.72086835847,9.9425,22.3000,0.0142,-0.0016,0.0010,-0.600423370,-0.376822185,84.826249619,0.0833,0.0647,0.0749,0.0190,0.0188,0.0166,0.0240,0.0240,0.0916,0f000041,0*3c7c9677", "robot status", "#INSPVAXA,USB3,0,44.5,FINESTEERING,2113,382072.650,02000000,471d,15824;INS_SOLUTION_GOOD,INS_RTKFIXED,37.37017977677,126.72086835714,9.9426,22.3000,0.0145,-0.0018,0.0010,-0.601093520,-0.377339744,84.826092502,0.0833,0.0647,0.0749,0.0190,0.0188,0.0166,0.0240,0.0240,0.0916,0f000041,0*fbe3393e", "robot status", "#DUALANTENNAHEADINGA,USB3,0,44.5,FINESTEERING,2113,382072.700,02000000,d426,15824;SOL_COMPUTED,NARROW_INT,-1.000000000,89.975273132,-13.948364258,0.0,0.481979400,0.867224634,\"681H\",35,23,23,19,04,00,30,33*f997b352", "robot status", "#INSPVAXA,USB3,0,44.5,FINESTEERING,2113,382072.750,02000000,471d,15824;INS_SOLUTION_GOOD,INS_RTKFIXED,37.37017978839,126.72086835452,9.9426,22.3000,0.0149,-0.0021,0.0012,-0.601399663,-0.376752375,84.827544932,0.0833,0.0647,0.0749,0.0190,0.0188,0.0166,0.0240,0.0240,0.0916,0f000041,0*3d31e06d", "robot status", "#INSPVAXA,USB3,0,44.5,FINESTEERING,2113,382072.800,02000000,471d,15824;INS_SOLUTION_GOOD,INS_RTKFIXED,37.37017979429,126.72086835334,9.9427,22.3000,0.0147,-0.0016,0.0008,-0.601268076,-0.376299547,84.828005025,0.0833,0.0647,0.0749,0.0190,0.0188,0.0166,0.0240,0.0240,0.0916,0f000041,0*7b0e1304", "robot status", "#INSPVAXA,USB3,0,44.5,FINESTEERING,2113,382072.850,02000000,471d,15824;INS_SOLUTION_GOOD,INS_RTKFIXED,37.37017980033,126.72086835205,9.9427,22.3000,0.0153,-0.0017,0.0005,-0.601132622,-0.377409872,84.827951729,0.0833,0.0647,0.0749,0.0190,0.0188,0.0166,0.0240,0.0240,0.0916,0f000041,0*43fcba7f", "robot status", "#INSPVAXA,USB3,0,44.5,FINESTEERING,2113,382072.900,02000000,471d,15824;INS_SOLUTION_GOOD,INS_RTKFIXED,37.37017980641,126.72086835074,9.9427,22.3000,0.0155,-0.0018,0.0008,-0.600826968,-0.377590309,84.828393900,0.0833,0.0647,0.0749,0.0190,0.0188,0.0166,0.0240,0.0240,0.0916,0f000041,0*c1950432", "robot status", "#INSPVAXA,USB3,0,44.5,FINESTEERING,2113,382072.950,02000000,471d,15824;INS_SOLUTION_GOOD,INS_RTKFIXED,37.37017981271,126.72086834953,9.9427,22.3000,0.0158,-0.0019,0.0010,-0.601456711,-0.378062994,84.827443183,0.0833,0.0647,0.0749,0.0190,0.0188,0.0166,0.0240,0.0240,0.0916,0f000041,0*7eb37011", "robot status", "#INSPVAXA,USB3,0,44.5,FINESTEERING,2113,382073.000,02000000,471d,15824;INS_SOLUTION_GOOD,INS_RTKFIXED,37.37017981907,126.72086834832,9.9428,22.3000,0.0157,-0.0018,0.0009,-0.601524700,-0.377645550,84.827940345,0.0833,0.0647,0.0749,0.0190,0.0188,0.0166,0.0240,0.0240,0.0916,0f000041,0*09fb9f6e", "robot status", "#INSPVAXA,USB3,0,44.5,FINESTEERING,2113,382073.050,02008000,471d,15824;INS_SOLUTION_GOOD,INS_RTKFIXED,37.37017982519,126.72086834667,9.9428,22.3000,0.0158,-0.0017,0.0009,-0.600941136,-0.378310594,84.827916904,0.0905,0.0735,0.0815,0.0219,0.0215,0.0184,0.0252,0.0252,0.0922,0f000041,0*a776cc5b", "robot status", "#INSPVAXA,USB3,0,46.5,FINESTEERING,2113,382073.100,02008000,471d,15824;INS_SOLUTION_GOOD,INS_RTKFIXED,37.37017983097,126.72086834460,9.9428,22.3000,0.0159,-0.0021,0.0012,-0.601409588,-0.378404215,84.827698413,0.0905,0.0735,0.0815,0.0219,0.0215,0.0184,0.0252,0.0252,0.0922,0f000041,0*461a525c", "robot status", "#INSPVAXA,USB3,0,46.5,FINESTEERING,2113,382073.150,02008000,471d,15824;INS_SOLUTION_GOOD,INS_RTKFIXED,37.37017983701,126.72086834253,9.9428,22.3000,0.0162,-0.0026,0.0012,-0.601216017,-0.378191620,84.828256813,0.0905,0.0735,0.0815,0.0219,0.0215,0.0184,0.0252,0.0252,0.0922,0f000041,0*50820eda", "robot status", "#INSPVAXA,USB3,0,46.5,FINESTEERING,2113,382073.200,02008000,471d,15824;INS_SOLUTION_GOOD,INS_RTKFIXED,37.37017984310,126.72086834041,9.9428,22.3000,0.0161,-0.0024,0.0010,-0.600990118,-0.378155990,84.828243106,0.0905,0.0735,0.0815,0.0219,0.0215,0.0184,0.0252,0.0252,0.0922,0f000041,0*fbb9e56a", "robot status", "#INSPVAXA,USB3,0,46.5,FINESTEERING,2113,382073.250,02008000,471d,15824;INS_SOLUTION_GOOD,INS_RTKFIXED,37.37017984912,126.72086833549,9.9428,22.3000,0.0150,-0.0156,0.0024,-0.597995653,-0.404271858,84.803240511,0.0905,0.0735,0.0815,0.0219,0.0215,0.0184,0.0252,0.0252,0.0922,0f000041,0*7704b871", "robot status", "#INSPVAXA,USB3,0,46.5,FINESTEERING,2113,382073.300,02008000,471d,15824;INS_SOLUTION_GOOD,INS_RTKFIXED,37.37017985430,126.72086831287,9.9429,22.3000,0.0124,-0.0534,-0.0000,-0.574113136,-0.439276111,84.605615695,0.0905,0.0735,0.0815,0.0219,0.0215,0.0184,0.0252,0.0252,0.0922,0f000041,0*a0860f7d", "robot status", "#INSPVAXA,USB3,0,46.5,FINESTEERING,2113,382073.350,02008000,471d,15824;INS_SOLUTION_GOOD,INS_RTKFIXED,37.37017985732,126.72086828103,9.9428,22.3000,0.0056,-0.0557,0.0007,-0.531266257,-0.376325193,84.115137436,0.0905,0.0735,0.0815,0.0219,0.0215,0.0184,0.0252,0.0252,0.0922,0f000041,0*c308584a", "robot status", "#INSPVAXA,USB3,0,46.5,FINESTEERING,2113,382073.400,02008000,471d,15824;INS_SOLUTION_GOOD,INS_RTKFIXED,37.37017985750,126.72086825047,9.9428,22.3000,0.0033,-0.0500,-0.0001,-0.499758909,-0.391516197,83.654091933,0.0905,0.0735,0.0815,0.0219,0.0215,0.0184,0.0252,0.0252,0.0922,0f000041,0*d8f92733", "robot status", "#INSPVAXA,USB3,0,46.5,FINESTEERING,2113,382073.450,02008000,471d,15824;INS_SOLUTION_GOOD,INS_RTKFIXED,37.37017985919,126.72086822634,9.9429,22.3000,0.0090,-0.0358,0.0079,-0.477981026,-0.383111575,83.305488484,0.0905,0.0735,0.0815,0.0219,0.0215,0.0184,0.0252,0.0252,0.0922,0f000041,0*83609da6", "robot status", "#INSPVAXA,USB3,0,46.5,FINESTEERING,2113,382073.500,02008000,471d,15824;INS_SOLUTION_GOOD,INS_RTKFIXED,37.37017986054,126.72086820985,9.9432,22.3000,-0.0004,-0.0189,0.0092,-0.504412095,-0.416138278,82.501100512,0.0905,0.0735,0.0815,0.0219,0.0215,0.0184,0.0252,0.0252,0.0922,0f000041,0*6a191126", "robot status", "#INSPVAXA,USB3,0,46.5,FINESTEERING,2113,382073.550,02008000,471d,15824;INS_SOLUTION_GOOD,INS_RTKFIXED,37.37017985663,126.72086819980,9.9435,22.3000,-0.0096,-0.0129,0.0017,-0.552263944,-0.354856746,81.230931103,0.0905,0.0735,0.0815,0.0219,0.0215,0.0184,0.0252,0.0252,0.0922,0f000041,0*52cc3930", "robot status", "#INSPVAXA,USB3,0,46.5,FINESTEERING,2113,382073.600,02008000,471d,15824;INS_SOLUTION_GOOD,INS_RTKFIXED,37.37017985847,126.72086819786,9.9432,22.3000,0.0216,0.0110,-0.0108,-0.326101461,-0.414850627,79.777704809,0.0905,0.0735,0.0815,0.0219,0.0215,0.0184,0.0252,0.0252,0.0922,0f000041,0*8cc06660", "robot status", "#INSPVAXA,USB3,0,46.5,FINESTEERING,2113,382073.650,02008000,471d,15824;INS_SOLUTION_GOOD,INS_RTKFIXED,37.37017986325,126.72086820349,9.9430,22.3000,-0.0054,0.0099,0.0011,-0.489440255,-0.463213005,78.348364299,0.0905,0.0735,0.0815,0.0219,0.0215,0.0184,0.0252,0.0252,0.0922,0f000041,0*28b3adb3", "robot status", "#INSPVAXA,USB3,0,46.5,FINESTEERING,2113,382073.700,02008000,471d,15824;INS_SOLUTION_GOOD,INS_RTKFIXED,37.37017985481,126.72086820984,9.9432,22.3000,-0.0202,0.0211,-0.0028,-0.300682735,-0.484644921,77.139613993,0.0905,0.0735,0.0815,0.0219,0.0215,0.0184,0.0252,0.0252,0.0922,0f000041,0*e864d66f", "robot status", "#INSPVAXA,USB3,0,46.5,FINESTEERING,2113,382073.750,02008000,471d,15824;INS_SOLUTION_GOOD,INS_RTKFIXED,37.37017985371,126.72086822476,9.9429,22.3000,0.0207,0.0316,0.0002,-0.315083233,-0.469559740,75.928624821,0.0905,0.0735,0.0815,0.0219,0.0215,0.0184,0.0252,0.0252,0.0922,0f000041,0*1be82db3", "robot status", "#INSPVAXA,USB3,0,46.5,FINESTEERING,2113,382073.800,02008000,471d,15824;INS_SOLUTION_GOOD,INS_RTKFIXED,37.37017985981,126.72086824005,9.9431,22.3000,0.0009,0.0256,0.0043,-0.396936839,-0.541302612,74.927238131,0.0905,0.0735,0.0815,0.0219,0.0215,0.0184,0.0252,0.0252,0.0922,0f000041,0*5a89a369", "robot status", "#INSPVAXA,USB3,0,46.5,FINESTEERING,2113,382073.850,02008000,471d,15824;INS_SOLUTION_GOOD,INS_RTKFIXED,37.37017985062,126.72086825315,9.9428,22.3000,-0.0272,0.0277,-0.0063,-0.282923448,-0.471363391,74.013956210,0.0905,0.0735,0.0815,0.0219,0.0215,0.0184,0.0252,0.0252,0.0922,0f000041,0*4027b572", "robot status", "#DUALANTENNAHEADINGA,USB3,0,46.5,FINESTEERING,2113,382073.900,02008000,d426,15824;SOL_COMPUTED,NARROW_INT,-1.000000000,78.651481628,-12.052124023,0.0,0.509071231,0.873149753,\"681H\",36,23,23,19,04,00,30,33*0d0a6589", "robot status", "#INSPVAXA,USB3,0,46.5,FINESTEERING,2113,382073.950,02008000,471d,15824;INS_SOLUTION_GOOD,INS_RTKFIXED,37.37017989649,126.72086831776,9.9426,22.3000,0.1072,0.0871,-0.0078,-0.217773206,-0.477172654,72.942590895,0.0905,0.0735,0.0815,0.0219,0.0215,0.0184,0.0252,0.0252,0.0922,0f000041,0*18189655", "robot status", "#DUALANTENNAHEADINGA,USB3,0,46.5,FINESTEERING,2113,382074.000,02008000,d426,15824;SOL_COMPUTED,NARROW_INT,-1.000000000,78.022827148,-12.189239502,0.0,0.511835754,0.878186822,\"681H\",35,22,22,18,04,00,30,33*80866a32", "robot status", "#INSPVAXA,USB3,0,46.5,FINESTEERING,2113,382074.050,02008000,471d,15824;INS_SOLUTION_GOOD,INS_RTKFIXED,37.37017996612,126.72086846792,9.9427,22.3000,0.0731,0.1918,-0.0122,-0.319955121,-0.338009754,72.678219722,0.0990,0.0834,0.0881,0.0245,0.0239,0.0196,0.0262,0.0263,0.0927,0f000041,0*32726947", "robot status", "#INSPVAXA,USB3,0,46.5,FINESTEERING,2113,382074.100,02008000,471d,15824;INS_SOLUTION_GOOD,INS_RTKFIXED,37.37018000250,126.72086859216,9.9424,22.3000,0.1026,0.2532,-0.0002,-0.271388405,-0.269199630,72.566759689,0.0990,0.0834,0.0881,0.0245,0.0239,0.0196,0.0262,0.0263,0.0927,0f000041,0*07177ded", "robot status", "#INSPVAXA,USB3,0,46.5,FINESTEERING,2113,382074.150,02008000,471d,15824;INS_SOLUTION_GOOD,INS_RTKFIXED,37.37018005037,126.72086875607,9.9424,22.3000,0.1279,0.3339,-0.0029,-0.282952207,-0.151965015,72.525987216,0.0990,0.0834,0.0881,0.0245,0.0239,0.0196,0.0262,0.0263,0.0927,0f000041,0*a11ee4aa", "robot status", "#DUALANTENNAHEADINGA,USB3,0,46.5,FINESTEERING,2113,382074.200,02008000,d426,15824;SOL_COMPUTED,NARROW_INT,-1.000000000,78.011558533,-11.055664063,0.0,0.509357631,0.882816851,\"681H\",36,24,24,19,04,00,30,33*07dc8a92", "robot status", "#INSPVAXA,USB3,0,46.5,FINESTEERING,2113,382074.250,02008000,471d,15824;INS_SOLUTION_GOOD,INS_RTKFIXED,37.37018017202,126.72086918154,9.9420,22.3000,0.1624,0.4170,0.0143,-0.209669700,-0.153797942,72.309538846,0.0990,0.0834,0.0881,0.0245,0.0239,0.0196,0.0262,0.0263,0.0927,0f000041,0*ded3edc9", "robot status", "#DUALANTENNAHEADINGA,USB3,0,46.5,FINESTEERING,2113,382074.300,02008000,d426,15824;SOL_COMPUTED,NARROW_INT,-1.000000000,77.479995728,-12.038085938,0.0,0.508858621,0.874182045,\"681H\",37,24,24,19,04,00,30,33*ce880b09", "robot status", "#INSPVAXA,USB3,0,46.5,FINESTEERING,2113,382074.350,02008000,471d,15824;INS_SOLUTION_GOOD,INS_RTKFIXED,37.37018030286,126.72086964440,9.9406,22.3000,0.1228,0.3796,-0.0010,-0.217043144,-0.338500013,71.668382831,0.0990,0.0834,0.0881,0.0245,0.0239,0.0196,0.0262,0.0263,0.0927,0f000041,0*7e2a731e", "robot status", "#DUALANTENNAHEADINGA,USB3,0,46.5,FINESTEERING,2113,382074.400,02008000,d426,15824;SOL_COMPUTED,NARROW_INT,-1.000000000,76.580001831,-11.882720947,0.0,0.515698373,0.884670496,\"681H\",37,24,24,19,04,00,30,33*32836438", "robot status", "#INSPVAXA,USB3,0,46.5,FINESTEERING,2113,382074.450,02008000,471d,15824;INS_SOLUTION_GOOD,INS_RTKFIXED,37.37018036952,126.72086999188,9.9410,22.3000,0.0446,0.2362,-0.0352,-0.354483640,-0.351873472,70.390742960,0.0990,0.0834,0.0881,0.0245,0.0239,0.0196,0.0262,0.0263,0.0927,0f000041,0*6be97706", "robot status", "#INSPVAXA,USB3,0,46.5,FINESTEERING,2113,382074.500,02008000,471d,15824;INS_SOLUTION_GOOD,INS_RTKFIXED,37.37018038718,126.72087010403,9.9407,22.3000,0.0438,0.1706,0.0083,-0.229295548,-0.346317564,69.474232041,0.0990,0.0834,0.0881,0.0245,0.0239,0.0196,0.0262,0.0263,0.0927,0f000041,0*b2894c28", "robot status", "#INSPVAXA,USB3,0,46.5,FINESTEERING,2113,382074.550,02008000,471d,15824;INS_SOLUTION_GOOD,INS_RTKFIXED,37.37018040626,126.72087018266,9.9407,22.3000,0.0536,0.1150,-0.0069,-0.183680761,-0.397737056,68.723280204,0.0990,0.0834,0.0881,0.0245,0.0239,0.0196,0.0262,0.0263,0.0927,0f000041,0*1e421d1b", "robot status", "#DUALANTENNAHEADINGA,USB3,0,46.5,FINESTEERING,2113,382074.600,02008000,d426,15824;SOL_COMPUTED,NARROW_INT,-1.000000000,73.438514709,-11.795562744,0.0,0.529014885,0.898859024,\"681H\",34,24,24,19,04,00,30,33*d140b573", "robot status", "#INSPVAXA,USB3,0,46.5,FINESTEERING,2113,382074.650,02008000,471d,15824;INS_SOLUTION_GOOD,INS_RTKFIXED,37.37018043528,126.72087026367,9.9410,22.3000,0.0260,0.0318,0.0004,-0.173594475,-0.393629965,66.934229523,0.0990,0.0834,0.0881,0.0245,0.0239,0.0196,0.0262,0.0263,0.0927,0f000041,0*3d06f000", "robot status", "#DUALANTENNAHEADINGA,USB3,0,46.5,FINESTEERING,2113,382074.700,02008000,d426,15824;SOL_COMPUTED,NARROW_INT,-1.000000000,71.638641357,-12.334777832,0.0,0.529923081,0.890470386,\"681H\",34,24,24,18,04,00,30,33*91bc0a85", "robot status", "#INSPVAXA,USB3,0,46.5,FINESTEERING,2113,382074.750,02008000,471d,15824;INS_SOLUTION_GOOD,INS_RTKFIXED,37.37018047770,126.72087026598,9.9412,22.3000,0.0546,-0.0228,0.0050,-0.201971885,-0.437046725,64.945993388,0.0990,0.0834,0.0881,0.0245,0.0239,0.0196,0.0262,0.0263,0.0927,0f000041,0*30d6f8e5", "robot status", "#DUALANTENNAHEADINGA,USB3,0,46.5,FINESTEERING,2113,382074.800,02008000,d426,15824;SOL_COMPUTED,NARROW_INT,-1.000000000,69.411788940,-12.675720215,0.0,0.531659663,0.886485517,\"681H\",32,23,23,17,04,00,30,33*1331230f", "robot status", "#INSPVAXA,USB3,0,46.5,FINESTEERING,2113,382074.850,02008000,471d,15824;INS_SOLUTION_GOOD,INS_RTKFIXED,37.37018048268,126.72087021848,9.9413,22.3000,0.0047,-0.0489,0.0103,-0.043579673,-0.400753028,62.965735239,0.0990,0.0834,0.0881,0.0245,0.0239,0.0196,0.0262,0.0263,0.0927,0f000041,0*a7fbe48a", "robot status", "#DUALANTENNAHEADINGA,USB3,0,46.5,FINESTEERING,2113,382074.900,02008000,d426,15824;SOL_COMPUTED,NARROW_INT,-1.000000000,67.294761658,-13.091033936,0.0,0.536597013,0.883473516,\"681H\",34,23,23,17,04,00,30,33*ec12414b", "robot status", "#INSPVAXA,USB3,0,46.5,FINESTEERING,2113,382074.950,02008000,471d,15824;INS_SOLUTION_GOOD,INS_RTKFIXED,37.37018053084,126.72087016749,9.9415,22.3000,0.0719,-0.0353,-0.0107,-0.235179959,-0.475335780,60.798262010,0.0990,0.0834,0.0881,0.0245,0.0239,0.0196,0.0262,0.0263,0.0927,0f000041,0*91dc11cc", "robot status", "#DUALANTENNAHEADINGA,USB3,0,46.5,FINESTEERING,2113,382075.000,02008000,d426,15824;SOL_COMPUTED,NARROW_INT,-1.000000000,64.811676025,-13.705932617,0.0,0.541863739,0.882216036,\"681H\",33,23,23,17,04,00,30,33*f088b7a2", "robot status", "#INSPVAXA,USB3,0,45.0,FINESTEERING,2113,382075.050,02008000,471d,15824;INS_SOLUTION_GOOD,INS_RTKFIXED,37.37018056441,126.72087016362,9.9415,22.3000,0.0714,0.0363,-0.0047,0.007427792,-0.391928341,59.023828348,0.1057,0.0906,0.0916,0.0264,0.0254,0.0201,0.0271,0.0272,0.0935,0f000041,0*57834955", "robot status", "#DUALANTENNAHEADINGA,USB3,0,45.0,FINESTEERING,2113,382075.100,02008000,d426,15824;SOL_COMPUTED,NARROW_INT,-1.000000000,63.604549408,-12.995452881,0.0,0.544039726,0.889402032,\"681H\",33,23,23,17,04,00,30,33*5d7a1de6", "robot status", "#INSPVAXA,USB3,0,45.0,FINESTEERING,2113,382075.150,02008000,471d,15824;INS_SOLUTION_GOOD,INS_RTKFIXED,37.37018064504,126.72087024340,9.9421,22.3000,0.1291,0.1299,0.0021,-0.155678674,-0.369785023,58.356103478,0.1057,0.0906,0.0916,0.0264,0.0254,0.0201,0.0271,0.0272,0.0935,0f000041,0*ccc1e980", "robot status", "#DUALANTENNAHEADINGA,USB3,0,45.0,FINESTEERING,2113,382075.200,02008000,d426,15824;SOL_COMPUTED,NARROW_INT,-1.000000000,63.339069366,-14.000732422,0.0,0.545248568,0.878647864,\"681H\",34,24,24,17,04,00,30,33*fd9571e5", "robot status", "#INSPVAXA,USB3,0,45.0,FINESTEERING,2113,382075.250,02008000,471d,15824;INS_SOLUTION_GOOD,INS_RTKFIXED,37.37018077401,126.72087044015,9.9424,22.3000,0.1930,0.2525,0.0030,-0.199447241,-0.381265553,57.977175984,0.1057,0.0906,0.0916,0.0264,0.0254,0.0201,0.0271,0.0272,0.0935,0f000041,0*1a1b3fe4", "robot status", "#DUALANTENNAHEADINGA,USB3,0,45.0,FINESTEERING,2113,382075.300,02008000,d426,15824;SOL_COMPUTED,NARROW_INT,-1.000000000,63.204113007,-13.782287598,0.0,0.539072216,0.873227894,\"681H\",33,24,24,17,04,00,30,33*e5b0cbed", "robot status", "#INSPVAXA,USB3,0,45.0,FINESTEERING,2113,382075.350,02008000,471d,15824;INS_SOLUTION_GOOD,INS_RTKFIXED,37.37018095215,126.72087078322,9.9421,22.3000,0.2492,0.3667,-0.0135,-0.141741377,-0.276070815,57.886013358,0.1057,0.0906,0.0916,0.0264,0.0254,0.0201,0.0271,0.0272,0.0935,0f000041,0*763b3e5a", "robot status", "#DUALANTENNAHEADINGA,USB3,0,45.0,FINESTEERING,2113,382075.400,02008000,d426,15824;SOL_COMPUTED,NARROW_INT,-1.000000000,63.048889160,-13.575622559,0.0,0.540124536,0.879550219,\"681H\",33,24,24,17,04,00,30,33*536f0fdf", "robot status", "#INSPVAXA,USB3,0,45.0,FINESTEERING,2113,382075.450,02008000,471d,15824;INS_SOLUTION_GOOD,INS_RTKFIXED,37.37018119176,126.72087121527,9.9427,22.3000,0.3075,0.4214,-0.0122,-0.182196828,-0.471949325,57.577379022,0.1057,0.0906,0.0916,0.0264,0.0254,0.0201,0.0271,0.0272,0.0935,0f000041,0*81ccb12d", "robot status", "#DUALANTENNAHEADINGA,USB3,0,45.0,FINESTEERING,2113,382075.500,02008000,d426,15824;SOL_COMPUTED,NARROW_INT,-1.000000000,63.073009491,-12.718078613,0.0,0.541109324,0.891174018,\"681H\",34,23,23,17,04,00,30,33*7002238b", "robot status", "#INSPVAXA,USB3,0,45.0,FINESTEERING,2113,382075.550,02008000,471d,15824;INS_SOLUTION_GOOD,INS_RTKFIXED,37.37018146664,126.72087169708,9.9427,22.3000,0.3456,0.4702,-0.0219,-0.333967549,-0.384103926,57.389891741,0.1057,0.0906,0.0916,0.0264,0.0254,0.0201,0.0271,0.0272,0.0935,0f000041,0*268896aa", "robot status", "#DUALANTENNAHEADINGA,USB3,0,45.0,FINESTEERING,2113,382075.600,02008000,d426,15824;SOL_COMPUTED,NARROW_INT,-1.000000000,63.127716064,-12.739074707,0.0,0.540316105,0.889290690,\"681H\",34,23,23,17,04,00,30,33*c2bfe3af", "robot status", "#INSPVAXA,USB3,0,45.0,FINESTEERING,2113,382075.650,02008000,471d,15824;INS_SOLUTION_GOOD,INS_RTKFIXED,37.37018176750,126.72087225123,9.9428,22.3000,0.3931,0.5281,0.0002,-0.440905585,-0.399206061,57.195037419,0.1057,0.0906,0.0916,0.0264,0.0254,0.0201,0.0271,0.0272,0.0935,0f000041,0*ac343d6c", "robot status", "#DUALANTENNAHEADINGA,USB3,0,45.0,FINESTEERING,2113,382075.700,02008000,d426,15824;SOL_COMPUTED,NARROW_INT,-1.000000000,62.709659576,-12.680664063,0.0,0.537887096,0.884669185,\"681H\",34,23,23,17,04,00,30,33*a5a5b52a", "robot status", "#INSPVAXA,USB3,0,45.0,FINESTEERING,2113,382075.750,02008000,471d,15824;INS_SOLUTION_GOOD,INS_RTKFIXED,37.37018211327,126.72087284902,9.9436,22.3000,0.3928,0.5151,0.0173,-0.701722471,-0.720401751,57.040958335,0.1057,0.0906,0.0916,0.0264,0.0254,0.0201,0.0271,0.0272,0.0935,0f000041,0*75fc3156", "robot status", "#DUALANTENNAHEADINGA,USB3,0,45.0,FINESTEERING,2113,382075.800,02008000,d426,15824;SOL_COMPUTED,NARROW_INT,-1.000000000,62.346096039,-13.883911133,0.0,0.543809891,0.884740591,\"681H\",34,23,23,17,04,00,30,33*eb2d5d2f", "robot status", "#INSPVAXA,USB3,0,45.0,FINESTEERING,2113,382075.850,02008000,471d,15824;INS_SOLUTION_GOOD,INS_RTKFIXED,37.37018236085,126.72087331544,9.9435,22.3000,0.2126,0.3217,-0.0253,-0.616537830,-1.091030831,56.873048199,0.1057,0.0906,0.0916,0.0264,0.0254,0.0201,0.0271,0.0272,0.0935,0f000041,0*54b52a4a", "robot status", "#DUALANTENNAHEADINGA,USB3,0,45.0,FINESTEERING,2113,382075.900,02008000,d426,15824;SOL_COMPUTED,NARROW_INT,-1.000000000,62.310142517,-14.039154053,0.0,0.547599375,0.896733701,\"681H\",34,23,23,17,04,00,30,33*74f7288d", "robot status", "#INSPVAXA,USB3,0,45.0,FINESTEERING,2113,382075.950,02008000,471d,15824;INS_SOLUTION_GOOD,INS_RTKFIXED,37.37018248700,126.72087353594,9.9439,22.3000,0.1137,0.1048,-0.0036,-0.495101407,-1.045343873,56.585953321,0.1057,0.0906,0.0916,0.0264,0.0254,0.0201,0.0271,0.0272,0.0935,0f000041,0*0c4a0f1e", "robot status", "#DUALANTENNAHEADINGA,USB3,0,45.0,FINESTEERING,2113,382076.000,02008000,d426,15824;SOL_COMPUTED,NARROW_INT,-1.000000000,61.921573639,-13.914062500,0.0,0.557226360,0.902951717,\"681H\",34,23,23,17,04,00,30,33*6a0f317a", "robot status", "#INSPVAXA,USB3,0,45.0,FINESTEERING,2113,382076.050,02008000,471d,15824;INS_SOLUTION_GOOD,INS_RTKFIXED,37.37018253368,126.72087360381,9.9438,22.3000,0.0455,0.0427,-0.0018,-0.517898315,-0.949012831,56.811620679,0.1137,0.1003,0.0968,0.0282,0.0271,0.0207,0.0279,0.0280,0.0940,0f000041,0*fb78a047", "robot status", "#DUALANTENNAHEADINGA,USB3,0,45.0,FINESTEERING,2113,382076.100,02008000,d426,15824;SOL_COMPUTED,NARROW_INT,-1.000000000,62.073051453,-13.937500000,0.0,0.558652580,0.911445558,\"681H\",35,23,23,17,04,00,30,33*0b472d2b", "robot status", "#INSPVAXA,USB3,0,45.5,FINESTEERING,2113,382076.150,02008000,471d,15824;INS_SOLUTION_GOOD,INS_RTKFIXED,37.37018255048,126.72087362761,9.9435,22.3000,0.0469,0.0192,-0.0021,-0.491401697,-0.869285185,56.693003399,0.1137,0.1003,0.0968,0.0282,0.0271,0.0207,0.0279,0.0280,0.0940,0f000041,0*a175cc42", "robot status", "#DUALANTENNAHEADINGA,USB3,0,45.5,FINESTEERING,2113,382076.200,02008000,d426,15824;SOL_COMPUTED,NARROW_INT,-1.000000000,62.038036346,-14.132171631,0.0,0.551886797,0.902549088,\"681H\",35,23,23,17,04,00,30,33*d42e1f1f", "robot status", "#INSPVAXA,USB3,0,45.5,FINESTEERING,2113,382076.250,02008000,471d,15824;INS_SOLUTION_GOOD,INS_RTKFIXED,37.37018255017,126.72087362240,9.9433,22.3000,0.0212,-0.0212,-0.0029,-0.486715850,-0.862278573,57.053295752,0.1137,0.1003,0.0968,0.0282,0.0271,0.0207,0.0279,0.0280,0.0940,0f000041,0*3c9cc9b8", "robot status", "#DUALANTENNAHEADINGA,USB3,0,45.5,FINESTEERING,2113,382076.300,02008000,d426,15824;SOL_COMPUTED,NARROW_INT,-1.000000000,62.585472107,-14.265991211,0.0,0.549001098,0.899196625,\"681H\",35,23,23,17,04,00,30,33*cf1c8a00", "robot status", "#INSPVAXA,USB3,0,45.5,FINESTEERING,2113,382076.350,02008000,471d,15824;INS_SOLUTION_GOOD,INS_RTKFIXED,37.37018253867,126.72087358288,9.9431,22.3000,0.0073,-0.0287,-0.0037,-0.514540453,-0.845255014,56.930703050,0.1137,0.1003,0.0968,0.0282,0.0271,0.0207,0.0279,0.0280,0.0940,0f000041,0*092512fc", "robot status", "#DUALANTENNAHEADINGA,USB3,0,45.5,FINESTEERING,2113,382076.400,02008000,d426,15824;SOL_COMPUTED,NARROW_INT,-1.000000000,62.472717285,-13.483306885,0.0,0.546154857,0.904208302,\"681H\",35,23,23,17,04,00,30,33*fc042c88", "robot status", "#INSPVAXA,USB3,0,45.5,FINESTEERING,2113,382076.450,02008000,471d,15824;INS_SOLUTION_GOOD,INS_RTKFIXED,37.37018252361,126.72087354917,9.9429,22.3000,0.0200,-0.0202,-0.0026,-0.507713263,-0.836049091,57.033650756,0.1137,0.1003,0.0968,0.0282,0.0271,0.0207,0.0279,0.0280,0.0940,0f000041,0*8b0a5aac", "robot status", "#DUALANTENNAHEADINGA,USB3,0,45.5,FINESTEERING,2113,382076.500,02008000,d426,15824;SOL_COMPUTED,NARROW_INT,-1.000000000,62.689403534,-14.039703369,0.0,0.542382181,0.895851910,\"681H\",35,23,23,17,04,00,30,33*84645a55", "robot status", "#INSPVAXA,USB3,0,45.5,FINESTEERING,2113,382076.550,02008000,471d,15824;INS_SOLUTION_GOOD,INS_RTKFIXED,37.37018251831,126.72087352935,9.9427,22.3000,0.0231,-0.0036,-0.0023,-0.516288123,-0.834689327,56.977501046,0.1137,0.1003,0.0968,0.0282,0.0271,0.0207,0.0279,0.0280,0.0940,0f000041,0*028672f1", "robot status", "#DUALANTENNAHEADINGA,USB3,0,45.5,FINESTEERING,2113,382076.600,02008000,d426,15824;SOL_COMPUTED,NARROW_INT,-1.000000000,62.613159180,-13.677642822,0.0,0.536181331,0.891214252,\"681H\",35,23,23,17,04,00,30,33*ab1fa589", "robot status", "#INSPVAXA,USB3,0,45.5,FINESTEERING,2113,382076.700,02008000,471d,15824;INS_SOLUTION_GOOD,INS_RTKFIXED,37.37018249873,126.72087348635,9.9425,22.3000,-0.0050,-0.0469,-0.0042,-0.500776644,-0.862598426,56.577039938,0.1137,0.1003,0.0968,0.0282,0.0271,0.0207,0.0279,0.0280,0.0940,0f000041,0*69866e08", "robot status", "#DUALANTENNAHEADINGA,USB3,0,45.5,FINESTEERING,2113,382076.700,02008000,d426,15824;SOL_COMPUTED,NARROW_INT,-1.000000000,62.160305023,-14.089050293,0.0,0.540129185,0.890074372,\"681H\",35,23,23,17,04,00,30,33*c004067f", "robot status", "#INSPVAXA,USB3,0,45.5,FINESTEERING,2113,382076.750,02008000,471d,15824;INS_SOLUTION_GOOD,INS_RTKFIXED,37.37018248264,126.72087344949,9.9424,22.3000,-0.0144,-0.0738,-0.0032,-0.507775550,-0.871395656,56.420424796,0.1137,0.1003,0.0968,0.0282,0.0271,0.0207,0.0279,0.0280,0.0940,0f000041,0*259c79b5", "robot status", "#DUALANTENNAHEADINGA,USB3,0,45.5,FINESTEERING,2113,382076.800,02008000,d426,15824;SOL_COMPUTED,NARROW_INT,-1.000000000,61.583477020,-15.025451660,0.0,0.534774482,0.874262989,\"681H\",35,23,23,17,04,00,30,33*2e2eea9f", "robot status", "#INSPVAXA,USB3,0,45.5,FINESTEERING,2113,382076.900,02008000,471d,15824;INS_SOLUTION_GOOD,INS_RTKFIXED,37.37018238089,126.72087320439,9.9428,22.3000,-0.0984,-0.2093,0.0012,-0.552659634,-0.816157337,55.404341314,0.1137,0.1003,0.0968,0.0282,0.0271,0.0207,0.0279,0.0280,0.0940,0f000041,0*beabe4af", "robot status", "#DUALANTENNAHEADINGA,USB3,0,45.5,FINESTEERING,2113,382076.900,02008000,d426,15824;SOL_COMPUTED,NARROW_INT,-1.000000000,60.593006134,-15.024047852,0.0,0.535586357,0.873998046,\"681H\",34,23,23,17,04,00,30,33*1c4ac519", "robot status", "#INSPVAXA,USB3,0,45.5,FINESTEERING,2113,382076.950,02008000,471d,15824;INS_SOLUTION_GOOD,INS_RTKFIXED,37.37018231794,126.72087306992,9.9427,22.3000,-0.1311,-0.2546,-0.0083,-0.589583080,-0.828109403,55.103046016,0.1137,0.1003,0.0968,0.0282,0.0271,0.0207,0.0279,0.0280,0.0940,0f000041,0*ee3d7094", "robot status", "#DUALANTENNAHEADINGA,USB3,0,45.5,FINESTEERING,2113,382077.000,02008000,d426,15824;SOL_COMPUTED,NARROW_INT,-1.000000000,60.373241425,-14.698272705,0.0,0.533141017,0.874071717,\"681H\",35,23,23,17,04,00,30,33*5a275546", "robot status", "#INSPVAXA,USB3,0,45.5,FINESTEERING,2113,382077.050,02008000,471d,15824;INS_SOLUTION_GOOD,INS_RTKFIXED,37.37018215217,126.72087275361,9.9423,22.3000,-0.1734,-0.3002,-0.0023,-0.589762244,-0.790996978,54.526795048,0.1220,0.1112,0.1028,0.0299,0.0288,0.0212,0.0286,0.0287,0.0947,0f000041,0*53551944", "robot status", "#INSPVAXA,USB3,0,45.5,FINESTEERING,2113,382077.150,02008000,471d,15824;INS_SOLUTION_GOOD,INS_RTKFIXED,37.37018196863,126.72087241035,9.9422,22.3000,-0.1763,-0.2971,-0.0107,-0.613721377,-0.890660641,54.210564854,0.1220,0.1112,0.1028,0.0299,0.0288,0.0212,0.0286,0.0287,0.0947,0f000041,0*8b060a35", "robot status", "#INSPVAXA,USB3,0,45.5,FINESTEERING,2113,382077.150,02008000,471d,15824;INS_SOLUTION_GOOD,INS_RTKFIXED,37.37018196863,126.72087241035,9.9422,22.3000,-0.1763,-0.2971,-0.0107,-0.613721377,-0.890660641,54.210564854,0.1220,0.1112,0.1028,0.0299,0.0288,0.0212,0.0286,0.0287,0.0947,0f000041,0*8b060a35", "robot status", "#DUALANTENNAHEADINGA,USB3,0,45.5,FINESTEERING,2113,382077.200,02008000,d426,15824;SOL_COMPUTED,NARROW_INT,-1.000000000,59.077186584,-14.386932373,0.0,0.535175920,0.874459386,\"681H\",36,24,24,17,04,00,30,33*3dce839e", "robot status", "#INSPVAXA,USB3,0,45.5,FINESTEERING,2113,382077.300,02000000,471d,15824;INS_SOLUTION_GOOD,INS_RTKFIXED,37.37018172360,126.72087200522,9.9414,22.3000,-0.1144,-0.1811,-0.0158,-0.497439215,-0.601652755,54.071825419,0.1220,0.1112,0.1028,0.0299,0.0288,0.0212,0.0286,0.0287,0.0947,0f000041,0*36964435", "robot status", "#INSPVAXA,USB3,0,45.5,FINESTEERING,2113,382077.350,02000000,471d,15824;INS_SOLUTION_GOOD,INS_RTKFIXED,37.37018167003,126.72087191931,9.9409,22.3000,-0.0726,-0.1289,-0.0017,-0.447445485,-0.558476653,54.129696835,0.1220,0.1112,0.1028,0.0299,0.0288,0.0212,0.0286,0.0287,0.0947,0f000041,0*b4372186", "robot status", "#INSPVAXA,USB3,0,45.5,FINESTEERING,2113,382077.350,02000000,471d,15824;INS_SOLUTION_GOOD,INS_RTKFIXED,37.37018167003,126.72087191931,9.9409,22.3000,-0.0726,-0.1289,-0.0017,-0.447445485,-0.558476653,54.129696835,0.1220,0.1112,0.1028,0.0299,0.0288,0.0212,0.0286,0.0287,0.0947,0f000041,0*b4372186", "robot status", "#DUALANTENNAHEADINGA,USB3,0,45.5,FINESTEERING,2113,382077.400,02000000,d426,15824;SOL_COMPUTED,NARROW_INT,-1.000000000,59.565399170,-14.847381592,0.0,0.535671532,0.875570297,\"681H\",36,24,24,17,04,00,30,33*723e8b8b", "robot status", "#INSPVAXA,USB3,0,45.5,FINESTEERING,2113,382077.450,02000000,471d,15824;INS_SOLUTION_GOOD,INS_RTKFIXED,37.37018161371,126.72087182468,9.9406,22.3000,-0.0039,-0.0530,-0.0008,-0.362280489,-0.655369448,54.327688551,0.1220,0.1112,0.1028,0.0299,0.0288,0.0212,0.0286,0.0287,0.0947,0f000041,0*ea7967f9", "robot status", "#INSPVAXA,USB3,0,45.5,FINESTEERING,2113,382077.550,02000000,471d,15824;INS_SOLUTION_GOOD,INS_RTKFIXED,37.37018160610,126.72087180297,9.9399,22.3000,0.0343,0.0107,-0.0009,-0.407000122,-0.638946441,54.323525463,0.1220,0.1112,0.1028,0.0299,0.0288,0.0212,0.0286,0.0287,0.0947,0f000041,0*f917b60f", "robot status", "#INSPVAXA,USB3,0,45.5,FINESTEERING,2113,382077.550,02000000,471d,15824;INS_SOLUTION_GOOD,INS_RTKFIXED,37.37018160610,126.72087180297,9.9399,22.3000,0.0343,0.0107,-0.0009,-0.407000122,-0.638946441,54.323525463,0.1220,0.1112,0.1028,0.0299,0.0288,0.0212,0.0286,0.0287,0.0947,0f000041,0*f917b60f", "robot status", "#DUALANTENNAHEADINGA,USB3,0,45.5,FINESTEERING,2113,382077.600,02000000,d426,15824;SOL_COMPUTED,NARROW_INT,-1.000000000,59.926795959,-13.898925781,0.0,0.532789528,0.896207094,\"681H\",34,24,24,17,04,00,30,33*99594338", "robot status", "#INSPVAXA,USB3,0,45.5,FINESTEERING,2113,382077.700,02000000,471d,15824;INS_SOLUTION_GOOD,INS_RTKFIXED,37.37018162718,126.72087183707,9.9389,22.3000,0.0425,0.0109,-0.0039,-0.397074034,-0.674477817,54.407107545,0.1220,0.1112,0.1028,0.0299,0.0288,0.0212,0.0286,0.0287,0.0947,0f000041,0*971b41c3", "robot status", "#INSPVAXA,USB3,0,45.5,FINESTEERING,2113,382077.750,02000000,471d,15824;INS_SOLUTION_GOOD,INS_RTKFIXED,37.37018163294,126.72087184197,9.9386,22.3000,0.0304,0.0019,-0.0031,-0.401095985,-0.676812542,54.401108405,0.1220,0.1112,0.1028,0.0299,0.0288,0.0212,0.0286,0.0287,0.0947,0f000041,0*4934b136", "robot status", "#INSPVAXA,USB3,0,45.5,FINESTEERING,2113,382077.800,02000000,471d,15824;INS_SOLUTION_GOOD,INS_RTKFIXED,37.37018163353,126.72087184005,9.9384,22.3000,0.0198,-0.0128,-0.0038,-0.399057042,-0.682784219,54.425903921,0.1220,0.1112,0.1028,0.0299,0.0288,0.0212,0.0286,0.0287,0.0947,0f000041,0*746c6d10", "robot status", "#DUALANTENNAHEADINGA,USB3,0,45.5,FINESTEERING,2113,382077.800,02000000,d426,15824;SOL_COMPUTED,NARROW_INT,-1.000000000,59.770839691,-14.208770752,0.0,0.535655320,0.896162331,\"681H\",34,24,24,17,04,00,30,33*2e155f98", "robot status", "#INSPVAXA,USB3,0,45.5,FINESTEERING,2113,382077.900,02000000,471d,15824;INS_SOLUTION_GOOD,INS_RTKFIXED,37.37018162317,126.72087181517,9.9378,22.3000,0.0090,-0.0293,-0.0037,-0.399270460,-0.665854087,54.408406980,0.1220,0.1112,0.1028,0.0299,0.0288,0.0212,0.0286,0.0287,0.0947,0f000041,0*2a56ea16", "robot status", "#INSPVAXA,USB3,0,45.5,FINESTEERING,2113,382077.950,02000000,471d,15824;INS_SOLUTION_GOOD,INS_RTKFIXED,37.37018161724,126.72087180065,9.9375,22.3000,0.0110,-0.0263,-0.0033,-0.396788774,-0.662807281,54.417128028,0.1220,0.1112,0.1028,0.0299,0.0288,0.0212,0.0286,0.0287,0.0947,0f000041,0*2f978761", "robot status", "#INSPVAXA,USB3,0,45.5,FINESTEERING,2113,382078.000,02000000,471d,15824;INS_SOLUTION_GOOD,INS_RTKFIXED,37.37018161317,126.72087178831,9.9373,22.3000,0.0165,-0.0214,-0.0036,-0.396018645,-0.661337907,54.419607778,0.1220,0.1112,0.1028,0.0299,0.0288,0.0212,0.0286,0.0287,0.0947,0f000041,0*80f08117", "robot status", "#DUALANTENNAHEADINGA,USB3,0,45.5,FINESTEERING,2113,382078.000,02000000,d426,15824;SOL_COMPUTED,NARROW_INT,-1.000000000,59.611606598,-15.507110596,0.0,0.535073936,0.887549400,\"681H\",34,24,24,17,04,00,30,33*82b8fb6e", "robot status", "#INSPVAXA,USB3,0,41.5,FINESTEERING,2113,382078.050,02000000,471d,15824;INS_SOLUTION_GOOD,INS_RTKFIXED,37.37018160978,126.72087178279,9.9369,22.3000,0.0218,-0.0137,-0.0033,-0.398775668,-0.659662557,54.410397614,0.1299,0.1219,0.1088,0.0313,0.0302,0.0217,0.0296,0.0296,0.0954,0f000041,0*63691409", "robot status", "#INSPVAXA,USB3,0,41.5,FINESTEERING,2113,382078.150,02000000,471d,15824;INS_SOLUTION_GOOD,INS_RTKFIXED,37.37018161040,126.72087178177,9.9360,22.3000,0.0235,-0.0110,-0.0034,-0.396035363,-0.668307330,54.423184386,0.1299,0.1219,0.1088,0.0313,0.0302,0.0217,0.0296,0.0296,0.0954,0f000041,0*aef97e91", "robot status", "#INSPVAXA,USB3,0,41.5,FINESTEERING,2113,382078.200,02000000,471d,15824;INS_SOLUTION_GOOD,INS_RTKFIXED,37.37018161042,126.72087177969,9.9355,22.3000,0.0209,-0.0151,-0.0033,-0.397956439,-0.668828835,54.417422562,0.1299,0.1219,0.1088,0.0313,0.0302,0.0217,0.0296,0.0296,0.0954,0f000041,0*b88bd42c", "robot status", "#INSPVAXA,USB3,0,41.5,FINESTEERING,2113,382078.250,02000000,471d,15824;INS_SOLUTION_GOOD,INS_RTKFIXED,37.37018160766,126.72087177622,9.9351,22.3000,0.0175,-0.0183,-0.0034,-0.398020483,-0.668988255,54.420981971,0.1299,0.1219,0.1088,0.0313,0.0302,0.0217,0.0296,0.0296,0.0954,0f000041,0*9aa3f1b5", "robot status", "#INSPVAXA,USB3,0,41.5,FINESTEERING,2113,382078.300,02000000,471d,15824;INS_SOLUTION_GOOD,INS_RTKFIXED,37.37018160552,126.72087177058,9.9346,22.3000,0.0169,-0.0198,-0.0036,-0.397716535,-0.665195345,54.421386188,0.1299,0.1219,0.1088,0.0313,0.0302,0.0217,0.0296,0.0296,0.0954,0f000041,0*bb410fd7", "robot status", "#INSPVAXA,USB3,0,41.5,FINESTEERING,2113,382078.350,02000000,471d,15824;INS_SOLUTION_GOOD,INS_RTKFIXED,37.37018160380,126.72087176493,9.9342,22.3000,0.0186,-0.0184,-0.0036,-0.398193646,-0.664642248,54.414736655,0.1299,0.1219,0.1088,0.0313,0.0302,0.0217,0.0296,0.0296,0.0954,0f000041,0*63de3f06", "robot status", "#INSPVAXA,USB3,0,41.5,FINESTEERING,2113,382078.400,02000000,471d,15824;INS_SOLUTION_GOOD,INS_RTKFIXED,37.37018160287,126.72087176066,9.9337,22.3000,0.0199,-0.0153,-0.0038,-0.399027521,-0.664851123,54.418583348,0.1299,0.1219,0.1088,0.0313,0.0302,0.0217,0.0296,0.0296,0.0954,0f000041,0*d7739379", "robot status", "#INSPVAXA,USB3,0,41.5,FINESTEERING,2113,382078.450,02000000,471d,15824;INS_SOLUTION_GOOD,INS_RTKFIXED,37.37018160268,126.72087175777,9.9333,22.3000,0.0212,-0.0136,-0.0038,-0.397910090,-0.666900211,54.420803488,0.1299,0.1219,0.1088,0.0313,0.0302,0.0217,0.0296,0.0296,0.0954,0f000041,0*774b935c", "robot status", "#INSPVAXA,USB3,0,41.5,FINESTEERING,2113,382078.500,02000000,471d,15824;INS_SOLUTION_GOOD,INS_RTKFIXED,37.37018160129,126.72087175599,9.9328,22.3000,0.0212,-0.0135,-0.0036,-0.398174402,-0.666434946,54.418302632,0.1299,0.1219,0.1088,0.0313,0.0302,0.0217,0.0296,0.0296,0.0954,0f000041,0*988239f6", "robot status", "#INSPVAXA,USB3,0,41.5,FINESTEERING,2113,382078.550,02000000,471d,15824;INS_SOLUTION_GOOD,INS_RTKFIXED,37.37018160137,126.72087175305,9.9324,22.3000,0.0207,-0.0148,-0.0037,-0.398174533,-0.667806460,54.423686726,0.1299,0.1219,0.1088,0.0313,0.0302,0.0217,0.0296,0.0296,0.0954,0f000041,0*6c7bc505", "robot status", "#INSPVAXA,USB3,0,41.5,FINESTEERING,2113,382078.600,02000000,471d,15824;INS_SOLUTION_GOOD,INS_RTKFIXED,37.37018160091,126.72087174913,9.9319,22.3000,0.0184,-0.0168,-0.0034,-0.399616763,-0.669406373,54.426163412,0.1299,0.1219,0.1088,0.0313,0.0302,0.0217,0.0296,0.0296,0.0954,0f000041,0*b5b42f08", "robot status", "#INSPVAXA,USB3,0,41.5,FINESTEERING,2113,382078.650,02000000,471d,15824;INS_SOLUTION_GOOD,INS_RTKFIXED,37.37018159810,126.72087174489,9.9314,22.3000,0.0169,-0.0182,-0.0033,-0.398930269,-0.667860840,54.420936487,0.1299,0.1219,0.1088,0.0313,0.0302,0.0217,0.0296,0.0296,0.0954,0f000041,0*b782ba33", "robot status", "#INSPVAXA,USB3,0,41.5,FINESTEERING,2113,382078.700,02000000,471d,15824;INS_SOLUTION_GOOD,INS_RTKFIXED,37.37018159682,126.72087173967,9.9310,22.3000,0.0181,-0.0175,-0.0033,-0.397860800,-0.666807611,54.421680581,0.1299,0.1219,0.1088,0.0313,0.0302,0.0217,0.0296,0.0296,0.0954,0f000041,0*9a5525e9", "robot status", "#INSPVAXA,USB3,0,41.5,FINESTEERING,2113,382078.750,02000000,471d,15824;INS_SOLUTION_GOOD,INS_RTKFIXED,37.37018159639,126.72087173527,9.9306,22.3000,0.0201,-0.0153,-0.0033,-0.399098829,-0.666006999,54.421519606,0.1299,0.1219,0.1088,0.0313,0.0302,0.0217,0.0296,0.0296,0.0954,0f000041,0*7c509bd9", "robot status", "#INSPVAXA,USB3,0,41.5,FINESTEERING,2113,382078.800,02000000,471d,15824;INS_SOLUTION_GOOD,INS_RTKFIXED,37.37018159671,126.72087173215,9.9302,22.3000,0.0211,-0.0131,-0.0035,-0.398269724,-0.667477964,54.424615148,0.1299,0.1219,0.1088,0.0313,0.0302,0.0217,0.0296,0.0296,0.0954,0f000041,0*ea8744d8", "robot status", "#INSPVAXA,USB3,0,41.5,FINESTEERING,2113,382078.850,02000000,471d,15824;INS_SOLUTION_GOOD,INS_RTKFIXED,37.37018159746,126.72087172966,9.9298,22.3000,0.0216,-0.0128,-0.0036,-0.397891359,-0.668083893,54.429116548,0.1299,0.1219,0.1088,0.0313,0.0302,0.0217,0.0296,0.0296,0.0954,0f000041,0*5e1b3e1a", "robot status", "#DUALANTENNAHEADINGA,USB3,0,41.5,FINESTEERING,2113,382078.900,02000000,d426,15824;SOL_COMPUTED,NARROW_INT,-1.000000000,59.889842987,-14.379272461,0.0,0.531375706,0.886130989,\"681H\",34,24,24,17,04,00,30,33*654889e3", "robot status", "#INSPVAXA,USB3,0,41.5,FINESTEERING,2113,382078.950,02000000,471d,15824;INS_SOLUTION_GOOD,INS_RTKFIXED,37.37018159603,126.72087172324,9.9290,22.3000,0.0177,-0.0173,-0.0034,-0.396368187,-0.670564662,54.422242053,0.1299,0.1219,0.1088,0.0313,0.0302,0.0217,0.0296,0.0296,0.0954,0f000041,0*c405c9f4", "robot status", "#INSPVAXA,USB3,0,41.5,FINESTEERING,2113,382079.000,02000000,471d,15824;INS_SOLUTION_GOOD,INS_RTKFIXED,37.37018159546,126.72087171789,9.9285,22.3000,0.0185,-0.0178,-0.0031,-0.396349401,-0.667035889,54.424026339,0.1299,0.1219,0.1088,0.0313,0.0302,0.0217,0.0296,0.0296,0.0954,0f000041,0*615d5fca", "robot status", "#INSPVAXA,USB3,0,41.5,FINESTEERING,2113,382079.050,02000000,471d,15824;INS_SOLUTION_GOOD,INS_RTKFIXED,37.37018159244,126.72087171410,9.9281,22.3000,0.0198,-0.0152,-0.0031,-0.398070359,-0.665172273,54.421390352,0.1368,0.1314,0.1142,0.0325,0.0314,0.0220,0.0304,0.0303,0.0960,0f000041,0*ba5e35ba", "robot status", "#DUALANTENNAHEADINGA,USB3,0,41.5,FINESTEERING,2113,382079.100,02000000,d426,15824;SOL_COMPUTED,NARROW_INT,-1.000000000,59.941829681,-14.307830811,0.0,0.528966308,0.882468522,\"681H\",34,24,24,17,04,00,30,33*7de07ad8", "robot status", "#INSPVAXA,USB3,0,46.0,FINESTEERING,2113,382079.150,02000000,471d,15824;INS_SOLUTION_GOOD,INS_RTKFIXED,37.37018158259,126.72087171187,9.9272,22.3000,0.0212,-0.0126,-0.0034,-0.396422955,-0.668154773,54.424327020,0.1368,0.1314,0.1142,0.0325,0.0314,0.0220,0.0304,0.0303,0.0960,0f000041,0*322b4b38", "robot status", "#INSPVAXA,USB3,0,46.0,FINESTEERING,2113,382079.200,02000000,471d,15824;INS_SOLUTION_GOOD,INS_RTKFIXED,37.37018157890,126.72087171013,9.9268,22.3000,0.0201,-0.0139,-0.0034,-0.398236275,-0.669418783,54.424002459,0.1368,0.1314,0.1142,0.0325,0.0314,0.0220,0.0304,0.0303,0.0960,0f000041,0*293cde3b", "robot status", "#INSPVAXA,USB3,0,46.0,FINESTEERING,2113,382079.250,02000000,471d,15824;INS_SOLUTION_GOOD,INS_RTKFIXED,37.37018157277,126.72087170866,9.9263,22.3000,0.0186,-0.0147,-0.0033,-0.397371016,-0.669938977,54.423078303,0.1368,0.1314,0.1142,0.0325,0.0314,0.0220,0.0304,0.0303,0.0960,0f000041,0*61eb0af1", "robot status", "#DUALANTENNAHEADINGA,USB3,0,46.0,FINESTEERING,2113,382079.300,02000000,d426,15824;SOL_COMPUTED,NARROW_INT,-1.000000000,59.814067841,-14.400115967,0.0,0.525958717,0.873251081,\"681H\",34,24,24,17,04,00,30,33*18aafe1d", "robot status", "#INSPVAXA,USB3,0,46.0,FINESTEERING,2113,382079.350,02000000,471d,15824;INS_SOLUTION_GOOD,INS_RTKFIXED,37.37018156416,126.72087170287,9.9255,22.3000,0.0194,-0.0143,-0.0033,-0.398999728,-0.667771127,54.423007051,0.1368,0.1314,0.1142,0.0325,0.0314,0.0220,0.0304,0.0303,0.0960,0f000041,0*3dc3c330", "robot status", "#INSPVAXA,USB3,0,46.0,FINESTEERING,2113,382079.400,02000000,471d,15824;INS_SOLUTION_GOOD,INS_RTKFIXED,37.37018156035,126.72087170090,9.9250,22.3000,0.0198,-0.0123,-0.0032,-0.397973722,-0.668018270,54.421543700,0.1368,0.1314,0.1142,0.0325,0.0314,0.0220,0.0304,0.0303,0.0960,0f000041,0*857c2bda", "robot status", "#INSPVAXA,USB3,0,46.0,FINESTEERING,2113,382079.450,02000000,471d,15824;INS_SOLUTION_GOOD,INS_RTKFIXED,37.37018155685,126.72087169962,9.9246,22.3000,0.0206,-0.0117,-0.0028,-0.396928906,-0.669763009,54.423567528,0.1368,0.1314,0.1142,0.0325,0.0314,0.0220,0.0304,0.0303,0.0960,0f000041,0*d6e435db", "robot status", "#DUALANTENNAHEADINGA,USB3,0,46.0,FINESTEERING,2113,382079.500,02000000,d426,15824;SOL_COMPUTED,NARROW_INT,-1.000000000,59.825092316,-13.806610107,0.0,0.529175401,0.882389426,\"681H\",34,24,24,17,04,00,30,33*cf8397ca", "robot status", "#INSPVAXA,USB3,0,46.0,FINESTEERING,2113,382079.550,02000000,471d,15824;INS_SOLUTION_GOOD,INS_RTKFIXED,37.37018154822,126.72087169714,9.9237,22.3000,0.0199,-0.0123,-0.0031,-0.399439833,-0.671173171,54.423917497,0.1368,0.1314,0.1142,0.0325,0.0314,0.0220,0.0304,0.0303,0.0960,0f000041,0*72c7be21", "robot status", "#INSPVAXA,USB3,0,46.0,FINESTEERING,2113,382079.600,02000000,471d,15824;INS_SOLUTION_GOOD,INS_RTKFIXED,37.37018154473,126.72087169552,9.9232,22.3000,0.0192,-0.0124,-0.0029,-0.398842312,-0.669897708,54.426511830,0.1368,0.1314,0.1142,0.0325,0.0314,0.0220,0.0304,0.0303,0.0960,0f000041,0*c78fac7d", "robot status", "#INSPVAXA,USB3,0,46.0,FINESTEERING,2113,382079.650,02000000,471d,15824;INS_SOLUTION_GOOD,INS_RTKFIXED,37.37018153923,126.72087169442,9.9227,22.3000,0.0187,-0.0129,-0.0037,-0.398115569,-0.670222367,54.423758813,0.1368,0.1314,0.1142,0.0325,0.0314,0.0220,0.0304,0.0303,0.0960,0f000041,0*cc33372d", "robot status", "#INSPVAXA,USB3,0,46.0,FINESTEERING,2113,382079.700,02000000,471d,15824;INS_SOLUTION_GOOD,INS_RTKFIXED,37.37018153583,126.72087169255,9.9222,22.3000,0.0194,-0.0123,-0.0038,-0.398652530,-0.669843731,54.425900568,0.1368,0.1314,0.1142,0.0325,0.0314,0.0220,0.0304,0.0303,0.0960,0f000041,0*310aecbf", "robot status", "#INSPVAXA,USB3,0,46.0,FINESTEERING,2113,382079.750,02000000,471d,15824;INS_SOLUTION_GOOD,INS_RTKFIXED,37.37018153270,126.72087169107,9.9218,22.3000,0.0193,-0.0115,-0.0035,-0.399699142,-0.670630395,54.429202659,0.1368,0.1314,0.1142,0.0325,0.0314,0.0220,0.0304,0.0303,0.0960,0f000041,0*109cdb27", "robot status", "#DUALANTENNAHEADINGA,USB3,0,46.0,FINESTEERING,2113,382079.800,02000000,d426,15824;SOL_COMPUTED,NARROW_INT,-1.000000000,59.783794403,-14.102447510,0.0,0.536478579,0.886337399,\"681H\",35,24,24,17,04,00,30,33*3abf4920", "robot status", "#INSPVAXA,USB3,0,46.0,FINESTEERING,2113,382079.850,02000000,471d,15824;INS_SOLUTION_GOOD,INS_RTKFIXED,37.37018152419,126.72087168913,9.9208,22.3000,0.0189,-0.0123,-0.0039,-0.397593372,-0.671522308,54.423707419,0.1368,0.1314,0.1142,0.0325,0.0314,0.0220,0.0304,0.0303,0.0960,0f000041,0*99700067", "robot status", "#DUALANTENNAHEADINGA,USB3,0,46.0,FINESTEERING,2113,382079.900,02000000,d426,15824;SOL_COMPUTED,NARROW_INT,-1.000000000,60.035209656,-13.786712646,0.0,0.539343774,0.892305315,\"681H\",35,24,24,17,04,00,30,33*8930a561", "robot status", "#INSPVAXA,USB3,0,46.0,FINESTEERING,2113,382079.950,02000000,471d,15824;INS_SOLUTION_GOOD,INS_RTKFIXED,37.37018151796,126.72087168510,9.9198,22.3000,0.0179,-0.0131,-0.0043,-0.398900813,-0.672273255,54.424599543,0.1368,0.1314,0.1142,0.0325,0.0314,0.0220,0.0304,0.0303,0.0960,0f000041,0*44dbdb1b", "robot status", "#DUALANTENNAHEADINGA,USB3,0,46.0,FINESTEERING,2113,382080.000,02000000,d426,15824;SOL_COMPUTED,NARROW_INT,-1.000000000,60.116764069,-13.842926025,0.0,0.537861764,0.890418410,\"681H\",35,24,24,17,04,00,30,33*a6abe33a", "robot status", "#INSPVAXA,USB3,0,46.0,FINESTEERING,2113,382080.050,02000000,471d,15824;INS_SOLUTION_GOOD,INS_RTKFIXED,37.37018151367,126.72087168296,9.9189,22.3000,0.0202,-0.0112,-0.0044,-0.399381353,-0.671368311,54.426963550,0.1424,0.1392,0.1186,0.0334,0.0323,0.0222,0.0311,0.0310,0.0968,0f000041,0*b23a1702", "robot status", "#DUALANTENNAHEADINGA,USB3,0,46.0,FINESTEERING,2113,382080.100,02000000,d426,15824;SOL_COMPUTED,NARROW_INT,-1.000000000,60.159118652,-13.784210205,0.0,0.532414675,0.881637812,\"681H\",35,24,24,17,04,00,30,33*6f9a432b", "robot status", "#INSPVAXA,USB3,0,48.0,FINESTEERING,2113,382080.150,02000000,471d,15824;INS_SOLUTION_GOOD,INS_RTKFIXED,37.37018150494,126.72087168805,9.9182,22.3000,0.0175,-0.0120,-0.0048,-0.396774071,-0.671861596,54.426036874,0.1424,0.1392,0.1186,0.0334,0.0323,0.0222,0.0311,0.0310,0.0968,0f000041,0*6943e9be", "robot status", "#DUALANTENNAHEADINGA,USB3,0,48.0,FINESTEERING,2113,382080.200,02000000,d426,15824;SOL_COMPUTED,NARROW_INT,-1.000000000,60.061973572,-13.714172363,0.0,0.531580806,0.881464720,\"681H\",35,24,24,17,04,00,30,33*18c6a979", "robot status", "#INSPVAXA,USB3,0,48.0,FINESTEERING,2113,382080.250,02000000,471d,15824;INS_SOLUTION_GOOD,INS_RTKFIXED,37.37018149653,126.72087169283,9.9174,22.3000,0.0204,-0.0094,-0.0053,-0.398649737,-0.668881888,54.426585634,0.1424,0.1392,0.1186,0.0334,0.0323,0.0222,0.0311,0.0310,0.0968,0f000041,0*eb54c9ce", "robot status", "#DUALANTENNAHEADINGA,USB3,0,48.0,FINESTEERING,2113,382080.300,02000000,d426,15824;SOL_COMPUTED,NARROW_INT,-1.000000000,60.245460510,-13.417510986,0.0,0.529223621,0.880011678,\"681H\",35,24,24,17,04,00,30,33*2703d42e", "robot status", "#INSPVAXA,USB3,0,48.0,FINESTEERING,2113,382080.350,02000000,471d,15824;INS_SOLUTION_GOOD,INS_RTKFIXED,37.37018149027,126.72087169830,9.9167,22.3000,0.0172,-0.0116,-0.0056,-0.396532163,-0.673442279,54.429501470,0.1424,0.1392,0.1186,0.0334,0.0323,0.0222,0.0311,0.0310,0.0968,0f000041,0*e7062904", "robot status", "#DUALANTENNAHEADINGA,USB3,0,48.0,FINESTEERING,2113,382080.400,02000000,d426,15824;SOL_COMPUTED,NARROW_INT,-1.000000000,60.290962219,-13.224334717,0.0,0.532243669,0.883669376,\"681H\",35,24,24,17,04,00,30,33*4f40ffbc", "robot status", "#INSPVAXA,USB3,0,48.0,FINESTEERING,2113,382080.450,02000000,471d,15824;INS_SOLUTION_GOOD,INS_RTKFIXED,37.37018148140,126.72087169820,9.9159,22.3000,0.0152,-0.0148,-0.0049,-0.397557309,-0.670707864,54.433161289,0.1424,0.1392,0.1186,0.0334,0.0323,0.0222,0.0311,0.0310,0.0968,0f000041,0*523f8663", "robot status", "#INSPVAXA,USB3,0,48.0,FINESTEERING,2113,382080.500,02000000,471d,15824;INS_SOLUTION_GOOD,INS_RTKFIXED,37.37018147421,126.72087169857,9.9155,22.3000,0.0108,-0.0149,-0.0066,-0.405540805,-0.678661443,54.522406923,0.1424,0.1392,0.1186,0.0334,0.0323,0.0222,0.0311,0.0310,0.0968,0f000041,0*fe2d6248", "robot status", "#INSPVAXA,USB3,0,48.0,FINESTEERING,2113,382080.550,02000000,471d,15824;INS_SOLUTION_GOOD,INS_RTKFIXED,37.37018146810,126.72087169714,9.9151,22.3000,0.0128,-0.0177,-0.0054,-0.391653226,-0.683202130,54.625186039,0.1424,0.1392,0.1186,0.0334,0.0323,0.0222,0.0311,0.0310,0.0968,0f000041,0*ce9f916f", "robot status", "#DUALANTENNAHEADINGA,USB3,0,48.0,FINESTEERING,2113,382080.600,02000000,d426,15824;SOL_COMPUTED,NARROW_INT,-1.000000000,60.232620239,-14.380371094,0.0,0.528812766,0.868161440,\"681H\",34,24,24,17,04,00,30,33*4216726c", "robot status", "#INSPVAXA,USB3,0,48.0,FINESTEERING,2113,382080.650,02000000,471d,15824;INS_SOLUTION_GOOD,INS_RTKFIXED,37.37018145637,126.72087169284,9.9143,22.3000,0.0114,-0.0155,-0.0052,-0.407772434,-0.681312462,54.550452734,0.1424,0.1392,0.1186,0.0334,0.0323,0.0222,0.0311,0.0310,0.0968,0f000041,0*3b17ad47", "robot status", "#DUALANTENNAHEADINGA,USB3,0,48.0,FINESTEERING,2113,382080.700,02000000,d426,15824;SOL_COMPUTED,NARROW_INT,-1.000000000,60.085067749,-14.072662354,0.0,0.529727459,0.869054377,\"681H\",34,24,24,17,04,00,30,33*d83580fa", "robot status", "#INSPVAXA,USB3,0,48.0,FINESTEERING,2113,382080.750,02000000,471d,15824;INS_SOLUTION_GOOD,INS_RTKFIXED,37.37018144729,126.72087169159,9.9136,22.3000,0.0191,-0.0137,-0.0052,-0.399806112,-0.682917635,54.593925319,0.1424,0.1392,0.1186,0.0334,0.0323,0.0222,0.0311,0.0310,0.0968,0f000041,0*4300c557", "robot status", "#DUALANTENNAHEADINGA,USB3,0,48.0,FINESTEERING,2113,382080.800,02000000,d426,15824;SOL_COMPUTED,NARROW_INT,-1.000000000,60.370964050,-13.838134766,0.0,0.530179918,0.868467510,\"681H\",34,24,24,17,04,00,30,33*ec4b03a6", "robot status", "#INSPVAXA,USB3,0,48.0,FINESTEERING,2113,382080.850,02000000,471d,15824;INS_SOLUTION_GOOD,INS_RTKFIXED,37.37018144038,126.72087169738,9.9128,22.3000,0.0187,-0.0055,-0.0054,-0.399252996,-0.684225007,54.587489530,0.1424,0.1392,0.1186,0.0334,0.0323,0.0222,0.0311,0.0310,0.0968,0f000041,0*44811b23", "robot status", "#DUALANTENNAHEADINGA,USB3,0,48.0,FINESTEERING,2113,382080.900,02000000,d426,15824;SOL_COMPUTED,NARROW_INT,-1.000000000,60.166244507,-13.964385986,0.0,0.533408284,0.870074272,\"681H\",34,24,24,17,04,00,30,33*580d984c", "robot status", "#INSPVAXA,USB3,0,48.0,FINESTEERING,2113,382080.950,02000000,471d,15824;INS_SOLUTION_GOOD,INS_RTKFIXED,37.37018143880,126.72087170543,9.9119,22.3000,0.0216,-0.0054,-0.0061,-0.403932440,-0.683505769,54.576362487,0.1424,0.1392,0.1186,0.0334,0.0323,0.0222,0.0311,0.0310,0.0968,0f000041,0*fb9eceaf", "robot status", "#DUALANTENNAHEADINGA,USB3,0,48.0,FINESTEERING,2113,382081.000,02000000,d426,15824;SOL_COMPUTED,NARROW_INT,-1.000000000,60.232143402,-13.753814697,0.0,0.529545546,0.870563447,\"681H\",34,24,24,16,04,00,30,33*40e98ecf", "robot status", "#INSPVAXA,USB3,0,46.5,FINESTEERING,2113,382081.050,02008000,471d,15824;INS_SOLUTION_GOOD,INS_RTKFIXED,37.37018143287,126.72087171622,9.9112,22.3000,0.0213,-0.0061,-0.0064,-0.399597178,-0.684844699,54.595372573,0.1468,0.1451,0.1221,0.0342,0.0330,0.0223,0.0318,0.0315,0.0975,0f000041,0*0da9dcd5", "robot status", "#DUALANTENNAHEADINGA,USB3,0,46.5,FINESTEERING,2113,382081.100,02008000,d426,15824;SOL_COMPUTED,NARROW_INT,-1.000000000,60.297271729,-13.351257324,0.0,0.527526021,0.870191038,\"681H\",34,24,24,16,04,00,30,33*e993ee68", "robot status", "#INSPVAXA,USB3,0,46.5,FINESTEERING,2113,382081.150,02008000,471d,15824;INS_SOLUTION_GOOD,INS_RTKFIXED,37.37018142721,126.72087172681,9.9107,22.3000,0.0213,-0.0026,-0.0063,-0.402063454,-0.681611270,54.588070203,0.1468,0.1451,0.1221,0.0342,0.0330,0.0223,0.0318,0.0315,0.0975,0f000041,0*9a52a31f", "robot status", "#DUALANTENNAHEADINGA,USB3,0,46.5,FINESTEERING,2113,382081.200,02008000,d426,15824;SOL_COMPUTED,NARROW_INT,-1.000000000,60.289707184,-13.986694336,0.0,0.524844110,0.860907912,\"681H\",34,26,26,17,04,00,30,33*4bb5cbef", "robot status", "#INSPVAXA,USB3,0,46.5,FINESTEERING,2113,382081.250,02008000,471d,15824;INS_SOLUTION_GOOD,INS_RTKFIXED,37.37018142119,126.72087174130,9.9102,22.3000,0.0234,-0.0021,-0.0061,-0.403048108,-0.681838668,54.585043545,0.1468,0.1451,0.1221,0.0342,0.0330,0.0223,0.0318,0.0315,0.0975,0f000041,0*ed04521f", "robot status", "#DUALANTENNAHEADINGA,USB3,0,46.5,FINESTEERING,2113,382081.300,02008000,d426,15824;SOL_COMPUTED,NARROW_INT,-1.000000000,60.037281036,-14.538482666,0.0,0.527922332,0.858946800,\"681H\",34,26,26,17,04,00,30,33*c65f6c88", "robot status", "#INSPVAXA,USB3,0,46.5,FINESTEERING,2113,382081.350,02008000,471d,15824;INS_SOLUTION_GOOD,INS_RTKFIXED,37.37018141744,126.72087175508,9.9096,22.3000,0.0228,-0.0019,-0.0060,-0.402446572,-0.680978796,54.590529258,0.1468,0.1451,0.1221,0.0342,0.0330,0.0223,0.0318,0.0315,0.0975,0f000041,0*7b7496c4", "robot status", "#DUALANTENNAHEADINGA,USB3,0,46.5,FINESTEERING,2113,382081.400,02008000,d426,15824;SOL_COMPUTED,NARROW_INT,-1.000000000,60.059219360,-13.669250488,0.0,0.527933419,0.864375412,\"681H\",34,26,26,17,04,00,30,33*0ae3bf03", "robot status", "#INSPVAXA,USB3,0,46.5,FINESTEERING,2113,382081.450,02008000,471d,15824;INS_SOLUTION_GOOD,INS_RTKFIXED,37.37018141389,126.72087176676,9.9091,22.3000,0.0214,-0.0039,-0.0060,-0.406996481,-0.678245532,54.584688998,0.1468,0.1451,0.1221,0.0342,0.0330,0.0223,0.0318,0.0315,0.0975,0f000041,0*abcd2ed9", "robot status", "#DUALANTENNAHEADINGA,USB3,0,46.5,FINESTEERING,2113,382081.500,02008000,d426,15824;SOL_COMPUTED,NARROW_INT,-1.000000000,60.084037781,-13.930175781,0.0,0.529839158,0.864973605,\"681H\",34,26,26,17,04,00,30,33*556d484c", "robot status", "#INSPVAXA,USB3,0,46.5,FINESTEERING,2113,382081.550,02008000,471d,15824;INS_SOLUTION_GOOD,INS_RTKFIXED,37.37018140638,126.72087177611,9.9086,22.3000,0.0175,-0.0090,-0.0059,-0.406762639,-0.678961697,54.592087445,0.1468,0.1451,0.1221,0.0342,0.0330,0.0223,0.0318,0.0315,0.0975,0f000041,0*7acf6259", "robot status", "#DUALANTENNAHEADINGA,USB3,0,46.5,FINESTEERING,2113,382081.600,02008000,d426,15824;SOL_COMPUTED,NARROW_INT,-1.000000000,60.068412781,-13.598083496,0.0,0.531127989,0.871529698,\"681H\",34,26,26,17,04,00,30,33*3095b456", "robot status", "#INSPVAXA,USB3,0,46.5,FINESTEERING,2113,382081.650,02008000,471d,15824;INS_SOLUTION_GOOD,INS_RTKFIXED,37.37018139506,126.72087177843,9.9080,22.3000,0.0134,-0.0150,-0.0061,-0.404313037,-0.680099764,54.598397920,0.1468,0.1451,0.1221,0.0342,0.0330,0.0223,0.0318,0.0315,0.0975,0f000041,0*92b7f9ce", "robot status", "#DUALANTENNAHEADINGA,USB3,0,46.5,FINESTEERING,2113,382081.700,02008000,d426,15824;SOL_COMPUTED,NARROW_INT,-1.000000000,59.793380737,-14.613891602,0.0,0.536075056,0.868601203,\"681H\",34,26,26,17,04,00,30,33*2d3e2138", "robot status", "#INSPVAXA,USB3,0,46.5,FINESTEERING,2113,382081.750,02008000,471d,15824;INS_SOLUTION_GOOD,INS_RTKFIXED,37.37018138384,126.72087177449,9.9074,22.3000,0.0122,-0.0168,-0.0064,-0.403317289,-0.681143276,54.596812700,0.1468,0.1451,0.1221,0.0342,0.0330,0.0223,0.0318,0.0315,0.0975,0f000041,0*bc6c21b9", "robot status", "#DUALANTENNAHEADINGA,USB3,0,46.5,FINESTEERING,2113,382081.800,02008000,d426,15824;SOL_COMPUTED,NARROW_INT,-1.000000000,59.787136078,-14.922698975,0.0,0.540687501,0.870441020,\"681H\",34,26,26,17,04,00,30,33*ca7c1fba", "robot status", "#INSPVAXA,USB3,0,46.5,FINESTEERING,2113,382081.850,02008000,471d,15824;INS_SOLUTION_GOOD,INS_RTKFIXED,37.37018137172,126.72087177311,9.9069,22.3000,0.0155,-0.0128,-0.0068,-0.401647372,-0.680697328,54.591664227,0.1468,0.1451,0.1221,0.0342,0.0330,0.0223,0.0318,0.0315,0.0975,0f000041,0*13b8b5b8", "robot status", "#DUALANTENNAHEADINGA,USB3,0,46.5,FINESTEERING,2113,382081.900,02008000,d426,15824;SOL_COMPUTED,NARROW_INT,-1.000000000,59.764480591,-15.165435791,0.0,0.536085129,0.862966180,\"681H\",34,26,26,17,04,00,30,33*4703ff4c", "robot status", "#INSPVAXA,USB3,0,46.5,FINESTEERING,2113,382081.950,02008000,471d,15824;INS_SOLUTION_GOOD,INS_RTKFIXED,37.37018136579,126.72087177689,9.9062,22.3000,0.0196,-0.0059,-0.0069,-0.401185482,-0.682283328,54.596993416,0.1468,0.1451,0.1221,0.0342,0.0330,0.0223,0.0318,0.0315,0.0975,0f000041,0*7f6defaf", "robot status", "#DUALANTENNAHEADINGA,USB3,0,46.5,FINESTEERING,2113,382082.000,02008000,d426,15824;SOL_COMPUTED,NARROW_INT,-1.000000000,59.508590698,-15.509246826,0.0,0.538162410,0.863001287,\"681H\",34,26,26,17,04,00,30,33*05aec1e1", "robot status", "#INSPVAXA,USB3,0,45.0,FINESTEERING,2113,382082.050,02008000,471d,15824;INS_SOLUTION_GOOD,INS_RTKFIXED,37.37018136277,126.72087178812,9.9056,22.3000,0.0219,-0.0033,-0.0068,-0.401153112,-0.684091519,54.594790448,0.1501,0.1494,0.1247,0.0348,0.0335,0.0224,0.0323,0.0320,0.0981,0f000041,0*43cd16ac", "robot status", "#DUALANTENNAHEADINGA,USB3,0,45.0,FINESTEERING,2113,382082.100,02008000,d426,15824;SOL_COMPUTED,NARROW_INT,-1.000000000,59.311008453,-16.623962402,0.0,0.535634458,0.848353207,\"681H\",34,26,26,17,04,00,30,33*ea10f673", "robot status", "#INSPVAXA,USB3,0,45.0,FINESTEERING,2113,382082.150,02008000,471d,15824;INS_SOLUTION_GOOD,INS_RTKFIXED,37.37018135899,126.72087180514,9.9051,22.3000,0.0211,-0.0039,-0.0073,-0.399584097,-0.683687283,54.597483993,0.1501,0.1494,0.1247,0.0348,0.0335,0.0224,0.0323,0.0320,0.0981,0f000041,0*5f3220cd", "robot status", "#DUALANTENNAHEADINGA,USB3,0,45.0,FINESTEERING,2113,382082.200,02008000,d426,15824;SOL_COMPUTED,NARROW_INT,-1.000000000,59.744815826,-14.281311035,0.0,0.367778182,0.505855620,\"681H\",34,24,24,17,04,00,30,33*b64f7924", "robot status", "#INSPVAXA,USB3,0,45.0,FINESTEERING,2113,382082.250,02008000,471d,15824;INS_SOLUTION_GOOD,INS_RTKFIXED,37.37018135461,126.72087182030,9.9046,22.3000,0.0201,-0.0056,-0.0074,-0.398057723,-0.682497542,54.600066501,0.1501,0.1494,0.1247,0.0348,0.0335,0.0224,0.0323,0.0320,0.0981,0f000041,0*7afcd4d7", "robot status", "#DUALANTENNAHEADINGA,USB3,0,45.0,FINESTEERING,2113,382082.300,02008000,d426,15824;SOL_COMPUTED,NARROW_INT,-1.000000000,59.761417389,-14.740631104,0.0,0.362006456,0.484096318,\"681H\",35,25,25,17,04,00,30,33*8c279a6b", "robot status", "#INSPVAXA,USB3,0,45.0,FINESTEERING,2113,382082.350,02008000,471d,15824;INS_SOLUTION_GOOD,INS_RTKFIXED,37.37018135117,126.72087183174,9.9040,22.3000,0.0189,-0.0070,-0.0076,-0.399216208,-0.682834702,54.598003280,0.1501,0.1494,0.1247,0.0348,0.0335,0.0224,0.0323,0.0320,0.0981,0f000041,0*19c0e757", "robot status", "#DUALANTENNAHEADINGA,USB3,0,45.0,FINESTEERING,2113,382082.400,02008000,d426,15824;SOL_COMPUTED,NARROW_INT,-1.000000000,59.960609436,-14.247863770,0.0,0.384348780,0.530657828,\"681H\",35,24,24,16,04,00,30,33*a6eab3b2", "robot status", "#INSPVAXA,USB3,0,45.0,FINESTEERING,2113,382082.450,02008000,471d,15824;INS_SOLUTION_GOOD,INS_RTKFIXED,37.37018134731,126.72087184242,9.9034,22.3000,0.0187,-0.0068,-0.0078,-0.399246480,-0.682145137,54.600300461,0.1501,0.1494,0.1247,0.0348,0.0335,0.0224,0.0323,0.0320,0.0981,0f000041,0*87afc3b5", "robot status", "#DUALANTENNAHEADINGA,USB3,0,45.0,FINESTEERING,2113,382082.500,02008000,d426,15824;SOL_COMPUTED,NARROW_INT,-1.000000000,59.854183197,-14.307098389,0.0,0.363931328,0.478495806,\"681H\",35,25,25,18,04,00,30,33*272bf891", "robot status", "#INSPVAXA,USB3,0,45.0,FINESTEERING,2113,382082.550,02008000,471d,15824;INS_SOLUTION_GOOD,INS_RTKFIXED,37.37018134252,126.72087185553,9.9028,22.3000,0.0196,-0.0049,-0.0078,-0.399138446,-0.681436034,54.598451207,0.1501,0.1494,0.1247,0.0348,0.0335,0.0224,0.0323,0.0320,0.0981,0f000041,0*7fb1972c", "robot status", "#DUALANTENNAHEADINGA,USB3,0,45.0,FINESTEERING,2113,382082.600,02008000,d426,15824;SOL_COMPUTED,NARROW_INT,-1.000000000,59.807731628,-14.413726807,0.0,0.375580400,0.484257936,\"681H\",35,26,26,18,04,00,30,33*f16b4954", "robot status", "#INSPVAXA,USB3,0,45.0,FINESTEERING,2113,382082.650,02008000,471d,15824;INS_SOLUTION_GOOD,INS_RTKFIXED,37.37018133903,126.72087187010,9.9021,22.3000,0.0200,-0.0040,-0.0075,-0.399517219,-0.682437422,54.599389636,0.1501,0.1494,0.1247,0.0348,0.0335,0.0224,0.0323,0.0320,0.0981,0f000041,0*53b9ca74", "robot status", "#DUALANTENNAHEADINGA,USB3,0,45.0,FINESTEERING,2113,382082.700,02008000,d426,15824;SOL_COMPUTED,NARROW_INT,-1.000000000,59.778518677,-14.347717285,0.0,0.377171099,0.486210555,\"681H\",33,26,26,18,04,00,30,33*e773823f", "robot status", "#INSPVAXA,USB3,0,45.0,FINESTEERING,2113,382082.750,02008000,471d,15824;INS_SOLUTION_GOOD,INS_RTKFIXED,37.37018133718,126.72087188293,9.9015,22.3000,0.0194,-0.0051,-0.0076,-0.398802701,-0.682383752,54.601313925,0.1501,0.1494,0.1247,0.0348,0.0335,0.0224,0.0323,0.0320,0.0981,0f000041,0*1e34b68b", "robot status", "#DUALANTENNAHEADINGA,USB3,0,45.0,FINESTEERING,2113,382082.800,02008000,d426,15824;SOL_COMPUTED,NARROW_INT,-1.000000000,59.880165100,-14.028411865,0.0,0.379293084,0.489316314,\"681H\",33,26,26,18,04,00,30,33*51c298cf", "robot status", "#INSPVAXA,USB3,0,45.0,FINESTEERING,2113,382082.850,02008000,471d,15824;INS_SOLUTION_GOOD,INS_RTKFIXED,37.37018133355,126.72087189566,9.9009,22.3000,0.0189,-0.0058,-0.0078,-0.398923168,-0.681567036,54.601763118,0.1501,0.1494,0.1247,0.0348,0.0335,0.0224,0.0323,0.0320,0.0981,0f000041,0*56e02d39", "robot status", "#DUALANTENNAHEADINGA,USB3,0,45.0,FINESTEERING,2113,382082.900,02008000,d426,15824;SOL_COMPUTED,NARROW_INT,-1.000000000,59.645057678,-13.522766113,0.0,0.379535854,0.495416105,\"681H\",33,25,25,17,04,00,30,33*13e32d39", "robot status", "#INSPVAXA,USB3,0,45.0,FINESTEERING,2113,382082.950,02008000,471d,15824;INS_SOLUTION_GOOD,INS_RTKFIXED,37.37018133172,126.72087190679,9.9003,22.3000,0.0192,-0.0048,-0.0078,-0.398417978,-0.682805735,54.599250662,0.1501,0.1494,0.1247,0.0348,0.0335,0.0224,0.0323,0.0320,0.0981,0f000041,0*fb2233f9", "robot status", "#DUALANTENNAHEADINGA,USB3,0,45.0,FINESTEERING,2113,382083.000,02008000,d426,15824;SOL_COMPUTED,NARROW_INT,-1.000000000,59.685798645,-13.467620850,0.0,0.379064262,0.494928300,\"681H\",34,25,25,17,04,00,30,33*9042bb7e", "robot status", "#INSPVAXA,USB3,0,45.0,FINESTEERING,2113,382083.050,02008000,471d,15824;INS_SOLUTION_GOOD,INS_RTKFIXED,37.37018132743,126.72087191795,9.8998,22.3000,0.0196,-0.0037,-0.0080,-0.397110561,-0.681788167,54.598575645,0.1525,0.1524,0.1265,0.0353,0.0340,0.0225,0.0327,0.0323,0.0988,0f000041,0*ec74011d", "robot status", "#DUALANTENNAHEADINGA,USB3,0,45.0,FINESTEERING,2113,382083.100,02008000,d426,15824;SOL_COMPUTED,NARROW_INT,-1.000000000,59.638294220,-13.599914551,0.0,0.380230576,0.494886547,\"681H\",34,25,25,17,04,00,30,33*76bdaf0d", "robot status", "#INSPVAXA,USB3,0,46.0,FINESTEERING,2113,382083.150,02008000,471d,15824;INS_SOLUTION_GOOD,INS_RTKFIXED,37.37018131486,126.72087192674,9.8997,22.3000,0.0193,-0.0038,-0.0077,-0.396597239,-0.683463838,54.601157126,0.1525,0.1524,0.1265,0.0353,0.0340,0.0225,0.0327,0.0323,0.0988,0f000041,0*d9aa2c96", "robot status", "#DUALANTENNAHEADINGA,USB3,0,46.0,FINESTEERING,2113,382083.200,02008000,d426,15824;SOL_COMPUTED,NARROW_INT,-1.000000000,59.773227692,-14.014251709,0.0,0.528154016,0.817876518,\"681H\",34,24,24,17,04,00,30,33*78ae3e7a", "robot status", "#INSPVAXA,USB3,0,46.0,FINESTEERING,2113,382083.300,02008000,471d,15824;INS_SOLUTION_GOOD,INS_RTKFIXED,37.37018129730,126.72087193816,9.8995,22.3000,0.0187,-0.0043,-0.0071,-0.396393795,-0.681219253,54.600134940,0.1525,0.1524,0.1265,0.0353,0.0340,0.0225,0.0327,0.0323,0.0988,0f000041,0*349cd800", "robot status", "#DUALANTENNAHEADINGA,USB3,0,46.0,FINESTEERING,2113,382083.300,02008000,d426,15824;SOL_COMPUTED,NARROW_INT,-1.000000000,60.163658142,-13.424652100,0.0,0.528608024,0.824866354,\"681H\",34,24,24,17,04,00,30,33*c737697a", "robot status", "#INSPVAXA,USB3,0,46.0,FINESTEERING,2113,382083.350,02008000,471d,15824;INS_SOLUTION_GOOD,INS_RTKFIXED,37.37018129225,126.72087194169,9.8994,22.3000,0.0188,-0.0040,-0.0071,-0.395015571,-0.681675909,54.599977706,0.1525,0.1524,0.1265,0.0353,0.0340,0.0225,0.0327,0.0323,0.0988,0f000041,0*8b724574", "robot status", "#DUALANTENNAHEADINGA,USB3,0,46.0,FINESTEERING,2113,382083.400,02008000,d426,15824;SOL_COMPUTED,NARROW_INT,-1.000000000,60.110683441,-14.007995605,0.0,0.534412742,0.825756669,\"681H\",34,23,23,16,04,00,30,33*3667a9c8", "robot status", "#INSPVAXA,USB3,0,46.0,FINESTEERING,2113,382083.450,02008000,471d,15824;INS_SOLUTION_GOOD,INS_RTKFIXED,37.37018128258,126.72087194904,9.8993,22.3000,0.0189,-0.0037,-0.0070,-0.393372773,-0.682324526,54.601611225,0.1525,0.1524,0.1265,0.0353,0.0340,0.0225,0.0327,0.0323,0.0988,0f000041,0*e5591fc8", "robot status", "#DUALANTENNAHEADINGA,USB3,0,46.0,FINESTEERING,2113,382083.500,02008000,d426,15824;SOL_COMPUTED,NARROW_INT,-1.000000000,60.205780029,-13.975891113,0.0,0.531275034,0.822019339,\"681H\",34,23,23,16,04,00,30,33*620ee038", "robot status", "#INSPVAXA,USB3,0,46.0,FINESTEERING,2113,382083.550,02008000,471d,15824;INS_SOLUTION_GOOD,INS_RTKFIXED,37.37018127140,126.72087195766,9.8992,22.3000,0.0184,-0.0033,-0.0069,-0.394351231,-0.682823119,54.601808059,0.1525,0.1524,0.1265,0.0353,0.0340,0.0225,0.0327,0.0323,0.0988,0f000041,0*b7cfdf28", "robot status", "#DUALANTENNAHEADINGA,USB3,0,46.0,FINESTEERING,2113,382083.600,02008000,d426,15824;SOL_COMPUTED,NARROW_INT,-1.000000000,60.258075714,-13.598541260,0.0,0.527244508,0.821917713,\"681H\",34,23,23,15,04,00,30,33*dab80345", "robot status", "#INSPVAXA,USB3,0,46.0,FINESTEERING,2113,382083.700,02008000,471d,15824;INS_SOLUTION_GOOD,INS_RTKFIXED,37.37018125566,126.72087196982,9.8990,22.3000,0.0181,-0.0037,-0.0068,-0.392555682,-0.681556249,54.602043800,0.1525,0.1524,0.1265,0.0353,0.0340,0.0225,0.0327,0.0323,0.0988,0f000041,0*8277c102", "robot status", "#INSPVAXA,USB3,0,46.0,FINESTEERING,2113,382083.750,02008000,471d,15824;INS_SOLUTION_GOOD,INS_RTKFIXED,37.37018125126,126.72087197345,9.8989,22.3000,0.0180,-0.0037,-0.0067,-0.392480566,-0.681142254,54.602032994,0.1525,0.1524,0.1265,0.0353,0.0340,0.0225,0.0327,0.0323,0.0988,0f000041,0*50e5afbf", "robot status", "#INSPVAXA,USB3,0,46.0,FINESTEERING,2113,382083.750,02008000,471d,15824;INS_SOLUTION_GOOD,INS_RTKFIXED,37.37018125126,126.72087197345,9.8989,22.3000,0.0180,-0.0037,-0.0067,-0.392480566,-0.681142254,54.602032994,0.1525,0.1524,0.1265,0.0353,0.0340,0.0225,0.0327,0.0323,0.0988,0f000041,0*50e5afbf", "robot status", "#DUALANTENNAHEADINGA,USB3,0,46.0,FINESTEERING,2113,382083.800,02008000,d426,15824;SOL_COMPUTED,NARROW_INT,-1.000000000,60.228034973,-13.785156250,0.0,0.529838324,0.822935879,\"681H\",34,23,23,15,04,00,30,33*167f1578", "robot status", "#INSPVAXA,USB3,0,46.0,FINESTEERING,2113,382083.900,02008000,471d,15824;INS_SOLUTION_GOOD,INS_RTKFIXED,37.37018123662,126.72087198530,9.8987,22.3000,0.0175,-0.0034,-0.0065,-0.392845841,-0.681743671,54.603289657,0.1525,0.1524,0.1265,0.0353,0.0340,0.0225,0.0327,0.0323,0.0988,0f000041,0*ec88e29d", "robot status", "#DUALANTENNAHEADINGA,USB3,0,46.0,FINESTEERING,2113,382083.900,02008000,d426,15824;SOL_COMPUTED,NARROW_INT,-1.000000000,60.254852295,-14.083831787,0.0,0.525082588,0.814651728,\"681H\",34,23,23,15,04,00,30,33*247b3d88", "robot status", "#INSPVAXA,USB3,0,46.0,FINESTEERING,2113,382083.950,02008000,471d,15824;INS_SOLUTION_GOOD,INS_RTKFIXED,37.37018123248,126.72087198893,9.8986,22.3000,0.0174,-0.0037,-0.0064,-0.392513548,-0.682168872,54.603045450,0.1525,0.1524,0.1265,0.0353,0.0340,0.0225,0.0327,0.0323,0.0988,0f000041,0*c79640ca", "robot status", "#DUALANTENNAHEADINGA,USB3,0,46.0,FINESTEERING,2113,382084.000,02008000,d426,15824;SOL_COMPUTED,NARROW_INT,-1.000000000,60.436763763,-13.538787842,0.0,0.530071735,0.824255764,\"681H\",34,23,23,15,04,00,30,33*0f27d5bc", "robot status", "#INSPVAXA,USB3,0,44.0,FINESTEERING,2113,382084.100,02008000,471d,15824;INS_SOLUTION_GOOD,INS_RTKFIXED,37.37018121529,126.72087199539,9.8986,22.3000,0.0170,-0.0036,-0.0066,-0.392597889,-0.681364541,54.604617036,0.1542,0.1546,0.1278,0.0358,0.0345,0.0226,0.0331,0.0326,0.0995,0f000041,0*3c44bead", "robot status", "#INSPVAXA,USB3,0,44.0,FINESTEERING,2113,382084.150,02008000,471d,15824;INS_SOLUTION_GOOD,INS_RTKFIXED,37.37018120971,126.72087199588,9.8986,22.3000,0.0170,-0.0035,-0.0067,-0.392882714,-0.682098947,54.604784068,0.1542,0.1546,0.1278,0.0358,0.0345,0.0226,0.0331,0.0326,0.0995,0f000041,0*0a680397", "robot status", "#INSPVAXA,USB3,0,44.0,FINESTEERING,2113,382084.150,02008000,471d,15824;INS_SOLUTION_GOOD,INS_RTKFIXED,37.37018120971,126.72087199588,9.8986,22.3000,0.0170,-0.0035,-0.0067,-0.392882714,-0.682098947,54.604784068,0.1542,0.1546,0.1278,0.0358,0.0345,0.0226,0.0331,0.0326,0.0995,0f000041,0*0a680397", "robot status", "#DUALANTENNAHEADINGA,USB3,0,44.0,FINESTEERING,2113,382084.200,02008000,d426,15824;SOL_COMPUTED,NARROW_INT,-1.000000000,60.272026062,-14.518432617,0.0,0.526983321,0.812527776,\"681H\",34,25,25,17,04,00,30,33*7fd0b0d6", "robot status", "#INSPVAXA,USB3,0,44.0,FINESTEERING,2113,382084.300,02008000,471d,15824;INS_SOLUTION_GOOD,INS_RTKFIXED,37.37018119149,126.72087199784,9.8987,22.3000,0.0163,-0.0038,-0.0062,-0.392111961,-0.681286368,54.605344912,0.1542,0.1546,0.1278,0.0358,0.0345,0.0226,0.0331,0.0326,0.0995,0f000041,0*18945a43", "robot status", "#INSPVAXA,USB3,0,44.0,FINESTEERING,2113,382084.350,02008000,471d,15824;INS_SOLUTION_GOOD,INS_RTKFIXED,37.37018118610,126.72087199820,9.8987,22.3000,0.0163,-0.0040,-0.0064,-0.391158259,-0.681666118,54.605442323,0.1542,0.1546,0.1278,0.0358,0.0345,0.0226,0.0331,0.0326,0.0995,0f000041,0*e1ff08a7", "robot status", "#INSPVAXA,USB3,0,44.0,FINESTEERING,2113,382084.350,02008000,471d,15824;INS_SOLUTION_GOOD,INS_RTKFIXED,37.37018118610,126.72087199820,9.8987,22.3000,0.0163,-0.0040,-0.0064,-0.391158259,-0.681666118,54.605442323,0.1542,0.1546,0.1278,0.0358,0.0345,0.0226,0.0331,0.0326,0.0995,0f000041,0*e1ff08a7", "robot status", "#DUALANTENNAHEADINGA,USB3,0,44.0,FINESTEERING,2113,382084.400,02008000,d426,15824;SOL_COMPUTED,NARROW_INT,-1.000000000,60.279487610,-14.789825439,0.0,0.524249315,0.807350755,\"681H\",34,24,24,16,04,00,30,33*07c5761c", "robot status", "#INSPVAXA,USB3,0,44.0,FINESTEERING,2113,382084.500,02008000,471d,15824;INS_SOLUTION_GOOD,INS_RTKFIXED,37.37018116831,126.72087199952,9.8987,22.3000,0.0158,-0.0041,-0.0063,-0.391263300,-0.682226891,54.604567330,0.1542,0.1546,0.1278,0.0358,0.0345,0.0226,0.0331,0.0326,0.0995,0f000041,0*6e94f495", "robot status", "#INSPVAXA,USB3,0,44.0,FINESTEERING,2113,382084.550,02008000,471d,15824;INS_SOLUTION_GOOD,INS_RTKFIXED,37.37018116317,126.72087199981,9.8987,22.3000,0.0159,-0.0040,-0.0063,-0.391367325,-0.682579305,54.605108963,0.1542,0.1546,0.1278,0.0358,0.0345,0.0226,0.0331,0.0326,0.0995,0f000041,0*71db3841", "robot status", "#INSPVAXA,USB3,0,44.0,FINESTEERING,2113,382084.550,02008000,471d,15824;INS_SOLUTION_GOOD,INS_RTKFIXED,37.37018116317,126.72087199981,9.8987,22.3000,0.0159,-0.0040,-0.0063,-0.391367325,-0.682579305,54.605108963,0.1542,0.1546,0.1278,0.0358,0.0345,0.0226,0.0331,0.0326,0.0995,0f000041,0*71db3841", "robot status", "#INSPVAXA,USB3,0,44.0,FINESTEERING,2113,382084.650,02008000,471d,15824;INS_SOLUTION_GOOD,INS_RTKFIXED,37.37018115322,126.72087200054,9.8987,22.3000,0.0157,-0.0041,-0.0063,-0.390341511,-0.682701874,54.606530916,0.1542,0.1546,0.1278,0.0358,0.0345,0.0226,0.0331,0.0326,0.0995,0f000041,0*12174404", "robot status", "#INSPVAXA,USB3,0,44.0,FINESTEERING,2113,382084.700,02008000,471d,15824;INS_SOLUTION_GOOD,INS_RTKFIXED,37.37018114654,126.72087200137,9.8988,22.3000,0.0156,-0.0040,-0.0061,-0.390113059,-0.681866781,54.606404476,0.1542,0.1546,0.1278,0.0358,0.0345,0.0226,0.0331,0.0326,0.0995,0f000041,0*c51aed2b", "robot status", "#INSPVAXA,USB3,0,44.0,FINESTEERING,2113,382084.750,02008000,471d,15824;INS_SOLUTION_GOOD,INS_RTKFIXED,37.37018114182,126.72087200167,9.8988,22.3000,0.0156,-0.0044,-0.0060,-0.390348149,-0.681836746,54.606466779,0.1542,0.1546,0.1278,0.0358,0.0345,0.0226,0.0331,0.0326,0.0995,0f000041,0*e690f5e1", "robot status", "#INSPVAXA,USB3,0,44.0,FINESTEERING,2113,382084.750,02008000,471d,15824;INS_SOLUTION_GOOD,INS_RTKFIXED,37.37018114182,126.72087200167,9.8988,22.3000,0.0156,-0.0044,-0.0060,-0.390348149,-0.681836746,54.606466779,0.1542,0.1546,0.1278,0.0358,0.0345,0.0226,0.0331,0.0326,0.0995,0f000041,0*e690f5e1", "robot status", "#DUALANTENNAHEADINGA,USB3,0,44.0,FINESTEERING,2113,382084.800,02008000,d426,15824;SOL_COMPUTED,NARROW_INT,-1.000000000,60.193317413,-14.857940674,0.0,0.523242950,0.804948032,\"681H\",34,25,25,17,04,00,30,33*f7bee4f9", "robot status", "#INSPVAXA,USB3,0,44.0,FINESTEERING,2113,382084.900,02008000,471d,15824;INS_SOLUTION_GOOD,INS_RTKFIXED,37.37018112645,126.72087200283,9.8988,22.3000,0.0154,-0.0045,-0.0063,-0.389313818,-0.681463432,54.606889002,0.1542,0.1546,0.1278,0.0358,0.0345,0.0226,0.0331,0.0326,0.0995,0f000041,0*f585c54b", "robot status", "#INSPVAXA,USB3,0,44.0,FINESTEERING,2113,382084.950,02008000,471d,15824;INS_SOLUTION_GOOD,INS_RTKFIXED,37.37018112215,126.72087200306,9.8987,22.3000,0.0155,-0.0044,-0.0061,-0.388950107,-0.681144615,54.606577789,0.1542,0.1546,0.1278,0.0358,0.0345,0.0226,0.0331,0.0326,0.0995,0f000041,0*a876c4df", "robot status", "#INSPVAXA,USB3,0,44.0,FINESTEERING,2113,382084.950,02008000,471d,15824;INS_SOLUTION_GOOD,INS_RTKFIXED,37.37018112215,126.72087200306,9.8987,22.3000,0.0155,-0.0044,-0.0061,-0.388950107,-0.681144615,54.606577789,0.1542,0.1546,0.1278,0.0358,0.0345,0.0226,0.0331,0.0326,0.0995,0f000041,0*a876c4df", "robot status", "#INSPVAXA,USB3,0,44.0,FINESTEERING,2113,382085.050,02008000,471d,15824;INS_SOLUTION_GOOD,INS_RTKFIXED,37.37018111428,126.72087200503,9.8986,22.3000,0.0154,-0.0045,-0.0063,-0.388327729,-0.680788929,54.606539652,0.1555,0.1561,0.1287,0.0363,0.0349,0.0227,0.0334,0.0329,0.1002,0f000041,0*eb8edc3c", "robot status", "#INSPVAXA,USB3,0,45.0,FINESTEERING,2113,382085.100,02000000,471d,15824;INS_SOLUTION_GOOD,INS_RTKFIXED,37.37018111062,126.72087200862,9.8984,22.3000,0.0152,-0.0043,-0.0063,-0.387618946,-0.681036149,54.606913941,0.1555,0.1561,0.1287,0.0363,0.0349,0.0227,0.0334,0.0329,0.1002,0f000041,0*a4603479", "robot status", "#INSPVAXA,USB3,0,45.0,FINESTEERING,2113,382085.150,02000000,471d,15824;INS_SOLUTION_GOOD,INS_RTKFIXED,37.37018110833,126.72087201147,9.8981,22.3000,0.0153,-0.0041,-0.0063,-0.388120849,-0.681373103,54.606406367,0.1555,0.1561,0.1287,0.0363,0.0349,0.0227,0.0334,0.0329,0.1002,0f000041,0*3db8e125", "robot status", "#INSPVAXA,USB3,0,45.0,FINESTEERING,2113,382085.150,02000000,471d,15824;INS_SOLUTION_GOOD,INS_RTKFIXED,37.37018110833,126.72087201147,9.8981,22.3000,0.0153,-0.0041,-0.0063,-0.388120849,-0.681373103,54.606406367,0.1555,0.1561,0.1287,0.0363,0.0349,0.0227,0.0334,0.0329,0.1002,0f000041,0*3db8e125", "robot status", "#INSPVAXA,USB3,0,45.0,FINESTEERING,2113,382085.250,02000000,471d,15824;INS_SOLUTION_GOOD,INS_RTKFIXED,37.37018110247,126.72087201790,9.8976,22.3000,0.0150,-0.0041,-0.0064,-0.389408288,-0.680926110,54.608105838,0.1555,0.1561,0.1287,0.0363,0.0349,0.0227,0.0334,0.0329,0.1002,0f000041,0*110743b3", "robot status", "#INSPVAXA,USB3,0,45.0,FINESTEERING,2113,382085.300,02000000,471d,15824;INS_SOLUTION_GOOD,INS_RTKFIXED,37.37018110023,126.72087202080,9.8974,22.3000,0.0148,-0.0040,-0.0066,-0.389825699,-0.680545836,54.608147784,0.1555,0.1561,0.1287,0.0363,0.0349,0.0227,0.0334,0.0329,0.1002,0f000041,0*e5153cc1", "robot status", "#INSPVAXA,USB3,0,45.0,FINESTEERING,2113,382085.350,02000000,471d,15824;INS_SOLUTION_GOOD,INS_RTKFIXED,37.37018109806,126.72087202373,9.8971,22.3000,0.0150,-0.0039,-0.0071,-0.389761136,-0.681100082,54.608404466,0.1555,0.1561,0.1287,0.0363,0.0349,0.0227,0.0334,0.0329,0.1002,0f000041,0*064dbc0a", "robot status", "#INSPVAXA,USB3,0,45.0,FINESTEERING,2113,382085.350,02000000,471d,15824;INS_SOLUTION_GOOD,INS_RTKFIXED,37.37018109806,126.72087202373,9.8971,22.3000,0.0150,-0.0039,-0.0071,-0.389761136,-0.681100082,54.608404466,0.1555,0.1561,0.1287,0.0363,0.0349,0.0227,0.0334,0.0329,0.1002,0f000041,0*064dbc0a", "robot status", "#INSPVAXA,USB3,0,45.0,FINESTEERING,2113,382085.450,02000000,471d,15824;INS_SOLUTION_GOOD,INS_RTKFIXED,37.37018109413,126.72087202965,9.8965,22.3000,0.0154,-0.0037,-0.0071,-0.390473444,-0.681932439,54.609035252,0.1555,0.1561,0.1287,0.0363,0.0349,0.0227,0.0334,0.0329,0.1002,0f000041,0*f35e0254", "robot status", "#INSPVAXA,USB3,0,45.0,FINESTEERING,2113,382085.500,02000000,471d,15824;INS_SOLUTION_GOOD,INS_RTKFIXED,37.37018109099,126.72087203341,9.8963,22.3000,0.0151,-0.0038,-0.0073,-0.390302010,-0.681515793,54.608838668,0.1555,0.1561,0.1287,0.0363,0.0349,0.0227,0.0334,0.0329,0.1002,0f000041,0*8dbee4f2", "robot status", "#INSPVAXA,USB3,0,45.0,FINESTEERING,2113,382085.550,02000000,471d,15824;INS_SOLUTION_GOOD,INS_RTKFIXED,37.37018108925,126.72087203639,9.8960,22.3000,0.0151,-0.0036,-0.0074,-0.390808808,-0.681114275,54.609931880,0.1555,0.1561,0.1287,0.0363,0.0349,0.0227,0.0334,0.0329,0.1002,0f000041,0*13d3ad01", "robot status", "#INSPVAXA,USB3,0,45.0,FINESTEERING,2113,382085.600,02000000,471d,15824;INS_SOLUTION_GOOD,INS_RTKFIXED,37.37018108758,126.72087203939,9.8957,22.3000,0.0152,-0.0033,-0.0074,-0.391036253,-0.680831314,54.609148861,0.1555,0.1561,0.1287,0.0363,0.0349,0.0227,0.0334,0.0329,0.1002,0f000041,0*68270744", "robot status", "#INSPVAXA,USB3,0,45.0,FINESTEERING,2113,382085.650,02000000,471d,15824;INS_SOLUTION_GOOD,INS_RTKFIXED,37.37018108639,126.72087204293,9.8954,22.3000,0.0170,-0.0013,-0.0073,-0.390974950,-0.677563088,54.602634773,0.1555,0.1561,0.1287,0.0363,0.0349,0.0227,0.0334,0.0329,0.1002,0f000041,0*693df762", "robot status", "#INSPVAXA,USB3,0,45.0,FINESTEERING,2113,382085.700,02000000,471d,15824;INS_SOLUTION_GOOD,INS_RTKFIXED,37.37018108539,126.72087204997,9.8951,22.3000,0.0211,0.0054,-0.0074,-0.393752759,-0.671949359,54.577990701,0.1555,0.1561,0.1287,0.0363,0.0349,0.0227,0.0334,0.0329,0.1002,0f000041,0*7f63edeb", "robot status", "#INSPVAXA,USB3,0,45.0,FINESTEERING,2113,382085.750,02000000,471d,15824;INS_SOLUTION_GOOD,INS_RTKFIXED,37.37018108748,126.72087206024,9.8948,22.3000,0.0248,0.0136,-0.0076,-0.397228108,-0.665679759,54.530054120,0.1555,0.1561,0.1287,0.0363,0.0349,0.0227,0.0334,0.0329,0.1002,0f000041,0*e74c08eb", "robot status", "#INSPVAXA,USB3,0,45.0,FINESTEERING,2113,382085.800,02000000,471d,15824;INS_SOLUTION_GOOD,INS_RTKFIXED,37.37018109115,126.72087207378,9.8945,22.3000,0.0269,0.0147,-0.0077,-0.394013419,-0.668425256,54.460278298,0.1555,0.1561,0.1287,0.0363,0.0349,0.0227,0.0334,0.0329,0.1002,0f000041,0*1ba4d631", "robot status", "#INSPVAXA,USB3,0,45.0,FINESTEERING,2113,382085.850,02000000,471d,15824;INS_SOLUTION_GOOD,INS_RTKFIXED,37.37018109273,126.72087208506,9.8942,22.3000,0.0214,0.0058,-0.0066,-0.393181072,-0.677636556,54.321957645,0.1555,0.1561,0.1287,0.0363,0.0349,0.0227,0.0334,0.0329,0.1002,0f000041,0*1535fb94", "robot status", "#INSPVAXA,USB3,0,45.0,FINESTEERING,2113,382085.900,02000000,471d,15824;INS_SOLUTION_GOOD,INS_RTKFIXED,37.37018109297,126.72087209081,9.8939,22.3000,0.0159,-0.0023,-0.0076,-0.384420891,-0.676878771,54.174088596,0.1555,0.1561,0.1287,0.0363,0.0349,0.0227,0.0334,0.0329,0.1002,0f000041,0*26ae681c", "robot status", "#INSPVAXA,USB3,0,45.0,FINESTEERING,2113,382085.950,02000000,471d,15824;INS_SOLUTION_GOOD,INS_RTKFIXED,37.37018109064,126.72087209145,9.8935,22.3000,0.0107,-0.0110,-0.0099,-0.358586460,-0.694648131,54.055877176,0.1555,0.1561,0.1287,0.0363,0.0349,0.0227,0.0334,0.0329,0.1002,0f000041,0*518b838e", "robot status", "#INSPVAXA,USB3,0,45.0,FINESTEERING,2113,382086.000,02000000,471d,15824;INS_SOLUTION_GOOD,INS_RTKFIXED,37.37018108712,126.72087208898,9.8931,22.3000,0.0091,-0.0129,-0.0078,-0.348943767,-0.691888816,53.901578833,0.1555,0.1561,0.1287,0.0363,0.0349,0.0227,0.0334,0.0329,0.1002,0f000041,0*63acd863", "robot status", "#INSPVAXA,USB3,0,45.0,FINESTEERING,2113,382086.050,02000000,471d,15824;INS_SOLUTION_GOOD,INS_RTKFIXED,37.37018108230,126.72087208698,9.8928,22.3000,0.0107,-0.0091,-0.0102,-0.335720229,-0.693918826,53.739928797,0.1562,0.1573,0.1292,0.0367,0.0353,0.0228,0.0336,0.0332,0.1009,0f000041,0*707028c5", "robot status", "#INSPVAXA,USB3,0,45.0,FINESTEERING,2113,382086.100,02000000,471d,15824;INS_SOLUTION_GOOD,INS_RTKFIXED,37.37018107657,126.72087208482,9.8926,22.3000,0.0144,-0.0140,-0.0067,-0.322126968,-0.717887766,53.592890267,0.1562,0.1573,0.1292,0.0367,0.0353,0.0228,0.0336,0.0332,0.1009,0f000041,0*d42c4c15", "robot status", "#INSPVAXA,USB3,0,46.5,FINESTEERING,2113,382086.150,02000000,471d,15824;INS_SOLUTION_GOOD,INS_RTKFIXED,37.37018107058,126.72087208192,9.8924,22.3000,0.0077,-0.0112,-0.0081,-0.326724531,-0.720660709,53.351117406,0.1562,0.1573,0.1292,0.0367,0.0353,0.0228,0.0336,0.0332,0.1009,0f000041,0*765f9ea8", "robot status", "#INSPVAXA,USB3,0,46.5,FINESTEERING,2113,382086.200,02000000,471d,15824;INS_SOLUTION_GOOD,INS_RTKFIXED,37.37018106373,126.72087208054,9.8922,22.3000,0.0086,-0.0085,-0.0090,-0.303999444,-0.745863366,53.081469412,0.1562,0.1573,0.1292,0.0367,0.0353,0.0228,0.0336,0.0332,0.1009,0f000041,0*c75da79f", "robot status", "#INSPVAXA,USB3,0,46.5,FINESTEERING,2113,382086.250,02000000,471d,15824;INS_SOLUTION_GOOD,INS_RTKFIXED,37.37018105678,126.72087208164,9.8920,22.3000,0.0118,-0.0030,-0.0050,-0.283717963,-0.756844875,52.801710722,0.1562,0.1573,0.1292,0.0367,0.0353,0.0228,0.0336,0.0332,0.1009,0f000041,0*a6592b26", "robot status", "#INSPVAXA,USB3,0,46.5,FINESTEERING,2113,382086.300,02000000,471d,15824;INS_SOLUTION_GOOD,INS_RTKFIXED,37.37018105162,126.72087208458,9.8919,22.3000,0.0100,0.0021,-0.0058,-0.280526384,-0.765096699,52.474863037,0.1562,0.1573,0.1292,0.0367,0.0353,0.0228,0.0336,0.0332,0.1009,0f000041,0*786c9554", "robot status", "#INSPVAXA,USB3,0,46.5,FINESTEERING,2113,382086.350,02000000,471d,15824;INS_SOLUTION_GOOD,INS_RTKFIXED,37.37018104442,126.72087208875,9.8918,22.3000,0.0019,-0.0003,-0.0061,-0.278242514,-0.772989580,52.035014102,0.1562,0.1573,0.1292,0.0367,0.0353,0.0228,0.0336,0.0332,0.1009,0f000041,0*06288815", "robot status", "#INSPVAXA,USB3,0,46.5,FINESTEERING,2113,382086.400,02000000,471d,15824;INS_SOLUTION_GOOD,INS_RTKFIXED,37.37018103551,126.72087209373,9.8917,22.3000,0.0026,0.0021,-0.0046,-0.267563310,-0.735808691,51.529219686,0.1562,0.1573,0.1292,0.0367,0.0353,0.0228,0.0336,0.0332,0.1009,0f000041,0*119707c0", "robot status", "#INSPVAXA,USB3,0,46.5,FINESTEERING,2113,382086.450,02000000,471d,15824;INS_SOLUTION_GOOD,INS_RTKFIXED,37.37018102784,126.72087209769,9.8916,22.3000,0.0125,-0.0025,-0.0024,-0.261419657,-0.727539494,51.022170224,0.1562,0.1573,0.1292,0.0367,0.0353,0.0228,0.0336,0.0332,0.1009,0f000041,0*754e0fdd", "robot status", "#DUALANTENNAHEADINGA,USB3,0,46.5,FINESTEERING,2113,382086.500,02000000,d426,15824;SOL_COMPUTED,NARROW_INT,-1.000000000,55.612857819,-14.747497559,0.0,0.524562240,0.806664884,\"681H\",34,26,26,16,04,00,30,33*0942c3a6", "robot status", "#INSPVAXA,USB3,0,46.5,FINESTEERING,2113,382086.550,02000000,471d,15824;INS_SOLUTION_GOOD,INS_RTKFIXED,37.37018101284,126.72087210307,9.8917,22.3000,-0.0083,0.0015,-0.0050,-0.328436898,-0.719943534,49.976364802,0.1562,0.1573,0.1292,0.0367,0.0353,0.0228,0.0336,0.0332,0.1009,0f000041,0*af084f43", "robot status", "#INSPVAXA,USB3,0,46.5,FINESTEERING,2113,382086.600,02000000,471d,15824;INS_SOLUTION_GOOD,INS_RTKFIXED,37.37018100405,126.72087210605,9.8917,22.3000,0.0080,-0.0041,-0.0044,-0.276998680,-0.692649879,49.411506456,0.1562,0.1573,0.1292,0.0367,0.0353,0.0228,0.0336,0.0332,0.1009,0f000041,0*a229d347", "robot status", "#INSPVAXA,USB3,0,46.5,FINESTEERING,2113,382086.650,02000000,471d,15824;INS_SOLUTION_GOOD,INS_RTKFIXED,37.37018099969,126.72087210634,9.8916,22.3000,0.0101,-0.0070,-0.0080,-0.299322106,-0.679263288,48.934049167,0.1562,0.1573,0.1292,0.0367,0.0353,0.0228,0.0336,0.0332,0.1009,0f000041,0*5c2231b1", "robot status", "#DUALANTENNAHEADINGA,USB3,0,46.5,FINESTEERING,2113,382086.700,02000000,d426,15824;SOL_COMPUTED,NARROW_INT,-1.000000000,53.691761017,-15.024719238,0.0,0.529522061,0.805150807,\"681H\",34,26,26,16,04,00,30,33*2decc7ca", "robot status", "#INSPVAXA,USB3,0,46.5,FINESTEERING,2113,382086.750,02000000,471d,15824;INS_SOLUTION_GOOD,INS_RTKFIXED,37.37018098519,126.72087211079,9.8914,22.3000,-0.0007,0.0034,-0.0104,-0.263916927,-0.693815485,48.048757444,0.1562,0.1573,0.1292,0.0367,0.0353,0.0228,0.0336,0.0332,0.1009,0f000041,0*cb7f3707", "robot status", "#INSPVAXA,USB3,0,46.5,FINESTEERING,2113,382086.800,02000000,471d,15824;INS_SOLUTION_GOOD,INS_RTKFIXED,37.37018097319,126.72087211768,9.8912,22.3000,-0.0131,0.0094,-0.0092,-0.256669899,-0.699847584,47.512512761,0.1562,0.1573,0.1292,0.0367,0.0353,0.0228,0.0336,0.0332,0.1009,0f000041,0*2ec110e8", "robot status", "#INSPVAXA,USB3,0,46.5,FINESTEERING,2113,382086.850,02000000,471d,15824;INS_SOLUTION_GOOD,INS_RTKFIXED,37.37018095795,126.72087212713,9.8909,22.3000,-0.0053,0.0100,-0.0112,-0.216594867,-0.687147884,46.913861402,0.1562,0.1573,0.1292,0.0367,0.0353,0.0228,0.0336,0.0332,0.1009,0f000041,0*f8c96780", "robot status", "#DUALANTENNAHEADINGA,USB3,0,46.5,FINESTEERING,2113,382086.900,02000000,d426,15824;SOL_COMPUTED,NARROW_INT,-1.000000000,51.480041504,-15.522857666,0.0,0.527016401,0.796175599,\"681H\",33,25,25,16,04,00,30,33*28ddc428", "robot status", "#INSPVAXA,USB3,0,46.5,FINESTEERING,2113,382086.950,02000000,471d,15824;INS_SOLUTION_GOOD,INS_RTKFIXED,37.37018094910,126.72087213756,9.8903,22.3000,0.0109,0.0001,-0.0049,-0.247796783,-0.721341806,45.767687785,0.1562,0.1573,0.1292,0.0367,0.0353,0.0228,0.0336,0.0332,0.1009,0f000041,0*5b2817cb", "robot status", "#INSPVAXA,USB3,0,46.5,FINESTEERING,2113,382087.000,02000000,471d,15824;INS_SOLUTION_GOOD,INS_RTKFIXED,37.37018093983,126.72087213976,9.8901,22.3000,-0.0124,-0.0023,-0.0071,-0.252446922,-0.687751865,45.284452516,0.1562,0.1573,0.1292,0.0367,0.0353,0.0228,0.0336,0.0332,0.1009,0f000041,0*f7cafa3d", "robot status", "#INSPVAXA,USB3,0,46.5,FINESTEERING,2113,382087.050,02000000,471d,15824;INS_SOLUTION_GOOD,INS_RTKFIXED,37.37018092741,126.72087213979,9.8900,22.3000,-0.0030,-0.0065,0.0020,-0.191160370,-0.691288795,44.781390130,0.1537,0.1609,0.1285,0.0368,0.0362,0.0228,0.0337,0.0332,0.1017,0f000041,0*59e64c0c", "robot status", "#DUALANTENNAHEADINGA,USB3,0,46.5,FINESTEERING,2113,382087.100,02000000,d426,15824;SOL_COMPUTED,NARROW_INT,-1.000000000,49.628173828,-16.236206055,0.0,0.520508349,0.781016529,\"681H\",34,25,25,16,04,00,30,33*67ba2c5d", "robot status", "#INSPVAXA,USB3,0,47.0,FINESTEERING,2113,382087.150,02000000,471d,15824;INS_SOLUTION_GOOD,INS_RTKFIXED,37.37018090064,126.72087213789,9.8897,22.3000,-0.0244,0.0027,-0.0095,-0.318881764,-0.666042858,43.697330175,0.1537,0.1609,0.1285,0.0368,0.0362,0.0228,0.0337,0.0332,0.1017,0f000041,0*31c62f21", "robot status", "#INSPVAXA,USB3,0,47.0,FINESTEERING,2113,382087.200,02000000,471d,15824;INS_SOLUTION_GOOD,INS_RTKFIXED,37.37018088406,126.72087214139,9.8896,22.3000,-0.0046,0.0003,-0.0044,-0.235717272,-0.626378954,43.137417666,0.1537,0.1609,0.1285,0.0368,0.0362,0.0228,0.0337,0.0332,0.1017,0f000041,0*07ba3b05", "robot status", "#INSPVAXA,USB3,0,47.0,FINESTEERING,2113,382087.250,02000000,471d,15824;INS_SOLUTION_GOOD,INS_RTKFIXED,37.37018088093,126.72087214008,9.8895,22.3000,0.0287,-0.0114,-0.0075,-0.244952610,-0.642381026,42.570357262,0.1537,0.1609,0.1285,0.0368,0.0362,0.0228,0.0337,0.0332,0.1017,0f000041,0*6dfd071a", "robot status", "#DUALANTENNAHEADINGA,USB3,0,47.0,FINESTEERING,2113,382087.300,02000000,d426,15824;SOL_COMPUTED,NARROW_INT,-1.000000000,47.469841003,-16.205749512,0.0,0.520741045,0.783295333,\"681H\",34,24,24,17,04,00,30,33*116a5ade", "robot status", "#INSPVAXA,USB3,0,47.0,FINESTEERING,2113,382087.350,02000000,471d,15824;INS_SOLUTION_GOOD,INS_RTKFIXED,37.37018087620,126.72087214627,9.8888,22.3000,0.0151,0.0109,-0.0127,-0.224446686,-0.628996304,41.563238667,0.1537,0.1609,0.1285,0.0368,0.0362,0.0228,0.0337,0.0332,0.1017,0f000041,0*905f2bdc", "robot status", "#DUALANTENNAHEADINGA,USB3,0,47.0,FINESTEERING,2113,382087.400,02000000,d426,15824;SOL_COMPUTED,NARROW_INT,-1.000000000,46.380996704,-16.700195313,0.0,0.518081725,0.787882507,\"681H\",34,23,23,17,04,00,30,33*be140444", "robot status", "#INSPVAXA,USB3,0,47.0,FINESTEERING,2113,382087.450,02000000,471d,15824;INS_SOLUTION_GOOD,INS_RTKFIXED,37.37018090370,126.72087216668,9.8880,22.3000,0.0830,0.0260,-0.0115,-0.214462895,-0.641533972,40.858445824,0.1537,0.1609,0.1285,0.0368,0.0362,0.0228,0.0337,0.0332,0.1017,0f000041,0*1332c6d8", "robot status"]
  in  "file path":path=path "C:/AGV/Log/0709/Patrolrobot_2020-07-09  오후 7-06-35_log.txt"
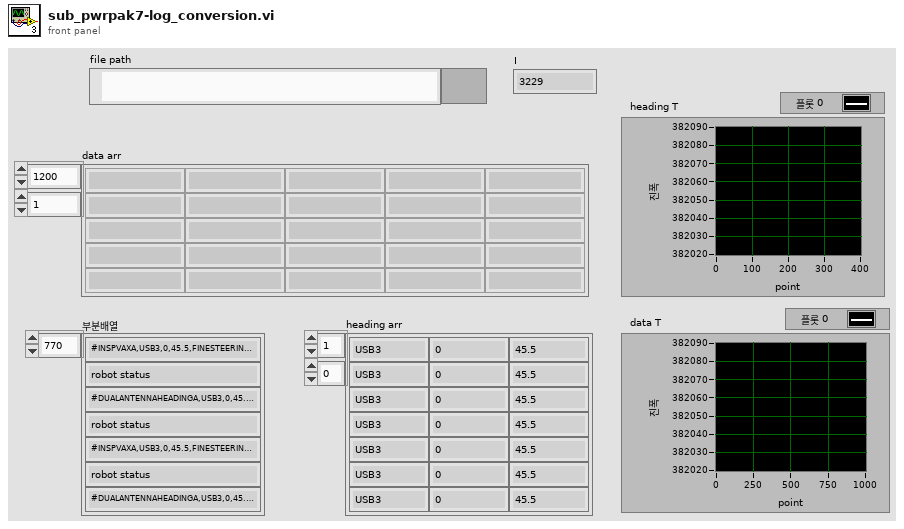
[diagram p1: front panel]
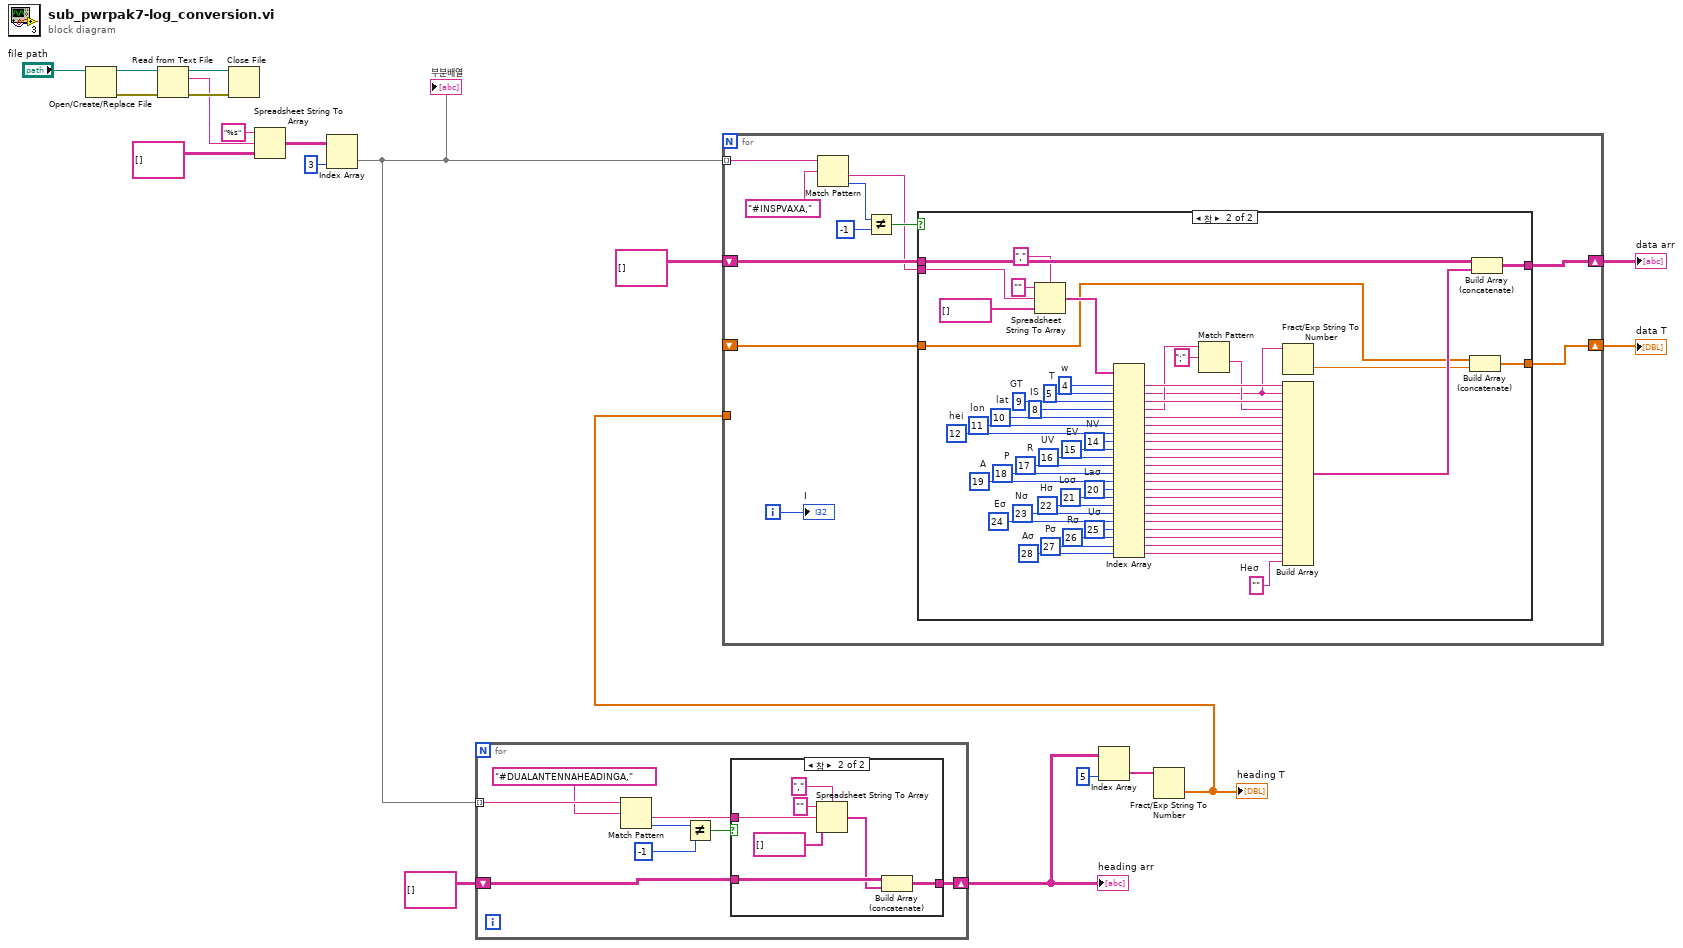
[diagram p0: block diagram]
diagram:
  n1 = Open/Create/Replace File(file path (use dialog)="file path") -> (refnum out=w19:refnum<file>, error out=w18:errorcluster)  [unwired: 5 in, 1 out]
  n2 = Read from Text File(file (use dialog)=w19, error in=w18) -> (refnum out=w16:refnum<file>, text=w14:string, error out=w17:errorcluster)  [unwired: 2 in, 1 out]
  n3 = Close File(refnum=w16, error in=w17) -> ()  [unwired: 2 out]
  n4 = Spreadsheet String To Array(format string="%s" ("포맷 문자열"), spreadsheet string=w14, array type (2D Dbl)=string[][] []) -> (array=w11:string[][])  [unwired: 1 in]
  n5 = Index Array(array=w11, index (col)=3 ("비활성화된 인덱스 (열)")) -> (element=w7:string[])  [unwired: 1 in]
  "부분배열" <- w7
  n6 = for {
    tunnel: w7 -> [w27] mode=indexing
    shift-right: [w20] -> w5
    shift-left: string[][] [] -> [w22]
    n7 = Match Pattern(string=w27, regular expression="#DUALANTENNAHEADINGA," ("정규식")) -> (after substring=w21:string, offset past match=w25:i32)  [unwired: 1 in, 2 out]
    n8 = Not Equal?(x=w25, y=-1) -> (x != y?=w23:bool)
    n9 = case shown="참" w23 {
      tunnel: w22 -> [w28 w35]
      tunnel: w21 -> [_ w31]
      tunnel: [w28 w34] -> w20
      frame False {
      }
      frame True {
        n10 = Spreadsheet String To Array(delimiter (Tab)="," ("구분 문자 (탭)"), format string="" ("포맷 문자열"), spreadsheet string=w31, array type (2D Dbl)=string[] []) -> (array=w29:string[])
        n11 = Build Array (concatenate)(w35, w29) -> (w34:string[][])
      }
    }
  }
  "heading arr" <- w5
  n12 = Index Array(array=w5, index (col)=5 ("비활성화된 인덱스 (열)")) -> (element=w3:string[])  [unwired: 1 in]
  n13 = Fract/Exp String To Number(string=w3) -> (number=w2:dbl[])  [unwired: 3 in, 1 out]
  "heading T" <- w2
  n14 = for {
    tunnel: w7 -> [w46] mode=indexing
    shift-right: [w39] -> w9
    shift-left: string[][] [] -> [w41]
    tunnel: w2 -> [_]
    shift-right: [w36] -> w1
    shift-left: _ -> [w37]
    i -> [w38]
    n15 = Match Pattern(string=w46, regular expression="#INSPVAXA," ("정규식")) -> (after substring=w40:string, offset past match=w44:i32)  [unwired: 1 in, 2 out]
    n16 = Not Equal?(x=w44, y=-1) -> (x != y?=w42:bool)
    n17 = case shown="참" w42 {
      tunnel: w41 -> [w48 w106]
      tunnel: w40 -> [_ w104]
      tunnel: [w48 w105] -> w39
      tunnel: w37 -> [w47 w51]
      tunnel: [w47 w50] -> w36
      frame False {
      }
      frame True {
        w53 = ""  # Heσ
        w59 = 28  # Aσ
        w60 = 27  # Pσ
        w61 = 26  # Rσ
        w62 = 25  # Uσ
        w63 = 24  # Eσ
        w69 = 23  # Nσ
        w70 = 22  # Hσ
        w71 = 21  # Loσ
        w72 = 20  # Laσ
        w76 = 19  # A
        w77 = 18  # P
        w78 = 17  # R
        w82 = 16  # UV
        w83 = 15  # EV
        w84 = 14  # NV
        w85 = 12  # hei
        w88 = 11  # lon
        w89 = 10  # lat
        w93 = 8  # IS
        w95 = 9  # GT
        w97 = 5  # T
        w99 = 4  # w
        n18 = Spreadsheet String To Array(delimiter (Tab)="," ("구분 문자 (탭)"), format string="" ("포맷 문자열"), spreadsheet string=w104, array type (2D Dbl)=string[] []) -> (array=w100:string[])
        n19 = Index Array(array=w100, index #1=w99, index #2=w97, index #3=w95, index #4=w93, index #5=w89, index #6=w88, index #7=w85, index #8=w84, index #9=w83, index #10=w82, index #11=w78, index #12=w77, index #13=w76, index #14=w72, index #15=w71, index #16=w70, index #17=w69, index #18=w63, index #19=w62, index #20=w61, index #21=w60, index #22=w59) -> (element #1=w98:string, element #2=w52:string, element #3=w94:string, element #4=w92:string, element #5=w87:string, element #6=w86:string, element #7=w81:string, element #8=w80:string, element #9=w79:string, element #10=w75:string, element #11=w74:string, element #12=w73:string, element #13=w68:string, element #14=w67:string, element #15=w66:string, element #16=w65:string, element #17=w64:string, element #18=w58:string, element #19=w57:string, element #20=w56:string, element #21=w55:string, element #22=w54:string)
        n20 = Match Pattern(string=w92, regular expression=";" ("정규식")) -> (after substring=w90:string)  [unwired: 1 in, 3 out]
        n21 = Fract/Exp String To Number(string=w52) -> (number=w49:dbl)  [unwired: 3 in, 1 out]
        n22 = Build Array(w98, w52, w94, w90, w87, w86, w81, w80, w79, w75, w74, w73, w68, w67, w66, w65, w64, w58, w57, w56, w55, w54, w53) -> (w96:string[])
        n23 = Build Array (concatenate)(w51, w49) -> (w50:dbl[])
        n24 = Build Array (concatenate)(w106, w96) -> (w105:string[][])
      }
    }
    "I" <- w38
  }
  "data arr" <- w9
  "data T" <- w1
